vi "Lab Panel V4.2.vi"() -> ()   [LabVIEW 2013]
uses:
  <vilib>/Platform/TimedLoop/XDataNode/timing_clust.ctl
  <vilib>/Platform/TimedLoop/XDataNode/nitl_modes.ctl
  <vilib>/Platform/TimedLoop/XDataNode/wakeup.ctl
  Global 1.vi
  <vilib>/platform/TimedLoop/XDataNode/XDataNode.xnode
  <vilib>/Platform/TimedLoop/XDataNode/XDNodeRunTimeDep.lvlib
panel:
  out "TEMP update":bool
  out "AI update":bool
  in  "stop":bool
  in  "Tab Control 2":T1(tab)
  out "SIG LAB05-2":T2 {"PF" format="%.2f"; "AMPS" format="%.1f"}
  out "SIG LAB05-1":T2 {"PF" format="%.2f"; "AMPS" format="%.1f"}
  out "SIG LAB04-2":T2 {"PF" format="%.2f"; "AMPS" format="%.1f"}
  out "SIG LAB04-1":T2 {"PF" format="%.2f"; "AMPS" format="%.1f"}
  out "SIG LAB03-2":T2 {"PF" format="%.2f"; "AMPS" format="%.1f"}
  out "SIG LAB03-1":T2 {"PF" format="%.2f"; "AMPS" format="%.1f"}
  out "SIG LAB02-2":T2 {"PF" format="%.2f"; "AMPS" format="%.1f"}
  in  "RUN LAB01-1":bool
  in  "O/I  LAB05-1":bool
  in  "O/I  LAB05-2":bool
  in  "O/I  LAB04-1":bool
  in  "O/I  LAB04-2":bool
  in  "O/I  LAB02-1":bool
  in  "O/I  LAB02-2":bool
  in  "O/I  LAB01-2":bool
  in  "O/I  LAB01-1":bool
  in  "O/I  LAB03-1":bool
  in  "RUN LAB05-2":bool
  in  "RUN LAB05-1":bool
  in  "RUN LAB04-2":bool
  in  "RUN LAB04-1":bool
  in  "RUN LAB03-2":bool
  in  "RUN LAB03-1":bool
  in  "RUN LAB02-2":bool
  in  "RUN LAB02-1":bool
  in  "RUN LAB01-2":bool
  in  "SELECT LAB05-2":T3(radio)
  in  "SELECT LAB05-1":T3(radio)
  in  "SELECT LAB04-2":T3(radio)
  in  "SELECT LAB04-1":T3(radio)
  in  "SELECT LAB03-2":T3(radio)
  in  "SELECT LAB03-1":T3(radio)
  in  "SELECT LAB02-2":T3(radio)
  in  "SELECT LAB02-1":T3(radio)
  in  "SELECT LAB01-2":T3(radio)
  in  "SELECT LAB01-1":T3(radio)
  in  "O/I  LAB03-2":bool
  out "SIG LAB01-1":T2 {"PF" format="%.2f"; "AMPS" format="%.1f"}
  out "SIG LAB01-2":T2 {"PF" format="%.2f"; "AMPS" format="%.1f"}
  out "SIG LAB02-1":T2 {"PF" format="%.2f"; "AMPS" format="%.1f"}
  out "DISP LAB05-2":T4 {"MINS" format="%.2g"}
  out "DISP LAB05-1":T4 {"MINS" format="%.2g"}
  out "DISP LAB04-2":T4 {"MINS" format="%.2g"}
  out "DISP LAB04-1":T4 {"MINS" format="%.2g"}
  out "DISP LAB03-2":T4 {"MINS" format="%.2g"}
  out "DISP LAB03-1":T4 {"MINS" format="%.2g"}
  in  "SET LAB05-2":T5={"NAME"="", "DESCRIPTION"="", "CYCLES"=5.0, "T-RISE mins"=0.0, "T-RISE deg C"=0.0} {"CYCLES" min=5.0 step=1.0}
  in  "SET LAB05-1":T5={"NAME"="", "DESCRIPTION"="", "CYCLES"=5.0, "T-RISE mins"=0.0, "T-RISE deg C"=0.0} {"CYCLES" min=5.0 step=1.0}
  in  "SET LAB04-2":T5={"NAME"="", "DESCRIPTION"="", "CYCLES"=5.0, "T-RISE mins"=0.0, "T-RISE deg C"=0.0} {"CYCLES" min=5.0 step=1.0}
  in  "SET LAB04-1":T5={"NAME"="", "DESCRIPTION"="", "CYCLES"=5.0, "T-RISE mins"=0.0, "T-RISE deg C"=0.0} {"CYCLES" min=5.0 step=1.0}
  in  "SET LAB03-2":T5={"NAME"="", "DESCRIPTION"="", "CYCLES"=5.0, "T-RISE mins"=0.0, "T-RISE deg C"=0.0} {"CYCLES" min=5.0 step=1.0}
  in  "SET LAB03-1":T5={"NAME"="", "DESCRIPTION"="", "CYCLES"=5.0, "T-RISE mins"=0.0, "T-RISE deg C"=0.0} {"CYCLES" min=5.0 step=1.0}
  out "DISP LAB02-2":T4 {"MINS" format="%.2g"}
  out "DISP LAB02-1":T4 {"MINS" format="%.2g"}
  in  "SET LAB02-2":T5={"NAME"="", "DESCRIPTION"="", "CYCLES"=5.0, "T-RISE mins"=0.0, "T-RISE deg C"=0.0} {"CYCLES" min=5.0 step=1.0}
  in  "SET LAB02-1":T5={"NAME"="", "DESCRIPTION"="", "CYCLES"=5.0, "T-RISE mins"=0.0, "T-RISE deg C"=0.0} {"CYCLES" min=5.0 step=1.0}
  out "RESULT LAB05-2":bool
  out "RESULT LAB05-1":bool
  out "RESULT LAB04-2":bool
  out "RESULT LAB04-1":bool
  out "RESULT LAB03-2":bool
  out "RESULT LAB03-1":bool
  out "RESULT LAB02-2":bool
  out "RESULT LAB02-1":bool
  out "RESULT LAB01-2":bool
  out "RESULT LAB01-1":bool
  in  "SET LAB01-1":T5={"NAME"="", "DESCRIPTION"="", "CYCLES"=5.0, "T-RISE mins"=0.0, "T-RISE deg C"=0.0} {"CYCLES" min=5.0 step=1.0}
  in  "SET LAB01-2":T5={"NAME"="", "DESCRIPTION"="", "CYCLES"=5.0, "T-RISE mins"=0.0, "T-RISE deg C"=0.0} {"CYCLES" min=5.0 step=1.0}
  out "DISP LAB01-1":T4 {"MINS" format="%.2g"}
  out "DISP LAB01-2":T4 {"MINS" format="%.2f"}
  out "TEMP RISE LAB05-2":cluster{"TL":dbl, "TN":dbl}
  out "TEMP RISE LAB05-1":cluster{"TL":dbl, "TN":dbl}
  out "TEMP RISE LAB04-2":cluster{"TL":dbl, "TN":dbl}
  out "TEMP RISE LAB04-1":cluster{"TL":dbl, "TN":dbl}
  out "TEMP RISE LAB03-2":cluster{"TL":dbl, "TN":dbl}
  out "TEMP RISE LAB03-1":cluster{"TL":dbl, "TN":dbl}
  out "TEMP RISE LAB02-2":cluster{"TL":dbl, "TN":dbl}
  out "TEMP RISE LAB02-1":cluster{"TL":dbl, "TN":dbl}
  out "TEMP RISE LAB01-2":cluster{"TL":dbl, "TN":dbl}
  out "TEMP RISE LAB01-1":cluster{"TL":dbl, "TN":dbl}
  in  "JIG OFF TIME (S)":dbl=2.0 min=2.0 max=10.0 step=0.5 format="%.1g"
  in  "JIG ON TIME (S)":dbl=1.0 min=1.0 max=10.0 step=0.5 format="%.1g"
  out "JIG LAB05-2":bool
  out "JIG LAB05-1":bool
  out "JIG LAB04-2":bool
  out "JIG LAB04-1":bool
  out "JIG LAB03-2":bool
  out "JIG LAB03-1":bool
  out "JIG LAB02-2":bool
  out "JIG LAB02-1":bool
  out "JIG LAB01-2":bool
  out "JIG LAB01-1":bool
  out "TEMP START LAB01-1":cluster{"TL":dbl, "TN":dbl}
  out "TEMP START LAB02-1":cluster{"TL":dbl, "TN":dbl}
  out "TEMP START LAB03-1":cluster{"TL":dbl, "TN":dbl}
  out "TEMP START LAB04-1":cluster{"TL":dbl, "TN":dbl}
  out "TEMP START LAB01-2":cluster{"TL":dbl, "TN":dbl}
  out "TEMP START LAB02-2":cluster{"TL":dbl, "TN":dbl}
  out "TEMP START LAB03-2":cluster{"TL":dbl, "TN":dbl}
  out "TEMP START LAB04-2":cluster{"TL":dbl, "TN":dbl}
  out "TEMP START LAB05-2":cluster{"TL":dbl, "TN":dbl}
  out "TEMP START LAB05-1":cluster{"TL":dbl, "TN":dbl}
  in  "MAIL SETTINGS":T6
  out "MAIL REPORT":string
  in  "TO (string):":string
  in  "Send Mail Now":bool
  in  "Auto Mail Send":bool
  in  "Network Directory":path
  out "CAL LAB01":T7 {"2 (TN) cal" min=0.0 step=0.01 format="%.2f"; "2 (TL) cal" min=0.0 step=0.01 format="%.2f"; "2 (PF) cal" min=0.0 step=0.01 format="%.2f"; "2 (V) cal" min=0.0 step=0.01 format="%.2f"; "2 (A) cal" min=0.0 step=0.01 format="%.2f"; "1 (TN) cal" min=0.0 step=0.01 format="%.2f"; "1 (TL) cal" min=0.0 step=0.01 format="%.2f"; "1 (PF) cal" min=0.0 step=0.01 format="%.2f"; "1 (V) cal" min=0.0 step=0.01 format="%.2f"; "1  (A) cal" min=0.0 step=0.01 format="%.2f"}
  out "CAL LAB03":T7 {"2 (TN) cal" min=0.0 step=0.01 format="%.2f"; "2 (TL) cal" min=0.0 step=0.01 format="%.2f"; "2 (PF) cal" min=0.0 step=0.01 format="%.2f"; "2 (V) cal" min=0.0 step=0.01 format="%.2f"; "2 (A) cal" min=0.0 step=0.01 format="%.2f"; "1 (TN) cal" min=0.0 step=0.01 format="%.2f"; "1 (TL) cal" min=0.0 step=0.01 format="%.2f"; "1 (PF) cal" min=0.0 step=0.01 format="%.2f"; "1 (V) cal" min=0.0 step=0.01 format="%.2f"; "1  (A) cal" min=0.0 step=0.01 format="%.2f"}
  out "CAL LAB02":T8 {"2 (TN) cal" min=0.0 step=0.01 format="%.2f"; "2 (TL) cal" min=0.0 step=0.01 format="%.2f"; "2 (PF) cal" min=0.0 step=0.01 format="%.2f"; "2 (V) cal" min=0.0 step=0.01 format="%.2f"; "2 (A) cal" min=0.0 step=0.01 format="%.2f"; "1 (TN) cal" min=0.0 step=0.01 format="%.2f"; "1 (TL) cal" min=0.0 step=0.01 format="%.2f"; "1 (PF) cal" min=0.0 step=0.01 format="%.2f"; "1 (V) cal" min=0.0 step=0.01 format="%.2f"; "1 (A) cal" min=0.0 step=0.01 format="%.2f"}
  out "CAL LAB05":T7 {"2 (TN) cal" min=0.0 step=0.01 format="%.2f"; "2 (TL) cal" min=0.0 step=0.01 format="%.2f"; "2 (PF) cal" min=0.0 step=0.01 format="%.2f"; "2 (V) cal" min=0.0 step=0.01 format="%.2f"; "2 (A) cal" min=0.0 step=0.01 format="%.2f"; "1 (TN) cal" min=0.0 step=0.01 format="%.2f"; "1 (TL) cal" min=0.0 step=0.01 format="%.2f"; "1 (PF) cal" min=0.0 step=0.01 format="%.2f"; "1 (V) cal" min=0.0 step=0.01 format="%.2f"; "1  (A) cal" min=0.0 step=0.01 format="%.2f"}
  out "CAL LAB04":T7 {"2 (TN) cal" min=0.0 step=0.01 format="%.2f"; "2 (TL) cal" min=0.0 step=0.01 format="%.2f"; "2 (PF) cal" min=0.0 step=0.01 format="%.2f"; "2 (V) cal" min=0.0 step=0.01 format="%.2f"; "2 (A) cal" min=0.0 step=0.01 format="%.2f"; "1 (TN) cal" min=0.0 step=0.01 format="%.2f"; "1 (TL) cal" min=0.0 step=0.01 format="%.2f"; "1 (PF) cal" min=0.0 step=0.01 format="%.2f"; "1 (V) cal" min=0.0 step=0.01 format="%.2f"; "1  (A) cal" min=0.0 step=0.01 format="%.2f"}
  out "calibration file error out":errorcluster
  in  "CALIBRATE":bool
  in  "SHOW ADMIN PAGE":bool
  out "ON L05-2":cluster{"amps":dbl, "volts":dbl, "pf":dbl}
  out "ON L05-1":cluster{"amps":dbl, "volts":dbl, "pf":dbl}
  out "FAIL LAB05-2":cluster{"LO":dbl, "HI":dbl}
  out "FAIL LAB05-1":cluster{"LO":dbl, "HI":dbl}
  out "FAIL LAB04-2":cluster{"LO":dbl, "HI":dbl}
  out "FAIL LAB04-1":cluster{"LO":dbl, "HI":dbl}
  out "FAIL LAB03-2":cluster{"LO":dbl, "HI":dbl}
  out "FAIL LAB03-1":cluster{"LO":dbl, "HI":dbl}
  out "FAIL LAB02-2":cluster{"LO":dbl, "HI":dbl}
  out "FAIL LAB02-1":cluster{"LO":dbl, "HI":dbl}
  out "FAIL LAB01-2":cluster{"LO":dbl, "HI":dbl}
  out "FAIL LAB01-1":cluster{"LO":dbl, "HI":dbl}
  out "ON L01-1":cluster{"amps":dbl, "volts":dbl, "pf":dbl}
  out "ON L01-2":cluster{"amps":dbl, "volts":dbl, "pf":dbl}
  out "ON L02-1":cluster{"amps":dbl, "volts":dbl, "pf":dbl}
  out "ON L02-2":cluster{"amps":dbl, "volts":dbl, "pf":dbl}
  out "ON L03-1":cluster{"amps":dbl, "volts":dbl, "pf":dbl}
  out "ON L03-2":cluster{"amps":dbl, "volts":dbl, "pf":dbl}
  out "ON L04-1":cluster{"amps":dbl, "volts":dbl, "pf":dbl}
  out "ON L04-2":cluster{"amps":dbl, "volts":dbl, "pf":dbl}
  in  "C drive data root dir":path
  out "run lab05-2":bool
  out "run lab05-1":bool
  out "run lab04-2":bool
  out "run lab04-1":bool
  out "run lab03-2":bool
  out "run lab03-1":bool
  out "run lab02-2":bool
  out "run lab02-1":bool
  out "run lab01-2":bool
  out "run lab01-1":bool
  out "stop2":bool
  in  "Tab Control":T9(tab)
  out "LAB01-2 (GRAPH)":dynamicdata(graph)
  out "LAB01-1 (GRAPH)":dynamicdata(graph)
  out "LAB02-2 (GRAPH)":dynamicdata(graph)
  out "LAB02-1 (GRAPH)":dynamicdata(graph)
  out "LAB03-2 (GRAPH)":dynamicdata(graph)
  out "LAB03-1 (GRAPH)":dynamicdata(graph)
  out "LAB04-2 (GRAPH)":dynamicdata(graph)
  out "LAB04-1 (GRAPH)":dynamicdata(graph)
  out "LAB05-2 (GRAPH)":dynamicdata(graph)
  out "LAB05-1 (GRAPH)":dynamicdata(graph)
  out "LAB05 TEMP":T10
  out "LAB04 TEMP":T10
  out "LAB02 TEMP":T10
  out "LAB01 TEMP":T10
  out "LAB03 TEMP":T10
  out "Analog Error Array":errorcluster[](array[cluster])
  out "AI loop time":dbl format="%.6g"
  out "loops":dbl
  in  "loop  delay(mS)":dbl
  out "on loops":dbl
  out "off loops":dbl
  out "jig cycle":dbl
  out "TDMS LAB01-1":refnum<k34>
  out "data file error":errorcluster
  out "TDMS LAB02-1":refnum<k34>
  out "TDMS LAB01-2":refnum<k34>
  out "TDMS LAB02-2":refnum<k34>
  out "TDMS LAB03-1":refnum<k34>
  out "TDMS LAB03-2":refnum<k34>
  out "TDMS LAB04-1":refnum<k34>
  out "TDMS LAB04-2":refnum<k34>
  out "TDMS LAB05-1":refnum<k34>
  out "TDMS LAB05-2":refnum<k34>
  out "mail control":string
  # "LAB01"
  # "LAB02"
  # "LAB05"
  # "LAB03"
  # "LAB04"
  # "LAB01"
  # "LAB02"
  # "LAB03"
  # "LAB04"
  # "LAB05"
  # "JIG SET"
  # "(Enter recipients address seperated by comma)"
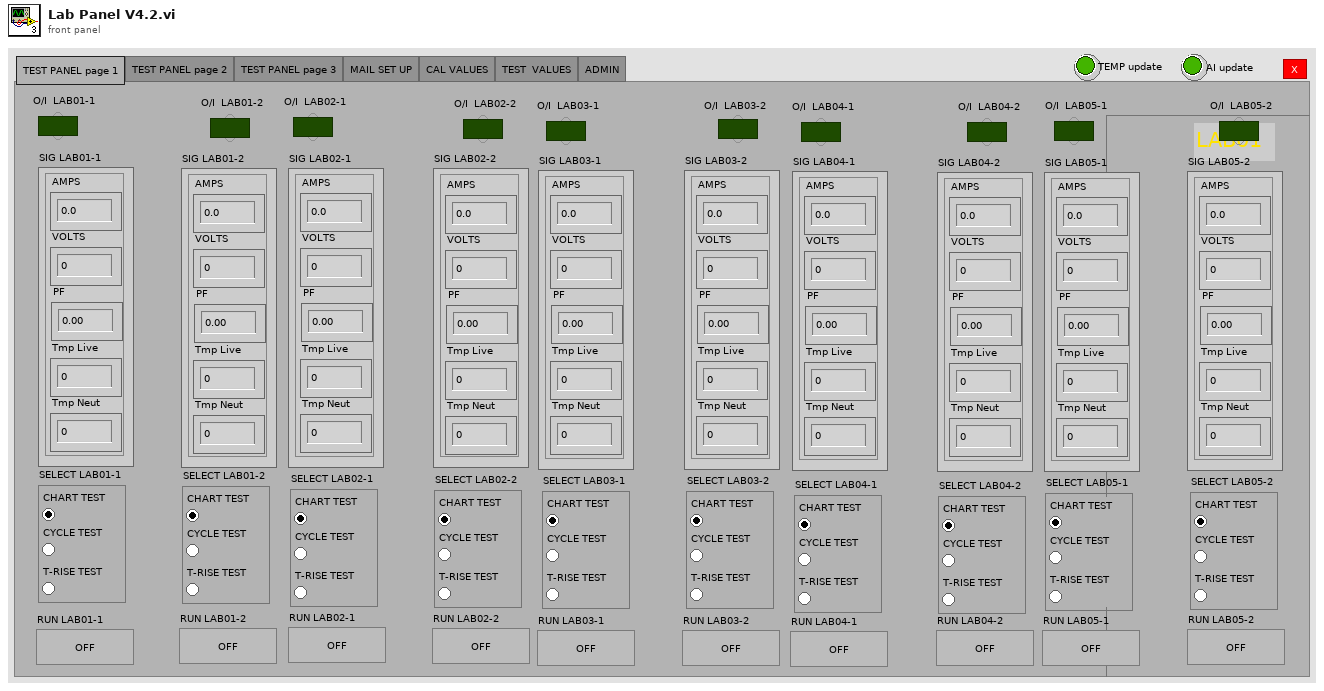
[diagram p1: front panel]
types:
  T1 = enum32{"TEST PANEL page 1", "TEST PANEL page 2", "TEST PANEL page 3", "MAIL SET UP", "CAL VALUES", "TEST  VALUES", "ADMIN"}
  T2 = cluster{"AMPS":dbl, "VOLTS":dbl, "PF":dbl, "Tmp Live":dbl, "Tmp Neut":dbl}
  T3 = enum32{"CHART TEST", "CYCLE TEST", "T-RISE TEST"}
  T4 = cluster{"CYCLE":dbl, "MINS":dbl, "STATUS":string}
  T5 = cluster{"NAME":string, "DESCRIPTION":string, "CYCLES":dbl, "T-RISE mins":dbl, "T-RISE deg C":dbl}
  T6 = cluster{"OUT SERVER ADDRESS":string, "FROM ACCOUNT":string, "USER NAME":string, "PASSWORD":string, "TEST MAIL":bool, "TEST MAIL STATUS":string, "mail error":errorcluster}
  T7 = cluster{"1  (A) cal":dbl, "1 (V) cal":dbl, "1 (PF) cal":dbl, "1 (TL) cal":dbl, "1 (TN) cal":dbl, "2 (A) cal":dbl, "2 (V) cal":dbl, "2 (PF) cal":dbl, "2 (TL) cal":dbl, "2 (TN) cal":dbl}
  T8 = cluster{"1 (A) cal":dbl, "1 (V) cal":dbl, "1 (PF) cal":dbl, "1 (TL) cal":dbl, "1 (TN) cal":dbl, "2 (A) cal":dbl, "2 (V) cal":dbl, "2 (PF) cal":dbl, "2 (TL) cal":dbl, "2 (TN) cal":dbl}
  T9 = enum32{"LAB01", "LAB02", "LAB03", "LAB04", "LAB05", "TEMPERATURE", "ERROR"}
  T10 = cluster{"T1 Live":dbl, "T1 Neut":dbl, "T2 Live":dbl, "T2 Neut":dbl, "ID":dbl, "ER":dbl}
  T11 = enum8{"Enabled", "Disabled", "Disabled and Grayed Out"}
  T12 = typedef "XDNodeRunTimeDep.lvlib/timing_clust.ctl" = cluster{"Expected End [f-1]":u64, "Actual End [f-1]":u64, "Finished Late? [f-1]":bool, "Expected End [i-1]":u64, "Actual End [i-1]":u64, "Finished Late? [i-1]":bool, "Expected Start [i]":u64, "Actual Start [i]":u64, "Expected Start [f]":u64, "Actual Start [f]":u64, "Source Name":string, "Structure Name":string, "Period":i64, "Deadline":i64, "Offset":i64, "Start":i64, "Priority":i32, "Timeout":i32, "Mode":T13, "Wakeup Reason":T14, "Error":errorcluster, "Source Type":string, "Secondary Source Type":string, "Global End Time":u64, "Global Start Time":u64, "Frame Duration":u64, "Iteration Duration":u64, "Assigned CPU":i32, "I/O Scan Engine Mode":u32}
  T13 = typedef "XDNodeRunTimeDep.lvlib/nitl_modes.ctl" = enum32{"No Change", "Process missed periods, maintain original phase", "Discard missed periods, maintain original phase", "Process missed periods, ignore original phase", "Discard missed periods, ignore original phase"}
  T14 = typedef "XDNodeRunTimeDep.lvlib/wakeup.ctl" = enum32{"Normal", "Aborted", "Asynchronous wakeup", "Timing source error", "Timed loop error", "Timeout"}
  T15 = enum16{"open", "open or create", "create or replace", "create", "open (read-only)"}
  T16 = enum16{"open", "replace", "create", "open or create", "replace or create", "replace or create with confirmation"}
  T17 = cluster{"SET LAB01-1":cluster{"NAME":string, "DESCRIPTION":string, "CYCLES":dbl, "T-RISE mins":dbl, "T-RISE deg C":dbl}, "SET LAB01-2":cluster{"NAME":string, "DESCRIPTION":string, "CYCLES":dbl, "T-RISE mins":dbl, "T-RISE deg C":dbl}, "SET LAB02-1":cluster{"NAME":string, "DESCRIPTION":string, "CYCLES":dbl, "T-RISE mins":dbl, "T-RISE deg C":dbl}, "SET LAB02-2":cluster{"NAME":string, "DESCRIPTION":string, "CYCLES":dbl, "T-RISE mins":dbl, "T-RISE deg C":dbl}, "SET LAB03-1":cluster{"NAME":string, "DESCRIPTION":string, "CYCLES":dbl, "T-RISE mins":dbl, "T-RISE deg C":dbl}, "SET LAB03-2":cluster{"NAME":string, "DESCRIPTION":string, "CYCLES":dbl, "T-RISE mins":dbl, "T-RISE deg C":dbl}, "SET LAB04-1":cluster{"NAME":string, "DESCRIPTION":string, "CYCLES":dbl, "T-RISE mins":dbl, "T-RISE deg C":dbl}, "SET LAB04-2":cluster{"NAME":string, "DESCRIPTION":string, "CYCLES":dbl, "T-RISE mins":dbl, "T-RISE deg C":dbl}, "SET LAB05-1":cluster{"NAME":string, "DESCRIPTION":string, "CYCLES":dbl, "T-RISE mins":dbl, "T-RISE deg C":dbl}, "SET LAB05-2":cluster{"NAME":string, "DESCRIPTION":string, "CYCLES":dbl, "T-RISE mins":dbl, "T-RISE deg C":dbl}, "Network Directory":path, "C drive data root dir":path}
  T18 = cluster{"MAIL SETTINGS":cluster{"OUT SERVER ADDRESS":string, "FROM ACCOUNT":string, "USER NAME":string, "PASSWORD":string, "TEST MAIL":bool, "TEST MAIL STATUS":string, "mail error":errorcluster}, "Auto Mail Send":bool, string}
  T19 = cluster{"T1":dbl, "T2":dbl, "T3":dbl, "T4":dbl, "ID":dbl, "ER":dbl}
  T20 = cluster{"LAB01-1 (A)":dbl, "LAB01-1 (V)":dbl, "LAB01-1 (PF)":dbl, "LAB01-2 (A)":dbl, "LAB01-2 (V)":dbl, "LAB01-2 (PF)":dbl}
  T21 = cluster{"LAB02-1 (A)":dbl, "LAB02-1 (V)":dbl, "LAB02-1 (PF)":dbl, "LAB02-2 (A)":dbl, "LAB02-2 (V)":dbl, "LAB02-2 (PF)":dbl}
  T22 = cluster{"LAB03-1 (A)":dbl, "LAB03-1 (V)":dbl, "LAB03-1 (PF)":dbl, "LAB03-2 (A)":dbl, "LAB03-2 (V)":dbl, "LAB03-2 (PF)":dbl}
  T23 = cluster{"LAB04-1 (A)":dbl, "LAB04-1 (V)":dbl, "LAB04-1 (PF)":dbl, "LAB04-2 (A)":dbl, "LAB04-2 (V)":dbl, "LAB04-2 (PF)":dbl}
  T24 = cluster{"LAB05-1 (A)":dbl, "LAB05-1 (V)":dbl, "LAB05-1 (PF)":dbl, "LAB05-2 (A)":dbl, "LAB05-2 (V)":dbl, "LAB05-2 (PF)":dbl}
  T25 = cluster{"FAIL LAB01-1":cluster{"LO":dbl, "HI":dbl}, "SIG LAB01-1":cluster{"AMPS":dbl, "VOLTS":dbl, "PF":dbl, "Tmp Live":dbl, "Tmp Neut":dbl}, "TEMP START LAB01-1":cluster{"TL":dbl, "TN":dbl}, "DISP LAB01-1":cluster{"CYCLE":dbl, "MINS":dbl, "STATUS":string}, "SET LAB01-1":cluster{"NAME":string, "DESCRIPTION":string, "CYCLES":dbl, "T-RISE mins":dbl, "T-RISE deg C":dbl}, "TDMS LAB01-1":refnum<k34>}
  T26 = cluster{"FAIL LAB01-2":cluster{"LO":dbl, "HI":dbl}, "SIG LAB01-2":cluster{"AMPS":dbl, "VOLTS":dbl, "PF":dbl, "Tmp Live":dbl, "Tmp Neut":dbl}, "TEMP START LAB01-2":cluster{"TL":dbl, "TN":dbl}, "DISP LAB01-2":cluster{"CYCLE":dbl, "MINS":dbl, "STATUS":string}, "SET LAB01-2":cluster{"NAME":string, "DESCRIPTION":string, "CYCLES":dbl, "T-RISE mins":dbl, "T-RISE deg C":dbl}, "TDMS LAB01-2":refnum<k34>}
  T27 = cluster{"FAIL LAB02-1":cluster{"LO":dbl, "HI":dbl}, "SIG LAB02-1":cluster{"AMPS":dbl, "VOLTS":dbl, "PF":dbl, "Tmp Live":dbl, "Tmp Neut":dbl}, "TEMP START LAB02-1":cluster{"TL":dbl, "TN":dbl}, "DISP LAB02-1":cluster{"CYCLE":dbl, "MINS":dbl, "STATUS":string}, "SET LAB02-1":cluster{"NAME":string, "DESCRIPTION":string, "CYCLES":dbl, "T-RISE mins":dbl, "T-RISE deg C":dbl}, "TDMS LAB02-1":refnum<k34>}
  T28 = cluster{"FAIL LAB02-2":cluster{"LO":dbl, "HI":dbl}, "SIG LAB02-2":cluster{"AMPS":dbl, "VOLTS":dbl, "PF":dbl, "Tmp Live":dbl, "Tmp Neut":dbl}, "TEMP START LAB02-2":cluster{"TL":dbl, "TN":dbl}, "DISP LAB02-2":cluster{"CYCLE":dbl, "MINS":dbl, "STATUS":string}, "SET LAB02-2":cluster{"NAME":string, "DESCRIPTION":string, "CYCLES":dbl, "T-RISE mins":dbl, "T-RISE deg C":dbl}, "TDMS LAB02-2":refnum<k34>}
  T29 = cluster{"FAIL LAB03-1":cluster{"LO":dbl, "HI":dbl}, "SIG LAB03-1":cluster{"AMPS":dbl, "VOLTS":dbl, "PF":dbl, "Tmp Live":dbl, "Tmp Neut":dbl}, "TEMP START LAB03-1":cluster{"TL":dbl, "TN":dbl}, "DISP LAB03-1":cluster{"CYCLE":dbl, "MINS":dbl, "STATUS":string}, "SET LAB03-1":cluster{"NAME":string, "DESCRIPTION":string, "CYCLES":dbl, "T-RISE mins":dbl, "T-RISE deg C":dbl}, "TDMS LAB03-1":refnum<k34>}
  T30 = cluster{"FAIL LAB03-2":cluster{"LO":dbl, "HI":dbl}, "SIG LAB03-2":cluster{"AMPS":dbl, "VOLTS":dbl, "PF":dbl, "Tmp Live":dbl, "Tmp Neut":dbl}, "TEMP START LAB03-2":cluster{"TL":dbl, "TN":dbl}, "DISP LAB03-2":cluster{"CYCLE":dbl, "MINS":dbl, "STATUS":string}, "SET LAB03-2":cluster{"NAME":string, "DESCRIPTION":string, "CYCLES":dbl, "T-RISE mins":dbl, "T-RISE deg C":dbl}, "TDMS LAB03-2":refnum<k34>}
  T31 = cluster{"FAIL LAB04-1":cluster{"LO":dbl, "HI":dbl}, "SIG LAB04-1":cluster{"AMPS":dbl, "VOLTS":dbl, "PF":dbl, "Tmp Live":dbl, "Tmp Neut":dbl}, "TEMP START LAB04-1":cluster{"TL":dbl, "TN":dbl}, "DISP LAB04-1":cluster{"CYCLE":dbl, "MINS":dbl, "STATUS":string}, "SET LAB04-1":cluster{"NAME":string, "DESCRIPTION":string, "CYCLES":dbl, "T-RISE mins":dbl, "T-RISE deg C":dbl}, "TDMS LAB04-1":refnum<k34>}
  T32 = cluster{"FAIL LAB04-2":cluster{"LO":dbl, "HI":dbl}, "SIG LAB04-2":cluster{"AMPS":dbl, "VOLTS":dbl, "PF":dbl, "Tmp Live":dbl, "Tmp Neut":dbl}, "TEMP START LAB04-2":cluster{"TL":dbl, "TN":dbl}, "DISP LAB04-2":cluster{"CYCLE":dbl, "MINS":dbl, "STATUS":string}, "SET LAB04-2":cluster{"NAME":string, "DESCRIPTION":string, "CYCLES":dbl, "T-RISE mins":dbl, "T-RISE deg C":dbl}, "TDMS LAB04-2":refnum<k34>}
  T33 = cluster{"FAIL LAB05-1":cluster{"LO":dbl, "HI":dbl}, "SIG LAB05-1":cluster{"AMPS":dbl, "VOLTS":dbl, "PF":dbl, "Tmp Live":dbl, "Tmp Neut":dbl}, "TEMP START LAB05-1":cluster{"TL":dbl, "TN":dbl}, "DISP LAB05-1":cluster{"CYCLE":dbl, "MINS":dbl, "STATUS":string}, "SET LAB05-1":cluster{"NAME":string, "DESCRIPTION":string, "CYCLES":dbl, "T-RISE mins":dbl, "T-RISE deg C":dbl}, "TDMS LAB05-1":refnum<k34>}
  T34 = cluster{"FAIL LAB05-2":cluster{"LO":dbl, "HI":dbl}, "SIG LAB05-2":cluster{"AMPS":dbl, "VOLTS":dbl, "PF":dbl, "Tmp Live":dbl, "Tmp Neut":dbl}, "TEMP START LAB05-2":cluster{"TL":dbl, "TN":dbl}, "DISP LAB05-2":cluster{"CYCLE":dbl, "MINS":dbl, "STATUS":string}, "SET LAB05-2":cluster{"NAME":string, "DESCRIPTION":string, "CYCLES":dbl, "T-RISE mins":dbl, "T-RISE deg C":dbl}, "TDMS LAB05-2":refnum<k34>}
  T35 = cluster{"MAIL SETTINGS":cluster{"OUT SERVER ADDRESS":string, "FROM ACCOUNT":string, "USER NAME":string, "PASSWORD":string, "TEST MAIL":bool, "TEST MAIL STATUS":string, "mail error":errorcluster}, "Auto Mail Send":bool, "TO (string):":string}
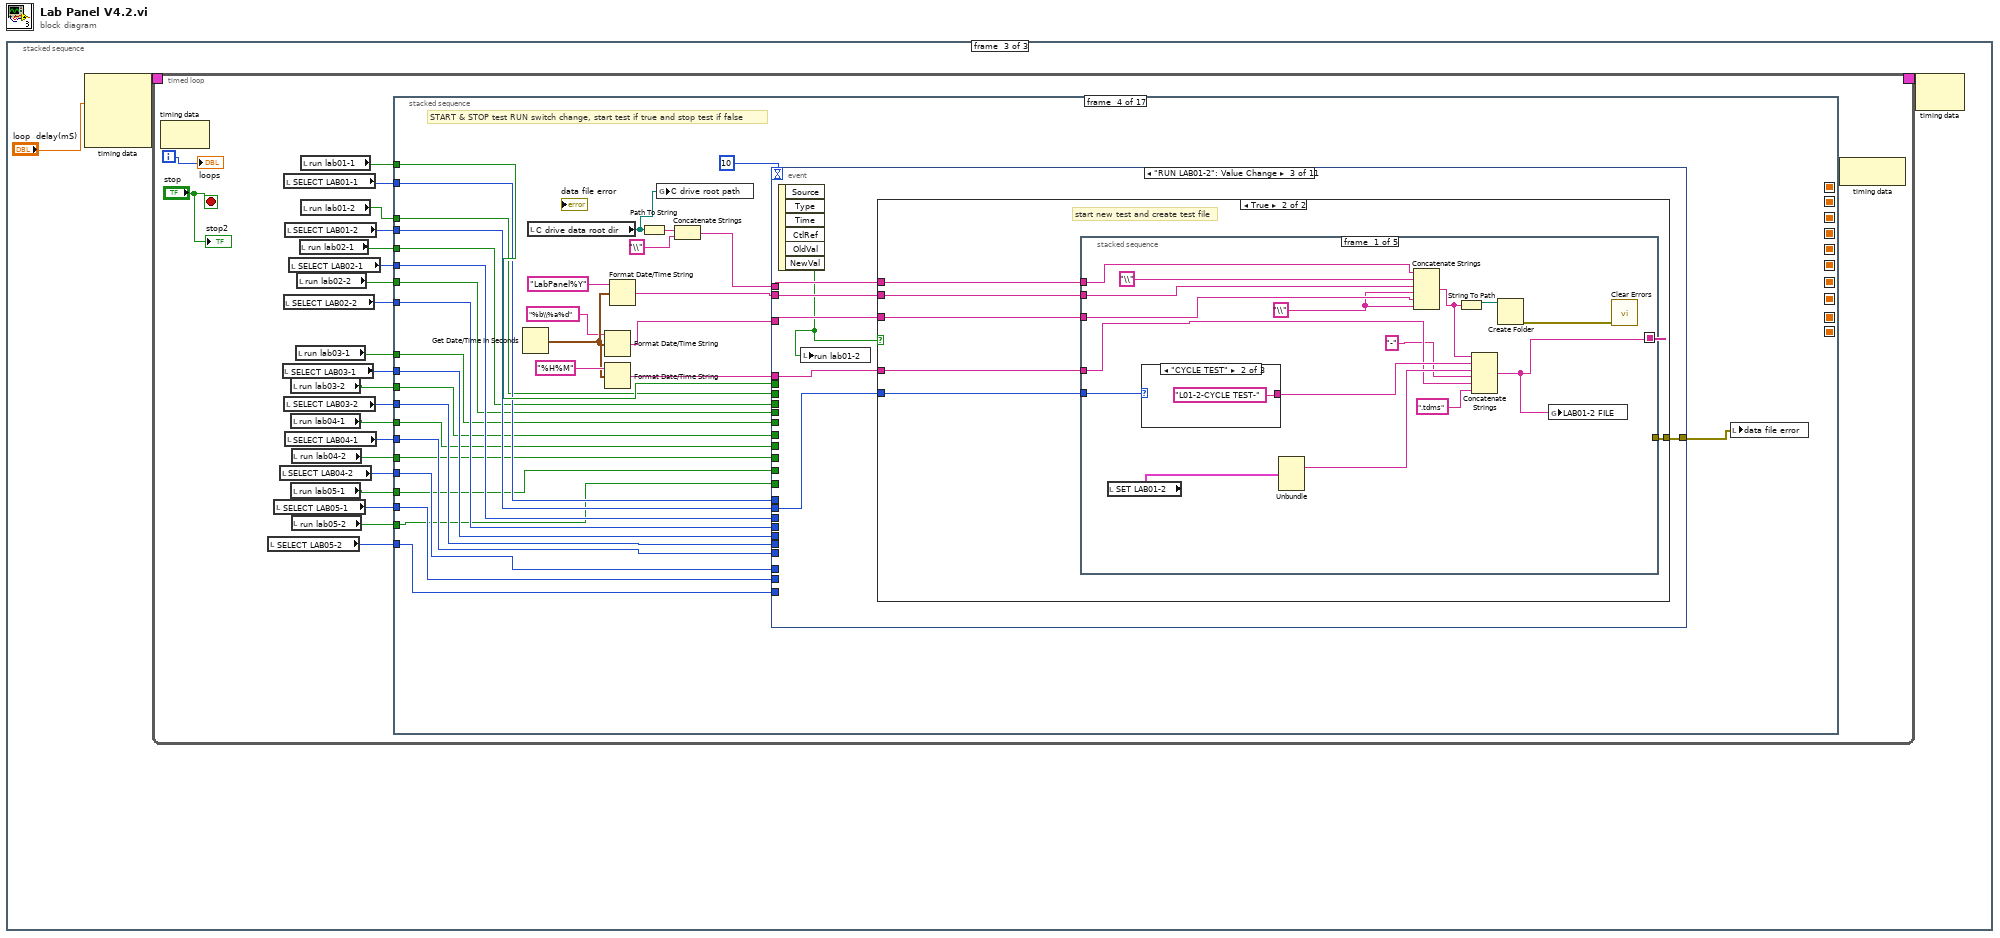
[diagram p0: block diagram]
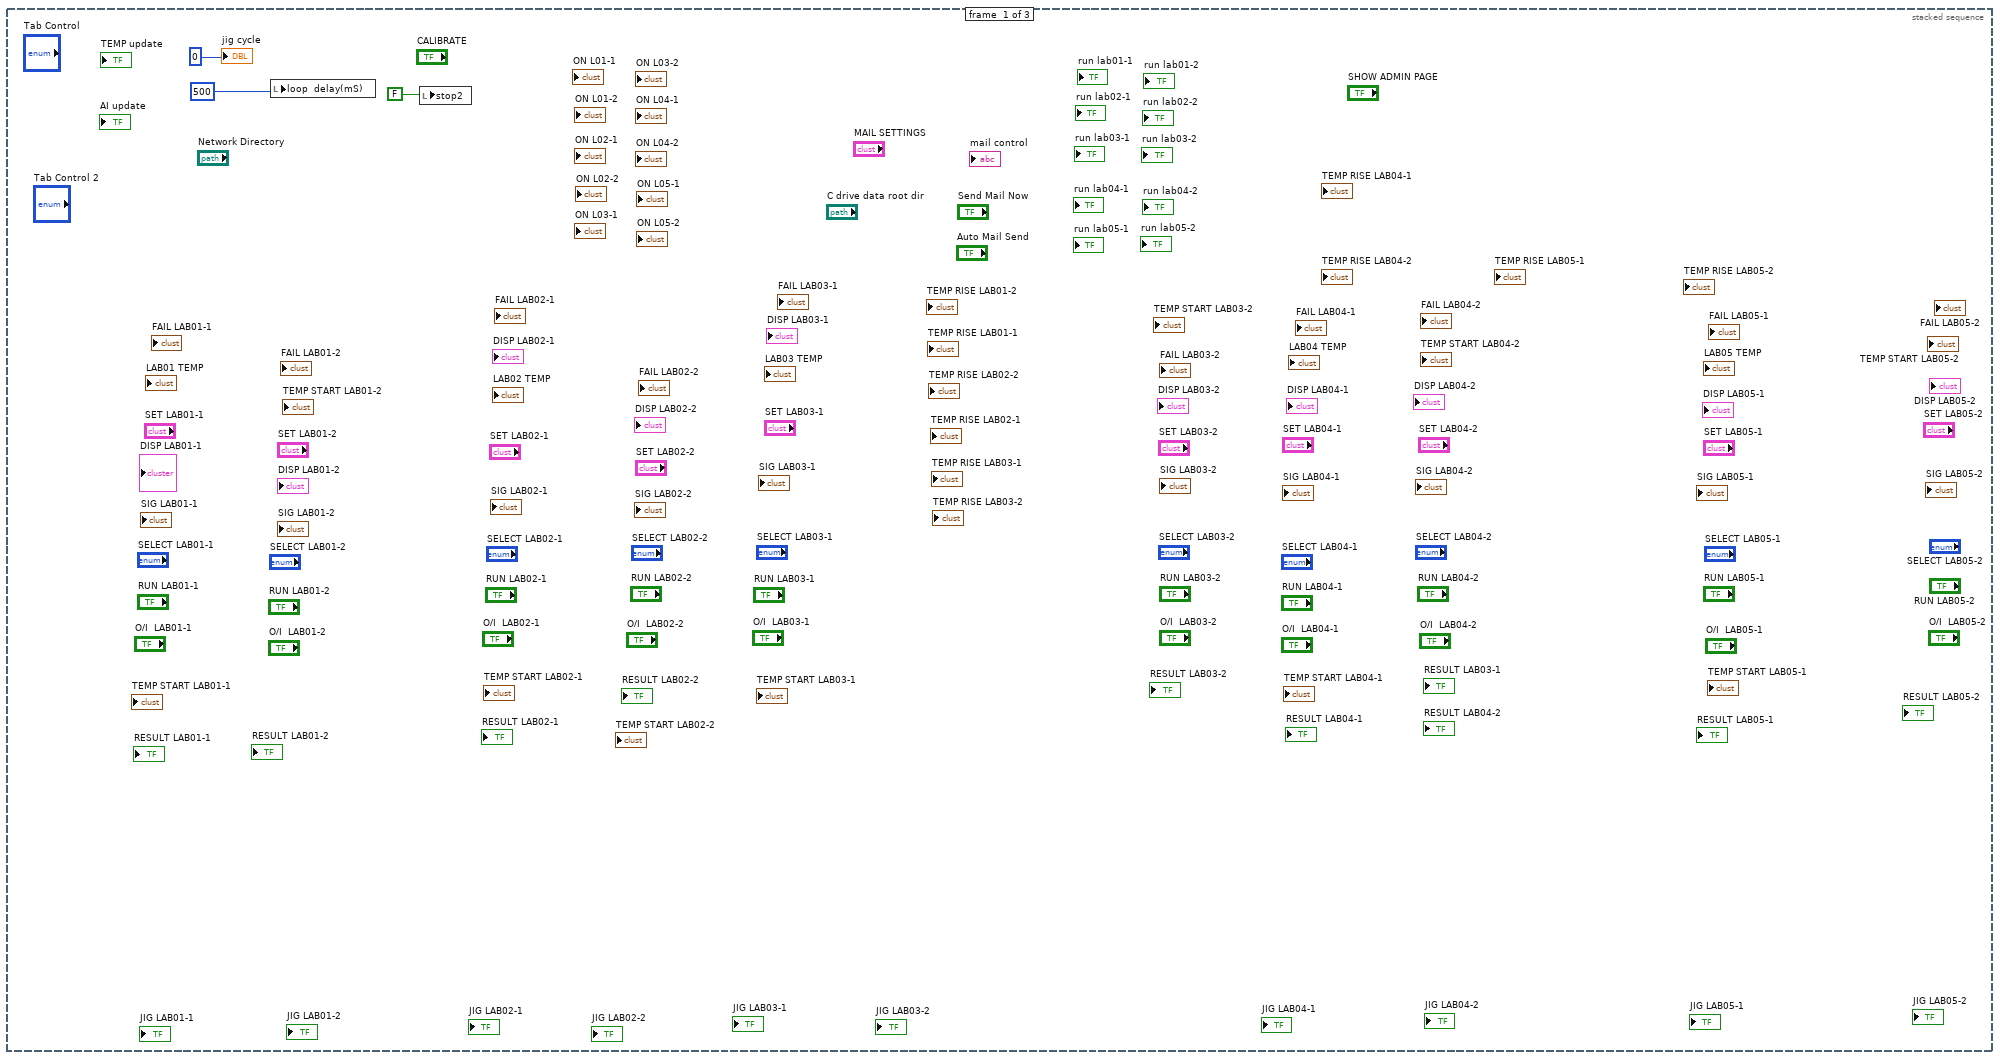
[diagram p2: hidden frame]
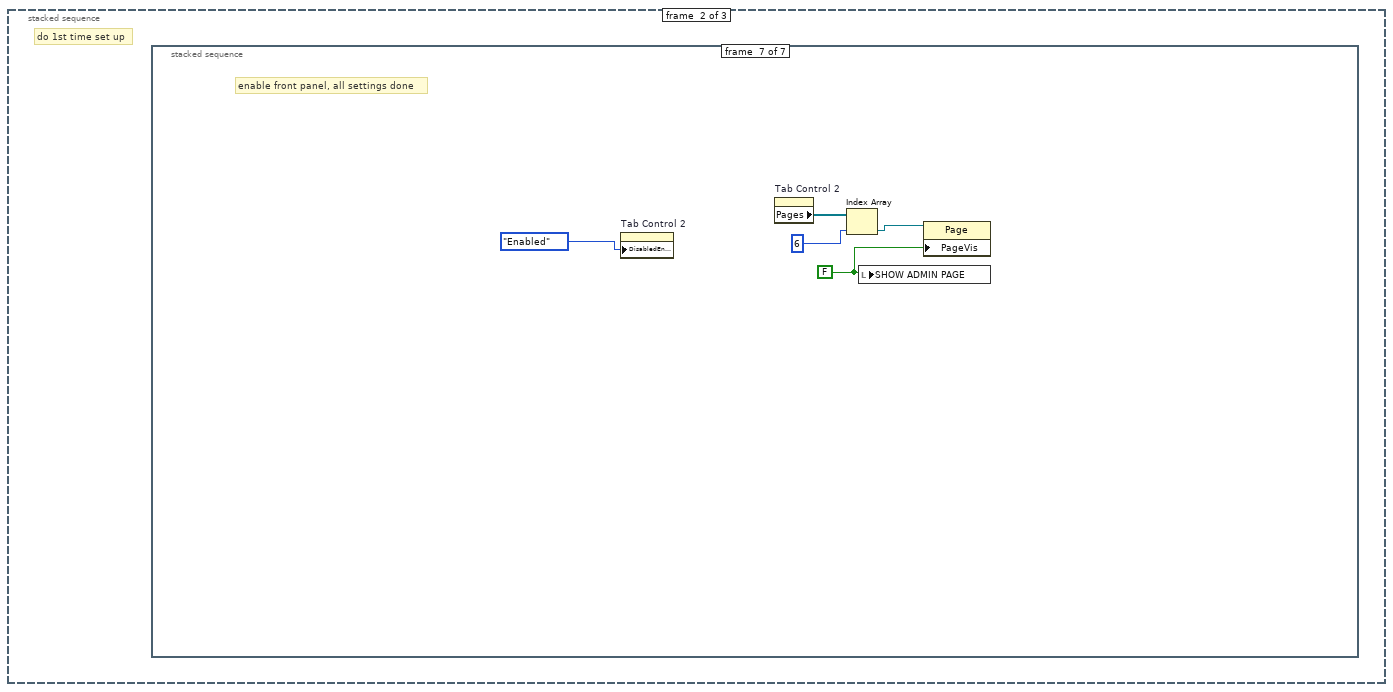
[diagram p3: hidden frame]
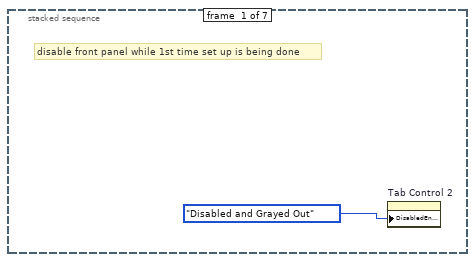
[diagram p4: hidden frame]
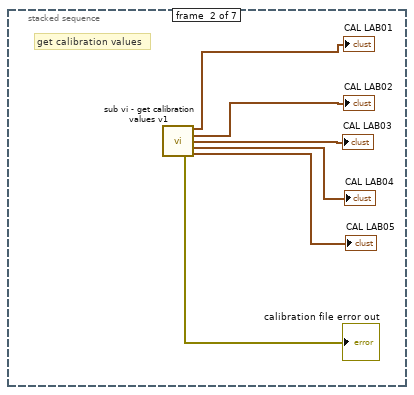
[diagram p5: hidden frame]
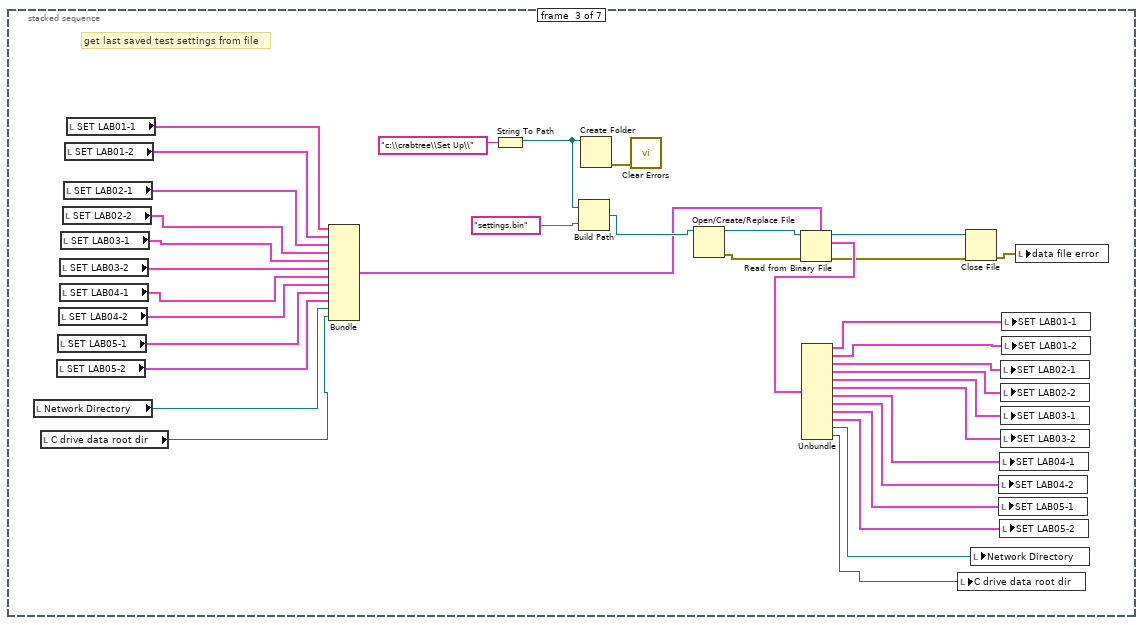
[diagram p6: hidden frame]
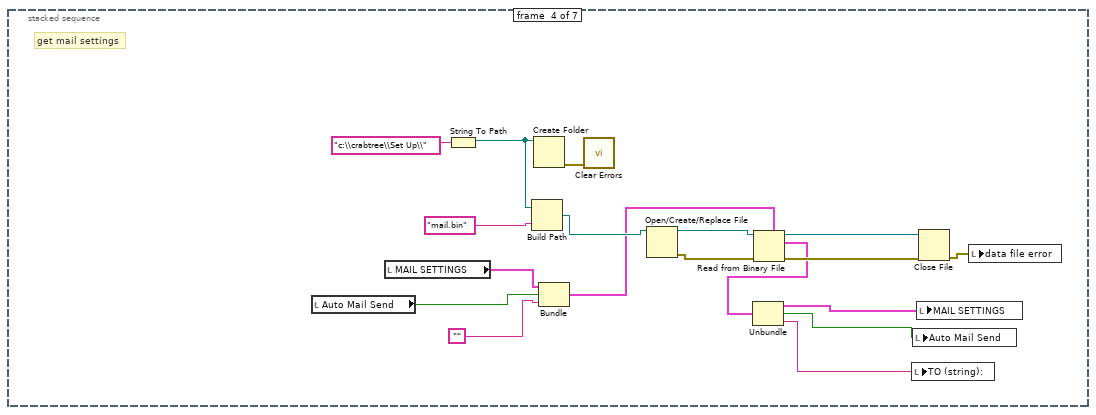
[diagram p7: hidden frame]
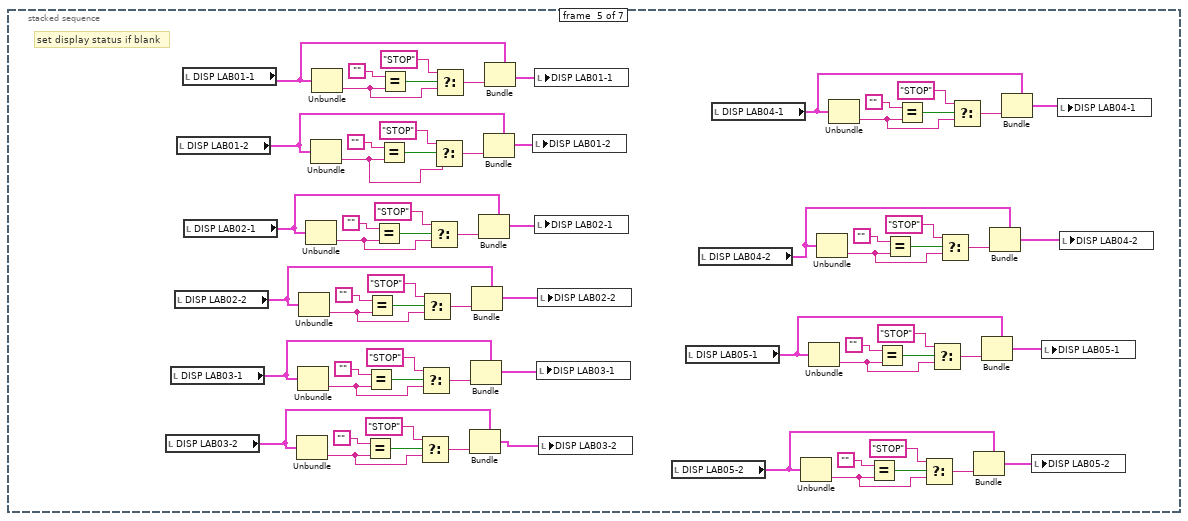
[diagram p8: hidden frame]
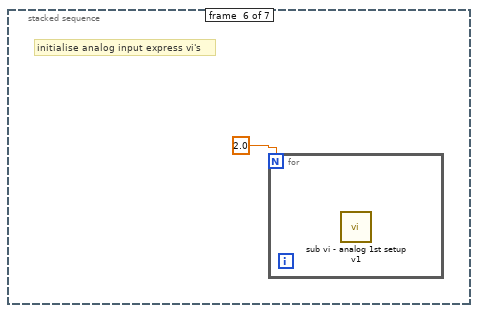
[diagram p9: hidden frame]
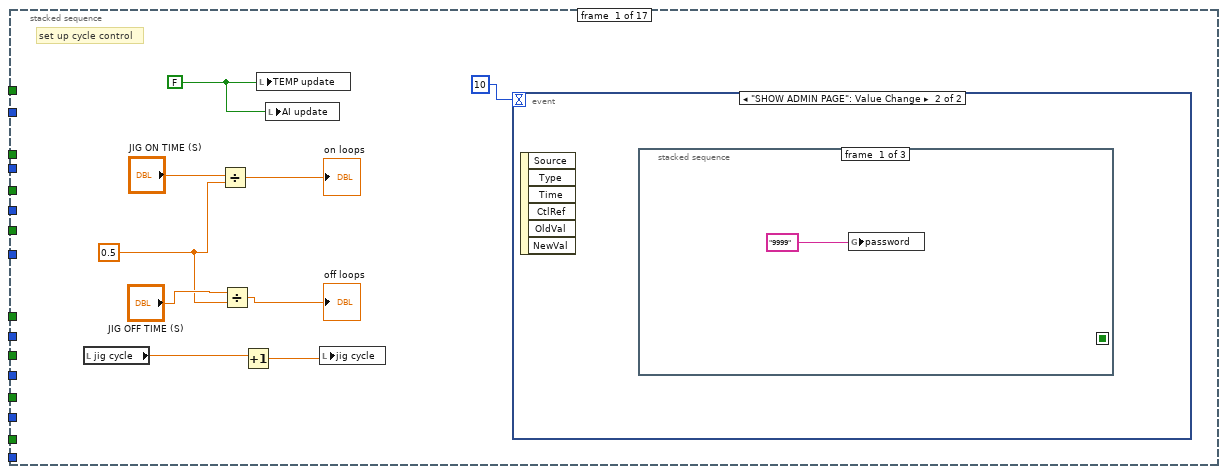
[diagram p10: hidden frame]
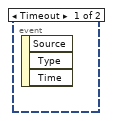
[diagram p11: hidden frame]
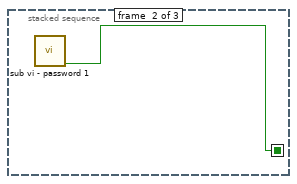
[diagram p12: hidden frame]
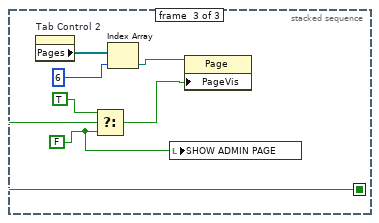
[diagram p13: hidden frame]
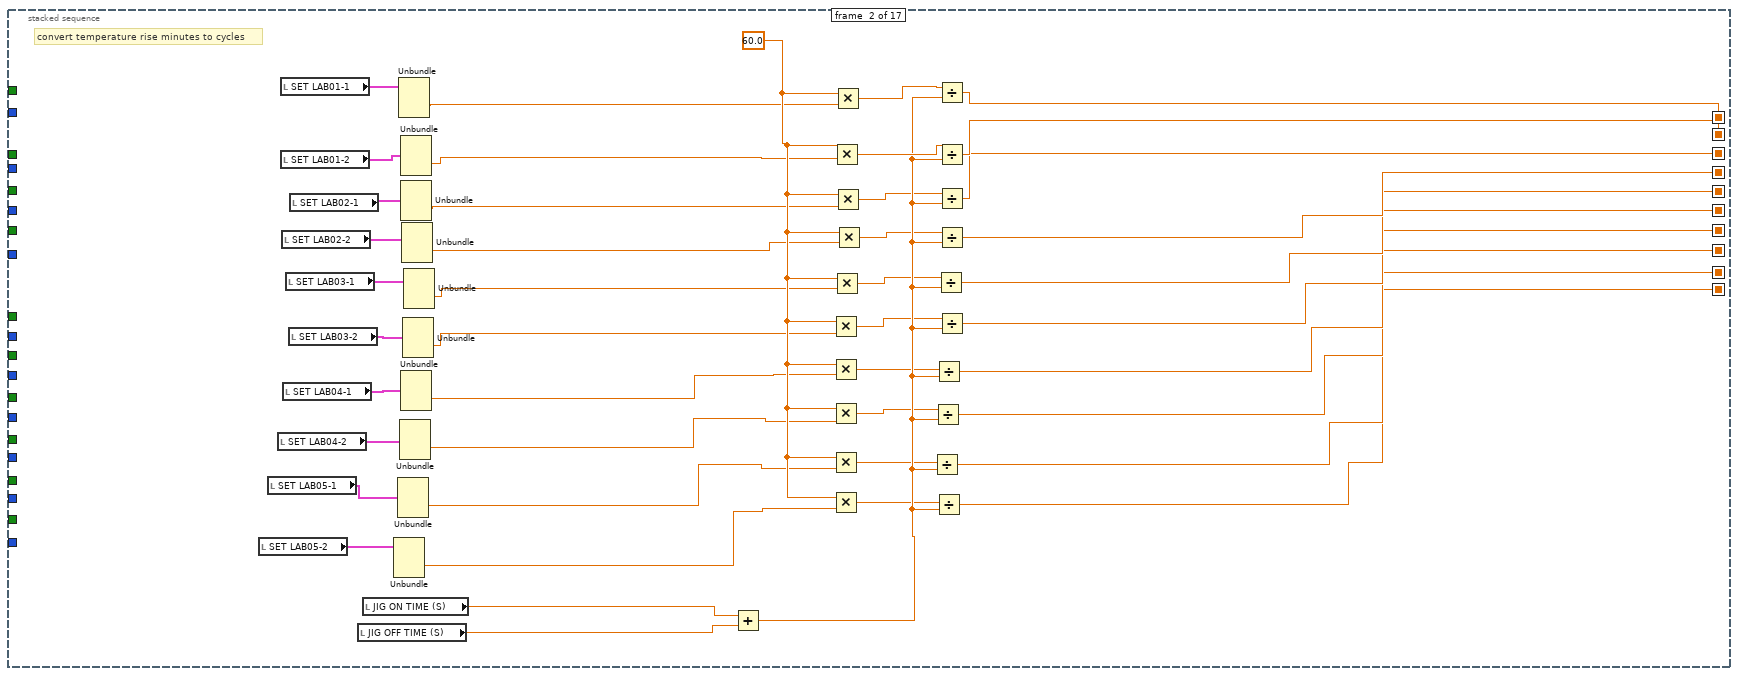
[diagram p14: hidden frame]
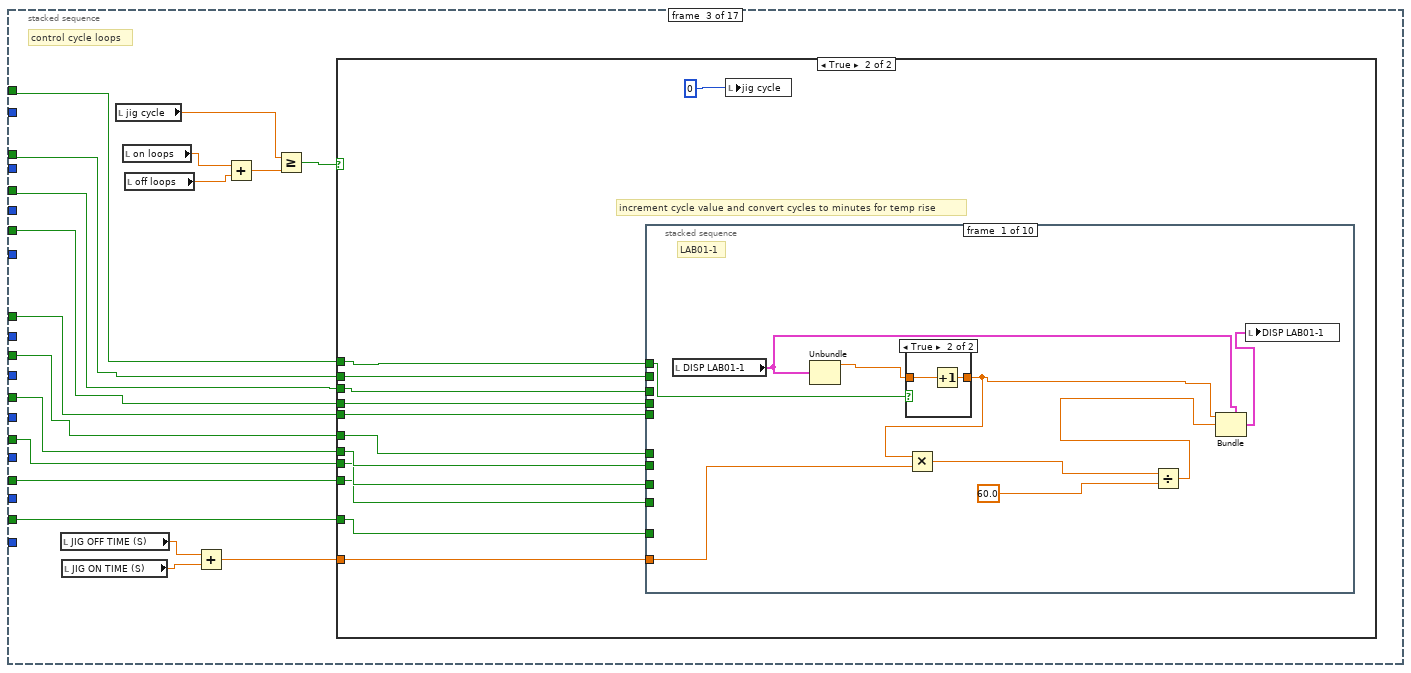
[diagram p15: hidden frame]
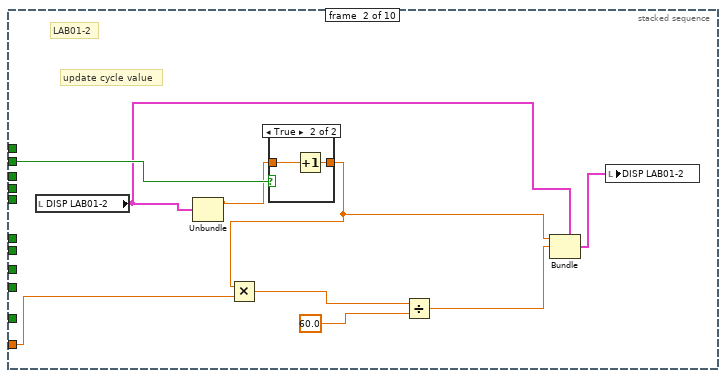
[diagram p18: hidden frame]
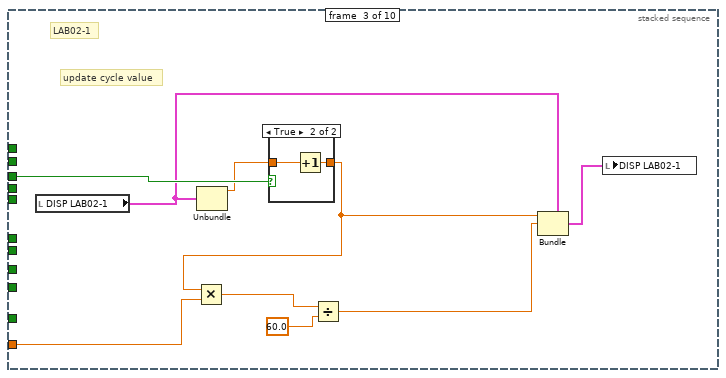
[diagram p20: hidden frame]
diagram:
  n1 = stacked-sequence {
    frame #0 {
      n2 = local write "loop  delay(mS)"(500) -> ()
      n3 = local write "stop2"(FALSE) -> ()
      "jig cycle" <- 0
    }
    frame #1 {
      # "do 1st time set up"
      n4 = stacked-sequence {
        frame #0 {
          # "disable front panel while 1st time set up is being done"
          n5 = property on="Tab Control 2" class="TabCtl (strict)"("DisabledEnum"=T11."Disabled and Grayed Out" ("Disabled")) -> ()  [unwired: 2 in, 2 out]
        }
        frame #1 {
          # "get calibration values"
          n6 = call "sub vi - get calibration values v1.vi"() -> ("LAB01 (CAL)"=→"CAL LAB01":T7, "LAB02 (CAL)"=→"CAL LAB02":T8, "LAB03 (CAL)"=→"CAL LAB03":T7, "LAB04 (CAL)"=→"CAL LAB04":T7, "calibration file error out"=→"calibration file error out":errorcluster, "LAB05 (CAL)"=→"CAL LAB05":T7)  [unwired: 10 in]
        }
        frame #2 {
          # "get last saved test settings from file"
          n7 = local read "Network Directory"() -> (w13:path)
          n8 = local read "C drive data root dir"() -> (w11:path)
          n9 = local read "SET LAB05-2"() -> (w43:T5)
          n10 = local read "SET LAB05-1"() -> (w44:T5)
          n11 = local read "SET LAB04-2"() -> (w45:T5)
          n12 = local read "SET LAB03-2"() -> (w42:T5)
          n13 = local read "SET LAB04-1"() -> (w46:T5)
          n14 = local read "SET LAB03-1"() -> (w41:T5)
          n15 = local read "SET LAB02-2"() -> (w40:T5)
          n16 = local read "SET LAB02-1"() -> (w39:T5)
          n17 = local read "SET LAB01-2"() -> (w38:T5)
          n18 = local read "SET LAB01-1"() -> (w37:T5)
          n19 = Bundle("SET LAB01-1"=w37, "SET LAB01-2"=w38, "SET LAB02-1"=w39, "SET LAB02-2"=w40, "SET LAB03-1"=w41, "SET LAB03-2"=w42, "SET LAB04-1"=w46, "SET LAB04-2"=w45, "SET LAB05-1"=w44, "SET LAB05-2"=w43, "Network Directory"=w13, "C drive data root dir"=w11) -> (w30:T17)  [unwired: 1 in]
          n20 = String To Path(string="c:\\crabtree\\Set Up\\") -> (path=w34:path)
          n21 = Build Path(base path=w34, name or relative path="settings.bin") -> (appended path=w32:path)
          n22 = Create Folder(path (use dialog)=w34) -> (error out=w36:errorcluster)  [unwired: 2 in, 2 out]
          n23 = call <vilib>:"Clear Errors.vi"("error in (no error)"=w36) -> ()  [unwired: 6 in, 1 out]
          n24 = Open/Create/Replace File(file path (use dialog)=w32) -> (refnum out=w29:refnum<file>, error out=w31:errorcluster)  [unwired: 5 in, 1 out]
          n25 = Read from Binary File(5:w30, 8:w31, 11:w29) -> (0:w26:errorcluster, 2:w28:T17, 3:w27:refnum<file>)  [unwired: 3 in, 1 out]
          n26 = Unbundle(w28) -> ("SET LAB01-1"=w24:T5, "SET LAB01-2"=w23:T5, "SET LAB02-1"=w22:T5, "SET LAB02-2"=w21:T5, "SET LAB03-1"=w20:T5, "SET LAB03-2"=w19:T5, "SET LAB04-1"=w18:T5, "SET LAB04-2"=w17:T5, "SET LAB05-1"=w16:T5, "SET LAB05-2"=w15:T5, "Network Directory"=w14:path, "C drive data root dir"=w12:path)
          n27 = local write "C drive data root dir"(w12) -> ()
          n28 = Close File(refnum=w27, error in=w26) -> (error out=w25:errorcluster)  [unwired: 1 out]
          n29 = local write "Network Directory"(w14) -> ()
          n30 = local write "SET LAB04-2"(w17) -> ()
          n31 = local write "SET LAB05-1"(w16) -> ()
          n32 = local write "SET LAB04-1"(w18) -> ()
          n33 = local write "SET LAB05-2"(w15) -> ()
          n34 = local write "SET LAB02-1"(w22) -> ()
          n35 = local write "SET LAB02-2"(w21) -> ()
          n36 = local write "SET LAB03-1"(w20) -> ()
          n37 = local write "SET LAB03-2"(w19) -> ()
          n38 = local write "SET LAB01-1"(w24) -> ()
          n39 = local write "SET LAB01-2"(w23) -> ()
          n40 = local write "data file error"(w25) -> ()
        }
        frame #3 {
          # "get mail settings"
          n41 = local read "Auto Mail Send"() -> (w50:bool)
          n42 = local read "MAIL SETTINGS"() -> (w54:T6)
          n43 = String To Path(string="c:\\crabtree\\Set Up\\") -> (path=w62:path)
          n44 = Build Path(base path=w62, name or relative path="mail.bin") -> (appended path=w60:path)
          n45 = Create Folder(path (use dialog)=w62) -> (error out=w64:errorcluster)  [unwired: 2 in, 2 out]
          n46 = Bundle("MAIL SETTINGS"=w54, "Auto Mail Send"=w50, "") -> (w53:T18)  [unwired: 1 in]
          n47 = call <vilib>:"Clear Errors.vi"("error in (no error)"=w64) -> ()  [unwired: 6 in, 1 out]
          n48 = Open/Create/Replace File(file path (use dialog)=w60) -> (refnum out=w58:refnum<file>, error out=w59:errorcluster)  [unwired: 5 in, 1 out]
          n49 = Read from Binary File(5:w53, 8:w59, 11:w58) -> (0:w56:errorcluster, 2:w52:T18, 3:w57:refnum<file>)  [unwired: 3 in, 1 out]
          n50 = Unbundle(w52) -> ("MAIL SETTINGS"=w51:T6, "Auto Mail Send"=w49:bool, w48:string)
          n51 = local write "TO (string):"(w48) -> ()
          n52 = local write "Auto Mail Send"(w49) -> ()
          n53 = local write "MAIL SETTINGS"(w51) -> ()
          n54 = Close File(refnum=w57, error in=w56) -> (error out=w55:errorcluster)  [unwired: 1 out]
          n55 = local write "data file error"(w55) -> ()
        }
        frame #4 {
          # "set display status if blank"
          n56 = local read "DISP LAB03-2"() -> (w94:T4)
          n57 = local read "DISP LAB03-1"() -> (w101:T4)
          n58 = local read "DISP LAB02-2"() -> (w108:T4)
          n59 = local read "DISP LAB01-2"() -> (w121:T4)
          n60 = local read "DISP LAB01-1"() -> (w130:T4)
          n61 = local read "DISP LAB02-1"() -> (w115:T4)
          n62 = Unbundle(w94) -> ("STATUS"=w96:string)  [unwired: 2 out]
          n63 = Unbundle(w101) -> ("STATUS"=w103:string)  [unwired: 2 out]
          n64 = Unbundle(w108) -> ("STATUS"=w110:string)  [unwired: 2 out]
          n65 = Unbundle(w115) -> ("STATUS"=w117:string)  [unwired: 2 out]
          n66 = Unbundle(w121) -> ("STATUS"=w124:string)  [unwired: 2 out]
          n67 = Unbundle(w130) -> ("STATUS"=w131:string)  [unwired: 2 out]
          n68 = Equal?(x="", y=w96) -> (x = y?=w98:bool)
          n69 = Equal?(x="", y=w103) -> (x = y?=w105:bool)
          n70 = Equal?(x="", y=w110) -> (x = y?=w112:bool)
          n71 = Equal?(x="", y=w117) -> (x = y?=w119:bool)
          n72 = Equal?(x="", y=w124) -> (x = y?=w126:bool)
          n73 = Equal?(x="", y=w131) -> (x = y?=w133:bool)
          n74 = Select(t="STOP", s=w98, f=w96) -> (s? t:f=w95:string)
          n75 = Select(t="STOP", s=w105, f=w103) -> (s? t:f=w102:string)
          n76 = Select(t="STOP", s=w112, f=w110) -> (s? t:f=w109:string)
          n77 = Select(t="STOP", s=w119, f=w117) -> (s? t:f=w116:string)
          n78 = Select(t="STOP", s=w126, f=w124) -> (s? t:f=w123:string)
          n79 = Select(t="STOP", s=w133, f=w131) -> (s? t:f=w129:string)
          n80 = Bundle(cluster=w94, "STATUS"=w95) -> (w93:T4)  [unwired: 2 in]
          n81 = Bundle(cluster=w101, "STATUS"=w102) -> (w100:T4)  [unwired: 2 in]
          n82 = Bundle(cluster=w108, "STATUS"=w109) -> (w107:T4)  [unwired: 2 in]
          n83 = Bundle(cluster=w115, "STATUS"=w116) -> (w114:T4)  [unwired: 2 in]
          n84 = Bundle(cluster=w121, "STATUS"=w123) -> (w122:T4)  [unwired: 2 in]
          n85 = Bundle(cluster=w130, "STATUS"=w129) -> (w128:T4)  [unwired: 2 in]
          n86 = local write "DISP LAB01-2"(w122) -> ()
          n87 = local write "DISP LAB01-1"(w128) -> ()
          n88 = local write "DISP LAB02-1"(w114) -> ()
          n89 = local write "DISP LAB03-1"(w100) -> ()
          n90 = local write "DISP LAB02-2"(w107) -> ()
          n91 = local write "DISP LAB03-2"(w93) -> ()
          n92 = local read "DISP LAB05-2"() -> (w66:T4)
          n93 = local read "DISP LAB05-1"() -> (w73:T4)
          n94 = local read "DISP LAB04-2"() -> (w75:T4)
          n95 = local read "DISP LAB04-1"() -> (w77:T4)
          n96 = Unbundle(w66) -> ("STATUS"=w68:string)  [unwired: 2 out]
          n97 = Unbundle(w73) -> ("STATUS"=w79:string)  [unwired: 2 out]
          n98 = Unbundle(w75) -> ("STATUS"=w84:string)  [unwired: 2 out]
          n99 = Unbundle(w77) -> ("STATUS"=w89:string)  [unwired: 2 out]
          n100 = Equal?(x="", y=w68) -> (x = y?=w70:bool)
          n101 = Equal?(x="", y=w79) -> (x = y?=w81:bool)
          n102 = Equal?(x="", y=w84) -> (x = y?=w86:bool)
          n103 = Equal?(x="", y=w89) -> (x = y?=w91:bool)
          n104 = Select(t="STOP", s=w70, f=w68) -> (s? t:f=w67:string)
          n105 = Select(t="STOP", s=w81, f=w79) -> (s? t:f=w78:string)
          n106 = Select(t="STOP", s=w86, f=w84) -> (s? t:f=w83:string)
          n107 = Select(t="STOP", s=w91, f=w89) -> (s? t:f=w88:string)
          n108 = Bundle(cluster=w66, "STATUS"=w67) -> (w65:T4)  [unwired: 2 in]
          n109 = Bundle(cluster=w73, "STATUS"=w78) -> (w72:T4)  [unwired: 2 in]
          n110 = Bundle(cluster=w75, "STATUS"=w83) -> (w74:T4)  [unwired: 2 in]
          n111 = Bundle(cluster=w77, "STATUS"=w88) -> (w76:T4)  [unwired: 2 in]
          n112 = local write "DISP LAB05-2"(w65) -> ()
          n113 = local write "DISP LAB05-1"(w72) -> ()
          n114 = local write "DISP LAB04-1"(w76) -> ()
          n115 = local write "DISP LAB04-2"(w74) -> ()
        }
        frame #5 {
          # "initialise analog input express vi's"
          n116 = for {
            N: 2.0 -> [_]
            n117 = call "sub vi - analog 1st setup v1.vi"() -> ()  [unwired: 11 in, 5 out]
          }
        }
        frame #6 {
          w136 = FALSE
          # "enable front panel, all settings done"
          n118 = property on="Tab Control 2" class="TabCtl (strict)"("DisabledEnum"=T11."Enabled" ("Disabled")) -> ()  [unwired: 2 in, 2 out]
          n119 = property on="Tab Control 2" class="TabCtl (strict)"() -> ("Pages"=w137:refnum<vi>[])  [unwired: 2 in, 2 out]
          n120 = Index Array(array=w137, index=6) -> (element=w139:refnum<vi>)
          n121 = local write "SHOW ADMIN PAGE"(w136) -> ()
          n122 = property class="Page"(reference=w139, "PageVis"=w136) -> ()  [unwired: 1 in, 2 out]
        }
      }
    }
    frame #2 {
      n123 = node-c288("loop  delay(mS)") -> (w143:T12)  [unwired: 3 in]
      n124 = timed-loop {
        timing: w143 -> [_]
        timing-out: [_] -> w142
        i -> [w165]
        stop <- "stop" stop-if-true
        n125 = node-c288() -> ()  [unwired: 1 in, 1 out]
        n126 = local read "SELECT LAB05-2"() -> (w145:T3)
        n127 = local read "SELECT LAB05-1"() -> (w146:T3)
        n128 = local read "SELECT LAB04-2"() -> (w147:T3)
        n129 = local read "SELECT LAB03-1"() -> (w150:T3)
        n130 = local read "SELECT LAB02-2"() -> (w151:T3)
        n131 = local read "SELECT LAB01-1"() -> (w154:T3)
        n132 = local read "SELECT LAB03-2"() -> (w149:T3)
        n133 = local read "SELECT LAB01-2"() -> (w153:T3)
        n134 = local read "SELECT LAB04-1"() -> (w148:T3)
        n135 = local read "SELECT LAB02-1"() -> (w152:T3)
        n136 = local read "run lab03-2"() -> (w159:bool)
        n137 = local read "run lab04-1"() -> (w158:bool)
        n138 = local read "run lab05-1"() -> (w156:bool)
        n139 = local read "run lab04-2"() -> (w157:bool)
        n140 = local read "run lab05-2"() -> (w155:bool)
        n141 = local read "run lab03-1"() -> (w160:bool)
        n142 = local read "run lab02-2"() -> (w161:bool)
        n143 = local read "run lab02-1"() -> (w162:bool)
        n144 = local read "run lab01-1"() -> (w164:bool)
        n145 = local read "run lab01-2"() -> (w163:bool)
        n146 = stacked-sequence {
          seq-local: [_ w227 _ _ _ _ _ _ _ _ _ _ _ _ _ _ _] -> [_ _ _ _ _ w1762 _ _ _ _ _ _ _ _ _ _ _]
          seq-local: [_ w226 _ _ _ _ _ _ _ _ _ _ _ _ _ _ _] -> [_ _ _ _ _ w1761 _ _ _ _ _ _ _ _ _ _ _]
          seq-local: [_ w213 _ _ _ _ _ _ _ _ _ _ _ _ _ _ _] -> [_ _ _ _ _ w1760 _ _ _ _ _ _ _ _ _ _ _]
          seq-local: [_ w212 _ _ _ _ _ _ _ _ _ _ _ _ _ _ _] -> [_ _ _ _ _ w1759 _ _ _ _ _ _ _ _ _ _ _]
          seq-local: [_ w211 _ _ _ _ _ _ _ _ _ _ _ _ _ _ _] -> [_ _ _ _ _ w1758 _ _ _ _ _ _ _ _ _ _ _]
          seq-local: [_ w210 _ _ _ _ _ _ _ _ _ _ _ _ _ _ _] -> [_ _ _ _ _ w1757 _ _ _ _ _ _ _ _ _ _ _]
          seq-local: [_ w209 _ _ _ _ _ _ _ _ _ _ _ _ _ _ _] -> [_ _ _ _ _ w1756 _ _ _ _ _ _ _ _ _ _ _]
          seq-local: [_ w208 _ _ _ _ _ _ _ _ _ _ _ _ _ _ _] -> [_ _ _ _ _ w1755 _ _ _ _ _ _ _ _ _ _ _]
          seq-local: [_ w207 _ _ _ _ _ _ _ _ _ _ _ _ _ _ _] -> [_ _ _ _ _ w1754 _ _ _ _ _ _ _ _ _ _ _]
          seq-local: [_ w206 _ _ _ _ _ _ _ _ _ _ _ _ _ _ _] -> [_ _ _ _ _ w1753 _ _ _ _ _ _ _ _ _ _ _]
          tunnel: w164 -> [_ _ w243 w408 w1352 w1782 w2092 w2337 _ _ _ _ w2788 w3733 _ _ w4008]
          tunnel: w163 -> [_ _ w242 w406 w1351 w1781 w2093 w2336 _ _ _ _ w2787 w3731 _ _ w4007]
          tunnel: w162 -> [_ _ w241 w404 w1350 w1780 w2091 w2335 _ _ _ _ w2786 w3729 _ _ w4006]
          tunnel: w161 -> [_ _ w240 w402 w1349 w1779 w2090 w2334 _ _ _ _ w2785 w3727 _ _ w4005]
          tunnel: w160 -> [_ _ w239 w400 w1348 w1778 w2089 w2333 _ _ _ _ w2784 w3725 _ _ w4004]
          tunnel: w159 -> [_ _ w238 w398 w1347 w1777 w2088 w2332 _ _ _ _ w2783 w3723 _ _ w4003]
          tunnel: w158 -> [_ _ w237 w396 w1346 w1776 w2087 w2331 _ _ _ _ w2782 w3721 _ _ w4002]
          tunnel: w157 -> [_ _ w236 w394 w1345 w1775 w2086 w2330 _ _ _ _ w2781 w3719 _ _ w4001]
          tunnel: w156 -> [_ _ w235 w392 w1344 w1774 w2085 w2329 _ _ _ _ w2780 w3717 _ _ w4000]
          tunnel: w155 -> [_ _ w234 w390 w1343 w1773 w2084 w2328 _ _ _ _ w2779 w3715 _ _ w3999]
          tunnel: w154 -> [_ _ _ w407 w1342 w1772 _ _ _ _ _ _ _ w3735 _ _ _]
          tunnel: w153 -> [_ _ _ w405 w1341 w1771 _ _ _ _ _ _ _ w3730 _ _ _]
          tunnel: w152 -> [_ _ _ w403 w1340 w1770 _ _ _ _ _ _ _ w3728 _ _ _]
          tunnel: w151 -> [_ _ _ w401 w1339 w1769 _ _ _ _ _ _ _ w3726 _ _ _]
          tunnel: w150 -> [_ _ _ w399 w1338 w1768 _ _ _ _ _ _ _ w3724 _ _ _]
          tunnel: w149 -> [_ _ _ w397 w1337 w1767 _ _ _ _ _ _ _ w3722 _ _ _]
          tunnel: w148 -> [_ _ _ w395 w1336 w1766 _ _ _ _ _ _ _ w3720 _ _ _]
          tunnel: w147 -> [_ _ _ w393 w1335 w1765 _ _ _ _ _ _ _ w3718 _ _ _]
          tunnel: w146 -> [_ _ _ w391 w1334 w1764 _ _ _ _ _ _ _ w3716 _ _ _]
          tunnel: w145 -> [_ _ _ w389 w1333 w1763 _ _ _ _ _ _ _ w3714 _ _ _]
          frame #0 {
            w169 = FALSE
            w174 = 0.5
            # "set up cycle control"
            n147 = local read "jig cycle"() -> (w173:dbl)
            n148 = Divide(x="JIG ON TIME (S)", y=w174) -> (x/y=→"on loops":dbl)
            n149 = Divide(x="JIG OFF TIME (S)", y=w174) -> (x/y=→"off loops":dbl)
            n150 = Increment(x=w173) -> (x+1=w172:dbl)
            n151 = local write "TEMP update"(w169) -> ()
            n152 = local write "AI update"(w169) -> ()
            n153 = local write "jig cycle"(w172) -> ()
            n154 = event shown="[1] \"SHOW ADMIN PAGE\": Value Change" {
              selector: _ -> [_ _]
              dyn-events: _ -> [_ _]
              timeout: 10 -> [_ _]
              event Timeout {
                n155 = event-data() -> ()  [unwired: 1 in, 3 out]
              }
              event "SHOW ADMIN PAGE": Value Change {
                n156 = event-data() -> ()  [unwired: 1 in, 6 out]
                n157 = stacked-sequence {
                  seq-local: [_ w178 _] -> [_ _ w179]
                  frame #0 {
                    n158 = global write "Global 1.vi" "password"("9999") -> ()
                  }
                  frame #1 {
                    n159 = call "sub vi - password 1.vi"() -> ("RESULT"=w178:bool)  [unwired: 11 in]
                  }
                  frame #2 {
                    w181 = FALSE
                    n160 = property on="Tab Control 2" class="TabCtl (strict)"() -> ("Pages"=w185:refnum<vi>[])  [unwired: 2 in, 2 out]
                    n161 = Select(t=TRUE, s=w179, f=w181) -> (s? t:f=w180:bool)
                    n162 = Index Array(array=w185, index=6) -> (element=w183:refnum<vi>)
                    n163 = local write "SHOW ADMIN PAGE"(w181) -> ()
                    n164 = property class="Page"(reference=w183, "PageVis"=w180) -> ()  [unwired: 1 in, 2 out]
                  }
                }
              }
            }
          }
          frame #1 {
            w223 = 60.0
            # "convert temperature rise minutes to cycles"
            n165 = local read "SET LAB05-2"() -> (w187:T5)
            n166 = local read "SET LAB05-1"() -> (w189:T5)
            n167 = local read "SET LAB04-2"() -> (w191:T5)
            n168 = local read "SET LAB01-1"() -> (w205:T5)
            n169 = local read "SET LAB01-2"() -> (w203:T5)
            n170 = local read "SET LAB02-2"() -> (w199:T5)
            n171 = local read "SET LAB04-1"() -> (w193:T5)
            n172 = local read "SET LAB03-1"() -> (w197:T5)
            n173 = local read "SET LAB03-2"() -> (w195:T5)
            n174 = local read "SET LAB02-1"() -> (w201:T5)
            n175 = local read "JIG OFF TIME (S)"() -> (w228:dbl)
            n176 = local read "JIG ON TIME (S)"() -> (w229:dbl)
            n177 = Unbundle(w187) -> ("T-RISE mins"=w186:dbl)  [unwired: 4 out]
            n178 = Unbundle(w189) -> ("T-RISE mins"=w188:dbl)  [unwired: 4 out]
            n179 = Unbundle(w205) -> ("T-RISE mins"=w204:dbl)  [unwired: 4 out]
            n180 = Unbundle(w191) -> ("T-RISE mins"=w190:dbl)  [unwired: 4 out]
            n181 = Unbundle(w203) -> ("T-RISE mins"=w202:dbl)  [unwired: 4 out]
            n182 = Unbundle(w201) -> ("T-RISE mins"=w200:dbl)  [unwired: 4 out]
            n183 = Unbundle(w193) -> ("T-RISE mins"=w192:dbl)  [unwired: 4 out]
            n184 = Unbundle(w199) -> ("T-RISE mins"=w198:dbl)  [unwired: 4 out]
            n185 = Unbundle(w195) -> ("T-RISE mins"=w194:dbl)  [unwired: 4 out]
            n186 = Unbundle(w197) -> ("T-RISE mins"=w196:dbl)  [unwired: 4 out]
            n187 = Add(x=w229, y=w228) -> (x+y=w222:dbl)
            n188 = Multiply(x=w223, y=w194) -> (x*y=w218:dbl)
            n189 = Multiply(x=w223, y=w192) -> (x*y=w217:dbl)
            n190 = Multiply(x=w223, y=w190) -> (x*y=w216:dbl)
            n191 = Multiply(x=w223, y=w188) -> (x*y=w215:dbl)
            n192 = Multiply(x=w223, y=w186) -> (x*y=w214:dbl)
            n193 = Multiply(x=w223, y=w202) -> (x*y=w224:dbl)
            n194 = Multiply(x=w223, y=w196) -> (x*y=w219:dbl)
            n195 = Multiply(x=w223, y=w204) -> (x*y=w225:dbl)
            n196 = Multiply(x=w223, y=w200) -> (x*y=w221:dbl)
            n197 = Multiply(x=w223, y=w198) -> (x*y=w220:dbl)
            n198 = Divide(x=w215, y=w222) -> (x/y=w207:dbl)
            n199 = Divide(x=w216, y=w222) -> (x/y=w208:dbl)
            n200 = Divide(x=w217, y=w222) -> (x/y=w209:dbl)
            n201 = Divide(x=w214, y=w222) -> (x/y=w206:dbl)
            n202 = Divide(x=w219, y=w222) -> (x/y=w211:dbl)
            n203 = Divide(x=w225, y=w222) -> (x/y=w227:dbl)
            n204 = Divide(x=w224, y=w222) -> (x/y=w226:dbl)
            n205 = Divide(x=w221, y=w222) -> (x/y=w213:dbl)
            n206 = Divide(x=w220, y=w222) -> (x/y=w212:dbl)
            n207 = Divide(x=w218, y=w222) -> (x/y=w210:dbl)
          }
          frame #2 {
            # "control cycle loops"
            n208 = local read "JIG OFF TIME (S)"() -> (w232:dbl)
            n209 = local read "JIG ON TIME (S)"() -> (w231:dbl)
            n210 = local read "jig cycle"() -> (w245:dbl)
            n211 = local read "on loops"() -> (w247:dbl)
            n212 = local read "off loops"() -> (w246:dbl)
            n213 = Add(x=w232, y=w231) -> (x+y=w230:dbl)
            n214 = Add(x=w247, y=w246) -> (x+y=w233:dbl)
            n215 = Greater Or Equal?(x=w245, y=w233) -> (x >= y?=w244:bool)
            n216 = case shown="True" w244 {
              tunnel: w243 -> [_ w258]
              tunnel: w242 -> [_ w257]
              tunnel: w241 -> [_ w256]
              tunnel: w240 -> [_ w255]
              tunnel: w239 -> [_ w254]
              tunnel: w238 -> [_ w253]
              tunnel: w237 -> [_ w252]
              tunnel: w236 -> [_ w251]
              tunnel: w235 -> [_ w250]
              tunnel: w234 -> [_ w249]
              tunnel: w230 -> [_ w248]
              frame False {
              }
              frame True {
                # "increment cycle value and convert cycles to minutes for temp rise"
                n217 = stacked-sequence {
                  tunnel: w258 -> [w268 _ _ _ _ _ _ _ _ _]
                  tunnel: w257 -> [_ w280 _ _ _ _ _ _ _ _]
                  tunnel: w256 -> [_ _ w292 _ _ _ _ _ _ _]
                  tunnel: w255 -> [_ _ _ w304 _ _ _ _ _ _]
                  tunnel: w254 -> [_ _ _ _ w316 _ _ _ _ _]
                  tunnel: w253 -> [_ _ _ _ _ w328 _ _ _ _]
                  tunnel: w252 -> [_ _ _ _ _ _ w340 _ _ _]
                  tunnel: w251 -> [_ _ _ _ _ _ _ w352 _ _]
                  tunnel: w250 -> [_ _ _ _ _ _ _ _ w364 _]
                  tunnel: w249 -> [_ _ _ _ _ _ _ _ _ w376]
                  tunnel: w248 -> [w265 w277 w289 w301 w313 w325 w337 w349 w361 w373]
                  frame #0 {
                    # "LAB01-1"
                    n218 = local read "DISP LAB01-1"() -> (w263:T4)
                    n219 = Unbundle(w263) -> ("CYCLE"=w264:dbl)  [unwired: 2 out]
                    n220 = case shown="True" w268 {
                      tunnel: w264 -> [w269 w271]
                      tunnel: [w269 w270] -> w262
                      frame False {
                      }
                      frame True {
                        n221 = Increment(x=w271) -> (x+1=w270:dbl)
                      }
                    }
                    n222 = Multiply(x=w262, y=w265) -> (x*y=w266:dbl)
                    n223 = Divide(x=w266, y=60.0) -> (x/y=w261:dbl)
                    n224 = Bundle(cluster=w263, "CYCLE"=w262, "MINS"=w261) -> (w260:T4)  [unwired: 1 in]
                    n225 = local write "DISP LAB01-1"(w260) -> ()
                  }
                  frame #1 {
                    # "update cycle value"
                    # "LAB01-2"
                    n226 = local read "DISP LAB01-2"() -> (w275:T4)
                    n227 = Unbundle(w275) -> ("CYCLE"=w276:dbl)  [unwired: 2 out]
                    n228 = case shown="True" w280 {
                      tunnel: w276 -> [w281 w283]
                      tunnel: [w281 w282] -> w273
                      frame False {
                      }
                      frame True {
                        n229 = Increment(x=w283) -> (x+1=w282:dbl)
                      }
                    }
                    n230 = Multiply(x=w273, y=w277) -> (x*y=w278:dbl)
                    n231 = Divide(x=w278, y=60.0) -> (x/y=w272:dbl)
                    n232 = Bundle(cluster=w275, "CYCLE"=w273, "MINS"=w272) -> (w274:T4)  [unwired: 1 in]
                    n233 = local write "DISP LAB01-2"(w274) -> ()
                  }
                  frame #2 {
                    # "update cycle value"
                    # "LAB02-1"
                    n234 = local read "DISP LAB02-1"() -> (w287:T4)
                    n235 = Unbundle(w287) -> ("CYCLE"=w288:dbl)  [unwired: 2 out]
                    n236 = case shown="True" w292 {
                      tunnel: [w293 w295] -> w285
                      tunnel: w288 -> [w293 w294]
                      frame False {
                      }
                      frame True {
                        n237 = Increment(x=w294) -> (x+1=w295:dbl)
                      }
                    }
                    n238 = Multiply(x=w285, y=w289) -> (x*y=w290:dbl)
                    n239 = Divide(x=w290, y=60.0) -> (x/y=w284:dbl)
                    n240 = Bundle(cluster=w287, "CYCLE"=w285, "MINS"=w284) -> (w286:T4)  [unwired: 1 in]
                    n241 = local write "DISP LAB02-1"(w286) -> ()
                  }
                  frame #3 {
                    # "update cycle value"
                    # "LAB02-2"
                    n242 = local read "DISP LAB02-2"() -> (w299:T4)
                    n243 = Unbundle(w299) -> ("CYCLE"=w300:dbl)  [unwired: 2 out]
                    n244 = case shown="True" w304 {
                      tunnel: [w305 w307] -> w298
                      tunnel: w300 -> [w305 w306]
                      frame False {
                      }
                      frame True {
                        n245 = Increment(x=w306) -> (x+1=w307:dbl)
                      }
                    }
                    n246 = Multiply(x=w298, y=w301) -> (x*y=w302:dbl)
                    n247 = Divide(x=w302, y=60.0) -> (x/y=w297:dbl)
                    n248 = Bundle(cluster=w299, "CYCLE"=w298, "MINS"=w297) -> (w296:T4)  [unwired: 1 in]
                    n249 = local write "DISP LAB02-2"(w296) -> ()
                  }
                  frame #4 {
                    # "update cycle value"
                    # "LAB03-1"
                    n250 = local read "DISP LAB03-1"() -> (w311:T4)
                    n251 = Unbundle(w311) -> ("CYCLE"=w312:dbl)  [unwired: 2 out]
                    n252 = case shown="True" w316 {
                      tunnel: [w317 w319] -> w308
                      tunnel: w312 -> [w317 w318]
                      frame False {
                      }
                      frame True {
                        n253 = Increment(x=w318) -> (x+1=w319:dbl)
                      }
                    }
                    n254 = Multiply(x=w308, y=w313) -> (x*y=w314:dbl)
                    n255 = Divide(x=w314, y=60.0) -> (x/y=w309:dbl)
                    n256 = Bundle(cluster=w311, "CYCLE"=w308, "MINS"=w309) -> (w310:T4)  [unwired: 1 in]
                    n257 = local write "DISP LAB03-1"(w310) -> ()
                  }
                  frame #5 {
                    # "update cycle value"
                    # "LAB03-2"
                    n258 = local read "DISP LAB03-2"() -> (w323:T4)
                    n259 = Unbundle(w323) -> ("CYCLE"=w324:dbl)  [unwired: 2 out]
                    n260 = case shown="False" w328 {
                      tunnel: [w329 w331] -> w322
                      tunnel: w324 -> [w329 w330]
                      frame False {
                      }
                      frame True {
                        n261 = Increment(x=w330) -> (x+1=w331:dbl)
                      }
                    }
                    n262 = Multiply(x=w322, y=w325) -> (x*y=w326:dbl)
                    n263 = Divide(x=w326, y=60.0) -> (x/y=w321:dbl)
                    n264 = Bundle(cluster=w323, "CYCLE"=w322, "MINS"=w321) -> (w320:T4)  [unwired: 1 in]
                    n265 = local write "DISP LAB03-2"(w320) -> ()
                  }
                  frame #6 {
                    # "update cycle value"
                    # "LAB04-1"
                    n266 = local read "DISP LAB04-1"() -> (w335:T4)
                    n267 = Unbundle(w335) -> ("CYCLE"=w336:dbl)  [unwired: 2 out]
                    n268 = case shown="True" w340 {
                      tunnel: [w341 w343] -> w333
                      tunnel: w336 -> [w341 w342]
                      frame False {
                      }
                      frame True {
                        n269 = Increment(x=w342) -> (x+1=w343:dbl)
                      }
                    }
                    n270 = Multiply(x=w333, y=w337) -> (x*y=w338:dbl)
                    n271 = Divide(x=w338, y=60.0) -> (x/y=w332:dbl)
                    n272 = Bundle(cluster=w335, "CYCLE"=w333, "MINS"=w332) -> (w334:T4)  [unwired: 1 in]
                    n273 = local write "DISP LAB04-1"(w334) -> ()
                  }
                  frame #7 {
                    # "update cycle value"
                    # "LAB04-2"
                    n274 = local read "DISP LAB04-2"() -> (w347:T4)
                    n275 = Unbundle(w347) -> ("CYCLE"=w348:dbl)  [unwired: 2 out]
                    n276 = case shown="True" w352 {
                      tunnel: [w353 w355] -> w345
                      tunnel: w348 -> [w353 w354]
                      frame False {
                      }
                      frame True {
                        n277 = Increment(x=w354) -> (x+1=w355:dbl)
                      }
                    }
                    n278 = Multiply(x=w345, y=w349) -> (x*y=w351:dbl)
                    n279 = Divide(x=w351, y=60.0) -> (x/y=w344:dbl)
                    n280 = Bundle(cluster=w347, "CYCLE"=w345, "MINS"=w344) -> (w346:T4)  [unwired: 1 in]
                    n281 = local write "DISP LAB04-2"(w346) -> ()
                  }
                  frame #8 {
                    # "update cycle value"
                    # "LAB05-1"
                    n282 = local read "DISP LAB05-1"() -> (w359:T4)
                    n283 = Unbundle(w359) -> ("CYCLE"=w360:dbl)  [unwired: 2 out]
                    n284 = case shown="True" w364 {
                      tunnel: [w365 w367] -> w357
                      tunnel: w360 -> [w365 w366]
                      frame False {
                      }
                      frame True {
                        n285 = Increment(x=w366) -> (x+1=w367:dbl)
                      }
                    }
                    n286 = Multiply(x=w357, y=w361) -> (x*y=w362:dbl)
                    n287 = Divide(x=w362, y=60.0) -> (x/y=w356:dbl)
                    n288 = Bundle(cluster=w359, "CYCLE"=w357, "MINS"=w356) -> (w358:T4)  [unwired: 1 in]
                    n289 = local write "DISP LAB05-1"(w358) -> ()
                  }
                  frame #9 {
                    # "update cycle value"
                    # "LAB05-2"
                    n290 = local read "DISP LAB05-2"() -> (w372:T4)
                    n291 = Unbundle(w372) -> ("CYCLE"=w371:dbl)  [unwired: 2 out]
                    n292 = case shown="True" w376 {
                      tunnel: [w377 w379] -> w370
                      tunnel: w371 -> [w377 w378]
                      frame False {
                      }
                      frame True {
                        n293 = Increment(x=w378) -> (x+1=w379:dbl)
                      }
                    }
                    n294 = Multiply(x=w370, y=w373) -> (x*y=w374:dbl)
                    n295 = Divide(x=w374, y=60.0) -> (x/y=w369:dbl)
                    n296 = Bundle(cluster=w372, "CYCLE"=w370, "MINS"=w369) -> (w368:T4)  [unwired: 1 in]
                    n297 = local write "DISP LAB05-2"(w368) -> ()
                  }
                }
                n298 = local write "jig cycle"(0) -> ()
              }
            }
          }
          frame #3 {
            # "START & STOP test RUN switch change, start test if true and stop test if false"
            n299 = Get Date/Time In Seconds() -> (seconds since 1Jan1904=w387:timestamp)
            n300 = local read "C drive data root dir"() -> (w380:path)
            n301 = Format Date/Time String(time format string (%c)="%b\\%a%d", seconds (now)=w387) -> (date/time string=w411:string)  [unwired: 1 in]
            n302 = Format Date/Time String(time format string (%c)="%H%M", seconds (now)=w387) -> (date/time string=w409:string)  [unwired: 1 in]
            n303 = Format Date/Time String(time format string (%c)="LabPanel%Y", seconds (now)=w387) -> (date/time string=w386:string)  [unwired: 1 in]
            n304 = Path To String(path=w380) -> (string=w383:string)
            n305 = global write "Global 1.vi" "C drive root path"(w380) -> ()
            n306 = Concatenate Strings(w383, "\\") -> (w381:string)
            n307 = event shown="[2] \"RUN LAB01-2\": Value Change" {
              selector: _ -> [_ _ _ _ _ _ _ _ _ _ _]
              dyn-events: _ -> [_ _ _ _ _ _ _ _ _ _ _]
              timeout: 10 -> [_ _ _ _ _ _ _ _ _ _ _]
              tunnel: w381 -> [_ w419 w511 w603 w695 w787 w879 w971 w1063 w1155 w1247]
              tunnel: w411 -> [_ w418 w510 w602 w694 w786 w878 w970 w1062 w1154 w1246]
              tunnel: w409 -> [_ w416 w509 w601 w693 w785 w877 w969 w1061 w1153 w1245]
              tunnel: w407 -> [_ w417 _ _ _ _ _ _ _ _ _]
              tunnel: w408 -> [_ _ _ _ _ _ _ _ _ _ _]
              tunnel: w406 -> [_ _ _ _ _ _ _ _ _ _ _]
              tunnel: w405 -> [_ _ w508 _ _ _ _ _ _ _ _]
              tunnel: w404 -> [_ _ _ _ _ _ _ _ _ _ _]
              tunnel: w403 -> [_ _ _ w600 _ _ _ _ _ _ _]
              tunnel: w402 -> [_ _ _ _ _ _ _ _ _ _ _]
              tunnel: w401 -> [_ _ _ _ w692 _ _ _ _ _ _]
              tunnel: w400 -> [_ _ _ _ _ _ _ _ _ _ _]
              tunnel: w399 -> [_ _ _ _ _ w784 _ _ _ _ _]
              tunnel: w398 -> [_ _ _ _ _ _ _ _ _ _ _]
              tunnel: w397 -> [_ _ _ _ _ _ w876 _ _ _ _]
              tunnel: w396 -> [_ _ _ _ _ _ _ _ _ _ _]
              tunnel: w395 -> [_ _ _ _ _ _ _ w968 _ _ _]
              tunnel: w394 -> [_ _ _ _ _ _ _ _ _ _ _]
              tunnel: w393 -> [_ _ _ _ _ _ _ _ w1060 _ _]
              tunnel: w392 -> [_ _ _ _ _ _ _ _ _ _ _]
              tunnel: w391 -> [_ _ _ _ _ _ _ _ _ w1152 _]
              tunnel: w390 -> [_ _ _ _ _ _ _ _ _ _ _]
              tunnel: w389 -> [_ _ _ _ _ _ _ _ _ _ w1244]
              tunnel: w386 -> [_ w415 w507 w599 w691 w783 w875 w967 w1059 w1151 w1243]
              tunnel: [_ w414 w506 w598 w690 w782 w874 w966 w1058 w1150 w1242] -> w384
              event Timeout {
                n308 = event-data() -> ()  [unwired: 1 in, 3 out]
              }
              event "RUN LAB01-1": Value Change {
                n309 = event-data() -> ("NewVal"=w413:bool)  [unwired: 1 in, 5 out]
                n310 = local write "run lab01-1"(w413) -> ()
                n311 = case shown="True" w413 {
                  tunnel: w419 -> [_ w452]
                  tunnel: w418 -> [_ w451]
                  tunnel: w417 -> [w421 w450]
                  tunnel: w416 -> [_ w449]
                  tunnel: w415 -> [_ w448]
                  tunnel: [w420 w447] -> w414
                  frame False {
                    # "stop test"
                    n312 = stacked-sequence {
                      tunnel: w421 -> [_ w433 _ _]
                      tunnel: [_ w425 _ _] -> w420
                      frame #0 {
                        n313 = local read "DISP LAB01-1"() -> (w424:T4)
                        n314 = Bundle(cluster=w424, "STATUS"="STOP") -> (w422:T4)  [unwired: 2 in]
                        n315 = local write "DISP LAB01-1"(w422) -> ()
                      }
                      frame #1 {
                        n316 = local read "DISP LAB01-1"() -> (w432:T4)
                        n317 = Unbundle(w432) -> ("CYCLE"=w430:dbl, "MINS"=w431:dbl)  [unwired: 1 out]
                        n318 = case shown="\"CYCLE TEST\"" w433 {
                          tunnel: w431 -> [_ _ w440]
                          tunnel: w430 -> [w438 w439 _]
                          tunnel: [w438 w439 w440] -> w429
                          frame "CHART TEST", Default {
                          }
                          frame "CYCLE TEST" {
                          }
                          frame "T-RISE TEST" {
                          }
                        }
                        n319 = local read "TDMS LAB01-1"() -> (w437:refnum<k34>)
                        n320 = Build Array("STOPPED") -> (w434:string[])
                        n321 = Build Array(w429) -> (w428:dbl[])
                        n322 = TDMS Write(0:w437, 5:"TEST RESULT", 7:w434, 9:w428) -> (4:w426:refnum<k34>, 15:w427:errorcluster)  [unwired: 2 in, 2 out]
                        n323 = TDMS Close(8:w427, 11:w426) -> (0:w425:errorcluster)  [unwired: 1 out]
                      }
                      frame #2 {
                        n324 = stacked-sequence {
                          tunnel: "LAB01-1" -> [w443 w445]
                          frame #0 {
                            n325 = call "sub vi - defrag tdms v1.vi"("panel id"=w443) -> ("error out"=w442:errorcluster)  [unwired: 10 in]
                            n326 = local write "data file error"(w442) -> ()
                          }
                          frame #1 {
                            n327 = call "Save data file to network drive v1.vi"("panel id"=w445) -> ("network file save error"=w444:errorcluster)  [unwired: 9 in, 1 out]
                            n328 = local write "RESULT LAB01-1"(FALSE) -> ()
                            n329 = local write "data file error"(w444) -> ()
                          }
                        }
                      }
                      frame #3 {
                      }
                    }
                  }
                  frame True {
                    # "start new test and create test file"
                    n330 = stacked-sequence {
                      seq-local: [w453 _ _ _ _] -> [_ w474 _ _ _]
                      tunnel: w452 -> [w458 _ _ _ _]
                      tunnel: w451 -> [w454 _ _ _ _]
                      tunnel: w450 -> [w468 _ _ _ _]
                      tunnel: w449 -> [w461 _ _ _ _]
                      tunnel: w448 -> [w456 _ _ _ _]
                      tunnel: [_ w475 _ _ _] -> w447
                      frame #0 {
                        w455 = "\\"
                        n331 = case shown="\"CHART TEST\", Default" w468 {
                          tunnel: ["L01-1-CHART TEST-" "L01-1-CYCLE TEST-" "L01-1-T-RISE TEST-"] -> w464
                          frame "CHART TEST", Default {
                          }
                          frame "CYCLE TEST" {
                          }
                          frame "T-RISE TEST" {
                          }
                        }
                        n332 = local read "SET LAB01-1"() -> (w463:T5)
                        n333 = Unbundle(w463) -> ("DESCRIPTION"=w462:string)  [unwired: 4 out]
                        n334 = Concatenate Strings(w458, "\\", w456, w455, w454, w455) -> (w465:string)
                        n335 = String To Path(string=w465) -> (path=w467:path)
                        n336 = Concatenate Strings(w465, w464, w462, "-", w461, ".tdms") -> (w453:string)
                        n337 = Create Folder(path (use dialog)=w467) -> (error out=w466:errorcluster)  [unwired: 2 in, 2 out]
                        n338 = call <vilib>:"Clear Errors.vi"("error in (no error)"=w466) -> ()  [unwired: 6 in, 1 out]
                        n339 = global write "Global 1.vi" "LAB01-1 FILE"(w453) -> ()
                      }
                      frame #1 {
                        n340 = String To Path(string=w474) -> (path=w472:path)
                        n341 = TDMS Open(5:FALSE, 6:FALSE, 10:T15."create or replace" ("operation (0:open)"), 11:w472) -> (0:w475:errorcluster, 3:→"TDMS LAB01-1":refnum<k34>)  [unwired: 3 in]
                      }
                      frame #2 {
                        n342 = local read "TDMS LAB01-1"() -> (w495:refnum<k34>)
                        n343 = local read "SET LAB01-1"() -> (w484:T5)
                        n344 = Build Array("Testers Name", "Description", "Set Test Cycles", "T-Rise minutes", "T-Rise Deg C") -> (w485:string[])
                        n345 = Unbundle(w484) -> ("NAME"=w483:string, "DESCRIPTION"=w482:string, "CYCLES"=w481:dbl, "T-RISE mins"=w480:dbl, "T-RISE deg C"=w479:dbl)
                        n346 = Number To Decimal String(number=w481) -> (decimal integer string=w494:string)  [unwired: 1 in]
                        n347 = Number To Decimal String(number=w480) -> (decimal integer string=w493:string)  [unwired: 1 in]
                        n348 = Number To Decimal String(number=w479) -> (decimal integer string=w492:string)  [unwired: 1 in]
                        n349 = Build Array(w483, w482, w494, w493, w492) -> (w491:string[])
                        n350 = TDMS Set Properties(5:w491, 7:w485, 11:w495) -> ()  [unwired: 3 in, 4 out]
                      }
                      frame #3 {
                        w496 = 0.0
                        n351 = local read "DISP LAB01-1"() -> (w499:T4)
                        n352 = Bundle(cluster=w499, "CYCLE"=w496, "MINS"=w496, "STATUS"="RUN") -> (w498:T4)
                        n353 = local write "DISP LAB01-1"(w498) -> ()
                      }
                      frame #4 {
                        n354 = local read "SIG LAB01-1"() -> (w502:T2)
                        n355 = local read "TEMP START LAB01-1"() -> (w504:cluster{"TL":dbl, "TN":dbl})
                        n356 = Unbundle(w502) -> ("Tmp Live"=w501:dbl, "Tmp Neut"=w500:dbl)  [unwired: 3 out]
                        n357 = Bundle(cluster=w504, "TL"=w501, "TN"=w500) -> (w503:cluster{"TL":dbl, "TN":dbl})
                        n358 = local write "TEMP START LAB01-1"(w503) -> ()
                      }
                    }
                  }
                }
              }
              event "RUN LAB01-2": Value Change {
                n359 = event-data() -> ("NewVal"=w505:bool)  [unwired: 1 in, 5 out]
                n360 = local write "run lab01-2"(w505) -> ()
                n361 = case shown="True" w505 {
                  tunnel: w511 -> [_ w544]
                  tunnel: w510 -> [_ w543]
                  tunnel: w508 -> [w513 w542]
                  tunnel: w509 -> [_ w541]
                  tunnel: w507 -> [_ w540]
                  tunnel: [w512 w539] -> w506
                  frame False {
                    # "stop test"
                    n362 = stacked-sequence {
                      tunnel: w513 -> [w522 _]
                      tunnel: [w514 _] -> w512
                      frame #0 {
                        n363 = local read "DISP LAB01-2"() -> (w521:T4)
                        n364 = Unbundle(w521) -> ("CYCLE"=w519:dbl, "MINS"=w520:dbl)  [unwired: 1 out]
                        n365 = case shown="\"CHART TEST\", Default" w522 {
                          tunnel: w520 -> [_ _ w529]
                          tunnel: w519 -> [w527 w528 _]
                          tunnel: [w527 w528 w529] -> w518
                          frame "CHART TEST", Default {
                          }
                          frame "CYCLE TEST" {
                          }
                          frame "T-RISE TEST" {
                          }
                        }
                        n366 = local read "TDMS LAB01-2"() -> (w526:refnum<k34>)
                        n367 = Build Array("STOPPED") -> (w523:string[])
                        n368 = Build Array(w518) -> (w517:dbl[])
                        n369 = TDMS Write(0:w526, 5:"TEST RESULT", 7:w523, 9:w517) -> (4:w515:refnum<k34>, 15:w516:errorcluster)  [unwired: 2 in, 2 out]
                        n370 = TDMS Close(8:w516, 11:w515) -> (0:w514:errorcluster)  [unwired: 1 out]
                      }
                      frame #1 {
                        n371 = local read "DISP LAB01-2"() -> (w533:T4)
                        n372 = stacked-sequence {
                          tunnel: "LAB01-2" -> [w535 w537]
                          frame #0 {
                            n373 = call "sub vi - defrag tdms v1.vi"("panel id"=w535) -> ("error out"=w534:errorcluster)  [unwired: 10 in]
                            n374 = local write "data file error"(w534) -> ()
                          }
                          frame #1 {
                            n375 = call "Save data file to network drive v1.vi"("panel id"=w537) -> ("network file save error"=w536:errorcluster)  [unwired: 9 in, 1 out]
                            n376 = local write "RESULT LAB01-2"(FALSE) -> ()
                            n377 = local write "data file error"(w536) -> ()
                          }
                        }
                        n378 = Bundle(cluster=w533, "STATUS"="STOP") -> (w531:T4)  [unwired: 2 in]
                        n379 = local write "DISP LAB01-2"(w531) -> ()
                      }
                    }
                  }
                  frame True {
                    # "start new test and create test file"
                    n380 = stacked-sequence {
                      seq-local: [w545 _ _ _ _] -> [_ w570 _ _ _]
                      tunnel: w544 -> [w550 _ _ _ _]
                      tunnel: w543 -> [w547 _ _ _ _]
                      tunnel: w542 -> [w560 _ _ _ _]
                      tunnel: w541 -> [w553 _ _ _ _]
                      tunnel: w540 -> [w548 _ _ _ _]
                      tunnel: [_ w564 _ _ _] -> w539
                      frame #0 {
                        w546 = "\\"
                        n381 = local read "SET LAB01-2"() -> (w555:T5)
                        n382 = case shown="\"CYCLE TEST\"" w560 {
                          tunnel: ["L01-2-CHART TEST-" "L01-2-CYCLE TEST-" "L01-2-T-RISE TEST-"] -> w556
                          frame "CHART TEST", Default {
                          }
                          frame "CYCLE TEST" {
                          }
                          frame "T-RISE TEST" {
                          }
                        }
                        n383 = Unbundle(w555) -> ("DESCRIPTION"=w554:string)  [unwired: 4 out]
                        n384 = Concatenate Strings(w550, "\\", w548, w546, w547, w546) -> (w557:string)
                        n385 = String To Path(string=w557) -> (path=w559:path)
                        n386 = Concatenate Strings(w557, w556, w554, "-", w553, ".tdms") -> (w545:string)
                        n387 = Create Folder(path (use dialog)=w559) -> (error out=w558:errorcluster)  [unwired: 2 in, 2 out]
                        n388 = global write "Global 1.vi" "LAB01-2 FILE"(w545) -> ()
                        n389 = call <vilib>:"Clear Errors.vi"("error in (no error)"=w558) -> ()  [unwired: 6 in, 1 out]
                      }
                      frame #1 {
                        n390 = String To Path(string=w570) -> (path=w565:path)
                        n391 = TDMS Open(5:FALSE, 6:FALSE, 10:T15."create or replace" ("operation (0:open)"), 11:w565) -> (0:w564:errorcluster, 3:→"TDMS LAB01-2":refnum<k34>)  [unwired: 3 in]
                      }
                      frame #2 {
                        n392 = local read "SET LAB01-2"() -> (w576:T5)
                        n393 = local read "TDMS LAB01-2"() -> (w587:refnum<k34>)
                        n394 = Build Array("Testers Name", "Description", "Set Test Cycles", "T-Rise minutes", "T-Rise Deg C") -> (w577:string[])
                        n395 = Unbundle(w576) -> ("NAME"=w575:string, "DESCRIPTION"=w574:string, "CYCLES"=w573:dbl, "T-RISE mins"=w572:dbl, "T-RISE deg C"=w571:dbl)
                        n396 = Number To Decimal String(number=w573) -> (decimal integer string=w586:string)  [unwired: 1 in]
                        n397 = Number To Decimal String(number=w572) -> (decimal integer string=w585:string)  [unwired: 1 in]
                        n398 = Number To Decimal String(number=w571) -> (decimal integer string=w584:string)  [unwired: 1 in]
                        n399 = Build Array(w575, w574, w586, w585, w584) -> (w583:string[])
                        n400 = TDMS Set Properties(5:w583, 7:w577, 11:w587) -> ()  [unwired: 3 in, 4 out]
                      }
                      frame #3 {
                        w589 = 0.0
                        n401 = local read "DISP LAB01-2"() -> (w591:T4)
                        n402 = Bundle(cluster=w591, "CYCLE"=w589, "MINS"=w589, "STATUS"="RUN") -> (w590:T4)
                        n403 = local write "DISP LAB01-2"(w590) -> ()
                      }
                      frame #4 {
                        n404 = local read "SIG LAB01-2"() -> (w594:T2)
                        n405 = local read "TEMP START LAB01-2"() -> (w596:cluster{"TL":dbl, "TN":dbl})
                        n406 = Unbundle(w594) -> ("Tmp Live"=w593:dbl, "Tmp Neut"=w592:dbl)  [unwired: 3 out]
                        n407 = Bundle(cluster=w596, "TL"=w593, "TN"=w592) -> (w595:cluster{"TL":dbl, "TN":dbl})
                        n408 = local write "TEMP START LAB01-2"(w595) -> ()
                      }
                    }
                  }
                }
              }
              event "RUN LAB02-1": Value Change {
                n409 = event-data() -> ("NewVal"=w597:bool)  [unwired: 1 in, 5 out]
                n410 = local write "run lab02-1"(w597) -> ()
                n411 = case shown="True" w597 {
                  tunnel: w603 -> [_ w636]
                  tunnel: w602 -> [_ w635]
                  tunnel: w600 -> [w605 w634]
                  tunnel: w601 -> [_ w633]
                  tunnel: w599 -> [_ w632]
                  tunnel: [w604 w631] -> w598
                  frame False {
                    # "stop test"
                    n412 = stacked-sequence {
                      tunnel: w605 -> [w614 _]
                      tunnel: [w606 _] -> w604
                      frame #0 {
                        n413 = local read "DISP LAB02-1"() -> (w613:T4)
                        n414 = Unbundle(w613) -> ("CYCLE"=w611:dbl, "MINS"=w612:dbl)  [unwired: 1 out]
                        n415 = case shown="\"CYCLE TEST\"" w614 {
                          tunnel: w612 -> [_ _ w621]
                          tunnel: w611 -> [w619 w620 _]
                          tunnel: [w619 w620 w621] -> w610
                          frame "CHART TEST", Default {
                          }
                          frame "CYCLE TEST" {
                          }
                          frame "T-RISE TEST" {
                          }
                        }
                        n416 = local read "TDMS LAB02-1"() -> (w618:refnum<k34>)
                        n417 = Build Array("STOPPED") -> (w615:string[])
                        n418 = Build Array(w610) -> (w609:dbl[])
                        n419 = TDMS Write(0:w618, 5:"TEST RESULT", 7:w615, 9:w609) -> (4:w607:refnum<k34>, 15:w608:errorcluster)  [unwired: 2 in, 2 out]
                        n420 = TDMS Close(8:w608, 11:w607) -> (0:w606:errorcluster)  [unwired: 1 out]
                      }
                      frame #1 {
                        n421 = local read "DISP LAB02-1"() -> (w625:T4)
                        n422 = stacked-sequence {
                          tunnel: "LAB02-1" -> [w627 w629]
                          frame #0 {
                            n423 = call "sub vi - defrag tdms v1.vi"("panel id"=w627) -> ("error out"=w626:errorcluster)  [unwired: 10 in]
                            n424 = local write "data file error"(w626) -> ()
                          }
                          frame #1 {
                            n425 = local write "RESULT LAB02-1"(FALSE) -> ()
                            n426 = call "Save data file to network drive v1.vi"("panel id"=w629) -> ("network file save error"=w628:errorcluster)  [unwired: 9 in, 1 out]
                            n427 = local write "data file error"(w628) -> ()
                          }
                        }
                        n428 = Bundle(cluster=w625, "STATUS"="STOP") -> (w623:T4)  [unwired: 2 in]
                        n429 = local write "DISP LAB02-1"(w623) -> ()
                      }
                    }
                  }
                  frame True {
                    # "start new test and create test file"
                    n430 = stacked-sequence {
                      seq-local: [w637 _ _ _ _] -> [_ w662 _ _ _]
                      tunnel: w636 -> [w642 _ _ _ _]
                      tunnel: w635 -> [w639 _ _ _ _]
                      tunnel: w634 -> [w652 _ _ _ _]
                      tunnel: w633 -> [w645 _ _ _ _]
                      tunnel: w632 -> [w640 _ _ _ _]
                      tunnel: [_ w656 _ _ _] -> w631
                      frame #0 {
                        w638 = "\\"
                        n431 = local read "SET LAB02-1"() -> (w647:T5)
                        n432 = case shown="\"CYCLE TEST\"" w652 {
                          tunnel: ["L02-1-CHART TEST-" "L02-1-CYCLE TEST-" "L02-1-T-RISE TEST-"] -> w648
                          frame "CHART TEST", Default {
                          }
                          frame "CYCLE TEST" {
                          }
                          frame "T-RISE TEST" {
                          }
                        }
                        n433 = Unbundle(w647) -> ("DESCRIPTION"=w646:string)  [unwired: 4 out]
                        n434 = Concatenate Strings(w642, "\\", w640, w638, w639, w638) -> (w649:string)
                        n435 = String To Path(string=w649) -> (path=w651:path)
                        n436 = Concatenate Strings(w649, w648, w646, "-", w645, ".tdms") -> (w637:string)
                        n437 = Create Folder(path (use dialog)=w651) -> (error out=w650:errorcluster)  [unwired: 2 in, 2 out]
                        n438 = global write "Global 1.vi" "LAB02-1 FILE"(w637) -> ()
                        n439 = call <vilib>:"Clear Errors.vi"("error in (no error)"=w650) -> ()  [unwired: 6 in, 1 out]
                      }
                      frame #1 {
                        n440 = String To Path(string=w662) -> (path=w657:path)
                        n441 = TDMS Open(5:FALSE, 6:FALSE, 10:T15."create or replace" ("operation (0:open)"), 11:w657) -> (0:w656:errorcluster, 3:→"TDMS LAB02-1":refnum<k34>)  [unwired: 3 in]
                      }
                      frame #2 {
                        n442 = local read "SET LAB02-1"() -> (w668:T5)
                        n443 = local read "TDMS LAB02-1"() -> (w679:refnum<k34>)
                        n444 = Build Array("Testers Name", "Description", "Set Test Cycles", "T-Rise minutes", "T-Rise Deg C") -> (w669:string[])
                        n445 = Unbundle(w668) -> ("NAME"=w667:string, "DESCRIPTION"=w666:string, "CYCLES"=w665:dbl, "T-RISE mins"=w664:dbl, "T-RISE deg C"=w663:dbl)
                        n446 = Number To Decimal String(number=w665) -> (decimal integer string=w678:string)  [unwired: 1 in]
                        n447 = Number To Decimal String(number=w664) -> (decimal integer string=w677:string)  [unwired: 1 in]
                        n448 = Number To Decimal String(number=w663) -> (decimal integer string=w676:string)  [unwired: 1 in]
                        n449 = Build Array(w667, w666, w678, w677, w676) -> (w675:string[])
                        n450 = TDMS Set Properties(5:w675, 7:w669, 11:w679) -> ()  [unwired: 3 in, 4 out]
                      }
                      frame #3 {
                        w681 = 0.0
                        n451 = local read "DISP LAB02-1"() -> (w683:T4)
                        n452 = Bundle(cluster=w683, "CYCLE"=w681, "MINS"=w681, "STATUS"="RUN") -> (w682:T4)
                        n453 = local write "DISP LAB02-1"(w682) -> ()
                      }
                      frame #4 {
                        n454 = local read "SIG LAB02-1"() -> (w686:T2)
                        n455 = local read "TEMP START LAB02-1"() -> (w688:cluster{"TL":dbl, "TN":dbl})
                        n456 = Unbundle(w686) -> ("Tmp Live"=w685:dbl, "Tmp Neut"=w684:dbl)  [unwired: 3 out]
                        n457 = Bundle(cluster=w688, "TL"=w685, "TN"=w684) -> (w687:cluster{"TL":dbl, "TN":dbl})
                        n458 = local write "TEMP START LAB02-1"(w687) -> ()
                      }
                    }
                  }
                }
              }
              event "RUN LAB02-2": Value Change {
                n459 = event-data() -> ("NewVal"=w689:bool)  [unwired: 1 in, 5 out]
                n460 = local write "run lab02-2"(w689) -> ()
                n461 = case shown="True" w689 {
                  tunnel: w695 -> [_ w728]
                  tunnel: w694 -> [_ w727]
                  tunnel: w692 -> [w697 w726]
                  tunnel: w693 -> [_ w725]
                  tunnel: w691 -> [_ w724]
                  tunnel: [w696 w723] -> w690
                  frame False {
                    # "stop test"
                    n462 = stacked-sequence {
                      tunnel: w697 -> [w706 _]
                      tunnel: [w698 _] -> w696
                      frame #0 {
                        n463 = local read "DISP LAB02-2"() -> (w705:T4)
                        n464 = Unbundle(w705) -> ("CYCLE"=w703:dbl, "MINS"=w704:dbl)  [unwired: 1 out]
                        n465 = case shown="\"CYCLE TEST\"" w706 {
                          tunnel: w704 -> [_ _ w713]
                          tunnel: w703 -> [w711 w712 _]
                          tunnel: [w711 w712 w713] -> w702
                          frame "CHART TEST", Default {
                          }
                          frame "CYCLE TEST" {
                          }
                          frame "T-RISE TEST" {
                          }
                        }
                        n466 = local read "TDMS LAB02-2"() -> (w710:refnum<k34>)
                        n467 = Build Array("STOPPED") -> (w707:string[])
                        n468 = Build Array(w702) -> (w701:dbl[])
                        n469 = TDMS Write(0:w710, 5:"TEST RESULT", 7:w707, 9:w701) -> (4:w699:refnum<k34>, 15:w700:errorcluster)  [unwired: 2 in, 2 out]
                        n470 = TDMS Close(8:w700, 11:w699) -> (0:w698:errorcluster)  [unwired: 1 out]
                      }
                      frame #1 {
                        n471 = local read "DISP LAB02-2"() -> (w717:T4)
                        n472 = stacked-sequence {
                          tunnel: "LAB02-2" -> [w719 w721]
                          frame #0 {
                            n473 = call "sub vi - defrag tdms v1.vi"("panel id"=w719) -> ("error out"=w718:errorcluster)  [unwired: 10 in]
                            n474 = local write "data file error"(w718) -> ()
                          }
                          frame #1 {
                            n475 = call "Save data file to network drive v1.vi"("panel id"=w721) -> ("network file save error"=w720:errorcluster)  [unwired: 9 in, 1 out]
                            n476 = local write "RESULT LAB02-2"(FALSE) -> ()
                            n477 = local write "data file error"(w720) -> ()
                          }
                        }
                        n478 = Bundle(cluster=w717, "STATUS"="STOP") -> (w715:T4)  [unwired: 2 in]
                        n479 = local write "DISP LAB02-2"(w715) -> ()
                      }
                    }
                  }
                  frame True {
                    # "start new test and create test file"
                    n480 = stacked-sequence {
                      seq-local: [w729 _ _ _ _] -> [_ w754 _ _ _]
                      tunnel: w728 -> [w734 _ _ _ _]
                      tunnel: w727 -> [w731 _ _ _ _]
                      tunnel: w726 -> [w744 _ _ _ _]
                      tunnel: w725 -> [w737 _ _ _ _]
                      tunnel: w724 -> [w732 _ _ _ _]
                      tunnel: [_ w748 _ _ _] -> w723
                      frame #0 {
                        w730 = "\\"
                        n481 = local read "SET LAB02-2"() -> (w739:T5)
                        n482 = case shown="\"CYCLE TEST\"" w744 {
                          tunnel: ["L02-2-CHART TEST-" "L02-2-CYCLE TEST-" "L02-2-T-RISE TEST-"] -> w740
                          frame "CHART TEST", Default {
                          }
                          frame "CYCLE TEST" {
                          }
                          frame "T-RISE TEST" {
                          }
                        }
                        n483 = Unbundle(w739) -> ("DESCRIPTION"=w738:string)  [unwired: 4 out]
                        n484 = Concatenate Strings(w734, "\\", w732, w730, w731, w730) -> (w741:string)
                        n485 = String To Path(string=w741) -> (path=w743:path)
                        n486 = Concatenate Strings(w741, w740, w738, "-", w737, ".tdms") -> (w729:string)
                        n487 = Create Folder(path (use dialog)=w743) -> (error out=w742:errorcluster)  [unwired: 2 in, 2 out]
                        n488 = global write "Global 1.vi" "LAB02-2 FILE"(w729) -> ()
                        n489 = call <vilib>:"Clear Errors.vi"("error in (no error)"=w742) -> ()  [unwired: 6 in, 1 out]
                      }
                      frame #1 {
                        n490 = String To Path(string=w754) -> (path=w749:path)
                        n491 = TDMS Open(5:FALSE, 6:FALSE, 10:T15."create or replace" ("operation (0:open)"), 11:w749) -> (0:w748:errorcluster, 3:→"TDMS LAB02-2":refnum<k34>)  [unwired: 3 in]
                      }
                      frame #2 {
                        n492 = local read "SET LAB02-2"() -> (w760:T5)
                        n493 = local read "TDMS LAB02-2"() -> (w771:refnum<k34>)
                        n494 = Build Array("Testers Name", "Description", "Set Test Cycles", "T-Rise minutes", "T-Rise Deg C") -> (w761:string[])
                        n495 = Unbundle(w760) -> ("NAME"=w759:string, "DESCRIPTION"=w758:string, "CYCLES"=w757:dbl, "T-RISE mins"=w756:dbl, "T-RISE deg C"=w755:dbl)
                        n496 = Number To Decimal String(number=w757) -> (decimal integer string=w770:string)  [unwired: 1 in]
                        n497 = Number To Decimal String(number=w756) -> (decimal integer string=w769:string)  [unwired: 1 in]
                        n498 = Number To Decimal String(number=w755) -> (decimal integer string=w768:string)  [unwired: 1 in]
                        n499 = Build Array(w759, w758, w770, w769, w768) -> (w767:string[])
                        n500 = TDMS Set Properties(5:w767, 7:w761, 11:w771) -> ()  [unwired: 3 in, 4 out]
                      }
                      frame #3 {
                        w773 = 0.0
                        n501 = local read "DISP LAB02-2"() -> (w775:T4)
                        n502 = Bundle(cluster=w775, "CYCLE"=w773, "MINS"=w773, "STATUS"="RUN") -> (w774:T4)
                        n503 = local write "DISP LAB02-2"(w774) -> ()
                      }
                      frame #4 {
                        n504 = local read "SIG LAB02-2"() -> (w778:T2)
                        n505 = local read "TEMP START LAB02-2"() -> (w780:cluster{"TL":dbl, "TN":dbl})
                        n506 = Unbundle(w778) -> ("Tmp Live"=w777:dbl, "Tmp Neut"=w776:dbl)  [unwired: 3 out]
                        n507 = Bundle(cluster=w780, "TL"=w777, "TN"=w776) -> (w779:cluster{"TL":dbl, "TN":dbl})
                        n508 = local write "TEMP START LAB02-2"(w779) -> ()
                      }
                    }
                  }
                }
              }
              event "RUN LAB03-1": Value Change {
                n509 = event-data() -> ("NewVal"=w781:bool)  [unwired: 1 in, 5 out]
                n510 = local write "run lab03-1"(w781) -> ()
                n511 = case shown="True" w781 {
                  tunnel: w787 -> [_ w820]
                  tunnel: w786 -> [_ w819]
                  tunnel: w784 -> [w789 w818]
                  tunnel: w785 -> [_ w817]
                  tunnel: w783 -> [_ w816]
                  tunnel: [w788 w815] -> w782
                  frame False {
                    # "stop test"
                    n512 = stacked-sequence {
                      tunnel: w789 -> [w798 _]
                      tunnel: [w790 _] -> w788
                      frame #0 {
                        n513 = local read "DISP LAB03-1"() -> (w797:T4)
                        n514 = Unbundle(w797) -> ("CYCLE"=w795:dbl, "MINS"=w796:dbl)  [unwired: 1 out]
                        n515 = case shown="\"CYCLE TEST\"" w798 {
                          tunnel: w796 -> [_ _ w805]
                          tunnel: w795 -> [w803 w804 _]
                          tunnel: [w803 w804 w805] -> w794
                          frame "CHART TEST", Default {
                          }
                          frame "CYCLE TEST" {
                          }
                          frame "T-RISE TEST" {
                          }
                        }
                        n516 = local read "TDMS LAB03-1"() -> (w802:refnum<k34>)
                        n517 = Build Array("STOPPED") -> (w799:string[])
                        n518 = Build Array(w794) -> (w793:dbl[])
                        n519 = TDMS Write(0:w802, 5:"TEST RESULT", 7:w799, 9:w793) -> (4:w791:refnum<k34>, 15:w792:errorcluster)  [unwired: 2 in, 2 out]
                        n520 = TDMS Close(8:w792, 11:w791) -> (0:w790:errorcluster)  [unwired: 1 out]
                      }
                      frame #1 {
                        n521 = local read "DISP LAB03-1"() -> (w809:T4)
                        n522 = stacked-sequence {
                          tunnel: "LAB03-1" -> [w811 w813]
                          frame #0 {
                            n523 = call "sub vi - defrag tdms v1.vi"("panel id"=w811) -> ("error out"=w810:errorcluster)  [unwired: 10 in]
                            n524 = local write "data file error"(w810) -> ()
                          }
                          frame #1 {
                            n525 = call "Save data file to network drive v1.vi"("panel id"=w813) -> ("network file save error"=w812:errorcluster)  [unwired: 9 in, 1 out]
                            n526 = local write "RESULT LAB03-1"(FALSE) -> ()
                            n527 = local write "data file error"(w812) -> ()
                          }
                        }
                        n528 = Bundle(cluster=w809, "STATUS"="STOP") -> (w807:T4)  [unwired: 2 in]
                        n529 = local write "DISP LAB03-1"(w807) -> ()
                      }
                    }
                  }
                  frame True {
                    # "start new test and create test file"
                    n530 = stacked-sequence {
                      seq-local: [w821 _ _ _ _] -> [_ w846 _ _ _]
                      tunnel: w820 -> [w826 _ _ _ _]
                      tunnel: w819 -> [w823 _ _ _ _]
                      tunnel: w818 -> [w836 _ _ _ _]
                      tunnel: w817 -> [w829 _ _ _ _]
                      tunnel: w816 -> [w824 _ _ _ _]
                      tunnel: [_ w840 _ _ _] -> w815
                      frame #0 {
                        w822 = "\\"
                        n531 = local read "SET LAB03-1"() -> (w831:T5)
                        n532 = case shown="\"T-RISE TEST\"" w836 {
                          tunnel: ["L03-1-CHART TEST-" "L03-1-CYCLE TEST-" "L03-1-T-RISE TEST-"] -> w832
                          frame "CHART TEST", Default {
                          }
                          frame "CYCLE TEST" {
                          }
                          frame "T-RISE TEST" {
                          }
                        }
                        n533 = Unbundle(w831) -> ("DESCRIPTION"=w830:string)  [unwired: 4 out]
                        n534 = Concatenate Strings(w826, "\\", w824, w822, w823, w822) -> (w833:string)
                        n535 = String To Path(string=w833) -> (path=w835:path)
                        n536 = Concatenate Strings(w833, w832, w830, "-", w829, ".tdms") -> (w821:string)
                        n537 = Create Folder(path (use dialog)=w835) -> (error out=w834:errorcluster)  [unwired: 2 in, 2 out]
                        n538 = global write "Global 1.vi" "LAB03-1 FILE"(w821) -> ()
                        n539 = call <vilib>:"Clear Errors.vi"("error in (no error)"=w834) -> ()  [unwired: 6 in, 1 out]
                      }
                      frame #1 {
                        n540 = String To Path(string=w846) -> (path=w841:path)
                        n541 = TDMS Open(5:FALSE, 6:FALSE, 10:T15."create or replace" ("operation (0:open)"), 11:w841) -> (0:w840:errorcluster, 3:→"TDMS LAB03-1":refnum<k34>)  [unwired: 3 in]
                      }
                      frame #2 {
                        n542 = local read "SET LAB03-1"() -> (w852:T5)
                        n543 = local read "TDMS LAB03-1"() -> (w863:refnum<k34>)
                        n544 = Build Array("Testers Name", "Description", "Set Test Cycles", "T-Rise minutes", "T-Rise Deg C") -> (w853:string[])
                        n545 = Unbundle(w852) -> ("NAME"=w851:string, "DESCRIPTION"=w850:string, "CYCLES"=w849:dbl, "T-RISE mins"=w848:dbl, "T-RISE deg C"=w847:dbl)
                        n546 = Number To Decimal String(number=w849) -> (decimal integer string=w862:string)  [unwired: 1 in]
                        n547 = Number To Decimal String(number=w848) -> (decimal integer string=w861:string)  [unwired: 1 in]
                        n548 = Number To Decimal String(number=w847) -> (decimal integer string=w860:string)  [unwired: 1 in]
                        n549 = Build Array(w851, w850, w862, w861, w860) -> (w859:string[])
                        n550 = TDMS Set Properties(5:w859, 7:w853, 11:w863) -> ()  [unwired: 3 in, 4 out]
                      }
                      frame #3 {
                        w865 = 0.0
                        n551 = local read "DISP LAB03-1"() -> (w867:T4)
                        n552 = Bundle(cluster=w867, "CYCLE"=w865, "MINS"=w865, "STATUS"="RUN") -> (w866:T4)
                        n553 = local write "DISP LAB03-1"(w866) -> ()
                      }
                      frame #4 {
                        n554 = local read "SIG LAB03-1"() -> (w870:T2)
                        n555 = local read "TEMP START LAB03-1"() -> (w872:cluster{"TL":dbl, "TN":dbl})
                        n556 = Unbundle(w870) -> ("Tmp Live"=w869:dbl, "Tmp Neut"=w868:dbl)  [unwired: 3 out]
                        n557 = Bundle(cluster=w872, "TL"=w869, "TN"=w868) -> (w871:cluster{"TL":dbl, "TN":dbl})
                        n558 = local write "TEMP START LAB03-1"(w871) -> ()
                      }
                    }
                  }
                }
              }
              event "RUN LAB03-2": Value Change {
                n559 = event-data() -> ("NewVal"=w873:bool)  [unwired: 1 in, 5 out]
                n560 = local write "run lab03-2"(w873) -> ()
                n561 = case shown="True" w873 {
                  tunnel: w879 -> [_ w912]
                  tunnel: w878 -> [_ w911]
                  tunnel: w876 -> [w881 w910]
                  tunnel: w877 -> [_ w909]
                  tunnel: w875 -> [_ w908]
                  tunnel: [w880 w907] -> w874
                  frame False {
                    # "stop test"
                    n562 = stacked-sequence {
                      tunnel: w881 -> [w890 _]
                      tunnel: [w882 _] -> w880
                      frame #0 {
                        n563 = local read "DISP LAB03-2"() -> (w889:T4)
                        n564 = Unbundle(w889) -> ("CYCLE"=w887:dbl, "MINS"=w888:dbl)  [unwired: 1 out]
                        n565 = case shown="\"CYCLE TEST\"" w890 {
                          tunnel: w888 -> [_ _ w897]
                          tunnel: w887 -> [w895 w896 _]
                          tunnel: [w895 w896 w897] -> w886
                          frame "CHART TEST", Default {
                          }
                          frame "CYCLE TEST" {
                          }
                          frame "T-RISE TEST" {
                          }
                        }
                        n566 = local read "TDMS LAB03-2"() -> (w894:refnum<k34>)
                        n567 = Build Array("STOPPED") -> (w891:string[])
                        n568 = Build Array(w886) -> (w885:dbl[])
                        n569 = TDMS Write(0:w894, 5:"TEST RESULT", 7:w891, 9:w885) -> (4:w883:refnum<k34>, 15:w884:errorcluster)  [unwired: 2 in, 2 out]
                        n570 = TDMS Close(8:w884, 11:w883) -> (0:w882:errorcluster)  [unwired: 1 out]
                      }
                      frame #1 {
                        n571 = local read "DISP LAB03-2"() -> (w901:T4)
                        n572 = stacked-sequence {
                          tunnel: "LAB03-2" -> [w903 w905]
                          frame #0 {
                            n573 = call "sub vi - defrag tdms v1.vi"("panel id"=w903) -> ("error out"=w902:errorcluster)  [unwired: 10 in]
                            n574 = local write "data file error"(w902) -> ()
                          }
                          frame #1 {
                            n575 = call "Save data file to network drive v1.vi"("panel id"=w905) -> ("network file save error"=w904:errorcluster)  [unwired: 9 in, 1 out]
                            n576 = local write "RESULT LAB03-2"(FALSE) -> ()
                            n577 = local write "data file error"(w904) -> ()
                          }
                        }
                        n578 = Bundle(cluster=w901, "STATUS"="STOP") -> (w899:T4)  [unwired: 2 in]
                        n579 = local write "DISP LAB03-2"(w899) -> ()
                      }
                    }
                  }
                  frame True {
                    # "start new test and create test file"
                    n580 = stacked-sequence {
                      seq-local: [w913 _ _ _ _] -> [_ w938 _ _ _]
                      tunnel: w912 -> [w918 _ _ _ _]
                      tunnel: w911 -> [w915 _ _ _ _]
                      tunnel: w910 -> [w928 _ _ _ _]
                      tunnel: w909 -> [w921 _ _ _ _]
                      tunnel: w908 -> [w916 _ _ _ _]
                      tunnel: [_ w932 _ _ _] -> w907
                      frame #0 {
                        w914 = "\\"
                        n581 = local read "SET LAB03-2"() -> (w923:T5)
                        n582 = case shown="\"T-RISE TEST\"" w928 {
                          tunnel: ["L03-2-CHART TEST-" "L03-2-CYCLE TEST-" "L03-2-T-RISE TEST-"] -> w924
                          frame "CHART TEST", Default {
                          }
                          frame "CYCLE TEST" {
                          }
                          frame "T-RISE TEST" {
                          }
                        }
                        n583 = Unbundle(w923) -> ("DESCRIPTION"=w922:string)  [unwired: 4 out]
                        n584 = Concatenate Strings(w918, "\\", w916, w914, w915, w914) -> (w925:string)
                        n585 = String To Path(string=w925) -> (path=w927:path)
                        n586 = Concatenate Strings(w925, w924, w922, "-", w921, ".tdms") -> (w913:string)
                        n587 = Create Folder(path (use dialog)=w927) -> (error out=w926:errorcluster)  [unwired: 2 in, 2 out]
                        n588 = global write "Global 1.vi" "LAB03-2 FILE"(w913) -> ()
                        n589 = call <vilib>:"Clear Errors.vi"("error in (no error)"=w926) -> ()  [unwired: 6 in, 1 out]
                      }
                      frame #1 {
                        n590 = String To Path(string=w938) -> (path=w933:path)
                        n591 = TDMS Open(5:FALSE, 6:FALSE, 10:T15."create or replace" ("operation (0:open)"), 11:w933) -> (0:w932:errorcluster, 3:→"TDMS LAB03-2":refnum<k34>)  [unwired: 3 in]
                      }
                      frame #2 {
                        n592 = local read "SET LAB03-2"() -> (w944:T5)
                        n593 = local read "TDMS LAB03-2"() -> (w955:refnum<k34>)
                        n594 = Build Array("Testers Name", "Description", "Set Test Cycles", "T-Rise minutes", "T-Rise Deg C") -> (w945:string[])
                        n595 = Unbundle(w944) -> ("NAME"=w943:string, "DESCRIPTION"=w942:string, "CYCLES"=w941:dbl, "T-RISE mins"=w940:dbl, "T-RISE deg C"=w939:dbl)
                        n596 = Number To Decimal String(number=w941) -> (decimal integer string=w954:string)  [unwired: 1 in]
                        n597 = Number To Decimal String(number=w940) -> (decimal integer string=w953:string)  [unwired: 1 in]
                        n598 = Number To Decimal String(number=w939) -> (decimal integer string=w952:string)  [unwired: 1 in]
                        n599 = Build Array(w943, w942, w954, w953, w952) -> (w951:string[])
                        n600 = TDMS Set Properties(5:w951, 7:w945, 11:w955) -> ()  [unwired: 3 in, 4 out]
                      }
                      frame #3 {
                        w957 = 0.0
                        n601 = local read "DISP LAB03-2"() -> (w959:T4)
                        n602 = Bundle(cluster=w959, "CYCLE"=w957, "MINS"=w957, "STATUS"="RUN") -> (w958:T4)
                        n603 = local write "DISP LAB03-2"(w958) -> ()
                      }
                      frame #4 {
                        n604 = local read "SIG LAB03-2"() -> (w962:T2)
                        n605 = local read "TEMP START LAB03-2"() -> (w964:cluster{"TL":dbl, "TN":dbl})
                        n606 = Unbundle(w962) -> ("Tmp Live"=w961:dbl, "Tmp Neut"=w960:dbl)  [unwired: 3 out]
                        n607 = Bundle(cluster=w964, "TL"=w961, "TN"=w960) -> (w963:cluster{"TL":dbl, "TN":dbl})
                        n608 = local write "TEMP START LAB03-2"(w963) -> ()
                      }
                    }
                  }
                }
              }
              event "RUN LAB04-1": Value Change {
                n609 = event-data() -> ("NewVal"=w965:bool)  [unwired: 1 in, 5 out]
                n610 = local write "run lab04-1"(w965) -> ()
                n611 = case shown="True" w965 {
                  tunnel: w971 -> [_ w1004]
                  tunnel: w970 -> [_ w1003]
                  tunnel: w968 -> [w973 w1002]
                  tunnel: w969 -> [_ w1001]
                  tunnel: w967 -> [_ w1000]
                  tunnel: [w972 w999] -> w966
                  frame False {
                    # "stop test"
                    n612 = stacked-sequence {
                      tunnel: w973 -> [w982 _]
                      tunnel: [w974 _] -> w972
                      frame #0 {
                        n613 = local read "DISP LAB04-1"() -> (w981:T4)
                        n614 = Unbundle(w981) -> ("CYCLE"=w979:dbl, "MINS"=w980:dbl)  [unwired: 1 out]
                        n615 = case shown="\"CYCLE TEST\"" w982 {
                          tunnel: w980 -> [_ _ w989]
                          tunnel: w979 -> [w987 w988 _]
                          tunnel: [w987 w988 w989] -> w978
                          frame "CHART TEST", Default {
                          }
                          frame "CYCLE TEST" {
                          }
                          frame "T-RISE TEST" {
                          }
                        }
                        n616 = local read "TDMS LAB04-1"() -> (w986:refnum<k34>)
                        n617 = Build Array("STOPPED") -> (w983:string[])
                        n618 = Build Array(w978) -> (w977:dbl[])
                        n619 = TDMS Write(0:w986, 5:"TEST RESULT", 7:w983, 9:w977) -> (4:w975:refnum<k34>, 15:w976:errorcluster)  [unwired: 2 in, 2 out]
                        n620 = TDMS Close(8:w976, 11:w975) -> (0:w974:errorcluster)  [unwired: 1 out]
                      }
                      frame #1 {
                        n621 = local read "DISP LAB04-1"() -> (w993:T4)
                        n622 = stacked-sequence {
                          tunnel: "LAB04-1" -> [w995 w997]
                          frame #0 {
                            n623 = call "sub vi - defrag tdms v1.vi"("panel id"=w995) -> ("error out"=w994:errorcluster)  [unwired: 10 in]
                            n624 = local write "data file error"(w994) -> ()
                          }
                          frame #1 {
                            n625 = call "Save data file to network drive v1.vi"("panel id"=w997) -> ("network file save error"=w996:errorcluster)  [unwired: 9 in, 1 out]
                            n626 = local write "RESULT LAB04-1"(FALSE) -> ()
                            n627 = local write "data file error"(w996) -> ()
                          }
                        }
                        n628 = Bundle(cluster=w993, "STATUS"="STOP") -> (w991:T4)  [unwired: 2 in]
                        n629 = local write "DISP LAB04-1"(w991) -> ()
                      }
                    }
                  }
                  frame True {
                    # "start new test and create test file"
                    n630 = stacked-sequence {
                      seq-local: [w1005 _ _ _ _] -> [_ w1030 _ _ _]
                      tunnel: w1004 -> [w1010 _ _ _ _]
                      tunnel: w1003 -> [w1006 _ _ _ _]
                      tunnel: w1002 -> [w1020 _ _ _ _]
                      tunnel: w1001 -> [w1013 _ _ _ _]
                      tunnel: w1000 -> [w1008 _ _ _ _]
                      tunnel: [_ w1024 _ _ _] -> w999
                      frame #0 {
                        w1007 = "\\"
                        n631 = local read "SET LAB04-1"() -> (w1015:T5)
                        n632 = case shown="\"CYCLE TEST\"" w1020 {
                          tunnel: ["L04-1-CHART TEST-" "L04-1-CYCLE TEST-" "L04-1-T-RISE TEST-"] -> w1016
                          frame "CHART TEST", Default {
                          }
                          frame "CYCLE TEST" {
                          }
                          frame "T-RISE TEST" {
                          }
                        }
                        n633 = Unbundle(w1015) -> ("DESCRIPTION"=w1014:string)  [unwired: 4 out]
                        n634 = Concatenate Strings(w1010, "\\", w1008, w1007, w1006, w1007) -> (w1017:string)
                        n635 = String To Path(string=w1017) -> (path=w1019:path)
                        n636 = Concatenate Strings(w1017, w1016, w1014, "-", w1013, ".tdms") -> (w1005:string)
                        n637 = Create Folder(path (use dialog)=w1019) -> (error out=w1018:errorcluster)  [unwired: 2 in, 2 out]
                        n638 = global write "Global 1.vi" "LAB04-1 FILE"(w1005) -> ()
                        n639 = call <vilib>:"Clear Errors.vi"("error in (no error)"=w1018) -> ()  [unwired: 6 in, 1 out]
                      }
                      frame #1 {
                        n640 = String To Path(string=w1030) -> (path=w1025:path)
                        n641 = TDMS Open(5:FALSE, 6:FALSE, 10:T15."create or replace" ("operation (0:open)"), 11:w1025) -> (0:w1024:errorcluster, 3:→"TDMS LAB04-1":refnum<k34>)  [unwired: 3 in]
                      }
                      frame #2 {
                        n642 = local read "SET LAB04-1"() -> (w1036:T5)
                        n643 = local read "TDMS LAB04-1"() -> (w1047:refnum<k34>)
                        n644 = Build Array("Testers Name", "Description", "Set Test Cycles", "T-Rise minutes", "T-Rise Deg C") -> (w1037:string[])
                        n645 = Unbundle(w1036) -> ("NAME"=w1035:string, "DESCRIPTION"=w1034:string, "CYCLES"=w1033:dbl, "T-RISE mins"=w1032:dbl, "T-RISE deg C"=w1031:dbl)
                        n646 = Number To Decimal String(number=w1033) -> (decimal integer string=w1046:string)  [unwired: 1 in]
                        n647 = Number To Decimal String(number=w1032) -> (decimal integer string=w1045:string)  [unwired: 1 in]
                        n648 = Number To Decimal String(number=w1031) -> (decimal integer string=w1044:string)  [unwired: 1 in]
                        n649 = Build Array(w1035, w1034, w1046, w1045, w1044) -> (w1043:string[])
                        n650 = TDMS Set Properties(5:w1043, 7:w1037, 11:w1047) -> ()  [unwired: 3 in, 4 out]
                      }
                      frame #3 {
                        w1049 = 0.0
                        n651 = local read "DISP LAB04-1"() -> (w1051:T4)
                        n652 = Bundle(cluster=w1051, "CYCLE"=w1049, "MINS"=w1049, "STATUS"="RUN") -> (w1050:T4)
                        n653 = local write "DISP LAB04-1"(w1050) -> ()
                      }
                      frame #4 {
                        n654 = local read "SIG LAB04-1"() -> (w1054:T2)
                        n655 = local read "TEMP START LAB04-1"() -> (w1056:cluster{"TL":dbl, "TN":dbl})
                        n656 = Unbundle(w1054) -> ("Tmp Live"=w1053:dbl, "Tmp Neut"=w1052:dbl)  [unwired: 3 out]
                        n657 = Bundle(cluster=w1056, "TL"=w1053, "TN"=w1052) -> (w1055:cluster{"TL":dbl, "TN":dbl})
                        n658 = local write "TEMP START LAB04-1"(w1055) -> ()
                      }
                    }
                  }
                }
              }
              event "RUN LAB04-2": Value Change {
                n659 = event-data() -> ("NewVal"=w1057:bool)  [unwired: 1 in, 5 out]
                n660 = local write "run lab04-2"(w1057) -> ()
                n661 = case shown="True" w1057 {
                  tunnel: w1063 -> [_ w1096]
                  tunnel: w1062 -> [_ w1095]
                  tunnel: w1060 -> [w1065 w1094]
                  tunnel: w1061 -> [_ w1093]
                  tunnel: w1059 -> [_ w1092]
                  tunnel: [w1064 w1091] -> w1058
                  frame False {
                    # "stop test"
                    n662 = stacked-sequence {
                      tunnel: w1065 -> [w1074 _]
                      tunnel: [w1066 _] -> w1064
                      frame #0 {
                        n663 = local read "DISP LAB04-2"() -> (w1073:T4)
                        n664 = Unbundle(w1073) -> ("CYCLE"=w1071:dbl, "MINS"=w1072:dbl)  [unwired: 1 out]
                        n665 = case shown="\"CYCLE TEST\"" w1074 {
                          tunnel: w1072 -> [_ _ w1081]
                          tunnel: w1071 -> [w1079 w1080 _]
                          tunnel: [w1079 w1080 w1081] -> w1070
                          frame "CHART TEST", Default {
                          }
                          frame "CYCLE TEST" {
                          }
                          frame "T-RISE TEST" {
                          }
                        }
                        n666 = local read "TDMS LAB04-2"() -> (w1078:refnum<k34>)
                        n667 = Build Array("STOPPED") -> (w1075:string[])
                        n668 = Build Array(w1070) -> (w1069:dbl[])
                        n669 = TDMS Write(0:w1078, 5:"TEST RESULT", 7:w1075, 9:w1069) -> (4:w1067:refnum<k34>, 15:w1068:errorcluster)  [unwired: 2 in, 2 out]
                        n670 = TDMS Close(8:w1068, 11:w1067) -> (0:w1066:errorcluster)  [unwired: 1 out]
                      }
                      frame #1 {
                        n671 = local read "DISP LAB04-2"() -> (w1085:T4)
                        n672 = stacked-sequence {
                          tunnel: "LAB04-2" -> [w1087 w1089]
                          frame #0 {
                            n673 = call "sub vi - defrag tdms v1.vi"("panel id"=w1087) -> ("error out"=w1086:errorcluster)  [unwired: 10 in]
                            n674 = local write "data file error"(w1086) -> ()
                          }
                          frame #1 {
                            n675 = call "Save data file to network drive v1.vi"("panel id"=w1089) -> ("network file save error"=w1088:errorcluster)  [unwired: 9 in, 1 out]
                            n676 = local write "RESULT LAB04-2"(FALSE) -> ()
                            n677 = local write "data file error"(w1088) -> ()
                          }
                        }
                        n678 = Bundle(cluster=w1085, "STATUS"="STOP") -> (w1083:T4)  [unwired: 2 in]
                        n679 = local write "DISP LAB04-2"(w1083) -> ()
                      }
                    }
                  }
                  frame True {
                    # "start new test and create test file"
                    n680 = stacked-sequence {
                      seq-local: [w1097 _ _ _ _] -> [_ w1122 _ _ _]
                      tunnel: w1096 -> [w1102 _ _ _ _]
                      tunnel: w1095 -> [w1098 _ _ _ _]
                      tunnel: w1094 -> [w1112 _ _ _ _]
                      tunnel: w1093 -> [w1105 _ _ _ _]
                      tunnel: w1092 -> [w1100 _ _ _ _]
                      tunnel: [_ w1116 _ _ _] -> w1091
                      frame #0 {
                        w1099 = "\\"
                        n681 = local read "SET LAB04-2"() -> (w1107:T5)
                        n682 = case shown="\"CHART TEST\", Default" w1112 {
                          tunnel: ["L04-2-CHART TEST-" "L04-2-CYCLE TEST-" "L04-2-T-RISE TEST-"] -> w1108
                          frame "CHART TEST", Default {
                          }
                          frame "CYCLE TEST" {
                          }
                          frame "T-RISE TEST" {
                          }
                        }
                        n683 = Unbundle(w1107) -> ("DESCRIPTION"=w1106:string)  [unwired: 4 out]
                        n684 = Concatenate Strings(w1102, "\\", w1100, w1099, w1098, w1099) -> (w1109:string)
                        n685 = String To Path(string=w1109) -> (path=w1111:path)
                        n686 = Concatenate Strings(w1109, w1108, w1106, "-", w1105, ".tdms") -> (w1097:string)
                        n687 = Create Folder(path (use dialog)=w1111) -> (error out=w1110:errorcluster)  [unwired: 2 in, 2 out]
                        n688 = global write "Global 1.vi" "LAB04-2 FILE"(w1097) -> ()
                        n689 = call <vilib>:"Clear Errors.vi"("error in (no error)"=w1110) -> ()  [unwired: 6 in, 1 out]
                      }
                      frame #1 {
                        n690 = String To Path(string=w1122) -> (path=w1117:path)
                        n691 = TDMS Open(5:FALSE, 6:FALSE, 10:T15."create or replace" ("operation (0:open)"), 11:w1117) -> (0:w1116:errorcluster, 3:→"TDMS LAB04-2":refnum<k34>)  [unwired: 3 in]
                      }
                      frame #2 {
                        n692 = local read "SET LAB04-2"() -> (w1128:T5)
                        n693 = local read "TDMS LAB04-2"() -> (w1139:refnum<k34>)
                        n694 = Build Array("Testers Name", "Description", "Set Test Cycles", "T-Rise minutes", "T-Rise Deg C") -> (w1129:string[])
                        n695 = Unbundle(w1128) -> ("NAME"=w1127:string, "DESCRIPTION"=w1126:string, "CYCLES"=w1125:dbl, "T-RISE mins"=w1124:dbl, "T-RISE deg C"=w1123:dbl)
                        n696 = Number To Decimal String(number=w1125) -> (decimal integer string=w1138:string)  [unwired: 1 in]
                        n697 = Number To Decimal String(number=w1124) -> (decimal integer string=w1137:string)  [unwired: 1 in]
                        n698 = Number To Decimal String(number=w1123) -> (decimal integer string=w1136:string)  [unwired: 1 in]
                        n699 = Build Array(w1127, w1126, w1138, w1137, w1136) -> (w1135:string[])
                        n700 = TDMS Set Properties(5:w1135, 7:w1129, 11:w1139) -> ()  [unwired: 3 in, 4 out]
                      }
                      frame #3 {
                        w1141 = 0.0
                        n701 = local read "DISP LAB04-2"() -> (w1143:T4)
                        n702 = Bundle(cluster=w1143, "CYCLE"=w1141, "MINS"=w1141, "STATUS"="RUN") -> (w1142:T4)
                        n703 = local write "DISP LAB04-2"(w1142) -> ()
                      }
                      frame #4 {
                        n704 = local read "SIG LAB04-2"() -> (w1146:T2)
                        n705 = local read "TEMP START LAB04-2"() -> (w1148:cluster{"TL":dbl, "TN":dbl})
                        n706 = Unbundle(w1146) -> ("Tmp Live"=w1145:dbl, "Tmp Neut"=w1144:dbl)  [unwired: 3 out]
                        n707 = Bundle(cluster=w1148, "TL"=w1145, "TN"=w1144) -> (w1147:cluster{"TL":dbl, "TN":dbl})
                        n708 = local write "TEMP START LAB04-2"(w1147) -> ()
                      }
                    }
                  }
                }
              }
              event "RUN LAB05-1": Value Change {
                n709 = event-data() -> ("NewVal"=w1149:bool)  [unwired: 1 in, 5 out]
                n710 = local write "run lab05-1"(w1149) -> ()
                n711 = case shown="True" w1149 {
                  tunnel: w1155 -> [_ w1188]
                  tunnel: w1154 -> [_ w1187]
                  tunnel: w1152 -> [w1157 w1186]
                  tunnel: w1153 -> [_ w1185]
                  tunnel: w1151 -> [_ w1184]
                  tunnel: [w1156 w1183] -> w1150
                  frame False {
                    # "stop test"
                    n712 = stacked-sequence {
                      tunnel: w1157 -> [w1166 _]
                      tunnel: [w1158 _] -> w1156
                      frame #0 {
                        n713 = local read "DISP LAB05-1"() -> (w1165:T4)
                        n714 = Unbundle(w1165) -> ("CYCLE"=w1163:dbl, "MINS"=w1164:dbl)  [unwired: 1 out]
                        n715 = case shown="\"CYCLE TEST\"" w1166 {
                          tunnel: w1164 -> [_ _ w1173]
                          tunnel: w1163 -> [w1171 w1172 _]
                          tunnel: [w1171 w1172 w1173] -> w1162
                          frame "CHART TEST", Default {
                          }
                          frame "CYCLE TEST" {
                          }
                          frame "T-RISE TEST" {
                          }
                        }
                        n716 = local read "TDMS LAB05-1"() -> (w1170:refnum<k34>)
                        n717 = Build Array("STOPPED") -> (w1167:string[])
                        n718 = Build Array(w1162) -> (w1161:dbl[])
                        n719 = TDMS Write(0:w1170, 5:"TEST RESULT", 7:w1167, 9:w1161) -> (4:w1159:refnum<k34>, 15:w1160:errorcluster)  [unwired: 2 in, 2 out]
                        n720 = TDMS Close(8:w1160, 11:w1159) -> (0:w1158:errorcluster)  [unwired: 1 out]
                      }
                      frame #1 {
                        n721 = local read "DISP LAB05-1"() -> (w1177:T4)
                        n722 = stacked-sequence {
                          tunnel: "LAB05-1" -> [w1179 w1181]
                          frame #0 {
                            n723 = call "sub vi - defrag tdms v1.vi"("panel id"=w1179) -> ("error out"=w1178:errorcluster)  [unwired: 10 in]
                            n724 = local write "data file error"(w1178) -> ()
                          }
                          frame #1 {
                            n725 = call "Save data file to network drive v1.vi"("panel id"=w1181) -> ("network file save error"=w1180:errorcluster)  [unwired: 9 in, 1 out]
                            n726 = local write "RESULT LAB05-1"(FALSE) -> ()
                            n727 = local write "data file error"(w1180) -> ()
                          }
                        }
                        n728 = Bundle(cluster=w1177, "STATUS"="STOP") -> (w1175:T4)  [unwired: 2 in]
                        n729 = local write "DISP LAB05-1"(w1175) -> ()
                      }
                    }
                  }
                  frame True {
                    # "start new test and create test file"
                    n730 = stacked-sequence {
                      seq-local: [w1189 _ _ _ _] -> [_ w1214 _ _ _]
                      tunnel: w1188 -> [w1194 _ _ _ _]
                      tunnel: w1187 -> [w1190 _ _ _ _]
                      tunnel: w1186 -> [w1204 _ _ _ _]
                      tunnel: w1185 -> [w1197 _ _ _ _]
                      tunnel: w1184 -> [w1192 _ _ _ _]
                      tunnel: [_ w1208 _ _ _] -> w1183
                      frame #0 {
                        w1191 = "\\"
                        n731 = local read "SET LAB05-1"() -> (w1199:T5)
                        n732 = case shown="\"CYCLE TEST\"" w1204 {
                          tunnel: ["L05-1-CHART TEST-" "L05-1-CYCLE TEST-" "L05-1-T-RISE TEST-"] -> w1200
                          frame "CHART TEST", Default {
                          }
                          frame "CYCLE TEST" {
                          }
                          frame "T-RISE TEST" {
                          }
                        }
                        n733 = Unbundle(w1199) -> ("DESCRIPTION"=w1198:string)  [unwired: 4 out]
                        n734 = Concatenate Strings(w1194, "\\", w1192, w1191, w1190, w1191) -> (w1201:string)
                        n735 = String To Path(string=w1201) -> (path=w1203:path)
                        n736 = Concatenate Strings(w1201, w1200, w1198, "-", w1197, ".tdms") -> (w1189:string)
                        n737 = Create Folder(path (use dialog)=w1203) -> (error out=w1202:errorcluster)  [unwired: 2 in, 2 out]
                        n738 = global write "Global 1.vi" "LAB05-1 FILE"(w1189) -> ()
                        n739 = call <vilib>:"Clear Errors.vi"("error in (no error)"=w1202) -> ()  [unwired: 6 in, 1 out]
                      }
                      frame #1 {
                        n740 = String To Path(string=w1214) -> (path=w1209:path)
                        n741 = TDMS Open(5:FALSE, 6:FALSE, 10:T15."create or replace" ("operation (0:open)"), 11:w1209) -> (0:w1208:errorcluster, 3:→"TDMS LAB05-1":refnum<k34>)  [unwired: 3 in]
                      }
                      frame #2 {
                        n742 = local read "SET LAB05-1"() -> (w1220:T5)
                        n743 = local read "TDMS LAB05-1"() -> (w1231:refnum<k34>)
                        n744 = Build Array("Testers Name", "Description", "Set Test Cycles", "T-Rise minutes", "T-Rise Deg C") -> (w1221:string[])
                        n745 = Unbundle(w1220) -> ("NAME"=w1219:string, "DESCRIPTION"=w1218:string, "CYCLES"=w1217:dbl, "T-RISE mins"=w1216:dbl, "T-RISE deg C"=w1215:dbl)
                        n746 = Number To Decimal String(number=w1217) -> (decimal integer string=w1230:string)  [unwired: 1 in]
                        n747 = Number To Decimal String(number=w1216) -> (decimal integer string=w1229:string)  [unwired: 1 in]
                        n748 = Number To Decimal String(number=w1215) -> (decimal integer string=w1228:string)  [unwired: 1 in]
                        n749 = Build Array(w1219, w1218, w1230, w1229, w1228) -> (w1227:string[])
                        n750 = TDMS Set Properties(5:w1227, 7:w1221, 11:w1231) -> ()  [unwired: 3 in, 4 out]
                      }
                      frame #3 {
                        w1233 = 0.0
                        n751 = local read "DISP LAB05-1"() -> (w1235:T4)
                        n752 = Bundle(cluster=w1235, "CYCLE"=w1233, "MINS"=w1233, "STATUS"="RUN") -> (w1234:T4)
                        n753 = local write "DISP LAB05-1"(w1234) -> ()
                      }
                      frame #4 {
                        n754 = local read "SIG LAB05-1"() -> (w1238:T2)
                        n755 = local read "TEMP START LAB05-1"() -> (w1240:cluster{"TL":dbl, "TN":dbl})
                        n756 = Unbundle(w1238) -> ("Tmp Live"=w1237:dbl, "Tmp Neut"=w1236:dbl)  [unwired: 3 out]
                        n757 = Bundle(cluster=w1240, "TL"=w1237, "TN"=w1236) -> (w1239:cluster{"TL":dbl, "TN":dbl})
                        n758 = local write "TEMP START LAB05-1"(w1239) -> ()
                      }
                    }
                  }
                }
              }
              event "RUN LAB05-2": Value Change {
                n759 = event-data() -> ("NewVal"=w1241:bool)  [unwired: 1 in, 5 out]
                n760 = local write "run lab05-2"(w1241) -> ()
                n761 = case shown="True" w1241 {
                  tunnel: w1247 -> [_ w1280]
                  tunnel: w1246 -> [_ w1279]
                  tunnel: w1244 -> [w1249 w1278]
                  tunnel: w1245 -> [_ w1277]
                  tunnel: w1243 -> [_ w1276]
                  tunnel: [w1248 w1275] -> w1242
                  frame False {
                    # "stop test"
                    n762 = stacked-sequence {
                      tunnel: w1249 -> [w1258 _]
                      tunnel: [w1250 _] -> w1248
                      frame #0 {
                        n763 = local read "DISP LAB05-2"() -> (w1257:T4)
                        n764 = Unbundle(w1257) -> ("CYCLE"=w1255:dbl, "MINS"=w1256:dbl)  [unwired: 1 out]
                        n765 = case shown="\"CYCLE TEST\"" w1258 {
                          tunnel: w1256 -> [_ _ w1265]
                          tunnel: w1255 -> [w1263 w1264 _]
                          tunnel: [w1263 w1264 w1265] -> w1254
                          frame "CHART TEST", Default {
                          }
                          frame "CYCLE TEST" {
                          }
                          frame "T-RISE TEST" {
                          }
                        }
                        n766 = local read "TDMS LAB05-2"() -> (w1262:refnum<k34>)
                        n767 = Build Array("STOPPED") -> (w1259:string[])
                        n768 = Build Array(w1254) -> (w1253:dbl[])
                        n769 = TDMS Write(0:w1262, 5:"TEST RESULT", 7:w1259, 9:w1253) -> (4:w1251:refnum<k34>, 15:w1252:errorcluster)  [unwired: 2 in, 2 out]
                        n770 = TDMS Close(8:w1252, 11:w1251) -> (0:w1250:errorcluster)  [unwired: 1 out]
                      }
                      frame #1 {
                        n771 = local read "DISP LAB05-2"() -> (w1269:T4)
                        n772 = stacked-sequence {
                          tunnel: "LAB05-2" -> [w1271 w1273]
                          frame #0 {
                            n773 = call "sub vi - defrag tdms v1.vi"("panel id"=w1271) -> ("error out"=w1270:errorcluster)  [unwired: 10 in]
                            n774 = local write "data file error"(w1270) -> ()
                          }
                          frame #1 {
                            n775 = local write "RESULT LAB05-2"(FALSE) -> ()
                            n776 = call "Save data file to network drive v1.vi"("panel id"=w1273) -> ("network file save error"=w1272:errorcluster)  [unwired: 9 in, 1 out]
                            n777 = local write "data file error"(w1272) -> ()
                          }
                        }
                        n778 = Bundle(cluster=w1269, "STATUS"="STOP") -> (w1267:T4)  [unwired: 2 in]
                        n779 = local write "DISP LAB05-2"(w1267) -> ()
                      }
                    }
                  }
                  frame True {
                    # "start new test and create test file"
                    n780 = stacked-sequence {
                      seq-local: [w1281 _ _ _ _] -> [_ w1306 _ _ _]
                      tunnel: w1280 -> [w1286 _ _ _ _]
                      tunnel: w1279 -> [w1282 _ _ _ _]
                      tunnel: w1278 -> [w1296 _ _ _ _]
                      tunnel: w1277 -> [w1289 _ _ _ _]
                      tunnel: w1276 -> [w1284 _ _ _ _]
                      tunnel: [_ w1300 _ _ _] -> w1275
                      frame #0 {
                        w1283 = "\\"
                        n781 = local read "SET LAB05-2"() -> (w1291:T5)
                        n782 = case shown="\"CYCLE TEST\"" w1296 {
                          tunnel: ["L05-2-CHART TEST-" "L05-2-CYCLE TEST-" "L05-2-T-RISE TEST-"] -> w1292
                          frame "CHART TEST", Default {
                          }
                          frame "CYCLE TEST" {
                          }
                          frame "T-RISE TEST" {
                          }
                        }
                        n783 = Unbundle(w1291) -> ("DESCRIPTION"=w1290:string)  [unwired: 4 out]
                        n784 = Concatenate Strings(w1286, "\\", w1284, w1283, w1282, w1283) -> (w1293:string)
                        n785 = String To Path(string=w1293) -> (path=w1295:path)
                        n786 = Concatenate Strings(w1293, w1292, w1290, "-", w1289, ".tdms") -> (w1281:string)
                        n787 = Create Folder(path (use dialog)=w1295) -> (error out=w1294:errorcluster)  [unwired: 2 in, 2 out]
                        n788 = global write "Global 1.vi" "LAB05-2 FILE"(w1281) -> ()
                        n789 = call <vilib>:"Clear Errors.vi"("error in (no error)"=w1294) -> ()  [unwired: 6 in, 1 out]
                      }
                      frame #1 {
                        n790 = String To Path(string=w1306) -> (path=w1301:path)
                        n791 = TDMS Open(5:FALSE, 6:FALSE, 10:T15."create or replace" ("operation (0:open)"), 11:w1301) -> (0:w1300:errorcluster, 3:→"TDMS LAB05-2":refnum<k34>)  [unwired: 3 in]
                      }
                      frame #2 {
                        n792 = local read "SET LAB05-2"() -> (w1312:T5)
                        n793 = local read "TDMS LAB05-2"() -> (w1323:refnum<k34>)
                        n794 = Build Array("Testers Name", "Description", "Set Test Cycles", "T-Rise minutes", "T-Rise Deg C") -> (w1313:string[])
                        n795 = Unbundle(w1312) -> ("NAME"=w1311:string, "DESCRIPTION"=w1310:string, "CYCLES"=w1309:dbl, "T-RISE mins"=w1308:dbl, "T-RISE deg C"=w1307:dbl)
                        n796 = Number To Decimal String(number=w1309) -> (decimal integer string=w1322:string)  [unwired: 1 in]
                        n797 = Number To Decimal String(number=w1308) -> (decimal integer string=w1321:string)  [unwired: 1 in]
                        n798 = Number To Decimal String(number=w1307) -> (decimal integer string=w1320:string)  [unwired: 1 in]
                        n799 = Build Array(w1311, w1310, w1322, w1321, w1320) -> (w1319:string[])
                        n800 = TDMS Set Properties(5:w1319, 7:w1313, 11:w1323) -> ()  [unwired: 3 in, 4 out]
                      }
                      frame #3 {
                        w1325 = 0.0
                        n801 = local read "DISP LAB05-2"() -> (w1327:T4)
                        n802 = Bundle(cluster=w1327, "CYCLE"=w1325, "MINS"=w1325, "STATUS"="RUN") -> (w1326:T4)
                        n803 = local write "DISP LAB05-2"(w1326) -> ()
                      }
                      frame #4 {
                        n804 = local read "SIG LAB05-2"() -> (w1330:T2)
                        n805 = local read "TEMP START LAB05-2"() -> (w1332:cluster{"TL":dbl, "TN":dbl})
                        n806 = Unbundle(w1330) -> ("Tmp Live"=w1329:dbl, "Tmp Neut"=w1328:dbl)  [unwired: 3 out]
                        n807 = Bundle(cluster=w1332, "TL"=w1329, "TN"=w1328) -> (w1331:cluster{"TL":dbl, "TN":dbl})
                        n808 = local write "TEMP START LAB05-2"(w1331) -> ()
                      }
                    }
                  }
                }
              }
            }
            n809 = local write "data file error"(w384) -> ()
          }
          frame #4 {
            # "check if test cycles reached for cycle tests, if so then test pass"
            n810 = stacked-sequence {
              tunnel: w1352 -> [_ _ _ _ _ _ _ _ _ _]
              tunnel: w1351 -> [_ _ _ _ _ _ _ _ _ _]
              tunnel: w1350 -> [_ _ _ _ _ _ _ _ _ _]
              tunnel: w1349 -> [_ _ _ _ _ _ _ _ _ _]
              tunnel: w1348 -> [_ _ _ _ _ _ _ _ _ _]
              tunnel: w1347 -> [_ _ _ _ _ _ _ _ _ _]
              tunnel: w1346 -> [_ _ _ _ _ _ _ _ _ _]
              tunnel: w1345 -> [_ _ _ _ _ _ _ _ _ _]
              tunnel: w1344 -> [_ _ _ _ _ _ _ _ _ _]
              tunnel: w1343 -> [_ _ _ _ _ _ _ _ _ _]
              tunnel: w1342 -> [w1358 _ _ _ _ _ _ _ _ _]
              tunnel: w1341 -> [_ w1393 _ _ _ _ _ _ _ _]
              tunnel: w1340 -> [_ _ w1433 _ _ _ _ _ _ _]
              tunnel: w1339 -> [_ _ _ w1473 _ _ _ _ _ _]
              tunnel: w1338 -> [_ _ _ _ w1513 _ _ _ _ _]
              tunnel: w1337 -> [_ _ _ _ _ w1553 _ _ _ _]
              tunnel: w1336 -> [_ _ _ _ _ _ w1593 _ _ _]
              tunnel: w1335 -> [_ _ _ _ _ _ _ w1633 _ _]
              tunnel: w1334 -> [_ _ _ _ _ _ _ _ w1673 _]
              tunnel: w1333 -> [_ _ _ _ _ _ _ _ _ w1713]
              frame #0 {
                # "LAB01-1"
                n811 = Less?(x=w1358, y=2) -> (x < y?=w1356:bool)
                n812 = local read "DISP LAB01-1"() -> (w1359:T4)
                n813 = Unbundle(w1359) -> ("STATUS"=w1353:string)  [unwired: 2 out]
                n814 = Equal?(x=w1353, y="RUN") -> (x = y?=w1355:bool)
                n815 = And(x=w1355, y=w1356) -> (x .and. y?=w1354:bool)
                n816 = case shown="True" w1354 {
                  tunnel: w1359 -> [_ w1364]
                  tunnel: w1358 -> [_ w1368]
                  frame False {
                  }
                  frame True {
                    n817 = local read "SET LAB01-1"() -> (w1370:T5)
                    n818 = local read "TDMS LAB01-1"() -> (w1363:refnum<k34>)
                    n819 = Unbundle(w1370) -> ("CYCLES"=w1361:dbl, "T-RISE mins"=w1367:dbl)  [unwired: 3 out]
                    n820 = case shown="\"CYCLE TEST\"" w1368 {
                      tunnel: w1367 -> [_ _ w1377]
                      tunnel: [w1372 w1374 w1377] -> w1366
                      tunnel: w1361 -> [w1372 w1374 _]
                      tunnel: ["CHART PASS" "CYCLE PASS" "T-RISE PASS"] -> w1365
                      frame "CHART TEST", Default {
                      }
                      frame "CYCLE TEST" {
                      }
                      frame "T-RISE TEST" {
                      }
                    }
                    n821 = Unbundle(w1364) -> ("CYCLE"=w1369:dbl)  [unwired: 2 out]
                    n822 = Increment(x=w1361) -> (x+1=w1362:dbl)
                    n823 = Greater Or Equal?(x=w1369, y=w1362) -> (x >= y?=w1371:bool)
                    n824 = case shown="True" w1371 {
                      tunnel: w1366 -> [w1381 _]
                      tunnel: w1365 -> [w1380 _]
                      tunnel: w1364 -> [w1379 _]
                      tunnel: w1363 -> [w1378 _]
                      frame True {
                        n825 = stacked-sequence {
                          tunnel: w1381 -> [w1385 _]
                          tunnel: w1380 -> [w1383 w1389]
                          tunnel: w1379 -> [_ w1392]
                          tunnel: w1378 -> [w1382 _]
                          frame #0 {
                            n826 = Build Array(w1383) -> (w1386:string[])
                            n827 = Build Array(w1385) -> (w1384:dbl[])
                            n828 = TDMS Write(0:w1382, 5:"TEST PASS", 7:w1386, 9:w1384) -> (15:w1388:errorcluster)  [unwired: 2 in, 3 out]
                            n829 = local write "data file error"(w1388) -> ()
                          }
                          frame #1 {
                            n830 = Bundle(cluster=w1392, "STATUS"=w1389) -> (w1390:T4)  [unwired: 2 in]
                            n831 = local write "RESULT LAB01-1"(TRUE) -> ()
                            n832 = local write "DISP LAB01-1"(w1390) -> ()
                          }
                        }
                      }
                      frame False {
                      }
                    }
                  }
                }
              }
              frame #1 {
                # "LAB01-2"
                n833 = Less?(x=w1393, y=2) -> (x < y?=w1396:bool)
                n834 = local read "DISP LAB01-2"() -> (w1398:T4)
                n835 = Unbundle(w1398) -> ("STATUS"=w1399:string)  [unwired: 2 out]
                n836 = Equal?(x=w1399, y="RUN") -> (x = y?=w1395:bool)
                n837 = And(x=w1395, y=w1396) -> (x .and. y?=w1394:bool)
                n838 = case shown="True" w1394 {
                  tunnel: w1398 -> [_ w1404]
                  tunnel: w1393 -> [_ w1408]
                  frame False {
                  }
                  frame True {
                    n839 = local read "SET LAB01-2"() -> (w1410:T5)
                    n840 = local read "TDMS LAB01-2"() -> (w1403:refnum<k34>)
                    n841 = Unbundle(w1410) -> ("CYCLES"=w1401:dbl, "T-RISE mins"=w1407:dbl)  [unwired: 3 out]
                    n842 = case shown="\"T-RISE TEST\"" w1408 {
                      tunnel: w1407 -> [_ _ w1417]
                      tunnel: [w1412 w1414 w1417] -> w1406
                      tunnel: w1401 -> [w1412 w1414 _]
                      tunnel: ["CHART PASS" "CYCLE PASS" "T-RISE PASS"] -> w1405
                      frame "CHART TEST", Default {
                      }
                      frame "CYCLE TEST" {
                      }
                      frame "T-RISE TEST" {
                      }
                    }
                    n843 = Unbundle(w1404) -> ("CYCLE"=w1409:dbl)  [unwired: 2 out]
                    n844 = Increment(x=w1401) -> (x+1=w1402:dbl)
                    n845 = Greater Or Equal?(x=w1409, y=w1402) -> (x >= y?=w1411:bool)
                    n846 = case shown="True" w1411 {
                      tunnel: w1406 -> [w1421 _]
                      tunnel: w1405 -> [w1420 _]
                      tunnel: w1404 -> [w1419 _]
                      tunnel: w1403 -> [w1418 _]
                      frame True {
                        n847 = stacked-sequence {
                          tunnel: w1421 -> [w1425 _]
                          tunnel: w1420 -> [w1423 w1429]
                          tunnel: w1419 -> [_ w1432]
                          tunnel: w1418 -> [w1422 _]
                          frame #0 {
                            n848 = Build Array(w1423) -> (w1426:string[])
                            n849 = Build Array(w1425) -> (w1424:dbl[])
                            n850 = TDMS Write(0:w1422, 5:"TEST PASS", 7:w1426, 9:w1424) -> (15:w1428:errorcluster)  [unwired: 2 in, 3 out]
                            n851 = local write "data file error"(w1428) -> ()
                          }
                          frame #1 {
                            n852 = Bundle(cluster=w1432, "STATUS"=w1429) -> (w1430:T4)  [unwired: 2 in]
                            n853 = local write "RESULT LAB01-2"(TRUE) -> ()
                            n854 = local write "DISP LAB01-2"(w1430) -> ()
                          }
                        }
                      }
                      frame False {
                      }
                    }
                  }
                }
              }
              frame #2 {
                # "LAB02-1"
                n855 = Less?(x=w1433, y=2) -> (x < y?=w1436:bool)
                n856 = local read "DISP LAB02-1"() -> (w1438:T4)
                n857 = Unbundle(w1438) -> ("STATUS"=w1439:string)  [unwired: 2 out]
                n858 = Equal?(x=w1439, y="RUN") -> (x = y?=w1435:bool)
                n859 = And(x=w1435, y=w1436) -> (x .and. y?=w1434:bool)
                n860 = case shown="True" w1434 {
                  tunnel: w1438 -> [_ w1444]
                  tunnel: w1433 -> [_ w1448]
                  frame False {
                  }
                  frame True {
                    n861 = local read "SET LAB02-1"() -> (w1450:T5)
                    n862 = local read "TDMS LAB02-1"() -> (w1443:refnum<k34>)
                    n863 = Unbundle(w1444) -> ("CYCLE"=w1449:dbl)  [unwired: 2 out]
                    n864 = Unbundle(w1450) -> ("CYCLES"=w1441:dbl, "T-RISE mins"=w1447:dbl)  [unwired: 3 out]
                    n865 = case shown="\"T-RISE TEST\"" w1448 {
                      tunnel: w1447 -> [_ _ w1457]
                      tunnel: [w1452 w1454 w1457] -> w1446
                      tunnel: w1441 -> [w1452 w1454 _]
                      tunnel: ["CHART PASS" "CYCLE PASS" "T-RISE PASS"] -> w1445
                      frame "CHART TEST", Default {
                      }
                      frame "CYCLE TEST" {
                      }
                      frame "T-RISE TEST" {
                      }
                    }
                    n866 = Increment(x=w1441) -> (x+1=w1442:dbl)
                    n867 = Greater Or Equal?(x=w1449, y=w1442) -> (x >= y?=w1451:bool)
                    n868 = case shown="True" w1451 {
                      tunnel: w1446 -> [w1461 _]
                      tunnel: w1445 -> [w1460 _]
                      tunnel: w1444 -> [w1459 _]
                      tunnel: w1443 -> [w1458 _]
                      frame True {
                        n869 = stacked-sequence {
                          tunnel: w1461 -> [w1465 _]
                          tunnel: w1460 -> [w1463 w1469]
                          tunnel: w1459 -> [_ w1472]
                          tunnel: w1458 -> [w1462 _]
                          frame #0 {
                            n870 = Build Array(w1463) -> (w1466:string[])
                            n871 = Build Array(w1465) -> (w1464:dbl[])
                            n872 = TDMS Write(0:w1462, 5:"TEST PASS", 7:w1466, 9:w1464) -> (15:w1468:errorcluster)  [unwired: 2 in, 3 out]
                            n873 = local write "data file error"(w1468) -> ()
                          }
                          frame #1 {
                            n874 = Bundle(cluster=w1472, "STATUS"=w1469) -> (w1470:T4)  [unwired: 2 in]
                            n875 = local write "RESULT LAB02-1"(TRUE) -> ()
                            n876 = local write "DISP LAB02-1"(w1470) -> ()
                          }
                        }
                      }
                      frame False {
                      }
                    }
                  }
                }
              }
              frame #3 {
                # "LAB02-2"
                n877 = Less?(x=w1473, y=2) -> (x < y?=w1476:bool)
                n878 = local read "DISP LAB02-2"() -> (w1478:T4)
                n879 = Unbundle(w1478) -> ("STATUS"=w1479:string)  [unwired: 2 out]
                n880 = Equal?(x=w1479, y="RUN") -> (x = y?=w1475:bool)
                n881 = And(x=w1475, y=w1476) -> (x .and. y?=w1474:bool)
                n882 = case shown="True" w1474 {
                  tunnel: w1478 -> [_ w1484]
                  tunnel: w1473 -> [_ w1488]
                  frame False {
                  }
                  frame True {
                    n883 = local read "SET LAB02-2"() -> (w1490:T5)
                    n884 = local read "TDMS LAB02-2"() -> (w1483:refnum<k34>)
                    n885 = Unbundle(w1484) -> ("CYCLE"=w1489:dbl)  [unwired: 2 out]
                    n886 = Unbundle(w1490) -> ("CYCLES"=w1481:dbl, "T-RISE mins"=w1487:dbl)  [unwired: 3 out]
                    n887 = case shown="\"T-RISE TEST\"" w1488 {
                      tunnel: w1487 -> [_ _ w1497]
                      tunnel: [w1492 w1494 w1497] -> w1486
                      tunnel: w1481 -> [w1492 w1494 _]
                      tunnel: ["CHART PASS" "CYCLE PASS" "T-RISE PASS"] -> w1485
                      frame "CHART TEST", Default {
                      }
                      frame "CYCLE TEST" {
                      }
                      frame "T-RISE TEST" {
                      }
                    }
                    n888 = Increment(x=w1481) -> (x+1=w1482:dbl)
                    n889 = Greater Or Equal?(x=w1489, y=w1482) -> (x >= y?=w1491:bool)
                    n890 = case shown="True" w1491 {
                      tunnel: w1486 -> [w1501 _]
                      tunnel: w1485 -> [w1500 _]
                      tunnel: w1484 -> [w1499 _]
                      tunnel: w1483 -> [w1498 _]
                      frame True {
                        n891 = stacked-sequence {
                          tunnel: w1501 -> [w1505 _]
                          tunnel: w1500 -> [w1503 w1509]
                          tunnel: w1499 -> [_ w1512]
                          tunnel: w1498 -> [w1502 _]
                          frame #0 {
                            n892 = Build Array(w1503) -> (w1506:string[])
                            n893 = Build Array(w1505) -> (w1504:dbl[])
                            n894 = TDMS Write(0:w1502, 5:"TEST PASS", 7:w1506, 9:w1504) -> (15:w1508:errorcluster)  [unwired: 2 in, 3 out]
                            n895 = local write "data file error"(w1508) -> ()
                          }
                          frame #1 {
                            n896 = Bundle(cluster=w1512, "STATUS"=w1509) -> (w1510:T4)  [unwired: 2 in]
                            n897 = local write "RESULT LAB02-2"(TRUE) -> ()
                            n898 = local write "DISP LAB02-2"(w1510) -> ()
                          }
                        }
                      }
                      frame False {
                      }
                    }
                  }
                }
              }
              frame #4 {
                # "LAB03-1"
                n899 = Less?(x=w1513, y=2) -> (x < y?=w1516:bool)
                n900 = local read "DISP LAB03-1"() -> (w1518:T4)
                n901 = Unbundle(w1518) -> ("STATUS"=w1519:string)  [unwired: 2 out]
                n902 = Equal?(x=w1519, y="RUN") -> (x = y?=w1515:bool)
                n903 = And(x=w1515, y=w1516) -> (x .and. y?=w1514:bool)
                n904 = case shown="True" w1514 {
                  tunnel: w1518 -> [_ w1524]
                  tunnel: w1513 -> [_ w1528]
                  frame False {
                  }
                  frame True {
                    n905 = local read "SET LAB03-1"() -> (w1530:T5)
                    n906 = local read "TDMS LAB03-1"() -> (w1523:refnum<k34>)
                    n907 = Unbundle(w1524) -> ("CYCLE"=w1529:dbl)  [unwired: 2 out]
                    n908 = Unbundle(w1530) -> ("CYCLES"=w1521:dbl, "T-RISE mins"=w1527:dbl)  [unwired: 3 out]
                    n909 = case shown="\"T-RISE TEST\"" w1528 {
                      tunnel: w1527 -> [_ _ w1537]
                      tunnel: [w1532 w1534 w1537] -> w1526
                      tunnel: w1521 -> [w1532 w1534 _]
                      tunnel: ["CHART PASS" "CYCLE PASS" "T-RISE PASS"] -> w1525
                      frame "CHART TEST", Default {
                      }
                      frame "CYCLE TEST" {
                      }
                      frame "T-RISE TEST" {
                      }
                    }
                    n910 = Increment(x=w1521) -> (x+1=w1522:dbl)
                    n911 = Greater Or Equal?(x=w1529, y=w1522) -> (x >= y?=w1531:bool)
                    n912 = case shown="True" w1531 {
                      tunnel: w1526 -> [w1541 _]
                      tunnel: w1525 -> [w1540 _]
                      tunnel: w1524 -> [w1539 _]
                      tunnel: w1523 -> [w1538 _]
                      frame True {
                        n913 = stacked-sequence {
                          tunnel: w1541 -> [w1545 _]
                          tunnel: w1540 -> [w1543 w1549]
                          tunnel: w1539 -> [_ w1552]
                          tunnel: w1538 -> [w1542 _]
                          frame #0 {
                            n914 = Build Array(w1543) -> (w1546:string[])
                            n915 = Build Array(w1545) -> (w1544:dbl[])
                            n916 = TDMS Write(0:w1542, 5:"TEST PASS", 7:w1546, 9:w1544) -> (15:w1548:errorcluster)  [unwired: 2 in, 3 out]
                            n917 = local write "data file error"(w1548) -> ()
                          }
                          frame #1 {
                            n918 = Bundle(cluster=w1552, "STATUS"=w1549) -> (w1550:T4)  [unwired: 2 in]
                            n919 = local write "RESULT LAB03-1"(TRUE) -> ()
                            n920 = local write "DISP LAB03-1"(w1550) -> ()
                          }
                        }
                      }
                      frame False {
                      }
                    }
                  }
                }
              }
              frame #5 {
                # "LAB03-2"
                n921 = Less?(x=w1553, y=2) -> (x < y?=w1556:bool)
                n922 = local read "DISP LAB03-2"() -> (w1558:T4)
                n923 = Unbundle(w1558) -> ("STATUS"=w1559:string)  [unwired: 2 out]
                n924 = Equal?(x=w1559, y="RUN") -> (x = y?=w1555:bool)
                n925 = And(x=w1555, y=w1556) -> (x .and. y?=w1554:bool)
                n926 = case shown="True" w1554 {
                  tunnel: w1558 -> [_ w1564]
                  tunnel: w1553 -> [_ w1568]
                  frame False {
                  }
                  frame True {
                    n927 = local read "SET LAB03-2"() -> (w1570:T5)
                    n928 = local read "TDMS LAB03-2"() -> (w1563:refnum<k34>)
                    n929 = Unbundle(w1564) -> ("CYCLE"=w1569:dbl)  [unwired: 2 out]
                    n930 = Unbundle(w1570) -> ("CYCLES"=w1561:dbl, "T-RISE mins"=w1567:dbl)  [unwired: 3 out]
                    n931 = case shown="\"T-RISE TEST\"" w1568 {
                      tunnel: w1567 -> [_ _ w1577]
                      tunnel: [w1572 w1574 w1577] -> w1566
                      tunnel: w1561 -> [w1572 w1574 _]
                      tunnel: ["CHART PASS" "CYCLE PASS" "T-RISE PASS"] -> w1565
                      frame "CHART TEST", Default {
                      }
                      frame "CYCLE TEST" {
                      }
                      frame "T-RISE TEST" {
                      }
                    }
                    n932 = Increment(x=w1561) -> (x+1=w1562:dbl)
                    n933 = Greater Or Equal?(x=w1569, y=w1562) -> (x >= y?=w1571:bool)
                    n934 = case shown="True" w1571 {
                      tunnel: w1566 -> [w1581 _]
                      tunnel: w1565 -> [w1580 _]
                      tunnel: w1564 -> [w1579 _]
                      tunnel: w1563 -> [w1578 _]
                      frame True {
                        n935 = stacked-sequence {
                          tunnel: w1581 -> [w1585 _]
                          tunnel: w1580 -> [w1583 w1589]
                          tunnel: w1579 -> [_ w1592]
                          tunnel: w1578 -> [w1582 _]
                          frame #0 {
                            n936 = Build Array(w1583) -> (w1586:string[])
                            n937 = Build Array(w1585) -> (w1584:dbl[])
                            n938 = TDMS Write(0:w1582, 5:"TEST PASS", 7:w1586, 9:w1584) -> (15:w1588:errorcluster)  [unwired: 2 in, 3 out]
                            n939 = local write "data file error"(w1588) -> ()
                          }
                          frame #1 {
                            n940 = Bundle(cluster=w1592, "STATUS"=w1589) -> (w1590:T4)  [unwired: 2 in]
                            n941 = local write "RESULT LAB03-2"(TRUE) -> ()
                            n942 = local write "DISP LAB03-2"(w1590) -> ()
                          }
                        }
                      }
                      frame False {
                      }
                    }
                  }
                }
              }
              frame #6 {
                # "LAB04-1"
                n943 = Less?(x=w1593, y=2) -> (x < y?=w1596:bool)
                n944 = local read "DISP LAB04-1"() -> (w1598:T4)
                n945 = Unbundle(w1598) -> ("STATUS"=w1599:string)  [unwired: 2 out]
                n946 = Equal?(x=w1599, y="RUN") -> (x = y?=w1595:bool)
                n947 = And(x=w1595, y=w1596) -> (x .and. y?=w1594:bool)
                n948 = case shown="True" w1594 {
                  tunnel: w1598 -> [_ w1604]
                  tunnel: w1593 -> [_ w1608]
                  frame False {
                  }
                  frame True {
                    n949 = local read "SET LAB04-1"() -> (w1610:T5)
                    n950 = local read "TDMS LAB04-1"() -> (w1603:refnum<k34>)
                    n951 = Unbundle(w1604) -> ("CYCLE"=w1609:dbl)  [unwired: 2 out]
                    n952 = Unbundle(w1610) -> ("CYCLES"=w1601:dbl, "T-RISE mins"=w1607:dbl)  [unwired: 3 out]
                    n953 = case shown="\"T-RISE TEST\"" w1608 {
                      tunnel: w1607 -> [_ _ w1617]
                      tunnel: [w1612 w1614 w1617] -> w1606
                      tunnel: w1601 -> [w1612 w1614 _]
                      tunnel: ["CHART PASS" "CYCLE PASS" "T-RISE PASS"] -> w1605
                      frame "CHART TEST", Default {
                      }
                      frame "CYCLE TEST" {
                      }
                      frame "T-RISE TEST" {
                      }
                    }
                    n954 = Increment(x=w1601) -> (x+1=w1602:dbl)
                    n955 = Greater Or Equal?(x=w1609, y=w1602) -> (x >= y?=w1611:bool)
                    n956 = case shown="True" w1611 {
                      tunnel: w1606 -> [w1621 _]
                      tunnel: w1605 -> [w1620 _]
                      tunnel: w1604 -> [w1619 _]
                      tunnel: w1603 -> [w1618 _]
                      frame True {
                        n957 = stacked-sequence {
                          tunnel: w1621 -> [w1625 _]
                          tunnel: w1620 -> [w1623 w1629]
                          tunnel: w1619 -> [_ w1632]
                          tunnel: w1618 -> [w1622 _]
                          frame #0 {
                            n958 = Build Array(w1623) -> (w1626:string[])
                            n959 = Build Array(w1625) -> (w1624:dbl[])
                            n960 = TDMS Write(0:w1622, 5:"TEST PASS", 7:w1626, 9:w1624) -> (15:w1628:errorcluster)  [unwired: 2 in, 3 out]
                            n961 = local write "data file error"(w1628) -> ()
                          }
                          frame #1 {
                            n962 = Bundle(cluster=w1632, "STATUS"=w1629) -> (w1630:T4)  [unwired: 2 in]
                            n963 = local write "RESULT LAB04-1"(TRUE) -> ()
                            n964 = local write "DISP LAB04-1"(w1630) -> ()
                          }
                        }
                      }
                      frame False {
                      }
                    }
                  }
                }
              }
              frame #7 {
                # "LAB04-2"
                n965 = Less?(x=w1633, y=2) -> (x < y?=w1636:bool)
                n966 = local read "DISP LAB04-2"() -> (w1638:T4)
                n967 = Unbundle(w1638) -> ("STATUS"=w1639:string)  [unwired: 2 out]
                n968 = Equal?(x=w1639, y="RUN") -> (x = y?=w1635:bool)
                n969 = And(x=w1635, y=w1636) -> (x .and. y?=w1634:bool)
                n970 = case shown="True" w1634 {
                  tunnel: w1638 -> [_ w1644]
                  tunnel: w1633 -> [_ w1648]
                  frame False {
                  }
                  frame True {
                    n971 = local read "SET LAB04-2"() -> (w1650:T5)
                    n972 = local read "TDMS LAB04-2"() -> (w1643:refnum<k34>)
                    n973 = Unbundle(w1644) -> ("CYCLE"=w1649:dbl)  [unwired: 2 out]
                    n974 = Unbundle(w1650) -> ("CYCLES"=w1641:dbl, "T-RISE mins"=w1647:dbl)  [unwired: 3 out]
                    n975 = case shown="\"T-RISE TEST\"" w1648 {
                      tunnel: w1647 -> [_ _ w1657]
                      tunnel: [w1652 w1654 w1657] -> w1646
                      tunnel: w1641 -> [w1652 w1654 _]
                      tunnel: ["CHART PASS" "CYCLE PASS" "T-RISE PASS"] -> w1645
                      frame "CHART TEST", Default {
                      }
                      frame "CYCLE TEST" {
                      }
                      frame "T-RISE TEST" {
                      }
                    }
                    n976 = Increment(x=w1641) -> (x+1=w1642:dbl)
                    n977 = Greater Or Equal?(x=w1649, y=w1642) -> (x >= y?=w1651:bool)
                    n978 = case shown="True" w1651 {
                      tunnel: w1646 -> [w1661 _]
                      tunnel: w1645 -> [w1660 _]
                      tunnel: w1644 -> [w1659 _]
                      tunnel: w1643 -> [w1658 _]
                      frame True {
                        n979 = stacked-sequence {
                          tunnel: w1661 -> [w1665 _]
                          tunnel: w1660 -> [w1663 w1669]
                          tunnel: w1659 -> [_ w1672]
                          tunnel: w1658 -> [w1662 _]
                          frame #0 {
                            n980 = Build Array(w1663) -> (w1666:string[])
                            n981 = Build Array(w1665) -> (w1664:dbl[])
                            n982 = TDMS Write(0:w1662, 5:"TEST PASS", 7:w1666, 9:w1664) -> (15:w1668:errorcluster)  [unwired: 2 in, 3 out]
                            n983 = local write "data file error"(w1668) -> ()
                          }
                          frame #1 {
                            n984 = Bundle(cluster=w1672, "STATUS"=w1669) -> (w1670:T4)  [unwired: 2 in]
                            n985 = local write "RESULT LAB04-2"(TRUE) -> ()
                            n986 = local write "DISP LAB04-2"(w1670) -> ()
                          }
                        }
                      }
                      frame False {
                      }
                    }
                  }
                }
              }
              frame #8 {
                # "LAB05-1"
                n987 = Less?(x=w1673, y=2) -> (x < y?=w1676:bool)
                n988 = local read "DISP LAB05-1"() -> (w1678:T4)
                n989 = Unbundle(w1678) -> ("STATUS"=w1679:string)  [unwired: 2 out]
                n990 = Equal?(x=w1679, y="RUN") -> (x = y?=w1675:bool)
                n991 = And(x=w1675, y=w1676) -> (x .and. y?=w1674:bool)
                n992 = case shown="True" w1674 {
                  tunnel: w1678 -> [_ w1684]
                  tunnel: w1673 -> [_ w1688]
                  frame False {
                  }
                  frame True {
                    n993 = local read "SET LAB05-1"() -> (w1690:T5)
                    n994 = local read "TDMS LAB05-1"() -> (w1683:refnum<k34>)
                    n995 = Unbundle(w1684) -> ("CYCLE"=w1689:dbl)  [unwired: 2 out]
                    n996 = Unbundle(w1690) -> ("CYCLES"=w1681:dbl, "T-RISE mins"=w1687:dbl)  [unwired: 3 out]
                    n997 = case shown="\"T-RISE TEST\"" w1688 {
                      tunnel: w1687 -> [_ _ w1697]
                      tunnel: [w1692 w1694 w1697] -> w1686
                      tunnel: w1681 -> [w1692 w1694 _]
                      tunnel: ["CHART PASS" "CYCLE PASS" "T-RISE PASS"] -> w1685
                      frame "CHART TEST", Default {
                      }
                      frame "CYCLE TEST" {
                      }
                      frame "T-RISE TEST" {
                      }
                    }
                    n998 = Increment(x=w1681) -> (x+1=w1682:dbl)
                    n999 = Greater Or Equal?(x=w1689, y=w1682) -> (x >= y?=w1691:bool)
                    n1000 = case shown="True" w1691 {
                      tunnel: w1686 -> [w1701 _]
                      tunnel: w1685 -> [w1700 _]
                      tunnel: w1684 -> [w1699 _]
                      tunnel: w1683 -> [w1698 _]
                      frame True {
                        n1001 = stacked-sequence {
                          tunnel: w1701 -> [w1705 _]
                          tunnel: w1700 -> [w1703 w1709]
                          tunnel: w1699 -> [_ w1712]
                          tunnel: w1698 -> [w1702 _]
                          frame #0 {
                            n1002 = Build Array(w1703) -> (w1706:string[])
                            n1003 = Build Array(w1705) -> (w1704:dbl[])
                            n1004 = TDMS Write(0:w1702, 5:"TEST PASS", 7:w1706, 9:w1704) -> (15:w1708:errorcluster)  [unwired: 2 in, 3 out]
                            n1005 = local write "data file error"(w1708) -> ()
                          }
                          frame #1 {
                            n1006 = Bundle(cluster=w1712, "STATUS"=w1709) -> (w1710:T4)  [unwired: 2 in]
                            n1007 = local write "RESULT LAB05-1"(TRUE) -> ()
                            n1008 = local write "DISP LAB05-1"(w1710) -> ()
                          }
                        }
                      }
                      frame False {
                      }
                    }
                  }
                }
              }
              frame #9 {
                # "LAB05-2"
                n1009 = Less?(x=w1713, y=2) -> (x < y?=w1716:bool)
                n1010 = local read "DISP LAB05-2"() -> (w1718:T4)
                n1011 = Unbundle(w1718) -> ("STATUS"=w1719:string)  [unwired: 2 out]
                n1012 = Equal?(x=w1719, y="RUN") -> (x = y?=w1715:bool)
                n1013 = And(x=w1715, y=w1716) -> (x .and. y?=w1714:bool)
                n1014 = case shown="True" w1714 {
                  tunnel: w1718 -> [_ w1724]
                  tunnel: w1713 -> [_ w1728]
                  frame False {
                  }
                  frame True {
                    n1015 = local read "SET LAB05-2"() -> (w1730:T5)
                    n1016 = local read "TDMS LAB05-2"() -> (w1723:refnum<k34>)
                    n1017 = Unbundle(w1724) -> ("CYCLE"=w1729:dbl)  [unwired: 2 out]
                    n1018 = Unbundle(w1730) -> ("CYCLES"=w1721:dbl, "T-RISE mins"=w1727:dbl)  [unwired: 3 out]
                    n1019 = case shown="\"T-RISE TEST\"" w1728 {
                      tunnel: w1727 -> [_ _ w1737]
                      tunnel: [w1732 w1734 w1737] -> w1726
                      tunnel: w1721 -> [w1732 w1734 _]
                      tunnel: ["CHART PASS" "CYCLE PASS" "T-RISE PASS"] -> w1725
                      frame "CHART TEST", Default {
                      }
                      frame "CYCLE TEST" {
                      }
                      frame "T-RISE TEST" {
                      }
                    }
                    n1020 = Increment(x=w1721) -> (x+1=w1722:dbl)
                    n1021 = Greater Or Equal?(x=w1729, y=w1722) -> (x >= y?=w1731:bool)
                    n1022 = case shown="True" w1731 {
                      tunnel: w1726 -> [w1741 _]
                      tunnel: w1725 -> [w1740 _]
                      tunnel: w1724 -> [w1739 _]
                      tunnel: w1723 -> [w1738 _]
                      frame True {
                        n1023 = stacked-sequence {
                          tunnel: w1741 -> [w1745 _]
                          tunnel: w1740 -> [w1743 w1749]
                          tunnel: w1739 -> [_ w1752]
                          tunnel: w1738 -> [w1742 _]
                          frame #0 {
                            n1024 = Build Array(w1743) -> (w1746:string[])
                            n1025 = Build Array(w1745) -> (w1744:dbl[])
                            n1026 = TDMS Write(0:w1742, 5:"TEST PASS", 7:w1746, 9:w1744) -> (15:w1748:errorcluster)  [unwired: 2 in, 3 out]
                            n1027 = local write "data file error"(w1748) -> ()
                          }
                          frame #1 {
                            n1028 = Bundle(cluster=w1752, "STATUS"=w1749) -> (w1750:T4)  [unwired: 2 in]
                            n1029 = local write "RESULT LAB05-2"(TRUE) -> ()
                            n1030 = local write "DISP LAB05-2"(w1750) -> ()
                          }
                        }
                      }
                      frame False {
                      }
                    }
                  }
                }
              }
            }
          }
          frame #5 {
            # "check if test cycles reached for temperature rise test"
            n1031 = stacked-sequence {
              tunnel: w1782 -> [_ _ _ _ _ _ _ _ _ _]
              tunnel: w1781 -> [_ _ _ _ _ _ _ _ _ _]
              tunnel: w1780 -> [_ _ _ _ _ _ _ _ _ _]
              tunnel: w1779 -> [_ _ _ _ _ _ _ _ _ _]
              tunnel: w1778 -> [_ _ _ _ _ _ _ _ _ _]
              tunnel: w1777 -> [_ _ _ _ _ _ _ _ _ _]
              tunnel: w1776 -> [_ _ _ _ _ _ _ _ _ _]
              tunnel: w1775 -> [_ _ _ _ _ _ _ _ _ _]
              tunnel: w1774 -> [_ _ _ _ _ _ _ _ _ _]
              tunnel: w1773 -> [_ _ _ _ _ _ _ _ _ _]
              tunnel: w1772 -> [w1788 _ _ _ _ _ _ _ _ _]
              tunnel: w1762 -> [w1783 _ _ _ _ _ _ _ _ _]
              tunnel: w1771 -> [_ w1814 _ _ _ _ _ _ _ _]
              tunnel: w1770 -> [_ _ w1844 _ _ _ _ _ _ _]
              tunnel: w1769 -> [_ _ _ w1874 _ _ _ _ _ _]
              tunnel: w1768 -> [_ _ _ _ w1904 _ _ _ _ _]
              tunnel: w1767 -> [_ _ _ _ _ w1934 _ _ _ _]
              tunnel: w1766 -> [_ _ _ _ _ _ w1964 _ _ _]
              tunnel: w1765 -> [_ _ _ _ _ _ _ w1994 _ _]
              tunnel: w1764 -> [_ _ _ _ _ _ _ _ w2024 _]
              tunnel: w1763 -> [_ _ _ _ _ _ _ _ _ w2054]
              tunnel: w1761 -> [_ w1813 _ _ _ _ _ _ _ _]
              tunnel: w1760 -> [_ _ w1843 _ _ _ _ _ _ _]
              tunnel: w1759 -> [_ _ _ w1873 _ _ _ _ _ _]
              tunnel: w1758 -> [_ _ _ _ w1903 _ _ _ _ _]
              tunnel: w1757 -> [_ _ _ _ _ w1933 _ _ _ _]
              tunnel: w1756 -> [_ _ _ _ _ _ w1963 _ _ _]
              tunnel: w1755 -> [_ _ _ _ _ _ _ w1993 _ _]
              tunnel: w1754 -> [_ _ _ _ _ _ _ _ w2023 _]
              tunnel: w1753 -> [_ _ _ _ _ _ _ _ _ w2053]
              frame #0 {
                # "LAB01-1"
                n1032 = Equal?(x=w1788, y=2) -> (x = y?=w1786:bool)
                n1033 = local read "DISP LAB01-1"() -> (w1789:T4)
                n1034 = Unbundle(w1789) -> ("STATUS"=w1790:string)  [unwired: 2 out]
                n1035 = Equal?(x=w1790, y="RUN") -> (x = y?=w1785:bool)
                n1036 = And(x=w1785, y=w1786) -> (x .and. y?=w1784:bool)
                n1037 = case shown="True" w1784 {
                  tunnel: w1789 -> [_ w1793]
                  tunnel: w1783 -> [_ w1796]
                  frame False {
                  }
                  frame True {
                    n1038 = local read "SET LAB01-1"() -> (w1795:T5)
                    n1039 = local read "TDMS LAB01-1"() -> (w1792:refnum<k34>)
                    n1040 = Unbundle(w1793) -> ("CYCLE"=w1797:dbl)  [unwired: 2 out]
                    n1041 = Unbundle(w1795) -> ("T-RISE mins"=w1794:dbl)  [unwired: 4 out]
                    n1042 = Greater Or Equal?(x=w1797, y=w1796) -> (x >= y?=w1798:bool)
                    n1043 = case shown="True" w1798 {
                      tunnel: w1794 -> [w1801 _]
                      tunnel: w1793 -> [w1800 _]
                      tunnel: w1792 -> [w1799 _]
                      frame True {
                        n1044 = stacked-sequence {
                          tunnel: w1801 -> [w1804 _]
                          tunnel: w1800 -> [_ w1809]
                          tunnel: w1799 -> [w1802 _]
                          frame #0 {
                            n1045 = Build Array("T-RISE") -> (w1806:string[])
                            n1046 = Build Array(w1804) -> (w1805:dbl[])
                            n1047 = TDMS Write(0:w1802, 5:"TEST PASS", 7:w1806, 9:w1805) -> (15:w1808:errorcluster)  [unwired: 2 in, 3 out]
                            n1048 = local write "data file error"(w1808) -> ()
                          }
                          frame #1 {
                            n1049 = Bundle(cluster=w1809, "STATUS"="T-RISE PASS") -> (w1811:T4)  [unwired: 2 in]
                            n1050 = local write "RESULT LAB01-1"(TRUE) -> ()
                            n1051 = local write "DISP LAB01-1"(w1811) -> ()
                          }
                        }
                      }
                      frame False {
                      }
                    }
                  }
                }
              }
              frame #1 {
                # "LAB01-2"
                n1052 = Equal?(x=w1814, y=2) -> (x = y?=w1817:bool)
                n1053 = local read "DISP LAB01-2"() -> (w1819:T4)
                n1054 = Unbundle(w1819) -> ("STATUS"=w1820:string)  [unwired: 2 out]
                n1055 = Equal?(x=w1820, y="RUN") -> (x = y?=w1816:bool)
                n1056 = And(x=w1816, y=w1817) -> (x .and. y?=w1815:bool)
                n1057 = case shown="True" w1815 {
                  tunnel: w1819 -> [_ w1823]
                  tunnel: w1813 -> [_ w1826]
                  frame False {
                  }
                  frame True {
                    n1058 = local read "SET LAB01-2"() -> (w1825:T5)
                    n1059 = local read "TDMS LAB01-2"() -> (w1822:refnum<k34>)
                    n1060 = Unbundle(w1823) -> ("CYCLE"=w1827:dbl)  [unwired: 2 out]
                    n1061 = Unbundle(w1825) -> ("T-RISE mins"=w1824:dbl)  [unwired: 4 out]
                    n1062 = Greater Or Equal?(x=w1827, y=w1826) -> (x >= y?=w1828:bool)
                    n1063 = case shown="True" w1828 {
                      tunnel: w1824 -> [w1831 _]
                      tunnel: w1823 -> [w1830 _]
                      tunnel: w1822 -> [w1829 _]
                      frame True {
                        n1064 = stacked-sequence {
                          tunnel: w1831 -> [w1834 _]
                          tunnel: w1830 -> [_ w1839]
                          tunnel: w1829 -> [w1832 _]
                          frame #0 {
                            n1065 = Build Array("T-RISE") -> (w1836:string[])
                            n1066 = Build Array(w1834) -> (w1835:dbl[])
                            n1067 = TDMS Write(0:w1832, 5:"TEST PASS", 7:w1836, 9:w1835) -> (15:w1838:errorcluster)  [unwired: 2 in, 3 out]
                            n1068 = local write "data file error"(w1838) -> ()
                          }
                          frame #1 {
                            n1069 = Bundle(cluster=w1839, "STATUS"="T-RISE PASS") -> (w1841:T4)  [unwired: 2 in]
                            n1070 = local write "RESULT LAB01-2"(TRUE) -> ()
                            n1071 = local write "DISP LAB01-2"(w1841) -> ()
                          }
                        }
                      }
                      frame False {
                      }
                    }
                  }
                }
              }
              frame #2 {
                # "LAB02-1"
                n1072 = Equal?(x=w1844, y=2) -> (x = y?=w1847:bool)
                n1073 = local read "DISP LAB02-1"() -> (w1849:T4)
                n1074 = Unbundle(w1849) -> ("STATUS"=w1850:string)  [unwired: 2 out]
                n1075 = Equal?(x=w1850, y="RUN") -> (x = y?=w1846:bool)
                n1076 = And(x=w1846, y=w1847) -> (x .and. y?=w1845:bool)
                n1077 = case shown="True" w1845 {
                  tunnel: w1849 -> [_ w1853]
                  tunnel: w1843 -> [_ w1856]
                  frame False {
                  }
                  frame True {
                    n1078 = local read "SET LAB02-1"() -> (w1855:T5)
                    n1079 = local read "TDMS LAB02-1"() -> (w1852:refnum<k34>)
                    n1080 = Unbundle(w1853) -> ("CYCLE"=w1857:dbl)  [unwired: 2 out]
                    n1081 = Unbundle(w1855) -> ("T-RISE mins"=w1854:dbl)  [unwired: 4 out]
                    n1082 = Greater Or Equal?(x=w1857, y=w1856) -> (x >= y?=w1858:bool)
                    n1083 = case shown="True" w1858 {
                      tunnel: w1854 -> [w1861 _]
                      tunnel: w1853 -> [w1860 _]
                      tunnel: w1852 -> [w1859 _]
                      frame True {
                        n1084 = stacked-sequence {
                          tunnel: w1861 -> [w1864 _]
                          tunnel: w1860 -> [_ w1869]
                          tunnel: w1859 -> [w1862 _]
                          frame #0 {
                            n1085 = Build Array("T-RISE") -> (w1866:string[])
                            n1086 = Build Array(w1864) -> (w1865:dbl[])
                            n1087 = TDMS Write(0:w1862, 5:"TEST PASS", 7:w1866, 9:w1865) -> (15:w1868:errorcluster)  [unwired: 2 in, 3 out]
                            n1088 = local write "data file error"(w1868) -> ()
                          }
                          frame #1 {
                            n1089 = Bundle(cluster=w1869, "STATUS"="T-RISE PASS") -> (w1871:T4)  [unwired: 2 in]
                            n1090 = local write "RESULT LAB02-1"(TRUE) -> ()
                            n1091 = local write "DISP LAB02-1"(w1871) -> ()
                          }
                        }
                      }
                      frame False {
                      }
                    }
                  }
                }
              }
              frame #3 {
                # "LAB02-2"
                n1092 = Equal?(x=w1874, y=2) -> (x = y?=w1877:bool)
                n1093 = local read "DISP LAB02-2"() -> (w1879:T4)
                n1094 = Unbundle(w1879) -> ("STATUS"=w1880:string)  [unwired: 2 out]
                n1095 = Equal?(x=w1880, y="RUN") -> (x = y?=w1876:bool)
                n1096 = And(x=w1876, y=w1877) -> (x .and. y?=w1875:bool)
                n1097 = case shown="True" w1875 {
                  tunnel: w1879 -> [_ w1883]
                  tunnel: w1873 -> [_ w1886]
                  frame False {
                  }
                  frame True {
                    n1098 = local read "SET LAB02-2"() -> (w1885:T5)
                    n1099 = local read "TDMS LAB02-2"() -> (w1882:refnum<k34>)
                    n1100 = Unbundle(w1883) -> ("CYCLE"=w1887:dbl)  [unwired: 2 out]
                    n1101 = Unbundle(w1885) -> ("T-RISE mins"=w1884:dbl)  [unwired: 4 out]
                    n1102 = Greater Or Equal?(x=w1887, y=w1886) -> (x >= y?=w1888:bool)
                    n1103 = case shown="True" w1888 {
                      tunnel: w1884 -> [w1891 _]
                      tunnel: w1883 -> [w1890 _]
                      tunnel: w1882 -> [w1889 _]
                      frame True {
                        n1104 = stacked-sequence {
                          tunnel: w1891 -> [w1894 _]
                          tunnel: w1890 -> [_ w1899]
                          tunnel: w1889 -> [w1892 _]
                          frame #0 {
                            n1105 = Build Array("T-RISE") -> (w1896:string[])
                            n1106 = Build Array(w1894) -> (w1895:dbl[])
                            n1107 = TDMS Write(0:w1892, 5:"TEST PASS", 7:w1896, 9:w1895) -> (15:w1898:errorcluster)  [unwired: 2 in, 3 out]
                            n1108 = local write "data file error"(w1898) -> ()
                          }
                          frame #1 {
                            n1109 = Bundle(cluster=w1899, "STATUS"="T-RISE PASS") -> (w1901:T4)  [unwired: 2 in]
                            n1110 = local write "RESULT LAB02-2"(TRUE) -> ()
                            n1111 = local write "DISP LAB02-2"(w1901) -> ()
                          }
                        }
                      }
                      frame False {
                      }
                    }
                  }
                }
              }
              frame #4 {
                # "LAB03-1"
                n1112 = Equal?(x=w1904, y=2) -> (x = y?=w1907:bool)
                n1113 = local read "DISP LAB03-1"() -> (w1909:T4)
                n1114 = Unbundle(w1909) -> ("STATUS"=w1910:string)  [unwired: 2 out]
                n1115 = Equal?(x=w1910, y="RUN") -> (x = y?=w1906:bool)
                n1116 = And(x=w1906, y=w1907) -> (x .and. y?=w1905:bool)
                n1117 = case shown="True" w1905 {
                  tunnel: w1909 -> [_ w1913]
                  tunnel: w1903 -> [_ w1916]
                  frame False {
                  }
                  frame True {
                    n1118 = local read "SET LAB03-1"() -> (w1915:T5)
                    n1119 = local read "TDMS LAB03-1"() -> (w1912:refnum<k34>)
                    n1120 = Unbundle(w1913) -> ("CYCLE"=w1917:dbl)  [unwired: 2 out]
                    n1121 = Unbundle(w1915) -> ("T-RISE mins"=w1914:dbl)  [unwired: 4 out]
                    n1122 = Greater Or Equal?(x=w1917, y=w1916) -> (x >= y?=w1918:bool)
                    n1123 = case shown="True" w1918 {
                      tunnel: w1914 -> [w1921 _]
                      tunnel: w1913 -> [w1920 _]
                      tunnel: w1912 -> [w1919 _]
                      frame True {
                        n1124 = stacked-sequence {
                          tunnel: w1921 -> [w1924 _]
                          tunnel: w1920 -> [_ w1929]
                          tunnel: w1919 -> [w1922 _]
                          frame #0 {
                            n1125 = Build Array("T-RISE") -> (w1926:string[])
                            n1126 = Build Array(w1924) -> (w1925:dbl[])
                            n1127 = TDMS Write(0:w1922, 5:"TEST PASS", 7:w1926, 9:w1925) -> (15:w1928:errorcluster)  [unwired: 2 in, 3 out]
                            n1128 = local write "data file error"(w1928) -> ()
                          }
                          frame #1 {
                            n1129 = Bundle(cluster=w1929, "STATUS"="T-RISE PASS") -> (w1931:T4)  [unwired: 2 in]
                            n1130 = local write "RESULT LAB03-1"(TRUE) -> ()
                            n1131 = local write "DISP LAB03-1"(w1931) -> ()
                          }
                        }
                      }
                      frame False {
                      }
                    }
                  }
                }
              }
              frame #5 {
                # "LAB03-2"
                n1132 = Equal?(x=w1934, y=2) -> (x = y?=w1937:bool)
                n1133 = local read "DISP LAB03-2"() -> (w1939:T4)
                n1134 = Unbundle(w1939) -> ("STATUS"=w1940:string)  [unwired: 2 out]
                n1135 = Equal?(x=w1940, y="RUN") -> (x = y?=w1936:bool)
                n1136 = And(x=w1936, y=w1937) -> (x .and. y?=w1935:bool)
                n1137 = case shown="True" w1935 {
                  tunnel: w1939 -> [_ w1943]
                  tunnel: w1933 -> [_ w1946]
                  frame False {
                  }
                  frame True {
                    n1138 = local read "SET LAB03-2"() -> (w1945:T5)
                    n1139 = local read "TDMS LAB03-2"() -> (w1942:refnum<k34>)
                    n1140 = Unbundle(w1943) -> ("CYCLE"=w1947:dbl)  [unwired: 2 out]
                    n1141 = Unbundle(w1945) -> ("T-RISE mins"=w1944:dbl)  [unwired: 4 out]
                    n1142 = Greater Or Equal?(x=w1947, y=w1946) -> (x >= y?=w1948:bool)
                    n1143 = case shown="True" w1948 {
                      tunnel: w1944 -> [w1951 _]
                      tunnel: w1943 -> [w1950 _]
                      tunnel: w1942 -> [w1949 _]
                      frame True {
                        n1144 = stacked-sequence {
                          tunnel: w1951 -> [w1954 _]
                          tunnel: w1950 -> [_ w1959]
                          tunnel: w1949 -> [w1952 _]
                          frame #0 {
                            n1145 = Build Array("T-RISE") -> (w1956:string[])
                            n1146 = Build Array(w1954) -> (w1955:dbl[])
                            n1147 = TDMS Write(0:w1952, 5:"TEST PASS", 7:w1956, 9:w1955) -> (15:w1958:errorcluster)  [unwired: 2 in, 3 out]
                            n1148 = local write "data file error"(w1958) -> ()
                          }
                          frame #1 {
                            n1149 = Bundle(cluster=w1959, "STATUS"="T-RISE PASS") -> (w1961:T4)  [unwired: 2 in]
                            n1150 = local write "RESULT LAB03-2"(TRUE) -> ()
                            n1151 = local write "DISP LAB03-2"(w1961) -> ()
                          }
                        }
                      }
                      frame False {
                      }
                    }
                  }
                }
              }
              frame #6 {
                # "LAB04-1"
                n1152 = Equal?(x=w1964, y=2) -> (x = y?=w1967:bool)
                n1153 = local read "DISP LAB04-1"() -> (w1969:T4)
                n1154 = Unbundle(w1969) -> ("STATUS"=w1970:string)  [unwired: 2 out]
                n1155 = Equal?(x=w1970, y="RUN") -> (x = y?=w1966:bool)
                n1156 = And(x=w1966, y=w1967) -> (x .and. y?=w1965:bool)
                n1157 = case shown="True" w1965 {
                  tunnel: w1969 -> [_ w1973]
                  tunnel: w1963 -> [_ w1976]
                  frame False {
                  }
                  frame True {
                    n1158 = local read "SET LAB04-1"() -> (w1975:T5)
                    n1159 = local read "TDMS LAB04-1"() -> (w1972:refnum<k34>)
                    n1160 = Unbundle(w1973) -> ("CYCLE"=w1977:dbl)  [unwired: 2 out]
                    n1161 = Unbundle(w1975) -> ("T-RISE mins"=w1974:dbl)  [unwired: 4 out]
                    n1162 = Greater Or Equal?(x=w1977, y=w1976) -> (x >= y?=w1978:bool)
                    n1163 = case shown="True" w1978 {
                      tunnel: w1974 -> [w1981 _]
                      tunnel: w1973 -> [w1980 _]
                      tunnel: w1972 -> [w1979 _]
                      frame True {
                        n1164 = stacked-sequence {
                          tunnel: w1981 -> [w1984 _]
                          tunnel: w1980 -> [_ w1989]
                          tunnel: w1979 -> [w1982 _]
                          frame #0 {
                            n1165 = Build Array("T-RISE") -> (w1986:string[])
                            n1166 = Build Array(w1984) -> (w1985:dbl[])
                            n1167 = TDMS Write(0:w1982, 5:"TEST PASS", 7:w1986, 9:w1985) -> (15:w1988:errorcluster)  [unwired: 2 in, 3 out]
                            n1168 = local write "data file error"(w1988) -> ()
                          }
                          frame #1 {
                            n1169 = Bundle(cluster=w1989, "STATUS"="T-RISE PASS") -> (w1991:T4)  [unwired: 2 in]
                            n1170 = local write "RESULT LAB04-1"(TRUE) -> ()
                            n1171 = local write "DISP LAB04-1"(w1991) -> ()
                          }
                        }
                      }
                      frame False {
                      }
                    }
                  }
                }
              }
              frame #7 {
                # "LAB04-2"
                n1172 = Equal?(x=w1994, y=2) -> (x = y?=w1997:bool)
                n1173 = local read "DISP LAB04-2"() -> (w1999:T4)
                n1174 = Unbundle(w1999) -> ("STATUS"=w2000:string)  [unwired: 2 out]
                n1175 = Equal?(x=w2000, y="RUN") -> (x = y?=w1996:bool)
                n1176 = And(x=w1996, y=w1997) -> (x .and. y?=w1995:bool)
                n1177 = case shown="True" w1995 {
                  tunnel: w1999 -> [_ w2003]
                  tunnel: w1993 -> [_ w2006]
                  frame False {
                  }
                  frame True {
                    n1178 = local read "SET LAB04-2"() -> (w2005:T5)
                    n1179 = local read "TDMS LAB04-2"() -> (w2002:refnum<k34>)
                    n1180 = Unbundle(w2003) -> ("CYCLE"=w2007:dbl)  [unwired: 2 out]
                    n1181 = Unbundle(w2005) -> ("T-RISE mins"=w2004:dbl)  [unwired: 4 out]
                    n1182 = Greater Or Equal?(x=w2007, y=w2006) -> (x >= y?=w2008:bool)
                    n1183 = case shown="True" w2008 {
                      tunnel: w2004 -> [w2011 _]
                      tunnel: w2003 -> [w2010 _]
                      tunnel: w2002 -> [w2009 _]
                      frame True {
                        n1184 = stacked-sequence {
                          tunnel: w2011 -> [w2014 _]
                          tunnel: w2010 -> [_ w2019]
                          tunnel: w2009 -> [w2012 _]
                          frame #0 {
                            n1185 = Build Array("T-RISE") -> (w2016:string[])
                            n1186 = Build Array(w2014) -> (w2015:dbl[])
                            n1187 = TDMS Write(0:w2012, 5:"TEST PASS", 7:w2016, 9:w2015) -> (15:w2018:errorcluster)  [unwired: 2 in, 3 out]
                            n1188 = local write "data file error"(w2018) -> ()
                          }
                          frame #1 {
                            n1189 = Bundle(cluster=w2019, "STATUS"="T-RISE PASS") -> (w2021:T4)  [unwired: 2 in]
                            n1190 = local write "RESULT LAB04-2"(TRUE) -> ()
                            n1191 = local write "DISP LAB04-2"(w2021) -> ()
                          }
                        }
                      }
                      frame False {
                      }
                    }
                  }
                }
              }
              frame #8 {
                # "LAB05-1"
                n1192 = Equal?(x=w2024, y=2) -> (x = y?=w2027:bool)
                n1193 = local read "DISP LAB05-1"() -> (w2029:T4)
                n1194 = Unbundle(w2029) -> ("STATUS"=w2030:string)  [unwired: 2 out]
                n1195 = Equal?(x=w2030, y="RUN") -> (x = y?=w2026:bool)
                n1196 = And(x=w2026, y=w2027) -> (x .and. y?=w2025:bool)
                n1197 = case shown="True" w2025 {
                  tunnel: w2029 -> [_ w2033]
                  tunnel: w2023 -> [_ w2036]
                  frame False {
                  }
                  frame True {
                    n1198 = local read "SET LAB05-1"() -> (w2035:T5)
                    n1199 = local read "TDMS LAB05-1"() -> (w2032:refnum<k34>)
                    n1200 = Unbundle(w2033) -> ("CYCLE"=w2037:dbl)  [unwired: 2 out]
                    n1201 = Unbundle(w2035) -> ("T-RISE mins"=w2034:dbl)  [unwired: 4 out]
                    n1202 = Greater Or Equal?(x=w2037, y=w2036) -> (x >= y?=w2038:bool)
                    n1203 = case shown="True" w2038 {
                      tunnel: w2034 -> [w2041 _]
                      tunnel: w2033 -> [w2040 _]
                      tunnel: w2032 -> [w2039 _]
                      frame True {
                        n1204 = stacked-sequence {
                          tunnel: w2041 -> [w2044 _]
                          tunnel: w2040 -> [_ w2049]
                          tunnel: w2039 -> [w2042 _]
                          frame #0 {
                            n1205 = Build Array("T-RISE") -> (w2046:string[])
                            n1206 = Build Array(w2044) -> (w2045:dbl[])
                            n1207 = TDMS Write(0:w2042, 5:"TEST PASS", 7:w2046, 9:w2045) -> (15:w2048:errorcluster)  [unwired: 2 in, 3 out]
                            n1208 = local write "data file error"(w2048) -> ()
                          }
                          frame #1 {
                            n1209 = Bundle(cluster=w2049, "STATUS"="T-RISE PASS") -> (w2051:T4)  [unwired: 2 in]
                            n1210 = local write "RESULT LAB05-1"(TRUE) -> ()
                            n1211 = local write "DISP LAB05-1"(w2051) -> ()
                          }
                        }
                      }
                      frame False {
                      }
                    }
                  }
                }
              }
              frame #9 {
                # "LAB05-2"
                n1212 = Equal?(x=w2054, y=2) -> (x = y?=w2057:bool)
                n1213 = local read "DISP LAB05-2"() -> (w2059:T4)
                n1214 = Unbundle(w2059) -> ("STATUS"=w2060:string)  [unwired: 2 out]
                n1215 = Equal?(x=w2060, y="RUN") -> (x = y?=w2056:bool)
                n1216 = And(x=w2056, y=w2057) -> (x .and. y?=w2055:bool)
                n1217 = case shown="True" w2055 {
                  tunnel: w2059 -> [_ w2063]
                  tunnel: w2053 -> [_ w2066]
                  frame False {
                  }
                  frame True {
                    n1218 = local read "SET LAB05-2"() -> (w2065:T5)
                    n1219 = local read "TDMS LAB05-2"() -> (w2062:refnum<k34>)
                    n1220 = Unbundle(w2063) -> ("CYCLE"=w2067:dbl)  [unwired: 2 out]
                    n1221 = Unbundle(w2065) -> ("T-RISE mins"=w2064:dbl)  [unwired: 4 out]
                    n1222 = Greater Or Equal?(x=w2067, y=w2066) -> (x >= y?=w2068:bool)
                    n1223 = case shown="True" w2068 {
                      tunnel: w2064 -> [w2071 _]
                      tunnel: w2063 -> [w2070 _]
                      tunnel: w2062 -> [w2069 _]
                      frame True {
                        n1224 = stacked-sequence {
                          tunnel: w2071 -> [w2074 _]
                          tunnel: w2070 -> [_ w2079]
                          tunnel: w2069 -> [w2072 _]
                          frame #0 {
                            n1225 = Build Array("T-RISE") -> (w2076:string[])
                            n1226 = Build Array(w2074) -> (w2075:dbl[])
                            n1227 = TDMS Write(0:w2072, 5:"TEST PASS", 7:w2076, 9:w2075) -> (15:w2078:errorcluster)  [unwired: 2 in, 3 out]
                            n1228 = local write "data file error"(w2078) -> ()
                          }
                          frame #1 {
                            n1229 = Bundle(cluster=w2079, "STATUS"="T-RISE PASS") -> (w2081:T4)  [unwired: 2 in]
                            n1230 = local write "RESULT LAB05-2"(TRUE) -> ()
                            n1231 = local write "DISP LAB05-2"(w2081) -> ()
                          }
                        }
                      }
                      frame False {
                      }
                    }
                  }
                }
              }
            }
          }
          frame #6 {
            # "end test & close test files"
            n1232 = stacked-sequence {
              tunnel: w2092 -> [_ _ _ _ _ _ _ _ _ _]
              tunnel: w2093 -> [_ _ _ _ _ _ _ _ _ _]
              tunnel: w2091 -> [_ _ _ _ _ _ _ _ _ _]
              tunnel: w2090 -> [_ _ _ _ _ _ _ _ _ _]
              tunnel: w2089 -> [_ _ _ _ _ _ _ _ _ _]
              tunnel: w2088 -> [_ _ _ _ _ _ _ _ _ _]
              tunnel: w2087 -> [_ _ _ _ _ _ _ _ _ _]
              tunnel: w2086 -> [_ _ _ _ _ _ _ _ _ _]
              tunnel: w2085 -> [_ _ _ _ _ _ _ _ _ _]
              tunnel: w2084 -> [_ _ _ _ _ _ _ _ _ _]
              frame #0 {
                # "LAB01-1"
                n1233 = local read "DISP LAB01-1"() -> (w2097:T4)
                n1234 = local read "run lab01-1"() -> (w2094:bool)
                n1235 = local read "TDMS LAB01-1"() -> (w2095:refnum<k34>)
                n1236 = Unbundle(w2097) -> ("CYCLE"=w2098:dbl, "STATUS"=w2096:string)  [unwired: 1 out]
                n1237 = case shown="True" w2094 {
                  tunnel: w2098 -> [_ w2102]
                  tunnel: w2097 -> [_ w2101]
                  tunnel: w2096 -> [_ w2100]
                  tunnel: w2095 -> [_ w2099]
                  frame False {
                  }
                  frame True {
                    n1238 = Not Equal?(x=w2100, y="RUN") -> (x != y?=w2103:bool)
                    n1239 = Greater?(x=w2102, y=2.0) -> (0:w2105:bool)
                    n1240 = And(x=w2105, y=w2103) -> (x .and. y?=w2104:bool)
                    n1241 = case shown="True" w2104 {
                      tunnel: w2101 -> [_ w2109]
                      tunnel: w2099 -> [_ w2108]
                      frame False {
                      }
                      frame True {
                        n1242 = stacked-sequence {
                          tunnel: w2109 -> [w2113 _ _]
                          tunnel: w2108 -> [_ w2115 _]
                          frame #0 {
                            w2110 = FALSE
                            n1243 = local write "mail control"("END") -> ()
                            n1244 = Bundle(cluster=w2113) -> (w2112:T4)  [unwired: 3 in]
                            n1245 = local write "DISP LAB01-1"(w2112) -> ()
                            n1246 = local write "O/I  LAB01-1"(w2110) -> ()
                            n1247 = local write "run lab01-1"(w2110) -> ()
                            n1248 = local write "RUN LAB01-1"(w2110) -> ()
                          }
                          frame #1 {
                            n1249 = TDMS Close(11:w2115) -> (0:w2114:errorcluster)  [unwired: 1 in, 1 out]
                            n1250 = local write "data file error"(w2114) -> ()
                          }
                          frame #2 {
                            n1251 = stacked-sequence {
                              tunnel: "LAB01-1" -> [w2118 w2120]
                              frame #0 {
                                n1252 = call "sub vi - defrag tdms v1.vi"("panel id"=w2118) -> ("error out"=w2117:errorcluster)  [unwired: 10 in]
                                n1253 = local write "data file error"(w2117) -> ()
                              }
                              frame #1 {
                                n1254 = call "Save data file to network drive v1.vi"("panel id"=w2120) -> ("network file save error"=w2119:errorcluster)  [unwired: 9 in, 1 out]
                                n1255 = local write "data file error"(w2119) -> ()
                              }
                            }
                          }
                        }
                      }
                    }
                  }
                }
              }
              frame #1 {
                # "LAB01-2"
                n1256 = local read "run lab01-2"() -> (w2121:bool)
                n1257 = case shown="True" w2121 {
                  frame False {
                  }
                  frame True {
                    n1258 = local read "DISP LAB01-2"() -> (w2128:T4)
                    n1259 = local read "TDMS LAB01-2"() -> (w2127:refnum<k34>)
                    n1260 = Unbundle(w2128) -> ("CYCLE"=w2124:dbl, "STATUS"=w2129:string)  [unwired: 1 out]
                    n1261 = Not Equal?(x=w2129, y="RUN") -> (x != y?=w2123:bool)
                    n1262 = Greater?(x=w2124, y=2.0) -> (0:w2125:bool)
                    n1263 = And(x=w2125, y=w2123) -> (x .and. y?=w2122:bool)
                    n1264 = case shown="True" w2122 {
                      tunnel: w2128 -> [_ w2132]
                      tunnel: w2127 -> [_ w2131]
                      frame False {
                      }
                      frame True {
                        n1265 = stacked-sequence {
                          tunnel: w2132 -> [w2135 _ _]
                          tunnel: w2131 -> [_ w2137 _]
                          frame #0 {
                            w2133 = FALSE
                            n1266 = local write "mail control"("END") -> ()
                            n1267 = Bundle(cluster=w2135) -> (w2136:T4)  [unwired: 3 in]
                            n1268 = local write "RUN LAB01-2"(w2133) -> ()
                            n1269 = local write "run lab01-2"(w2133) -> ()
                            n1270 = local write "O/I  LAB01-2"(w2133) -> ()
                            n1271 = local write "DISP LAB01-2"(w2136) -> ()
                          }
                          frame #1 {
                            n1272 = TDMS Close(11:w2137) -> (0:w2138:errorcluster)  [unwired: 1 in, 1 out]
                            n1273 = local write "data file error"(w2138) -> ()
                          }
                          frame #2 {
                            n1274 = stacked-sequence {
                              tunnel: "LAB01-2" -> [w2141 w2143]
                              frame #0 {
                                n1275 = call "sub vi - defrag tdms v1.vi"("panel id"=w2141) -> ("error out"=w2140:errorcluster)  [unwired: 10 in]
                                n1276 = local write "data file error"(w2140) -> ()
                              }
                              frame #1 {
                                n1277 = call "Save data file to network drive v1.vi"("panel id"=w2143) -> ("network file save error"=w2142:errorcluster)  [unwired: 9 in, 1 out]
                                n1278 = local write "data file error"(w2142) -> ()
                              }
                            }
                          }
                        }
                      }
                    }
                  }
                }
              }
              frame #2 {
                # "LAB02-1"
                n1279 = local read "run lab02-1"() -> (w2144:bool)
                n1280 = case shown="True" w2144 {
                  frame False {
                  }
                  frame True {
                    n1281 = local read "DISP LAB02-1"() -> (w2151:T4)
                    n1282 = Unbundle(w2151) -> ("CYCLE"=w2147:dbl, "STATUS"=w2152:string)  [unwired: 1 out]
                    n1283 = local read "TDMS LAB02-1"() -> (w2150:refnum<k34>)
                    n1284 = Not Equal?(x=w2152, y="RUN") -> (x != y?=w2146:bool)
                    n1285 = Greater?(x=w2147, y=2.0) -> (0:w2148:bool)
                    n1286 = And(x=w2148, y=w2146) -> (x .and. y?=w2145:bool)
                    n1287 = case shown="True" w2145 {
                      tunnel: w2151 -> [_ w2155]
                      tunnel: w2150 -> [_ w2154]
                      frame False {
                      }
                      frame True {
                        n1288 = stacked-sequence {
                          tunnel: w2155 -> [w2158 _ _]
                          tunnel: w2154 -> [_ w2160 _]
                          frame #0 {
                            w2156 = FALSE
                            n1289 = local write "mail control"("END") -> ()
                            n1290 = Bundle(cluster=w2158) -> (w2159:T4)  [unwired: 3 in]
                            n1291 = local write "O/I  LAB02-1"(w2156) -> ()
                            n1292 = local write "RUN LAB02-1"(w2156) -> ()
                            n1293 = local write "run lab02-1"(w2156) -> ()
                            n1294 = local write "DISP LAB02-1"(w2159) -> ()
                          }
                          frame #1 {
                            n1295 = TDMS Close(11:w2160) -> (0:w2161:errorcluster)  [unwired: 1 in, 1 out]
                            n1296 = local write "data file error"(w2161) -> ()
                          }
                          frame #2 {
                            n1297 = stacked-sequence {
                              tunnel: "LAB02-1" -> [w2164 w2166]
                              frame #0 {
                                n1298 = call "sub vi - defrag tdms v1.vi"("panel id"=w2164) -> ("error out"=w2163:errorcluster)  [unwired: 10 in]
                                n1299 = local write "data file error"(w2163) -> ()
                              }
                              frame #1 {
                                n1300 = call "Save data file to network drive v1.vi"("panel id"=w2166) -> ("network file save error"=w2165:errorcluster)  [unwired: 9 in, 1 out]
                                n1301 = local write "data file error"(w2165) -> ()
                              }
                            }
                          }
                        }
                      }
                    }
                  }
                }
              }
              frame #3 {
                # "LAB02-2"
                n1302 = local read "run lab02-2"() -> (w2167:bool)
                n1303 = case shown="True" w2167 {
                  frame False {
                  }
                  frame True {
                    n1304 = local read "DISP LAB02-2"() -> (w2174:T4)
                    n1305 = local read "TDMS LAB02-2"() -> (w2173:refnum<k34>)
                    n1306 = Unbundle(w2174) -> ("CYCLE"=w2170:dbl, "STATUS"=w2175:string)  [unwired: 1 out]
                    n1307 = Not Equal?(x=w2175, y="RUN") -> (x != y?=w2169:bool)
                    n1308 = Greater?(x=w2170, y=2.0) -> (0:w2171:bool)
                    n1309 = And(x=w2171, y=w2169) -> (x .and. y?=w2168:bool)
                    n1310 = case shown="True" w2168 {
                      tunnel: w2174 -> [_ w2178]
                      tunnel: w2173 -> [_ w2177]
                      frame False {
                      }
                      frame True {
                        n1311 = stacked-sequence {
                          tunnel: w2178 -> [w2181 _ _]
                          tunnel: w2177 -> [_ w2183 _]
                          frame #0 {
                            w2179 = FALSE
                            n1312 = local write "mail control"("END") -> ()
                            n1313 = Bundle(cluster=w2181) -> (w2182:T4)  [unwired: 3 in]
                            n1314 = local write "O/I  LAB02-2"(w2179) -> ()
                            n1315 = local write "run lab02-2"(w2179) -> ()
                            n1316 = local write "RUN LAB02-2"(w2179) -> ()
                            n1317 = local write "DISP LAB02-2"(w2182) -> ()
                          }
                          frame #1 {
                            n1318 = TDMS Close(11:w2183) -> (0:w2184:errorcluster)  [unwired: 1 in, 1 out]
                            n1319 = local write "data file error"(w2184) -> ()
                          }
                          frame #2 {
                            n1320 = stacked-sequence {
                              tunnel: "LAB02-2" -> [w2187 w2189]
                              frame #0 {
                                n1321 = call "sub vi - defrag tdms v1.vi"("panel id"=w2187) -> ("error out"=w2186:errorcluster)  [unwired: 10 in]
                                n1322 = local write "data file error"(w2186) -> ()
                              }
                              frame #1 {
                                n1323 = call "Save data file to network drive v1.vi"("panel id"=w2189) -> ("network file save error"=w2188:errorcluster)  [unwired: 9 in, 1 out]
                                n1324 = local write "data file error"(w2188) -> ()
                              }
                            }
                          }
                        }
                      }
                    }
                  }
                }
              }
              frame #4 {
                # "LAB03-1"
                n1325 = local read "run lab03-1"() -> (w2190:bool)
                n1326 = case shown="True" w2190 {
                  frame False {
                  }
                  frame True {
                    n1327 = local read "DISP LAB03-1"() -> (w2197:T4)
                    n1328 = local read "TDMS LAB03-1"() -> (w2196:refnum<k34>)
                    n1329 = Unbundle(w2197) -> ("CYCLE"=w2193:dbl, "STATUS"=w2198:string)  [unwired: 1 out]
                    n1330 = Not Equal?(x=w2198, y="RUN") -> (x != y?=w2192:bool)
                    n1331 = Greater?(x=w2193, y=2.0) -> (0:w2194:bool)
                    n1332 = And(x=w2194, y=w2192) -> (x .and. y?=w2191:bool)
                    n1333 = case shown="True" w2191 {
                      tunnel: w2197 -> [_ w2201]
                      tunnel: w2196 -> [_ w2200]
                      frame False {
                      }
                      frame True {
                        n1334 = stacked-sequence {
                          tunnel: w2201 -> [w2204 _ _]
                          tunnel: w2200 -> [_ w2206 _]
                          frame #0 {
                            w2202 = FALSE
                            n1335 = local write "mail control"("END") -> ()
                            n1336 = Bundle(cluster=w2204) -> (w2205:T4)  [unwired: 3 in]
                            n1337 = local write "O/I  LAB03-1"(w2202) -> ()
                            n1338 = local write "run lab03-1"(w2202) -> ()
                            n1339 = local write "RUN LAB03-1"(w2202) -> ()
                            n1340 = local write "DISP LAB03-1"(w2205) -> ()
                          }
                          frame #1 {
                            n1341 = TDMS Close(11:w2206) -> (0:w2207:errorcluster)  [unwired: 1 in, 1 out]
                            n1342 = local write "data file error"(w2207) -> ()
                          }
                          frame #2 {
                            n1343 = stacked-sequence {
                              tunnel: "LAB03-1" -> [w2210 w2212]
                              frame #0 {
                                n1344 = call "sub vi - defrag tdms v1.vi"("panel id"=w2210) -> ("error out"=w2209:errorcluster)  [unwired: 10 in]
                                n1345 = local write "data file error"(w2209) -> ()
                              }
                              frame #1 {
                                n1346 = call "Save data file to network drive v1.vi"("panel id"=w2212) -> ("network file save error"=w2211:errorcluster)  [unwired: 9 in, 1 out]
                                n1347 = local write "data file error"(w2211) -> ()
                              }
                            }
                          }
                        }
                      }
                    }
                  }
                }
              }
              frame #5 {
                # "LAB03-2"
                n1348 = local read "run lab03-2"() -> (w2213:bool)
                n1349 = case shown="True" w2213 {
                  frame False {
                  }
                  frame True {
                    n1350 = local read "DISP LAB03-2"() -> (w2220:T4)
                    n1351 = Unbundle(w2220) -> ("CYCLE"=w2216:dbl, "STATUS"=w2221:string)  [unwired: 1 out]
                    n1352 = local read "TDMS LAB03-2"() -> (w2219:refnum<k34>)
                    n1353 = Not Equal?(x=w2221, y="RUN") -> (x != y?=w2215:bool)
                    n1354 = Greater?(x=w2216, y=2.0) -> (0:w2217:bool)
                    n1355 = And(x=w2217, y=w2215) -> (x .and. y?=w2214:bool)
                    n1356 = case shown="True" w2214 {
                      tunnel: w2220 -> [_ w2224]
                      tunnel: w2219 -> [_ w2223]
                      frame False {
                      }
                      frame True {
                        n1357 = stacked-sequence {
                          tunnel: w2224 -> [w2227 _ _]
                          tunnel: w2223 -> [_ w2229 _]
                          frame #0 {
                            w2225 = FALSE
                            n1358 = local write "mail control"("END") -> ()
                            n1359 = Bundle(cluster=w2227) -> (w2228:T4)  [unwired: 3 in]
                            n1360 = local write "RUN LAB03-2"(w2225) -> ()
                            n1361 = local write "O/I  LAB03-2"(w2225) -> ()
                            n1362 = local write "DISP LAB03-2"(w2228) -> ()
                            n1363 = local write "run lab03-2"(w2225) -> ()
                          }
                          frame #1 {
                            n1364 = TDMS Close(11:w2229) -> (0:w2230:errorcluster)  [unwired: 1 in, 1 out]
                            n1365 = local write "data file error"(w2230) -> ()
                          }
                          frame #2 {
                            n1366 = stacked-sequence {
                              tunnel: "LAB03-2" -> [w2233 w2235]
                              frame #0 {
                                n1367 = call "sub vi - defrag tdms v1.vi"("panel id"=w2233) -> ("error out"=w2232:errorcluster)  [unwired: 10 in]
                                n1368 = local write "data file error"(w2232) -> ()
                              }
                              frame #1 {
                                n1369 = call "Save data file to network drive v1.vi"("panel id"=w2235) -> ("network file save error"=w2234:errorcluster)  [unwired: 9 in, 1 out]
                                n1370 = local write "data file error"(w2234) -> ()
                              }
                            }
                          }
                        }
                      }
                    }
                  }
                }
              }
              frame #6 {
                # "LAB04-1"
                n1371 = local read "run lab04-1"() -> (w2236:bool)
                n1372 = case shown="True" w2236 {
                  frame False {
                  }
                  frame True {
                    n1373 = local read "DISP LAB04-1"() -> (w2243:T4)
                    n1374 = Unbundle(w2243) -> ("CYCLE"=w2239:dbl, "STATUS"=w2244:string)  [unwired: 1 out]
                    n1375 = local read "TDMS LAB04-1"() -> (w2242:refnum<k34>)
                    n1376 = Not Equal?(x=w2244, y="RUN") -> (x != y?=w2238:bool)
                    n1377 = Greater?(x=w2239, y=2.0) -> (0:w2240:bool)
                    n1378 = And(x=w2240, y=w2238) -> (x .and. y?=w2237:bool)
                    n1379 = case shown="True" w2237 {
                      tunnel: w2243 -> [_ w2247]
                      tunnel: w2242 -> [_ w2246]
                      frame False {
                      }
                      frame True {
                        n1380 = stacked-sequence {
                          tunnel: w2247 -> [w2250 _ _]
                          tunnel: w2246 -> [_ w2252 _]
                          frame #0 {
                            w2248 = FALSE
                            n1381 = local write "mail control"("END") -> ()
                            n1382 = Bundle(cluster=w2250) -> (w2251:T4)  [unwired: 3 in]
                            n1383 = local write "RUN LAB04-1"(w2248) -> ()
                            n1384 = local write "O/I  LAB04-1"(w2248) -> ()
                            n1385 = local write "run lab04-1"(w2248) -> ()
                            n1386 = local write "DISP LAB04-1"(w2251) -> ()
                          }
                          frame #1 {
                            n1387 = TDMS Close(11:w2252) -> (0:w2253:errorcluster)  [unwired: 1 in, 1 out]
                            n1388 = local write "data file error"(w2253) -> ()
                          }
                          frame #2 {
                            n1389 = stacked-sequence {
                              tunnel: "LAB04-1" -> [w2256 w2258]
                              frame #0 {
                                n1390 = call "sub vi - defrag tdms v1.vi"("panel id"=w2256) -> ("error out"=w2255:errorcluster)  [unwired: 10 in]
                                n1391 = local write "data file error"(w2255) -> ()
                              }
                              frame #1 {
                                n1392 = call "Save data file to network drive v1.vi"("panel id"=w2258) -> ("network file save error"=w2257:errorcluster)  [unwired: 9 in, 1 out]
                                n1393 = local write "data file error"(w2257) -> ()
                              }
                            }
                          }
                        }
                      }
                    }
                  }
                }
              }
              frame #7 {
                # "LAB04-2"
                n1394 = local read "run lab04-2"() -> (w2259:bool)
                n1395 = case shown="True" w2259 {
                  frame False {
                  }
                  frame True {
                    n1396 = local read "DISP LAB04-2"() -> (w2266:T4)
                    n1397 = Unbundle(w2266) -> ("CYCLE"=w2262:dbl, "STATUS"=w2267:string)  [unwired: 1 out]
                    n1398 = Not Equal?(x=w2267, y="RUN") -> (x != y?=w2261:bool)
                    n1399 = local read "TDMS LAB04-2"() -> (w2265:refnum<k34>)
                    n1400 = Greater?(x=w2262, y=2.0) -> (0:w2263:bool)
                    n1401 = And(x=w2263, y=w2261) -> (x .and. y?=w2260:bool)
                    n1402 = case shown="True" w2260 {
                      tunnel: w2266 -> [_ w2270]
                      tunnel: w2265 -> [_ w2269]
                      frame False {
                      }
                      frame True {
                        n1403 = stacked-sequence {
                          tunnel: w2270 -> [w2273 _ _]
                          tunnel: w2269 -> [_ w2275 _]
                          frame #0 {
                            w2271 = FALSE
                            n1404 = local write "mail control"("END") -> ()
                            n1405 = Bundle(cluster=w2273) -> (w2274:T4)  [unwired: 3 in]
                            n1406 = local write "O/I  LAB04-2"(w2271) -> ()
                            n1407 = local write "RUN LAB04-2"(w2271) -> ()
                            n1408 = local write "run lab04-2"(w2271) -> ()
                            n1409 = local write "DISP LAB04-2"(w2274) -> ()
                          }
                          frame #1 {
                            n1410 = TDMS Close(11:w2275) -> (0:w2276:errorcluster)  [unwired: 1 in, 1 out]
                            n1411 = local write "data file error"(w2276) -> ()
                          }
                          frame #2 {
                            n1412 = stacked-sequence {
                              tunnel: "LAB04-2" -> [w2279 w2281]
                              frame #0 {
                                n1413 = call "sub vi - defrag tdms v1.vi"("panel id"=w2279) -> ("error out"=w2278:errorcluster)  [unwired: 10 in]
                                n1414 = local write "data file error"(w2278) -> ()
                              }
                              frame #1 {
                                n1415 = call "Save data file to network drive v1.vi"("panel id"=w2281) -> ("network file save error"=w2280:errorcluster)  [unwired: 9 in, 1 out]
                                n1416 = local write "data file error"(w2280) -> ()
                              }
                            }
                          }
                        }
                      }
                    }
                  }
                }
              }
              frame #8 {
                # "LAB05-1"
                n1417 = local read "run lab05-1"() -> (w2282:bool)
                n1418 = case shown="True" w2282 {
                  frame False {
                  }
                  frame True {
                    n1419 = local read "DISP LAB05-1"() -> (w2289:T4)
                    n1420 = Unbundle(w2289) -> ("CYCLE"=w2285:dbl, "STATUS"=w2290:string)  [unwired: 1 out]
                    n1421 = Not Equal?(x=w2290, y="RUN") -> (x != y?=w2284:bool)
                    n1422 = local read "TDMS LAB05-1"() -> (w2288:refnum<k34>)
                    n1423 = Greater?(x=w2285, y=2.0) -> (0:w2286:bool)
                    n1424 = And(x=w2286, y=w2284) -> (x .and. y?=w2283:bool)
                    n1425 = case shown="True" w2283 {
                      tunnel: w2289 -> [_ w2293]
                      tunnel: w2288 -> [_ w2292]
                      frame False {
                      }
                      frame True {
                        n1426 = stacked-sequence {
                          tunnel: w2293 -> [w2296 _ _]
                          tunnel: w2292 -> [_ w2298 _]
                          frame #0 {
                            w2294 = FALSE
                            n1427 = local write "mail control"("END") -> ()
                            n1428 = Bundle(cluster=w2296) -> (w2297:T4)  [unwired: 3 in]
                            n1429 = local write "O/I  LAB05-1"(w2294) -> ()
                            n1430 = local write "RUN LAB05-1"(w2294) -> ()
                            n1431 = local write "run lab05-1"(w2294) -> ()
                            n1432 = local write "DISP LAB05-1"(w2297) -> ()
                          }
                          frame #1 {
                            n1433 = TDMS Close(11:w2298) -> (0:w2299:errorcluster)  [unwired: 1 in, 1 out]
                            n1434 = local write "data file error"(w2299) -> ()
                          }
                          frame #2 {
                            n1435 = stacked-sequence {
                              tunnel: "LAB05-1" -> [w2302 w2304]
                              frame #0 {
                                n1436 = call "sub vi - defrag tdms v1.vi"("panel id"=w2302) -> ("error out"=w2301:errorcluster)  [unwired: 10 in]
                                n1437 = local write "data file error"(w2301) -> ()
                              }
                              frame #1 {
                                n1438 = call "Save data file to network drive v1.vi"("panel id"=w2304) -> ("network file save error"=w2303:errorcluster)  [unwired: 9 in, 1 out]
                                n1439 = local write "data file error"(w2303) -> ()
                              }
                            }
                          }
                        }
                      }
                    }
                  }
                }
              }
              frame #9 {
                # "LAB05-2"
                n1440 = local read "run lab05-2"() -> (w2305:bool)
                n1441 = case shown="True" w2305 {
                  frame False {
                  }
                  frame True {
                    n1442 = local read "DISP LAB05-2"() -> (w2312:T4)
                    n1443 = Unbundle(w2312) -> ("CYCLE"=w2308:dbl, "STATUS"=w2313:string)  [unwired: 1 out]
                    n1444 = Not Equal?(x=w2313, y="RUN") -> (x != y?=w2307:bool)
                    n1445 = local read "TDMS LAB05-2"() -> (w2311:refnum<k34>)
                    n1446 = Greater?(x=w2308, y=2.0) -> (0:w2309:bool)
                    n1447 = And(x=w2309, y=w2307) -> (x .and. y?=w2306:bool)
                    n1448 = case shown="True" w2306 {
                      tunnel: w2312 -> [_ w2316]
                      tunnel: w2311 -> [_ w2315]
                      frame False {
                      }
                      frame True {
                        n1449 = stacked-sequence {
                          tunnel: w2316 -> [w2319 _ _]
                          tunnel: w2315 -> [_ w2321 _]
                          frame #0 {
                            w2317 = FALSE
                            n1450 = local write "mail control"("END") -> ()
                            n1451 = Bundle(cluster=w2319) -> (w2320:T4)  [unwired: 3 in]
                            n1452 = local write "RUN LAB05-2"(w2317) -> ()
                            n1453 = local write "O/I  LAB05-2"(w2317) -> ()
                            n1454 = local write "run lab05-2"(w2317) -> ()
                            n1455 = local write "DISP LAB05-2"(w2320) -> ()
                          }
                          frame #1 {
                            n1456 = TDMS Close(11:w2321) -> (0:w2322:errorcluster)  [unwired: 1 in, 1 out]
                            n1457 = local write "data file error"(w2322) -> ()
                          }
                          frame #2 {
                            n1458 = stacked-sequence {
                              tunnel: "LAB05-2" -> [w2325 w2327]
                              frame #0 {
                                n1459 = call "sub vi - defrag tdms v1.vi"("panel id"=w2325) -> ("error out"=w2324:errorcluster)  [unwired: 10 in]
                                n1460 = local write "data file error"(w2324) -> ()
                              }
                              frame #1 {
                                n1461 = call "Save data file to network drive v1.vi"("panel id"=w2327) -> ("network file save error"=w2326:errorcluster)  [unwired: 9 in, 1 out]
                                n1462 = local write "data file error"(w2326) -> ()
                              }
                            }
                          }
                        }
                      }
                    }
                  }
                }
              }
            }
            n1463 = local read "Network Directory"() -> (w2083:path)
            n1464 = global write "Global 1.vi" "Network Drive"(w2083) -> ()
          }
          frame #7 {
            # "disable functions"
            n1465 = stacked-sequence {
              tunnel: w2337 -> [w2351 _ w2407]
              tunnel: w2336 -> [w2346 _ w2406]
              tunnel: w2335 -> [w2345 _ w2405]
              tunnel: w2334 -> [w2343 _ w2404]
              tunnel: w2333 -> [w2344 _ w2403]
              tunnel: w2332 -> [_ w2368 w2402]
              tunnel: w2331 -> [_ w2369 w2401]
              tunnel: w2330 -> [_ w2370 w2400]
              tunnel: w2329 -> [_ w2371 w2399]
              tunnel: w2328 -> [_ w2372 w2398]
              frame #0 {
                n1466 = Select(t=2, s=w2343, f=0) -> (s? t:f=w2339:i32)
                n1467 = Select(t=2, s=w2345, f=0) -> (s? t:f=w2340:i32)
                n1468 = Select(t=2, s=w2344, f=0) -> (s? t:f=w2338:i32)
                n1469 = Select(t=2, s=w2351, f=0) -> (s? t:f=w2342:i32)
                n1470 = Select(t=2, s=w2346, f=0) -> (s? t:f=w2341:i32)
                n1471 = property on="SELECT LAB02-2" class="RadioBtnsControl (strict)"("DisabledEnum"=w2339) -> ()  [unwired: 2 in, 2 out]
                n1472 = property on="SELECT LAB02-1" class="RadioBtnsControl (strict)"("DisabledEnum"=w2340) -> ()  [unwired: 2 in, 2 out]
                n1473 = property on="SELECT LAB03-1" class="RadioBtnsControl (strict)"("DisabledEnum"=w2338) -> ()  [unwired: 2 in, 2 out]
                n1474 = property on="SELECT LAB01-1" class="RadioBtnsControl (strict)"("DisabledEnum"=w2342) -> ()  [unwired: 2 in, 2 out]
                n1475 = property on="SELECT LAB01-2" class="RadioBtnsControl (strict)"("DisabledEnum"=w2341) -> ()  [unwired: 2 in, 2 out]
                n1476 = Not(x=w2351) -> (.not. x?=w2352:bool)
                n1477 = property on="RESULT LAB01-1" class="Bool (strict)"("Visible"=w2352) -> ()  [unwired: 2 in, 2 out]
                n1478 = Not(x=w2346) -> (.not. x?=w2350:bool)
                n1479 = Not(x=w2345) -> (.not. x?=w2349:bool)
                n1480 = Not(x=w2343) -> (.not. x?=w2348:bool)
                n1481 = property on="RESULT LAB01-2" class="Bool (strict)"("Visible"=w2350) -> ()  [unwired: 2 in, 2 out]
                n1482 = Not(x=w2344) -> (.not. x?=w2347:bool)
                n1483 = property on="RESULT LAB02-1" class="Bool (strict)"("Visible"=w2349) -> ()  [unwired: 2 in, 2 out]
                n1484 = property on="RESULT LAB02-2" class="Bool (strict)"("Visible"=w2348) -> ()  [unwired: 2 in, 2 out]
                n1485 = property on="RESULT LAB03-1" class="Bool (strict)"("Visible"=w2347) -> ()  [unwired: 2 in, 2 out]
                n1486 = property on="SET LAB01-1" class="Clust (strict)"("DisabledEnum"=w2342) -> ()  [unwired: 2 in, 2 out]
                n1487 = property on="SET LAB01-2" class="Clust (strict)"("DisabledEnum"=w2341) -> ()  [unwired: 2 in, 2 out]
                n1488 = property on="SET LAB02-1" class="Clust (strict)"("DisabledEnum"=w2340) -> ()  [unwired: 2 in, 2 out]
                n1489 = property on="SET LAB02-2" class="Clust (strict)"("DisabledEnum"=w2339) -> ()  [unwired: 2 in, 2 out]
                n1490 = property on="SET LAB03-1" class="Clust (strict)"("DisabledEnum"=w2338) -> ()  [unwired: 2 in, 2 out]
                n1491 = property on="O/I  LAB01-1" class="Bool (strict)"("DisabledEnum"=w2342) -> ()  [unwired: 2 in, 2 out]
                n1492 = property on="O/I  LAB01-2" class="Bool (strict)"("DisabledEnum"=w2341) -> ()  [unwired: 2 in, 2 out]
                n1493 = property on="O/I  LAB02-1" class="Bool (strict)"("DisabledEnum"=w2340) -> ()  [unwired: 2 in, 2 out]
                n1494 = property on="O/I  LAB02-2" class="Bool (strict)"("DisabledEnum"=w2339) -> ()  [unwired: 2 in, 2 out]
                n1495 = property on="O/I  LAB03-1" class="Bool (strict)"("DisabledEnum"=w2338) -> ()  [unwired: 2 in, 2 out]
              }
              frame #1 {
                n1496 = Select(t=2, s=w2372, f=0) -> (s? t:f=w2363:i32)
                n1497 = Select(t=2, s=w2371, f=0) -> (s? t:f=w2364:i32)
                n1498 = Select(t=2, s=w2368, f=0) -> (s? t:f=w2367:i32)
                n1499 = Select(t=2, s=w2369, f=0) -> (s? t:f=w2366:i32)
                n1500 = Select(t=2, s=w2370, f=0) -> (s? t:f=w2365:i32)
                n1501 = property on="SELECT LAB05-2" class="RadioBtnsControl (strict)"("DisabledEnum"=w2363) -> ()  [unwired: 2 in, 2 out]
                n1502 = property on="SELECT LAB05-1" class="RadioBtnsControl (strict)"("DisabledEnum"=w2364) -> ()  [unwired: 2 in, 2 out]
                n1503 = property on="SELECT LAB03-2" class="RadioBtnsControl (strict)"("DisabledEnum"=w2367) -> ()  [unwired: 2 in, 2 out]
                n1504 = property on="SELECT LAB04-1" class="RadioBtnsControl (strict)"("DisabledEnum"=w2366) -> ()  [unwired: 2 in, 2 out]
                n1505 = property on="SELECT LAB04-2" class="RadioBtnsControl (strict)"("DisabledEnum"=w2365) -> ()  [unwired: 2 in, 2 out]
                n1506 = property on="SET LAB05-2" class="Clust (strict)"("DisabledEnum"=w2363) -> ()  [unwired: 2 in, 2 out]
                n1507 = property on="SET LAB05-1" class="Clust (strict)"("DisabledEnum"=w2364) -> ()  [unwired: 2 in, 2 out]
                n1508 = property on="SET LAB03-2" class="Clust (strict)"("DisabledEnum"=w2367) -> ()  [unwired: 2 in, 2 out]
                n1509 = property on="SET LAB04-1" class="Clust (strict)"("DisabledEnum"=w2366) -> ()  [unwired: 2 in, 2 out]
                n1510 = property on="SET LAB04-2" class="Clust (strict)"("DisabledEnum"=w2365) -> ()  [unwired: 2 in, 2 out]
                n1511 = property on="O/I  LAB05-2" class="Bool (strict)"("DisabledEnum"=w2363) -> ()  [unwired: 2 in, 2 out]
                n1512 = property on="O/I  LAB05-1" class="Bool (strict)"("DisabledEnum"=w2364) -> ()  [unwired: 2 in, 2 out]
                n1513 = property on="O/I  LAB04-1" class="Bool (strict)"("DisabledEnum"=w2366) -> ()  [unwired: 2 in, 2 out]
                n1514 = property on="O/I  LAB04-2" class="Bool (strict)"("DisabledEnum"=w2365) -> ()  [unwired: 2 in, 2 out]
                n1515 = property on="O/I  LAB03-2" class="Bool (strict)"("DisabledEnum"=w2367) -> ()  [unwired: 2 in, 2 out]
                n1516 = Not(x=w2372) -> (.not. x?=w2373:bool)
                n1517 = Not(x=w2371) -> (.not. x?=w2374:bool)
                n1518 = Not(x=w2370) -> (.not. x?=w2375:bool)
                n1519 = property on="RESULT LAB05-2" class="Bool (strict)"("Visible"=w2373) -> ()  [unwired: 2 in, 2 out]
                n1520 = property on="RESULT LAB05-1" class="Bool (strict)"("Visible"=w2374) -> ()  [unwired: 2 in, 2 out]
                n1521 = Not(x=w2369) -> (.not. x?=w2376:bool)
                n1522 = property on="RESULT LAB04-2" class="Bool (strict)"("Visible"=w2375) -> ()  [unwired: 2 in, 2 out]
                n1523 = Not(x=w2368) -> (.not. x?=w2377:bool)
                n1524 = property on="RESULT LAB04-1" class="Bool (strict)"("Visible"=w2376) -> ()  [unwired: 2 in, 2 out]
                n1525 = property on="RESULT LAB03-2" class="Bool (strict)"("Visible"=w2377) -> ()  [unwired: 2 in, 2 out]
              }
              frame #2 {
                # "disable calibrate if any test running"
                n1526 = Or(x=w2399, y=w2398) -> (x .or. y?=w2392:bool)
                n1527 = Or(x=w2401, y=w2400) -> (x .or. y?=w2394:bool)
                n1528 = Or(x=w2405, y=w2404) -> (x .or. y?=w2396:bool)
                n1529 = Or(x=w2403, y=w2402) -> (x .or. y?=w2395:bool)
                n1530 = Or(x=w2407, y=w2406) -> (x .or. y?=w2397:bool)
                n1531 = Or(x=w2395, y=w2394) -> (x .or. y?=w2393:bool)
                n1532 = Or(x=w2397, y=w2396) -> (x .or. y?=w2391:bool)
                n1533 = Or(x=w2393, y=w2392) -> (x .or. y?=w2390:bool)
                n1534 = Or(x=w2391, y=w2390) -> (x .or. y?=w2389:bool)
                n1535 = case shown="False" w2389 {
                  tunnel: [0 2] -> w2388
                  frame False {
                  }
                  frame True {
                  }
                }
                n1536 = property on="Network Directory" class="Path"("DisabledEnum"=w2388) -> ()  [unwired: 2 in, 2 out]
                n1537 = property on="MAIL SETTINGS" class="Clust (strict)"("DisabledEnum"=w2388) -> ()  [unwired: 2 in, 2 out]
                n1538 = property on="CALIBRATE" class="Bool (strict)"("DisabledEnum"=w2388) -> ()  [unwired: 2 in, 2 out]
                n1539 = property on="SHOW ADMIN PAGE" class="Bool (strict)"("DisabledEnum"=w2388) -> ()  [unwired: 2 in, 2 out]
              }
            }
          }
          frame #8 {
            # "drive jigs"
            n1540 = stacked-sequence {
              frame #0 {
                # "jig on"
                n1541 = local read "jig cycle"() -> (w2410:dbl)
                n1542 = Equal?(x=w2410, y=0) -> (x = y?=w2412:bool)
                n1543 = case shown="True" w2412 {
                  frame False {
                  }
                  frame True {
                    n1544 = local read "RUN LAB01-1"() -> (w2413:bool)
                    n1545 = local read "RUN LAB01-2"() -> (w2414:bool)
                    n1546 = local read "RUN LAB03-1"() -> (w2420:bool)
                    n1547 = local read "RUN LAB03-2"() -> (w2419:bool)
                    n1548 = local read "RUN LAB02-1"() -> (w2422:bool)
                    n1549 = local read "RUN LAB02-2"() -> (w2421:bool)
                    n1550 = local read "RUN LAB04-1"() -> (w2418:bool)
                    n1551 = local read "RUN LAB04-2"() -> (w2417:bool)
                    n1552 = local read "RUN LAB05-1"() -> (w2416:bool)
                    n1553 = local read "RUN LAB05-2"() -> (w2415:bool)
                    n1554 = local write "JIG LAB05-1"(w2416) -> ()
                    n1555 = local write "JIG LAB05-2"(w2415) -> ()
                    n1556 = local write "JIG LAB04-2"(w2417) -> ()
                    n1557 = local write "JIG LAB02-1"(w2422) -> ()
                    n1558 = local write "JIG LAB03-1"(w2420) -> ()
                    n1559 = local write "JIG LAB04-1"(w2418) -> ()
                    n1560 = local write "JIG LAB03-2"(w2419) -> ()
                    n1561 = local write "JIG LAB02-2"(w2421) -> ()
                    n1562 = local write "JIG LAB01-1"(w2413) -> ()
                    n1563 = local write "JIG LAB01-2"(w2414) -> ()
                  }
                }
              }
              frame #1 {
                # "jig off"
                n1564 = local read "jig cycle"() -> (w2425:dbl)
                n1565 = local read "on loops"() -> (w2424:dbl)
                n1566 = Equal?(x=w2425, y=w2424) -> (x = y?=w2423:bool)
                n1567 = case shown="True" w2423 {
                  frame False {
                  }
                  frame True {
                    w2476 = FALSE
                    w2477 = TRUE
                    w2475 = 2
                    n1568 = local read "SELECT LAB05-2"() -> (w2466:T3)
                    n1569 = local read "SELECT LAB04-2"() -> (w2468:T3)
                    n1570 = local read "SELECT LAB04-1"() -> (w2469:T3)
                    n1571 = local read "SELECT LAB05-1"() -> (w2467:T3)
                    n1572 = local read "SELECT LAB03-2"() -> (w2470:T3)
                    n1573 = local read "SELECT LAB02-1"() -> (w2473:T3)
                    n1574 = local read "SELECT LAB03-1"() -> (w2471:T3)
                    n1575 = local read "SELECT LAB02-2"() -> (w2472:T3)
                    n1576 = local read "SELECT LAB01-2"() -> (w2474:T3)
                    n1577 = local read "RUN LAB05-1"() -> (w2436:bool)
                    n1578 = local read "RUN LAB05-2"() -> (w2435:bool)
                    n1579 = local read "RUN LAB04-2"() -> (w2437:bool)
                    n1580 = local read "RUN LAB04-1"() -> (w2438:bool)
                    n1581 = local read "RUN LAB01-1"() -> (w2454:bool)
                    n1582 = local read "RUN LAB01-2"() -> (w2443:bool)
                    n1583 = local read "RUN LAB03-2"() -> (w2439:bool)
                    n1584 = local read "SELECT LAB01-1"() -> (w2478:T3)
                    n1585 = local read "RUN LAB03-1"() -> (w2440:bool)
                    n1586 = local read "RUN LAB02-1"() -> (w2442:bool)
                    n1587 = local read "RUN LAB02-2"() -> (w2441:bool)
                    n1588 = Equal?(x=w2475, y=w2471) -> (x = y?=w2449:bool)
                    n1589 = Equal?(x=w2475, y=w2470) -> (x = y?=w2448:bool)
                    n1590 = Equal?(x=w2475, y=w2469) -> (x = y?=w2447:bool)
                    n1591 = Equal?(x=w2475, y=w2468) -> (x = y?=w2446:bool)
                    n1592 = Equal?(x=w2475, y=w2467) -> (x = y?=w2445:bool)
                    n1593 = Equal?(x=w2475, y=w2466) -> (x = y?=w2444:bool)
                    n1594 = Equal?(x=w2475, y=w2478) -> (x = y?=w2455:bool)
                    n1595 = Equal?(x=w2475, y=w2473) -> (x = y?=w2451:bool)
                    n1596 = Equal?(x=w2475, y=w2472) -> (x = y?=w2450:bool)
                    n1597 = Equal?(x=w2475, y=w2474) -> (x = y?=w2452:bool)
                    n1598 = And(x=w2446, y=w2437) -> (x .and. y?=w2428:bool)
                    n1599 = And(x=w2449, y=w2440) -> (x .and. y?=w2431:bool)
                    n1600 = And(x=w2447, y=w2438) -> (x .and. y?=w2429:bool)
                    n1601 = And(x=w2444, y=w2435) -> (x .and. y?=w2426:bool)
                    n1602 = And(x=w2450, y=w2441) -> (x .and. y?=w2432:bool)
                    n1603 = And(x=w2448, y=w2439) -> (x .and. y?=w2430:bool)
                    n1604 = And(x=w2445, y=w2436) -> (x .and. y?=w2427:bool)
                    n1605 = And(x=w2452, y=w2443) -> (x .and. y?=w2434:bool)
                    n1606 = And(x=w2455, y=w2454) -> (x .and. y?=w2453:bool)
                    n1607 = And(x=w2451, y=w2442) -> (x .and. y?=w2433:bool)
                    n1608 = Select(t=w2477, s=w2453, f=w2476) -> (s? t:f=w2456:bool)
                    n1609 = Select(t=w2477, s=w2434, f=w2476) -> (s? t:f=w2457:bool)
                    n1610 = Select(t=w2477, s=w2433, f=w2476) -> (s? t:f=w2458:bool)
                    n1611 = Select(t=w2477, s=w2432, f=w2476) -> (s? t:f=w2459:bool)
                    n1612 = Select(t=w2477, s=w2431, f=w2476) -> (s? t:f=w2460:bool)
                    n1613 = Select(t=w2477, s=w2430, f=w2476) -> (s? t:f=w2461:bool)
                    n1614 = Select(t=w2477, s=w2429, f=w2476) -> (s? t:f=w2462:bool)
                    n1615 = Select(t=w2477, s=w2428, f=w2476) -> (s? t:f=w2463:bool)
                    n1616 = Select(t=w2477, s=w2427, f=w2476) -> (s? t:f=w2464:bool)
                    n1617 = Select(t=w2477, s=w2426, f=w2476) -> (s? t:f=w2465:bool)
                    n1618 = local write "JIG LAB03-2"(w2461) -> ()
                    n1619 = local write "JIG LAB02-1"(w2458) -> ()
                    n1620 = local write "JIG LAB02-2"(w2459) -> ()
                    n1621 = local write "JIG LAB01-2"(w2457) -> ()
                    n1622 = local write "JIG LAB03-1"(w2460) -> ()
                    n1623 = local write "JIG LAB01-1"(w2456) -> ()
                    n1624 = local write "JIG LAB05-2"(w2465) -> ()
                    n1625 = local write "JIG LAB04-1"(w2462) -> ()
                    n1626 = local write "JIG LAB05-1"(w2464) -> ()
                    n1627 = local write "JIG LAB04-2"(w2463) -> ()
                  }
                }
              }
            }
          }
          frame #9 {
            # "drive digital output"
            n1628 = local read "O/I  LAB05-2"() -> (w2484:bool)
            n1629 = local read "O/I  LAB05-1"() -> (w2486:bool)
            n1630 = local read "JIG LAB05-2"() -> (w2483:bool)
            n1631 = local read "O/I  LAB04-2"() -> (w2488:bool)
            n1632 = local read "JIG LAB05-1"() -> (w2485:bool)
            n1633 = local read "JIG LAB04-2"() -> (w2487:bool)
            n1634 = local read "O/I  LAB03-1"() -> (w2493:bool)
            n1635 = local read "O/I  LAB04-1"() -> (w2489:bool)
            n1636 = local read "O/I  LAB02-1"() -> (w2497:bool)
            n1637 = local read "O/I  LAB02-2"() -> (w2495:bool)
            n1638 = local read "O/I  LAB03-2"() -> (w2491:bool)
            n1639 = local read "JIG LAB04-1"() -> (w2482:bool)
            n1640 = local read "JIG LAB03-2"() -> (w2490:bool)
            n1641 = local read "O/I  LAB01-2"() -> (w2499:bool)
            n1642 = local read "JIG LAB02-1"() -> (w2496:bool)
            n1643 = local read "JIG LAB02-2"() -> (w2494:bool)
            n1644 = local read "JIG LAB03-1"() -> (w2492:bool)
            n1645 = local read "O/I  LAB01-1"() -> (w2501:bool)
            n1646 = local read "JIG LAB01-2"() -> (w2498:bool)
            n1647 = local read "JIG LAB01-1"() -> (w2500:bool)
            n1648 = Build Array(w2488, w2487, w2486, w2485, w2484, w2483) -> (w2479:bool[])
            n1649 = Build Array(w2494, w2493, w2492, w2491, w2490, w2489, w2482) -> (w2480:bool[])
            n1650 = Build Array(w2501, w2500, w2499, w2498, w2497, w2496, w2495) -> (w2481:bool[])
            n1651 = call "sub vi - Drive Relays All v6.vi"("Array #2"=w2479, "Array #1"=w2480, "Array #0"=w2481) -> ()  [unwired: 8 in, 1 out]
          }
          frame #10 {
            # "get temperature values"
            n1652 = stacked-sequence {
              frame #0 {
                n1653 = local read "jig cycle"() -> (w2502:dbl)
                n1654 = local read "on loops"() -> (w2505:dbl)
                n1655 = local read "jig cycle"() -> (w2507:dbl)
                n1656 = Add(x=w2505, y=2) -> (x+y=w2506:dbl)
                n1657 = Equal?(x=w2507, y=0) -> (x = y?=w2508:bool)
                n1658 = Equal?(x=w2502, y=w2506) -> (x = y?=w2503:bool)
                n1659 = case shown="True" w2508 {
                  frame False {
                  }
                  frame True {
                    w2520 = FALSE
                    w2521 = TRUE
                    n1660 = local write "TEMP update"(TRUE) -> ()
                    n1661 = call "sub vi - GET ALL TEMP v3.vi"("LA01-EN"=w2521, "LA02-EN"=w2521, "LA03-EN"=w2521, "LA04-EN"=w2520, "LA05-EN"=w2520, "Gen Cal Value"=1.0) -> ("LA01 TEMP"=w2519:T19, "LA02 TEMP"=w2517:T19, "LA03 TEMP"=w2516:T19)  [unwired: 4 in, 3 out]
                    n1662 = local write "LAB03 TEMP"(w2516) -> ()
                    n1663 = local write "LAB02 TEMP"(w2517) -> ()
                    n1664 = local write "LAB01 TEMP"(w2519) -> ()
                  }
                }
                n1665 = case shown="True" w2503 {
                  frame False {
                  }
                  frame True {
                    w2513 = TRUE
                    w2514 = FALSE
                    n1666 = local write "TEMP update"(TRUE) -> ()
                    n1667 = call "sub vi - GET ALL TEMP v3.vi"("LA01-EN"=w2514, "LA02-EN"=w2514, "LA03-EN"=w2514, "LA04-EN"=w2513, "LA05-EN"=w2513, "Gen Cal Value"=1.0) -> ("LA04 TEMP"=w2511:T19, "LA05 TEMP"=w2510:T19)  [unwired: 4 in, 4 out]
                    n1668 = local write "LAB04 TEMP"(w2511) -> ()
                    n1669 = local write "LAB05 TEMP"(w2510) -> ()
                  }
                }
              }
              frame #1 {
                n1670 = local read "CAL LAB01"() -> (w2539:T7)
                n1671 = local read "LAB01 TEMP"() -> (w2540:T10)
                n1672 = Unbundle By Name(w2540) -> ("T1 Live"=w2530:dbl, "T1 Neut"=w2529:dbl, "T2 Live"=w2528:dbl, "T2 Neut"=w2527:dbl)  [unwired: 2 out]
                n1673 = Unbundle By Name(w2539) -> ("1 (TL) cal"=w2526:dbl, "1 (TN) cal"=w2525:dbl, "2 (TL) cal"=w2524:dbl, "2 (TN) cal"=w2523:dbl)  [unwired: 6 out]
                n1674 = Multiply(x=w2530, y=w2526) -> (x*y=w2536:dbl)
                n1675 = Multiply(x=w2529, y=w2525) -> (x*y=w2535:dbl)
                n1676 = Multiply(x=w2528, y=w2524) -> (x*y=w2532:dbl)
                n1677 = Multiply(x=w2527, y=w2523) -> (x*y=w2531:dbl)
                n1678 = local read "SIG LAB01-2"() -> (w2534:T2)
                n1679 = local read "SIG LAB01-1"() -> (w2538:T2)
                n1680 = Bundle By Name(cluster=w2538, "Tmp Live"=w2536, "Tmp Neut"=w2535) -> (w2537:T2)
                n1681 = Bundle By Name(cluster=w2534, "Tmp Live"=w2532, "Tmp Neut"=w2531) -> (w2533:T2)
                n1682 = local write "SIG LAB01-1"(w2537) -> ()
                n1683 = local write "SIG LAB01-2"(w2533) -> ()
              }
              frame #2 {
                n1684 = local read "CAL LAB02"() -> (w2557:T8)
                n1685 = local read "LAB02 TEMP"() -> (w2558:T10)
                n1686 = Unbundle By Name(w2558) -> ("T1 Live"=w2548:dbl, "T1 Neut"=w2547:dbl, "T2 Live"=w2546:dbl, "T2 Neut"=w2545:dbl)  [unwired: 2 out]
                n1687 = Unbundle By Name(w2557) -> ("1 (TL) cal"=w2544:dbl, "1 (TN) cal"=w2543:dbl, "2 (TL) cal"=w2542:dbl, "2 (TN) cal"=w2541:dbl)  [unwired: 6 out]
                n1688 = Multiply(x=w2548, y=w2544) -> (x*y=w2554:dbl)
                n1689 = Multiply(x=w2547, y=w2543) -> (x*y=w2553:dbl)
                n1690 = Multiply(x=w2546, y=w2542) -> (x*y=w2550:dbl)
                n1691 = Multiply(x=w2545, y=w2541) -> (x*y=w2549:dbl)
                n1692 = local read "SIG LAB02-2"() -> (w2552:T2)
                n1693 = local read "SIG LAB02-1"() -> (w2556:T2)
                n1694 = Bundle By Name(cluster=w2556, "Tmp Live"=w2554, "Tmp Neut"=w2553) -> (w2555:T2)
                n1695 = Bundle By Name(cluster=w2552, "Tmp Live"=w2550, "Tmp Neut"=w2549) -> (w2551:T2)
                n1696 = local write "SIG LAB02-1"(w2555) -> ()
                n1697 = local write "SIG LAB02-2"(w2551) -> ()
              }
              frame #3 {
                n1698 = local read "CAL LAB03"() -> (w2575:T7)
                n1699 = local read "LAB03 TEMP"() -> (w2576:T10)
                n1700 = Unbundle By Name(w2576) -> ("T1 Live"=w2566:dbl, "T1 Neut"=w2565:dbl, "T2 Live"=w2564:dbl, "T2 Neut"=w2563:dbl)  [unwired: 2 out]
                n1701 = Unbundle By Name(w2575) -> ("1 (TL) cal"=w2562:dbl, "1 (TN) cal"=w2561:dbl, "2 (TL) cal"=w2560:dbl, "2 (TN) cal"=w2559:dbl)  [unwired: 6 out]
                n1702 = Multiply(x=w2566, y=w2562) -> (x*y=w2572:dbl)
                n1703 = Multiply(x=w2565, y=w2561) -> (x*y=w2571:dbl)
                n1704 = Multiply(x=w2564, y=w2560) -> (x*y=w2568:dbl)
                n1705 = Multiply(x=w2563, y=w2559) -> (x*y=w2567:dbl)
                n1706 = local read "SIG LAB03-2"() -> (w2570:T2)
                n1707 = local read "SIG LAB03-1"() -> (w2574:T2)
                n1708 = Bundle By Name(cluster=w2574, "Tmp Live"=w2572, "Tmp Neut"=w2571) -> (w2573:T2)
                n1709 = Bundle By Name(cluster=w2570, "Tmp Live"=w2568, "Tmp Neut"=w2567) -> (w2569:T2)
                n1710 = local write "SIG LAB03-1"(w2573) -> ()
                n1711 = local write "SIG LAB03-2"(w2569) -> ()
              }
              frame #4 {
                n1712 = local read "CAL LAB04"() -> (w2593:T7)
                n1713 = local read "LAB04 TEMP"() -> (w2594:T10)
                n1714 = Unbundle By Name(w2594) -> ("T1 Live"=w2584:dbl, "T1 Neut"=w2583:dbl, "T2 Live"=w2582:dbl, "T2 Neut"=w2581:dbl)  [unwired: 2 out]
                n1715 = Unbundle By Name(w2593) -> ("1 (TL) cal"=w2580:dbl, "1 (TN) cal"=w2579:dbl, "2 (TL) cal"=w2578:dbl, "2 (TN) cal"=w2577:dbl)  [unwired: 6 out]
                n1716 = Multiply(x=w2584, y=w2580) -> (x*y=w2590:dbl)
                n1717 = Multiply(x=w2583, y=w2579) -> (x*y=w2589:dbl)
                n1718 = Multiply(x=w2582, y=w2578) -> (x*y=w2586:dbl)
                n1719 = Multiply(x=w2581, y=w2577) -> (x*y=w2585:dbl)
                n1720 = local read "SIG LAB04-2"() -> (w2588:T2)
                n1721 = local read "SIG LAB04-1"() -> (w2592:T2)
                n1722 = Bundle By Name(cluster=w2592, "Tmp Live"=w2590, "Tmp Neut"=w2589) -> (w2591:T2)
                n1723 = Bundle By Name(cluster=w2588, "Tmp Live"=w2586, "Tmp Neut"=w2585) -> (w2587:T2)
                n1724 = local write "SIG LAB04-1"(w2591) -> ()
                n1725 = local write "SIG LAB04-2"(w2587) -> ()
              }
              frame #5 {
                n1726 = local read "CAL LAB05"() -> (w2611:T7)
                n1727 = local read "LAB05 TEMP"() -> (w2612:T10)
                n1728 = Unbundle By Name(w2612) -> ("T1 Live"=w2602:dbl, "T1 Neut"=w2601:dbl, "T2 Live"=w2600:dbl, "T2 Neut"=w2599:dbl)  [unwired: 2 out]
                n1729 = Unbundle By Name(w2611) -> ("1 (TL) cal"=w2598:dbl, "1 (TN) cal"=w2597:dbl, "2 (TL) cal"=w2596:dbl, "2 (TN) cal"=w2595:dbl)  [unwired: 6 out]
                n1730 = Multiply(x=w2602, y=w2598) -> (x*y=w2608:dbl)
                n1731 = Multiply(x=w2601, y=w2597) -> (x*y=w2607:dbl)
                n1732 = Multiply(x=w2600, y=w2596) -> (x*y=w2604:dbl)
                n1733 = Multiply(x=w2599, y=w2595) -> (x*y=w2603:dbl)
                n1734 = local read "SIG LAB05-2"() -> (w2606:T2)
                n1735 = local read "SIG LAB05-1"() -> (w2610:T2)
                n1736 = Bundle By Name(cluster=w2610, "Tmp Live"=w2608, "Tmp Neut"=w2607) -> (w2609:T2)
                n1737 = Bundle By Name(cluster=w2606, "Tmp Live"=w2604, "Tmp Neut"=w2603) -> (w2605:T2)
                n1738 = local write "SIG LAB05-1"(w2609) -> ()
                n1739 = local write "SIG LAB05-2"(w2605) -> ()
              }
            }
          }
          frame #11 {
            # "get analog values"
            n1740 = local read "on loops"() -> (w2619:dbl)
            n1741 = local read "jig cycle"() -> (w2616:dbl)
            n1742 = Add(x=w2619, y=1) -> (x+y=w2617:dbl)
            n1743 = Equal?(x=w2616, y=1) -> (x = y?=w2614:bool)
            n1744 = Equal?(x=w2616, y=w2617) -> (x = y?=w2615:bool)
            n1745 = Or(x=w2614, y=w2615) -> (x .or. y?=w2613:bool)
            n1746 = case shown="True" w2613 {
              frame False {
              }
              frame True {
                n1747 = call "sub vi - Read Analog All v8.vi"() -> ("Analog loop time"=w2627:dbl, "array GRAPH"=w2626:dynamicdata[], "LAB01"=w2625:T20, "LAB02"=w2624:T21, "LAB03"=w2623:T22, "LAB04"=w2622:T23, "array ERROR"=w2628:errorcluster[], "LAB05"=w2621:T24)  [unwired: 8 in]
                n1748 = stacked-sequence {
                  tunnel: w2628 -> [w2631 _ _ _ _ _]
                  tunnel: w2627 -> [w2630 _ _ _ _ _]
                  tunnel: w2626 -> [w2629 _ _ _ _ _]
                  tunnel: w2625 -> [_ w2676 _ _ _ _]
                  tunnel: w2624 -> [_ _ w2677 _ _ _]
                  tunnel: w2623 -> [_ _ _ w2702 _ _]
                  tunnel: w2622 -> [_ _ _ _ w2725 _]
                  tunnel: w2621 -> [_ _ _ _ _ w2750]
                  frame #0 {
                    n1749 = local write "AI update"(TRUE) -> ()
                    n1750 = Index Array(array=w2629, index=6) -> (element=→"LAB04-1 (GRAPH)":dynamicdata)
                    n1751 = Index Array(array=w2629, index=7) -> (element=→"LAB04-2 (GRAPH)":dynamicdata)
                    n1752 = Index Array(array=w2629, index=9) -> (element=→"LAB05-2 (GRAPH)":dynamicdata)
                    n1753 = Index Array(array=w2629, index=8) -> (element=→"LAB05-1 (GRAPH)":dynamicdata)
                    n1754 = Index Array(array=w2629, index=5) -> (element=→"LAB03-2 (GRAPH)":dynamicdata)
                    n1755 = Index Array(array=w2629, index=0) -> (element=→"LAB01-1 (GRAPH)":dynamicdata)
                    n1756 = Index Array(array=w2629, index=1) -> (element=→"LAB01-2 (GRAPH)":dynamicdata)
                    n1757 = Index Array(array=w2629, index=2) -> (element=→"LAB02-1 (GRAPH)":dynamicdata)
                    n1758 = Index Array(array=w2629, index=3) -> (element=→"LAB02-2 (GRAPH)":dynamicdata)
                    n1759 = Index Array(array=w2629, index=4) -> (element=→"LAB03-1 (GRAPH)":dynamicdata)
                    "AI loop time" <- w2630
                    "Analog Error Array" <- w2631
                  }
                  frame #1 {
                    n1760 = local read "CAL LAB01"() -> (w2675:T7)
                    n1761 = Unbundle By Name(w2676) -> ("LAB01-1 (A)"=w2674:dbl, "LAB01-1 (V)"=w2673:dbl, "LAB01-1 (PF)"=w2672:dbl, "LAB01-2 (A)"=w2671:dbl, "LAB01-2 (V)"=w2670:dbl, "LAB01-2 (PF)"=w2669:dbl)
                    n1762 = Unbundle By Name(w2675) -> ("1  (A) cal"=w2668:dbl, "1 (V) cal"=w2667:dbl, "1 (PF) cal"=w2666:dbl, "2 (A) cal"=w2665:dbl, "2 (V) cal"=w2664:dbl, "2 (PF) cal"=w2663:dbl)  [unwired: 4 out]
                    n1763 = Multiply(x=w2674, y=w2668) -> (x*y=w2661:dbl)
                    n1764 = Multiply(x=w2673, y=w2667) -> (x*y=w2660:dbl)
                    n1765 = Multiply(x=w2672, y=w2666) -> (x*y=w2659:dbl)
                    n1766 = Multiply(x=w2671, y=w2665) -> (x*y=w2655:dbl)
                    n1767 = Multiply(x=w2670, y=w2664) -> (x*y=w2654:dbl)
                    n1768 = Multiply(x=w2669, y=w2663) -> (x*y=w2653:dbl)
                    n1769 = local read "SIG LAB01-1"() -> (w2662:T2)
                    n1770 = local read "SIG LAB01-2"() -> (w2657:T2)
                    n1771 = Bundle By Name(cluster=w2662, "AMPS"=w2661, "VOLTS"=w2660, "PF"=w2659) -> (w2658:T2)
                    n1772 = Bundle By Name(cluster=w2657, "AMPS"=w2655, "VOLTS"=w2654, "PF"=w2653) -> (w2656:T2)
                    n1773 = local write "SIG LAB01-2"(w2656) -> ()
                    n1774 = local write "SIG LAB01-1"(w2658) -> ()
                  }
                  frame #2 {
                    n1775 = local read "CAL LAB02"() -> (w2700:T8)
                    n1776 = Unbundle By Name(w2677) -> ("LAB02-1 (A)"=w2699:dbl, "LAB02-1 (V)"=w2698:dbl, "LAB02-1 (PF)"=w2697:dbl, "LAB02-2 (A)"=w2696:dbl, "LAB02-2 (V)"=w2695:dbl, "LAB02-2 (PF)"=w2694:dbl)
                    n1777 = Unbundle By Name(w2700) -> ("1 (A) cal"=w2693:dbl, "1 (V) cal"=w2692:dbl, "1 (PF) cal"=w2691:dbl, "2 (A) cal"=w2690:dbl, "2 (V) cal"=w2689:dbl, "2 (PF) cal"=w2688:dbl)  [unwired: 4 out]
                    n1778 = Multiply(x=w2699, y=w2693) -> (x*y=w2686:dbl)
                    n1779 = Multiply(x=w2698, y=w2692) -> (x*y=w2685:dbl)
                    n1780 = Multiply(x=w2697, y=w2691) -> (x*y=w2684:dbl)
                    n1781 = Multiply(x=w2696, y=w2690) -> (x*y=w2680:dbl)
                    n1782 = Multiply(x=w2695, y=w2689) -> (x*y=w2679:dbl)
                    n1783 = Multiply(x=w2694, y=w2688) -> (x*y=w2678:dbl)
                    n1784 = local read "SIG LAB02-1"() -> (w2687:T2)
                    n1785 = local read "SIG LAB02-2"() -> (w2682:T2)
                    n1786 = Bundle By Name(cluster=w2687, "AMPS"=w2686, "VOLTS"=w2685, "PF"=w2684) -> (w2683:T2)
                    n1787 = Bundle By Name(cluster=w2682, "AMPS"=w2680, "VOLTS"=w2679, "PF"=w2678) -> (w2681:T2)
                    n1788 = local write "SIG LAB02-2"(w2681) -> ()
                    n1789 = local write "SIG LAB02-1"(w2683) -> ()
                  }
                  frame #3 {
                    n1790 = local read "CAL LAB03"() -> (w2724:T7)
                    n1791 = Unbundle By Name(w2702) -> ("LAB03-1 (A)"=w2723:dbl, "LAB03-1 (V)"=w2722:dbl, "LAB03-1 (PF)"=w2721:dbl, "LAB03-2 (A)"=w2720:dbl, "LAB03-2 (V)"=w2719:dbl, "LAB03-2 (PF)"=w2718:dbl)
                    n1792 = Unbundle By Name(w2724) -> ("1  (A) cal"=w2717:dbl, "1 (V) cal"=w2716:dbl, "1 (PF) cal"=w2715:dbl, "2 (A) cal"=w2714:dbl, "2 (V) cal"=w2713:dbl, "2 (PF) cal"=w2712:dbl)  [unwired: 4 out]
                    n1793 = Multiply(x=w2723, y=w2717) -> (x*y=w2710:dbl)
                    n1794 = Multiply(x=w2722, y=w2716) -> (x*y=w2701:dbl)
                    n1795 = Multiply(x=w2721, y=w2715) -> (x*y=w2709:dbl)
                    n1796 = Multiply(x=w2720, y=w2714) -> (x*y=w2705:dbl)
                    n1797 = Multiply(x=w2719, y=w2713) -> (x*y=w2704:dbl)
                    n1798 = Multiply(x=w2718, y=w2712) -> (x*y=w2703:dbl)
                    n1799 = local read "SIG LAB03-1"() -> (w2711:T2)
                    n1800 = local read "SIG LAB03-2"() -> (w2707:T2)
                    n1801 = Bundle By Name(cluster=w2711, "AMPS"=w2710, "VOLTS"=w2701, "PF"=w2709) -> (w2708:T2)
                    n1802 = Bundle By Name(cluster=w2707, "AMPS"=w2705, "VOLTS"=w2704, "PF"=w2703) -> (w2706:T2)
                    n1803 = local write "SIG LAB03-2"(w2706) -> ()
                    n1804 = local write "SIG LAB03-1"(w2708) -> ()
                  }
                  frame #4 {
                    n1805 = local read "CAL LAB04"() -> (w2748:T7)
                    n1806 = Unbundle By Name(w2725) -> ("LAB04-1 (A)"=w2747:dbl, "LAB04-1 (V)"=w2746:dbl, "LAB04-1 (PF)"=w2745:dbl, "LAB04-2 (A)"=w2744:dbl, "LAB04-2 (V)"=w2743:dbl, "LAB04-2 (PF)"=w2742:dbl)
                    n1807 = Unbundle By Name(w2748) -> ("1  (A) cal"=w2741:dbl, "1 (V) cal"=w2740:dbl, "1 (PF) cal"=w2739:dbl, "2 (A) cal"=w2738:dbl, "2 (V) cal"=w2737:dbl, "2 (PF) cal"=w2736:dbl)  [unwired: 4 out]
                    n1808 = Multiply(x=w2747, y=w2741) -> (x*y=w2734:dbl)
                    n1809 = Multiply(x=w2746, y=w2740) -> (x*y=w2733:dbl)
                    n1810 = Multiply(x=w2745, y=w2739) -> (x*y=w2732:dbl)
                    n1811 = Multiply(x=w2744, y=w2738) -> (x*y=w2728:dbl)
                    n1812 = Multiply(x=w2743, y=w2737) -> (x*y=w2727:dbl)
                    n1813 = Multiply(x=w2742, y=w2736) -> (x*y=w2726:dbl)
                    n1814 = local read "SIG LAB04-1"() -> (w2735:T2)
                    n1815 = local read "SIG LAB04-2"() -> (w2730:T2)
                    n1816 = Bundle By Name(cluster=w2735, "AMPS"=w2734, "VOLTS"=w2733, "PF"=w2732) -> (w2731:T2)
                    n1817 = Bundle By Name(cluster=w2730, "AMPS"=w2728, "VOLTS"=w2727, "PF"=w2726) -> (w2729:T2)
                    n1818 = local write "SIG LAB04-2"(w2729) -> ()
                    n1819 = local write "SIG LAB04-1"(w2731) -> ()
                  }
                  frame #5 {
                    n1820 = local read "CAL LAB05"() -> (w2772:T7)
                    n1821 = Unbundle By Name(w2750) -> ("LAB05-1 (A)"=w2771:dbl, "LAB05-1 (V)"=w2749:dbl, "LAB05-1 (PF)"=w2770:dbl, "LAB05-2 (A)"=w2769:dbl, "LAB05-2 (V)"=w2768:dbl, "LAB05-2 (PF)"=w2767:dbl)
                    n1822 = Unbundle By Name(w2772) -> ("1  (A) cal"=w2766:dbl, "1 (V) cal"=w2765:dbl, "1 (PF) cal"=w2764:dbl, "2 (A) cal"=w2763:dbl, "2 (V) cal"=w2762:dbl, "2 (PF) cal"=w2761:dbl)  [unwired: 4 out]
                    n1823 = Multiply(x=w2771, y=w2766) -> (x*y=w2759:dbl)
                    n1824 = Multiply(x=w2749, y=w2765) -> (x*y=w2758:dbl)
                    n1825 = Multiply(x=w2770, y=w2764) -> (x*y=w2757:dbl)
                    n1826 = Multiply(x=w2769, y=w2763) -> (x*y=w2753:dbl)
                    n1827 = Multiply(x=w2768, y=w2762) -> (x*y=w2752:dbl)
                    n1828 = Multiply(x=w2767, y=w2761) -> (x*y=w2751:dbl)
                    n1829 = local read "SIG LAB05-1"() -> (w2760:T2)
                    n1830 = local read "SIG LAB05-2"() -> (w2755:T2)
                    n1831 = Bundle By Name(cluster=w2760, "AMPS"=w2759, "VOLTS"=w2758, "PF"=w2757) -> (w2756:T2)
                    n1832 = Bundle By Name(cluster=w2755, "AMPS"=w2753, "VOLTS"=w2752, "PF"=w2751) -> (w2754:T2)
                    n1833 = local write "SIG LAB05-2"(w2754) -> ()
                    n1834 = local write "SIG LAB05-1"(w2756) -> ()
                  }
                }
              }
            }
          }
          frame #12 {
            # "save test data to file"
            n1835 = Get Date/Time In Seconds() -> (seconds since 1Jan1904=w2777:timestamp)
            n1836 = local read "on loops"() -> (w2792:dbl)
            n1837 = local read "jig cycle"() -> (w2789:dbl)
            n1838 = Format Date/Time String(time format string (%c)="%H:%M%:%S", seconds (now)=w2777) -> (date/time string=w2776:string)  [unwired: 1 in]
            n1839 = Add(x=w2792, y=2) -> (x+y=w2790:dbl)
            n1840 = Build Array(w2776) -> (w2775:string[])
            n1841 = Equal?(x=w2789, y=1) -> (x = y?=w2774:bool)
            n1842 = Equal?(x=w2789, y=w2790) -> (x = y?=w2773:bool)
            n1843 = stacked-sequence {
              tunnel: w2788 -> [w2797 _ _ _ _ _ _ _ _ _]
              tunnel: w2787 -> [_ w2886 _ _ _ _ _ _ _ _]
              tunnel: w2786 -> [_ _ w2978 _ _ _ _ _ _ _]
              tunnel: w2785 -> [_ _ _ w3070 _ _ _ _ _ _]
              tunnel: w2784 -> [_ _ _ _ w3162 _ _ _ _ _]
              tunnel: w2783 -> [_ _ _ _ _ w3254 _ _ _ _]
              tunnel: w2782 -> [_ _ _ _ _ _ w3346 _ _ _]
              tunnel: w2781 -> [_ _ _ _ _ _ _ w3438 _ _]
              tunnel: w2780 -> [_ _ _ _ _ _ _ _ w3530 _]
              tunnel: w2779 -> [_ _ _ _ _ _ _ _ _ w3622]
              tunnel: w2775 -> [w2796 w2889 w2981 w3073 w3165 w3257 w3349 w3441 w3533 w3625]
              tunnel: w2774 -> [w2795 w2888 w2980 w3072 w3164 w3256 w3348 w3440 w3532 w3624]
              tunnel: w2773 -> [w2794 w2887 w2979 w3071 w3163 w3255 w3347 w3439 w3531 w3623]
              frame #0 {
                n1844 = case shown="True" w2797 {
                  tunnel: w2796 -> [_ w2801]
                  tunnel: w2795 -> [_ w2800]
                  tunnel: w2794 -> [_ w2798]
                  frame False {
                  }
                  frame True {
                    n1845 = local read "DISP LAB01-1"() -> (w2802:T4)
                    n1846 = local read "SIG LAB01-1"() -> (w2803:T2)
                    n1847 = local read "ON L01-1"() -> (w2799:cluster{"amps":dbl, "volts":dbl, "pf":dbl})
                    n1848 = Unbundle(w2803) -> ("AMPS"=w2809:dbl, "VOLTS"=w2807:dbl, "PF"=w2806:dbl, "Tmp Live"=w2805:dbl, "Tmp Neut"=w2808:dbl)
                    n1849 = Unbundle(w2802) -> ("CYCLE"=w2804:dbl)  [unwired: 2 out]
                    n1850 = stacked-sequence {
                      tunnel: w2809 -> [w2813 w2831]
                      tunnel: w2808 -> [_ w2830]
                      tunnel: w2807 -> [w2812 w2829]
                      tunnel: w2806 -> [w2811 w2828]
                      tunnel: w2805 -> [_ w2827]
                      tunnel: w2804 -> [_ w2826]
                      tunnel: w2801 -> [_ w2825]
                      tunnel: w2800 -> [w2814 _]
                      tunnel: w2799 -> [w2810 w2823]
                      tunnel: w2798 -> [_ w2824]
                      frame #0 {
                        n1851 = case shown="True" w2814 {
                          tunnel: w2813 -> [_ w2819]
                          tunnel: w2812 -> [_ w2818]
                          tunnel: w2811 -> [_ w2817]
                          tunnel: w2810 -> [_ w2815]
                          frame False {
                          }
                          frame True {
                            n1852 = Bundle(cluster=w2815, "amps"=w2819, "volts"=w2818, "pf"=w2817) -> (w2816:cluster{"amps":dbl, "volts":dbl, "pf":dbl})
                            n1853 = local write "ON L01-1"(w2816) -> ()
                          }
                        }
                      }
                      frame #1 {
                        n1854 = Unbundle(w2823) -> ("amps"=w2822:dbl, "volts"=w2821:dbl, "pf"=w2820:dbl)
                        n1855 = case shown="True" w2824 {
                          tunnel: w2831 -> [_ w2836]
                          tunnel: w2830 -> [_ w2885]
                          tunnel: w2829 -> [_ _]
                          tunnel: w2828 -> [_ _]
                          tunnel: w2827 -> [_ w2884]
                          tunnel: w2826 -> [_ w2883]
                          tunnel: w2825 -> [_ w2879]
                          tunnel: w2822 -> [_ w2838]
                          tunnel: w2821 -> [_ w2837]
                          tunnel: w2820 -> [_ w2835]
                          frame False {
                          }
                          frame True {
                            n1856 = local read "TDMS LAB01-1"() -> (w2876:refnum<k34>)
                            n1857 = Build Array(w2837) -> (w2865:dbl[])
                            n1858 = Build Array(w2835) -> (w2860:dbl[])
                            n1859 = Build Array(w2884) -> (w2855:dbl[])
                            n1860 = Build Array(w2885) -> (w2850:dbl[])
                            n1861 = Build Array(w2838) -> (w2872:dbl[])
                            n1862 = Build Array(w2836) -> (w2834:dbl[])
                            n1863 = Build Array(w2883) -> (w2845:dbl[])
                            n1864 = Build Array("TEMP Neut") -> (w2851:string[])
                            n1865 = Build Array("CYCLE") -> (w2846:string[])
                            n1866 = Build Array("TEMP Live") -> (w2856:string[])
                            n1867 = Build Array("PF") -> (w2861:string[])
                            n1868 = Build Array("AMPS OFF") -> (w2839:string[])
                            n1869 = Build Array("AMPS ON") -> (w2873:string[])
                            n1870 = Build Array("VOLTS") -> (w2867:string[])
                            n1871 = TDMS Write(0:w2876, 5:"LAB01-1 TEST VALUES", 7:w2873, 9:w2872) -> (4:w2844:refnum<k34>, 6:w2843:string, 15:w2833:errorcluster)  [unwired: 2 in, 1 out]
                            n1872 = TDMS Write(0:w2844, 5:w2843, 7:w2839, 9:w2834, 11:w2833) -> (4:w2842:refnum<k34>, 6:w2841:string, 15:w2832:errorcluster)  [unwired: 1 in, 1 out]
                            n1873 = TDMS Write(0:w2842, 5:w2841, 7:w2867, 9:w2865, 11:w2832) -> (4:w2864:refnum<k34>, 6:w2863:string, 15:w2862:errorcluster)  [unwired: 1 in, 1 out]
                            n1874 = TDMS Write(0:w2864, 5:w2863, 7:w2861, 9:w2860, 11:w2862) -> (4:w2859:refnum<k34>, 6:w2858:string, 15:w2857:errorcluster)  [unwired: 1 in, 1 out]
                            n1875 = TDMS Write(0:w2859, 5:w2858, 7:w2856, 9:w2855, 11:w2857) -> (4:w2854:refnum<k34>, 6:w2853:string, 15:w2852:errorcluster)  [unwired: 1 in, 1 out]
                            n1876 = TDMS Write(0:w2854, 5:w2853, 7:w2851, 9:w2850, 11:w2852) -> (4:w2849:refnum<k34>, 6:w2848:string, 15:w2847:errorcluster)  [unwired: 1 in, 1 out]
                            n1877 = TDMS Write(0:w2849, 5:w2848, 7:w2846, 9:w2845, 11:w2847) -> (4:w2877:refnum<k34>, 6:w2881:string, 15:w2882:errorcluster)  [unwired: 1 in, 1 out]
                            n1878 = TDMS Write(0:w2877, 5:w2881, 7:"TIME", 9:w2879, 11:w2882) -> (15:w2878:errorcluster)  [unwired: 1 in, 3 out]
                            n1879 = local write "data file error"(w2878) -> ()
                          }
                        }
                      }
                    }
                  }
                }
              }
              frame #1 {
                n1880 = case shown="True" w2886 {
                  tunnel: w2889 -> [_ w2893]
                  tunnel: w2888 -> [_ w2892]
                  tunnel: w2887 -> [_ w2890]
                  frame False {
                  }
                  frame True {
                    n1881 = local read "DISP LAB01-2"() -> (w2894:T4)
                    n1882 = local read "SIG LAB01-2"() -> (w2895:T2)
                    n1883 = local read "ON L01-2"() -> (w2891:cluster{"amps":dbl, "volts":dbl, "pf":dbl})
                    n1884 = Unbundle(w2895) -> ("AMPS"=w2901:dbl, "VOLTS"=w2899:dbl, "PF"=w2898:dbl, "Tmp Live"=w2897:dbl, "Tmp Neut"=w2900:dbl)
                    n1885 = Unbundle(w2894) -> ("CYCLE"=w2896:dbl)  [unwired: 2 out]
                    n1886 = stacked-sequence {
                      tunnel: w2901 -> [w2905 w2923]
                      tunnel: w2900 -> [_ w2922]
                      tunnel: w2899 -> [w2904 w2921]
                      tunnel: w2898 -> [w2903 w2920]
                      tunnel: w2897 -> [_ w2919]
                      tunnel: w2896 -> [_ w2918]
                      tunnel: w2893 -> [_ w2917]
                      tunnel: w2892 -> [w2906 _]
                      tunnel: w2891 -> [w2902 w2915]
                      tunnel: w2890 -> [_ w2916]
                      frame #0 {
                        n1887 = case shown="True" w2906 {
                          tunnel: w2905 -> [_ w2911]
                          tunnel: w2904 -> [_ w2910]
                          tunnel: w2903 -> [_ w2909]
                          tunnel: w2902 -> [_ w2907]
                          frame False {
                          }
                          frame True {
                            n1888 = Bundle(cluster=w2907, "amps"=w2911, "volts"=w2910, "pf"=w2909) -> (w2908:cluster{"amps":dbl, "volts":dbl, "pf":dbl})
                            n1889 = local write "ON L01-2"(w2908) -> ()
                          }
                        }
                      }
                      frame #1 {
                        n1890 = Unbundle(w2915) -> ("amps"=w2914:dbl, "volts"=w2913:dbl, "pf"=w2912:dbl)
                        n1891 = case shown="True" w2916 {
                          tunnel: w2923 -> [_ w2928]
                          tunnel: w2922 -> [_ w2977]
                          tunnel: w2921 -> [_ _]
                          tunnel: w2920 -> [_ _]
                          tunnel: w2919 -> [_ w2976]
                          tunnel: w2918 -> [_ w2975]
                          tunnel: w2917 -> [_ w2971]
                          tunnel: w2914 -> [_ w2930]
                          tunnel: w2913 -> [_ w2929]
                          tunnel: w2912 -> [_ w2927]
                          frame False {
                          }
                          frame True {
                            n1892 = local read "TDMS LAB01-2"() -> (w2968:refnum<k34>)
                            n1893 = Build Array(w2929) -> (w2957:dbl[])
                            n1894 = Build Array(w2927) -> (w2952:dbl[])
                            n1895 = Build Array(w2976) -> (w2947:dbl[])
                            n1896 = Build Array(w2977) -> (w2942:dbl[])
                            n1897 = Build Array(w2930) -> (w2964:dbl[])
                            n1898 = Build Array(w2928) -> (w2926:dbl[])
                            n1899 = Build Array(w2975) -> (w2937:dbl[])
                            n1900 = Build Array("TEMP Neut") -> (w2943:string[])
                            n1901 = Build Array("CYCLE") -> (w2938:string[])
                            n1902 = Build Array("TEMP Live") -> (w2948:string[])
                            n1903 = Build Array("PF") -> (w2953:string[])
                            n1904 = Build Array("AMPS OFF") -> (w2931:string[])
                            n1905 = Build Array("AMPS ON") -> (w2965:string[])
                            n1906 = Build Array("VOLTS") -> (w2959:string[])
                            n1907 = TDMS Write(0:w2968, 5:"LAB01-2 TEST VALUES", 7:w2965, 9:w2964) -> (4:w2936:refnum<k34>, 6:w2935:string, 15:w2925:errorcluster)  [unwired: 2 in, 1 out]
                            n1908 = TDMS Write(0:w2936, 5:w2935, 7:w2931, 9:w2926, 11:w2925) -> (4:w2934:refnum<k34>, 6:w2933:string, 15:w2924:errorcluster)  [unwired: 1 in, 1 out]
                            n1909 = TDMS Write(0:w2934, 5:w2933, 7:w2959, 9:w2957, 11:w2924) -> (4:w2956:refnum<k34>, 6:w2955:string, 15:w2954:errorcluster)  [unwired: 1 in, 1 out]
                            n1910 = TDMS Write(0:w2956, 5:w2955, 7:w2953, 9:w2952, 11:w2954) -> (4:w2951:refnum<k34>, 6:w2950:string, 15:w2949:errorcluster)  [unwired: 1 in, 1 out]
                            n1911 = TDMS Write(0:w2951, 5:w2950, 7:w2948, 9:w2947, 11:w2949) -> (4:w2946:refnum<k34>, 6:w2945:string, 15:w2944:errorcluster)  [unwired: 1 in, 1 out]
                            n1912 = TDMS Write(0:w2946, 5:w2945, 7:w2943, 9:w2942, 11:w2944) -> (4:w2941:refnum<k34>, 6:w2940:string, 15:w2939:errorcluster)  [unwired: 1 in, 1 out]
                            n1913 = TDMS Write(0:w2941, 5:w2940, 7:w2938, 9:w2937, 11:w2939) -> (4:w2969:refnum<k34>, 6:w2973:string, 15:w2974:errorcluster)  [unwired: 1 in, 1 out]
                            n1914 = TDMS Write(0:w2969, 5:w2973, 7:"TIME", 9:w2971, 11:w2974) -> (15:w2970:errorcluster)  [unwired: 1 in, 3 out]
                            n1915 = local write "data file error"(w2970) -> ()
                          }
                        }
                      }
                    }
                  }
                }
              }
              frame #2 {
                n1916 = case shown="True" w2978 {
                  tunnel: w2981 -> [_ w2985]
                  tunnel: w2980 -> [_ w2984]
                  tunnel: w2979 -> [_ w2982]
                  frame False {
                  }
                  frame True {
                    n1917 = local read "DISP LAB02-1"() -> (w2986:T4)
                    n1918 = local read "SIG LAB02-1"() -> (w2987:T2)
                    n1919 = local read "ON L02-1"() -> (w2983:cluster{"amps":dbl, "volts":dbl, "pf":dbl})
                    n1920 = Unbundle(w2987) -> ("AMPS"=w2993:dbl, "VOLTS"=w2991:dbl, "PF"=w2990:dbl, "Tmp Live"=w2989:dbl, "Tmp Neut"=w2992:dbl)
                    n1921 = Unbundle(w2986) -> ("CYCLE"=w2988:dbl)  [unwired: 2 out]
                    n1922 = stacked-sequence {
                      tunnel: w2993 -> [w2997 w3015]
                      tunnel: w2992 -> [_ w3014]
                      tunnel: w2991 -> [w2996 w3013]
                      tunnel: w2990 -> [w2995 w3012]
                      tunnel: w2989 -> [_ w3011]
                      tunnel: w2988 -> [_ w3010]
                      tunnel: w2985 -> [_ w3009]
                      tunnel: w2984 -> [w2998 _]
                      tunnel: w2983 -> [w2994 w3007]
                      tunnel: w2982 -> [_ w3008]
                      frame #0 {
                        n1923 = case shown="True" w2998 {
                          tunnel: w2997 -> [_ w3003]
                          tunnel: w2996 -> [_ w3002]
                          tunnel: w2995 -> [_ w3001]
                          tunnel: w2994 -> [_ w2999]
                          frame False {
                          }
                          frame True {
                            n1924 = Bundle(cluster=w2999, "amps"=w3003, "volts"=w3002, "pf"=w3001) -> (w3000:cluster{"amps":dbl, "volts":dbl, "pf":dbl})
                            n1925 = local write "ON L02-1"(w3000) -> ()
                          }
                        }
                      }
                      frame #1 {
                        n1926 = Unbundle(w3007) -> ("amps"=w3006:dbl, "volts"=w3005:dbl, "pf"=w3004:dbl)
                        n1927 = case shown="True" w3008 {
                          tunnel: w3015 -> [_ w3020]
                          tunnel: w3014 -> [_ w3069]
                          tunnel: w3013 -> [_ _]
                          tunnel: w3012 -> [_ _]
                          tunnel: w3011 -> [_ w3068]
                          tunnel: w3010 -> [_ w3067]
                          tunnel: w3009 -> [_ w3063]
                          tunnel: w3006 -> [_ w3022]
                          tunnel: w3005 -> [_ w3021]
                          tunnel: w3004 -> [_ w3019]
                          frame False {
                          }
                          frame True {
                            n1928 = local read "TDMS LAB02-1"() -> (w3060:refnum<k34>)
                            n1929 = Build Array(w3021) -> (w3049:dbl[])
                            n1930 = Build Array(w3019) -> (w3044:dbl[])
                            n1931 = Build Array(w3068) -> (w3039:dbl[])
                            n1932 = Build Array(w3069) -> (w3034:dbl[])
                            n1933 = Build Array(w3022) -> (w3056:dbl[])
                            n1934 = Build Array(w3020) -> (w3018:dbl[])
                            n1935 = Build Array(w3067) -> (w3029:dbl[])
                            n1936 = Build Array("TEMP Neut") -> (w3035:string[])
                            n1937 = Build Array("CYCLE") -> (w3030:string[])
                            n1938 = Build Array("TEMP Live") -> (w3040:string[])
                            n1939 = Build Array("PF") -> (w3045:string[])
                            n1940 = Build Array("AMPS OFF") -> (w3023:string[])
                            n1941 = Build Array("AMPS ON") -> (w3057:string[])
                            n1942 = Build Array("VOLTS") -> (w3051:string[])
                            n1943 = TDMS Write(0:w3060, 5:"LAB02-1 TEST VALUES", 7:w3057, 9:w3056) -> (4:w3028:refnum<k34>, 6:w3027:string, 15:w3017:errorcluster)  [unwired: 2 in, 1 out]
                            n1944 = TDMS Write(0:w3028, 5:w3027, 7:w3023, 9:w3018, 11:w3017) -> (4:w3026:refnum<k34>, 6:w3025:string, 15:w3016:errorcluster)  [unwired: 1 in, 1 out]
                            n1945 = TDMS Write(0:w3026, 5:w3025, 7:w3051, 9:w3049, 11:w3016) -> (4:w3048:refnum<k34>, 6:w3047:string, 15:w3046:errorcluster)  [unwired: 1 in, 1 out]
                            n1946 = TDMS Write(0:w3048, 5:w3047, 7:w3045, 9:w3044, 11:w3046) -> (4:w3043:refnum<k34>, 6:w3042:string, 15:w3041:errorcluster)  [unwired: 1 in, 1 out]
                            n1947 = TDMS Write(0:w3043, 5:w3042, 7:w3040, 9:w3039, 11:w3041) -> (4:w3038:refnum<k34>, 6:w3037:string, 15:w3036:errorcluster)  [unwired: 1 in, 1 out]
                            n1948 = TDMS Write(0:w3038, 5:w3037, 7:w3035, 9:w3034, 11:w3036) -> (4:w3033:refnum<k34>, 6:w3032:string, 15:w3031:errorcluster)  [unwired: 1 in, 1 out]
                            n1949 = TDMS Write(0:w3033, 5:w3032, 7:w3030, 9:w3029, 11:w3031) -> (4:w3061:refnum<k34>, 6:w3065:string, 15:w3066:errorcluster)  [unwired: 1 in, 1 out]
                            n1950 = TDMS Write(0:w3061, 5:w3065, 7:"TIME", 9:w3063, 11:w3066) -> (15:w3062:errorcluster)  [unwired: 1 in, 3 out]
                            n1951 = local write "data file error"(w3062) -> ()
                          }
                        }
                      }
                    }
                  }
                }
              }
              frame #3 {
                n1952 = case shown="True" w3070 {
                  tunnel: w3073 -> [_ w3077]
                  tunnel: w3072 -> [_ w3076]
                  tunnel: w3071 -> [_ w3074]
                  frame False {
                  }
                  frame True {
                    n1953 = local read "DISP LAB02-2"() -> (w3078:T4)
                    n1954 = local read "SIG LAB02-2"() -> (w3079:T2)
                    n1955 = local read "ON L02-2"() -> (w3075:cluster{"amps":dbl, "volts":dbl, "pf":dbl})
                    n1956 = Unbundle(w3079) -> ("AMPS"=w3085:dbl, "VOLTS"=w3083:dbl, "PF"=w3082:dbl, "Tmp Live"=w3081:dbl, "Tmp Neut"=w3084:dbl)
                    n1957 = Unbundle(w3078) -> ("CYCLE"=w3080:dbl)  [unwired: 2 out]
                    n1958 = stacked-sequence {
                      tunnel: w3085 -> [w3089 w3107]
                      tunnel: w3084 -> [_ w3106]
                      tunnel: w3083 -> [w3088 w3105]
                      tunnel: w3082 -> [w3087 w3104]
                      tunnel: w3081 -> [_ w3103]
                      tunnel: w3080 -> [_ w3102]
                      tunnel: w3077 -> [_ w3101]
                      tunnel: w3076 -> [w3090 _]
                      tunnel: w3075 -> [w3086 w3099]
                      tunnel: w3074 -> [_ w3100]
                      frame #0 {
                        n1959 = case shown="True" w3090 {
                          tunnel: w3089 -> [_ w3095]
                          tunnel: w3088 -> [_ w3094]
                          tunnel: w3087 -> [_ w3093]
                          tunnel: w3086 -> [_ w3091]
                          frame False {
                          }
                          frame True {
                            n1960 = Bundle(cluster=w3091, "amps"=w3095, "volts"=w3094, "pf"=w3093) -> (w3092:cluster{"amps":dbl, "volts":dbl, "pf":dbl})
                            n1961 = local write "ON L02-2"(w3092) -> ()
                          }
                        }
                      }
                      frame #1 {
                        n1962 = Unbundle(w3099) -> ("amps"=w3098:dbl, "volts"=w3097:dbl, "pf"=w3096:dbl)
                        n1963 = case shown="True" w3100 {
                          tunnel: w3107 -> [_ w3112]
                          tunnel: w3106 -> [_ w3161]
                          tunnel: w3105 -> [_ _]
                          tunnel: w3104 -> [_ _]
                          tunnel: w3103 -> [_ w3160]
                          tunnel: w3102 -> [_ w3159]
                          tunnel: w3101 -> [_ w3155]
                          tunnel: w3098 -> [_ w3114]
                          tunnel: w3097 -> [_ w3113]
                          tunnel: w3096 -> [_ w3111]
                          frame False {
                          }
                          frame True {
                            n1964 = local read "TDMS LAB02-2"() -> (w3152:refnum<k34>)
                            n1965 = Build Array(w3113) -> (w3141:dbl[])
                            n1966 = Build Array(w3111) -> (w3136:dbl[])
                            n1967 = Build Array(w3160) -> (w3131:dbl[])
                            n1968 = Build Array(w3161) -> (w3126:dbl[])
                            n1969 = Build Array(w3114) -> (w3148:dbl[])
                            n1970 = Build Array(w3112) -> (w3110:dbl[])
                            n1971 = Build Array(w3159) -> (w3121:dbl[])
                            n1972 = Build Array("TEMP Neut") -> (w3127:string[])
                            n1973 = Build Array("CYCLE") -> (w3122:string[])
                            n1974 = Build Array("TEMP Live") -> (w3132:string[])
                            n1975 = Build Array("PF") -> (w3137:string[])
                            n1976 = Build Array("AMPS OFF") -> (w3115:string[])
                            n1977 = Build Array("AMPS ON") -> (w3149:string[])
                            n1978 = Build Array("VOLTS") -> (w3143:string[])
                            n1979 = TDMS Write(0:w3152, 5:"LAB02-2 TEST VALUES", 7:w3149, 9:w3148) -> (4:w3120:refnum<k34>, 6:w3119:string, 15:w3109:errorcluster)  [unwired: 2 in, 1 out]
                            n1980 = TDMS Write(0:w3120, 5:w3119, 7:w3115, 9:w3110, 11:w3109) -> (4:w3118:refnum<k34>, 6:w3117:string, 15:w3108:errorcluster)  [unwired: 1 in, 1 out]
                            n1981 = TDMS Write(0:w3118, 5:w3117, 7:w3143, 9:w3141, 11:w3108) -> (4:w3140:refnum<k34>, 6:w3139:string, 15:w3138:errorcluster)  [unwired: 1 in, 1 out]
                            n1982 = TDMS Write(0:w3140, 5:w3139, 7:w3137, 9:w3136, 11:w3138) -> (4:w3135:refnum<k34>, 6:w3134:string, 15:w3133:errorcluster)  [unwired: 1 in, 1 out]
                            n1983 = TDMS Write(0:w3135, 5:w3134, 7:w3132, 9:w3131, 11:w3133) -> (4:w3130:refnum<k34>, 6:w3129:string, 15:w3128:errorcluster)  [unwired: 1 in, 1 out]
                            n1984 = TDMS Write(0:w3130, 5:w3129, 7:w3127, 9:w3126, 11:w3128) -> (4:w3125:refnum<k34>, 6:w3124:string, 15:w3123:errorcluster)  [unwired: 1 in, 1 out]
                            n1985 = TDMS Write(0:w3125, 5:w3124, 7:w3122, 9:w3121, 11:w3123) -> (4:w3153:refnum<k34>, 6:w3157:string, 15:w3158:errorcluster)  [unwired: 1 in, 1 out]
                            n1986 = TDMS Write(0:w3153, 5:w3157, 7:"TIME", 9:w3155, 11:w3158) -> (15:w3154:errorcluster)  [unwired: 1 in, 3 out]
                            n1987 = local write "data file error"(w3154) -> ()
                          }
                        }
                      }
                    }
                  }
                }
              }
              frame #4 {
                n1988 = case shown="True" w3162 {
                  tunnel: w3165 -> [_ w3169]
                  tunnel: w3164 -> [_ w3168]
                  tunnel: w3163 -> [_ w3166]
                  frame False {
                  }
                  frame True {
                    n1989 = local read "DISP LAB03-1"() -> (w3170:T4)
                    n1990 = local read "SIG LAB03-1"() -> (w3171:T2)
                    n1991 = local read "ON L03-1"() -> (w3167:cluster{"amps":dbl, "volts":dbl, "pf":dbl})
                    n1992 = Unbundle(w3171) -> ("AMPS"=w3177:dbl, "VOLTS"=w3175:dbl, "PF"=w3174:dbl, "Tmp Live"=w3173:dbl, "Tmp Neut"=w3176:dbl)
                    n1993 = Unbundle(w3170) -> ("CYCLE"=w3172:dbl)  [unwired: 2 out]
                    n1994 = stacked-sequence {
                      tunnel: w3177 -> [w3181 w3199]
                      tunnel: w3176 -> [_ w3198]
                      tunnel: w3175 -> [w3180 w3197]
                      tunnel: w3174 -> [w3179 w3196]
                      tunnel: w3173 -> [_ w3195]
                      tunnel: w3172 -> [_ w3194]
                      tunnel: w3169 -> [_ w3193]
                      tunnel: w3168 -> [w3182 _]
                      tunnel: w3167 -> [w3178 w3191]
                      tunnel: w3166 -> [_ w3192]
                      frame #0 {
                        n1995 = case shown="True" w3182 {
                          tunnel: w3181 -> [_ w3187]
                          tunnel: w3180 -> [_ w3186]
                          tunnel: w3179 -> [_ w3185]
                          tunnel: w3178 -> [_ w3183]
                          frame False {
                          }
                          frame True {
                            n1996 = Bundle(cluster=w3183, "amps"=w3187, "volts"=w3186, "pf"=w3185) -> (w3184:cluster{"amps":dbl, "volts":dbl, "pf":dbl})
                            n1997 = local write "ON L03-1"(w3184) -> ()
                          }
                        }
                      }
                      frame #1 {
                        n1998 = Unbundle(w3191) -> ("amps"=w3190:dbl, "volts"=w3189:dbl, "pf"=w3188:dbl)
                        n1999 = case shown="True" w3192 {
                          tunnel: w3199 -> [_ w3204]
                          tunnel: w3198 -> [_ w3253]
                          tunnel: w3197 -> [_ _]
                          tunnel: w3196 -> [_ _]
                          tunnel: w3195 -> [_ w3252]
                          tunnel: w3194 -> [_ w3251]
                          tunnel: w3193 -> [_ w3247]
                          tunnel: w3190 -> [_ w3206]
                          tunnel: w3189 -> [_ w3205]
                          tunnel: w3188 -> [_ w3203]
                          frame False {
                          }
                          frame True {
                            n2000 = local read "TDMS LAB03-1"() -> (w3244:refnum<k34>)
                            n2001 = Build Array(w3205) -> (w3233:dbl[])
                            n2002 = Build Array(w3203) -> (w3228:dbl[])
                            n2003 = Build Array(w3252) -> (w3223:dbl[])
                            n2004 = Build Array(w3253) -> (w3218:dbl[])
                            n2005 = Build Array(w3206) -> (w3240:dbl[])
                            n2006 = Build Array(w3204) -> (w3202:dbl[])
                            n2007 = Build Array(w3251) -> (w3213:dbl[])
                            n2008 = Build Array("TEMP Neut") -> (w3219:string[])
                            n2009 = Build Array("CYCLE") -> (w3214:string[])
                            n2010 = Build Array("TEMP Live") -> (w3224:string[])
                            n2011 = Build Array("PF") -> (w3229:string[])
                            n2012 = Build Array("AMPS OFF") -> (w3207:string[])
                            n2013 = Build Array("AMPS ON") -> (w3241:string[])
                            n2014 = Build Array("VOLTS") -> (w3235:string[])
                            n2015 = TDMS Write(0:w3244, 5:"LAB03-1 TEST VALUES", 7:w3241, 9:w3240) -> (4:w3212:refnum<k34>, 6:w3211:string, 15:w3201:errorcluster)  [unwired: 2 in, 1 out]
                            n2016 = TDMS Write(0:w3212, 5:w3211, 7:w3207, 9:w3202, 11:w3201) -> (4:w3210:refnum<k34>, 6:w3209:string, 15:w3200:errorcluster)  [unwired: 1 in, 1 out]
                            n2017 = TDMS Write(0:w3210, 5:w3209, 7:w3235, 9:w3233, 11:w3200) -> (4:w3232:refnum<k34>, 6:w3231:string, 15:w3230:errorcluster)  [unwired: 1 in, 1 out]
                            n2018 = TDMS Write(0:w3232, 5:w3231, 7:w3229, 9:w3228, 11:w3230) -> (4:w3227:refnum<k34>, 6:w3226:string, 15:w3225:errorcluster)  [unwired: 1 in, 1 out]
                            n2019 = TDMS Write(0:w3227, 5:w3226, 7:w3224, 9:w3223, 11:w3225) -> (4:w3222:refnum<k34>, 6:w3221:string, 15:w3220:errorcluster)  [unwired: 1 in, 1 out]
                            n2020 = TDMS Write(0:w3222, 5:w3221, 7:w3219, 9:w3218, 11:w3220) -> (4:w3217:refnum<k34>, 6:w3216:string, 15:w3215:errorcluster)  [unwired: 1 in, 1 out]
                            n2021 = TDMS Write(0:w3217, 5:w3216, 7:w3214, 9:w3213, 11:w3215) -> (4:w3245:refnum<k34>, 6:w3249:string, 15:w3250:errorcluster)  [unwired: 1 in, 1 out]
                            n2022 = TDMS Write(0:w3245, 5:w3249, 7:"TIME", 9:w3247, 11:w3250) -> (15:w3246:errorcluster)  [unwired: 1 in, 3 out]
                            n2023 = local write "data file error"(w3246) -> ()
                          }
                        }
                      }
                    }
                  }
                }
              }
              frame #5 {
                n2024 = case shown="True" w3254 {
                  tunnel: w3257 -> [_ w3261]
                  tunnel: w3256 -> [_ w3260]
                  tunnel: w3255 -> [_ w3258]
                  frame False {
                  }
                  frame True {
                    n2025 = local read "DISP LAB03-2"() -> (w3262:T4)
                    n2026 = local read "SIG LAB03-2"() -> (w3263:T2)
                    n2027 = local read "ON L03-2"() -> (w3259:cluster{"amps":dbl, "volts":dbl, "pf":dbl})
                    n2028 = Unbundle(w3263) -> ("AMPS"=w3269:dbl, "VOLTS"=w3267:dbl, "PF"=w3266:dbl, "Tmp Live"=w3265:dbl, "Tmp Neut"=w3268:dbl)
                    n2029 = Unbundle(w3262) -> ("CYCLE"=w3264:dbl)  [unwired: 2 out]
                    n2030 = stacked-sequence {
                      tunnel: w3269 -> [w3273 w3291]
                      tunnel: w3268 -> [_ w3290]
                      tunnel: w3267 -> [w3272 w3289]
                      tunnel: w3266 -> [w3271 w3288]
                      tunnel: w3265 -> [_ w3287]
                      tunnel: w3264 -> [_ w3286]
                      tunnel: w3261 -> [_ w3285]
                      tunnel: w3260 -> [w3274 _]
                      tunnel: w3259 -> [w3270 w3283]
                      tunnel: w3258 -> [_ w3284]
                      frame #0 {
                        n2031 = case shown="True" w3274 {
                          tunnel: w3273 -> [_ w3279]
                          tunnel: w3272 -> [_ w3278]
                          tunnel: w3271 -> [_ w3277]
                          tunnel: w3270 -> [_ w3275]
                          frame False {
                          }
                          frame True {
                            n2032 = Bundle(cluster=w3275, "amps"=w3279, "volts"=w3278, "pf"=w3277) -> (w3276:cluster{"amps":dbl, "volts":dbl, "pf":dbl})
                            n2033 = local write "ON L03-2"(w3276) -> ()
                          }
                        }
                      }
                      frame #1 {
                        n2034 = Unbundle(w3283) -> ("amps"=w3282:dbl, "volts"=w3281:dbl, "pf"=w3280:dbl)
                        n2035 = case shown="True" w3284 {
                          tunnel: w3291 -> [_ w3296]
                          tunnel: w3290 -> [_ w3345]
                          tunnel: w3289 -> [_ _]
                          tunnel: w3288 -> [_ _]
                          tunnel: w3287 -> [_ w3344]
                          tunnel: w3286 -> [_ w3343]
                          tunnel: w3285 -> [_ w3339]
                          tunnel: w3282 -> [_ w3298]
                          tunnel: w3281 -> [_ w3297]
                          tunnel: w3280 -> [_ w3295]
                          frame False {
                          }
                          frame True {
                            n2036 = local read "TDMS LAB03-2"() -> (w3336:refnum<k34>)
                            n2037 = Build Array(w3297) -> (w3325:dbl[])
                            n2038 = Build Array(w3295) -> (w3320:dbl[])
                            n2039 = Build Array(w3344) -> (w3315:dbl[])
                            n2040 = Build Array(w3345) -> (w3310:dbl[])
                            n2041 = Build Array(w3298) -> (w3332:dbl[])
                            n2042 = Build Array(w3296) -> (w3294:dbl[])
                            n2043 = Build Array(w3343) -> (w3305:dbl[])
                            n2044 = Build Array("TEMP Neut") -> (w3311:string[])
                            n2045 = Build Array("CYCLE") -> (w3306:string[])
                            n2046 = Build Array("TEMP Live") -> (w3316:string[])
                            n2047 = Build Array("PF") -> (w3321:string[])
                            n2048 = Build Array("AMPS OFF") -> (w3299:string[])
                            n2049 = Build Array("AMPS ON") -> (w3333:string[])
                            n2050 = Build Array("VOLTS") -> (w3327:string[])
                            n2051 = TDMS Write(0:w3336, 5:"LAB03-2 TEST VALUES", 7:w3333, 9:w3332) -> (4:w3304:refnum<k34>, 6:w3303:string, 15:w3293:errorcluster)  [unwired: 2 in, 1 out]
                            n2052 = TDMS Write(0:w3304, 5:w3303, 7:w3299, 9:w3294, 11:w3293) -> (4:w3302:refnum<k34>, 6:w3301:string, 15:w3292:errorcluster)  [unwired: 1 in, 1 out]
                            n2053 = TDMS Write(0:w3302, 5:w3301, 7:w3327, 9:w3325, 11:w3292) -> (4:w3324:refnum<k34>, 6:w3323:string, 15:w3322:errorcluster)  [unwired: 1 in, 1 out]
                            n2054 = TDMS Write(0:w3324, 5:w3323, 7:w3321, 9:w3320, 11:w3322) -> (4:w3319:refnum<k34>, 6:w3318:string, 15:w3317:errorcluster)  [unwired: 1 in, 1 out]
                            n2055 = TDMS Write(0:w3319, 5:w3318, 7:w3316, 9:w3315, 11:w3317) -> (4:w3314:refnum<k34>, 6:w3313:string, 15:w3312:errorcluster)  [unwired: 1 in, 1 out]
                            n2056 = TDMS Write(0:w3314, 5:w3313, 7:w3311, 9:w3310, 11:w3312) -> (4:w3309:refnum<k34>, 6:w3308:string, 15:w3307:errorcluster)  [unwired: 1 in, 1 out]
                            n2057 = TDMS Write(0:w3309, 5:w3308, 7:w3306, 9:w3305, 11:w3307) -> (4:w3337:refnum<k34>, 6:w3341:string, 15:w3342:errorcluster)  [unwired: 1 in, 1 out]
                            n2058 = TDMS Write(0:w3337, 5:w3341, 7:"TIME", 9:w3339, 11:w3342) -> (15:w3338:errorcluster)  [unwired: 1 in, 3 out]
                            n2059 = local write "data file error"(w3338) -> ()
                          }
                        }
                      }
                    }
                  }
                }
              }
              frame #6 {
                n2060 = case shown="True" w3346 {
                  tunnel: w3349 -> [_ w3353]
                  tunnel: w3348 -> [_ w3352]
                  tunnel: w3347 -> [_ w3350]
                  frame False {
                  }
                  frame True {
                    n2061 = local read "DISP LAB04-1"() -> (w3354:T4)
                    n2062 = local read "SIG LAB04-1"() -> (w3355:T2)
                    n2063 = local read "ON L04-1"() -> (w3351:cluster{"amps":dbl, "volts":dbl, "pf":dbl})
                    n2064 = Unbundle(w3355) -> ("AMPS"=w3361:dbl, "VOLTS"=w3359:dbl, "PF"=w3358:dbl, "Tmp Live"=w3357:dbl, "Tmp Neut"=w3360:dbl)
                    n2065 = Unbundle(w3354) -> ("CYCLE"=w3356:dbl)  [unwired: 2 out]
                    n2066 = stacked-sequence {
                      tunnel: w3361 -> [w3365 w3383]
                      tunnel: w3360 -> [_ w3382]
                      tunnel: w3359 -> [w3364 w3381]
                      tunnel: w3358 -> [w3363 w3380]
                      tunnel: w3357 -> [_ w3379]
                      tunnel: w3356 -> [_ w3378]
                      tunnel: w3353 -> [_ w3377]
                      tunnel: w3352 -> [w3366 _]
                      tunnel: w3351 -> [w3362 w3375]
                      tunnel: w3350 -> [_ w3376]
                      frame #0 {
                        n2067 = case shown="True" w3366 {
                          tunnel: w3365 -> [_ w3371]
                          tunnel: w3364 -> [_ w3370]
                          tunnel: w3363 -> [_ w3369]
                          tunnel: w3362 -> [_ w3367]
                          frame False {
                          }
                          frame True {
                            n2068 = Bundle(cluster=w3367, "amps"=w3371, "volts"=w3370, "pf"=w3369) -> (w3368:cluster{"amps":dbl, "volts":dbl, "pf":dbl})
                            n2069 = local write "ON L04-1"(w3368) -> ()
                          }
                        }
                      }
                      frame #1 {
                        n2070 = Unbundle(w3375) -> ("amps"=w3374:dbl, "volts"=w3373:dbl, "pf"=w3372:dbl)
                        n2071 = case shown="True" w3376 {
                          tunnel: w3383 -> [_ w3388]
                          tunnel: w3382 -> [_ w3437]
                          tunnel: w3381 -> [_ _]
                          tunnel: w3380 -> [_ _]
                          tunnel: w3379 -> [_ w3436]
                          tunnel: w3378 -> [_ w3435]
                          tunnel: w3377 -> [_ w3431]
                          tunnel: w3374 -> [_ w3390]
                          tunnel: w3373 -> [_ w3389]
                          tunnel: w3372 -> [_ w3387]
                          frame False {
                          }
                          frame True {
                            n2072 = local read "TDMS LAB04-1"() -> (w3428:refnum<k34>)
                            n2073 = Build Array(w3389) -> (w3417:dbl[])
                            n2074 = Build Array(w3387) -> (w3412:dbl[])
                            n2075 = Build Array(w3436) -> (w3407:dbl[])
                            n2076 = Build Array(w3437) -> (w3402:dbl[])
                            n2077 = Build Array(w3390) -> (w3424:dbl[])
                            n2078 = Build Array(w3388) -> (w3386:dbl[])
                            n2079 = Build Array(w3435) -> (w3397:dbl[])
                            n2080 = Build Array("TEMP Neut") -> (w3403:string[])
                            n2081 = Build Array("CYCLE") -> (w3398:string[])
                            n2082 = Build Array("TEMP Live") -> (w3408:string[])
                            n2083 = Build Array("PF") -> (w3413:string[])
                            n2084 = Build Array("AMPS OFF") -> (w3391:string[])
                            n2085 = Build Array("AMPS ON") -> (w3425:string[])
                            n2086 = Build Array("VOLTS") -> (w3419:string[])
                            n2087 = TDMS Write(0:w3428, 5:"LAB04-1 TEST VALUES", 7:w3425, 9:w3424) -> (4:w3396:refnum<k34>, 6:w3395:string, 15:w3385:errorcluster)  [unwired: 2 in, 1 out]
                            n2088 = TDMS Write(0:w3396, 5:w3395, 7:w3391, 9:w3386, 11:w3385) -> (4:w3394:refnum<k34>, 6:w3393:string, 15:w3384:errorcluster)  [unwired: 1 in, 1 out]
                            n2089 = TDMS Write(0:w3394, 5:w3393, 7:w3419, 9:w3417, 11:w3384) -> (4:w3416:refnum<k34>, 6:w3415:string, 15:w3414:errorcluster)  [unwired: 1 in, 1 out]
                            n2090 = TDMS Write(0:w3416, 5:w3415, 7:w3413, 9:w3412, 11:w3414) -> (4:w3411:refnum<k34>, 6:w3410:string, 15:w3409:errorcluster)  [unwired: 1 in, 1 out]
                            n2091 = TDMS Write(0:w3411, 5:w3410, 7:w3408, 9:w3407, 11:w3409) -> (4:w3406:refnum<k34>, 6:w3405:string, 15:w3404:errorcluster)  [unwired: 1 in, 1 out]
                            n2092 = TDMS Write(0:w3406, 5:w3405, 7:w3403, 9:w3402, 11:w3404) -> (4:w3401:refnum<k34>, 6:w3400:string, 15:w3399:errorcluster)  [unwired: 1 in, 1 out]
                            n2093 = TDMS Write(0:w3401, 5:w3400, 7:w3398, 9:w3397, 11:w3399) -> (4:w3429:refnum<k34>, 6:w3433:string, 15:w3434:errorcluster)  [unwired: 1 in, 1 out]
                            n2094 = TDMS Write(0:w3429, 5:w3433, 7:"TIME", 9:w3431, 11:w3434) -> (15:w3430:errorcluster)  [unwired: 1 in, 3 out]
                            n2095 = local write "data file error"(w3430) -> ()
                          }
                        }
                      }
                    }
                  }
                }
              }
              frame #7 {
                n2096 = case shown="True" w3438 {
                  tunnel: w3441 -> [_ w3445]
                  tunnel: w3440 -> [_ w3444]
                  tunnel: w3439 -> [_ w3442]
                  frame False {
                  }
                  frame True {
                    n2097 = local read "DISP LAB04-2"() -> (w3446:T4)
                    n2098 = local read "SIG LAB04-2"() -> (w3447:T2)
                    n2099 = local read "ON L04-2"() -> (w3443:cluster{"amps":dbl, "volts":dbl, "pf":dbl})
                    n2100 = Unbundle(w3447) -> ("AMPS"=w3453:dbl, "VOLTS"=w3451:dbl, "PF"=w3450:dbl, "Tmp Live"=w3449:dbl, "Tmp Neut"=w3452:dbl)
                    n2101 = Unbundle(w3446) -> ("CYCLE"=w3448:dbl)  [unwired: 2 out]
                    n2102 = stacked-sequence {
                      tunnel: w3453 -> [w3457 w3475]
                      tunnel: w3452 -> [_ w3474]
                      tunnel: w3451 -> [w3456 w3473]
                      tunnel: w3450 -> [w3455 w3472]
                      tunnel: w3449 -> [_ w3471]
                      tunnel: w3448 -> [_ w3470]
                      tunnel: w3445 -> [_ w3469]
                      tunnel: w3444 -> [w3458 _]
                      tunnel: w3443 -> [w3454 w3467]
                      tunnel: w3442 -> [_ w3468]
                      frame #0 {
                        n2103 = case shown="True" w3458 {
                          tunnel: w3457 -> [_ w3463]
                          tunnel: w3456 -> [_ w3462]
                          tunnel: w3455 -> [_ w3461]
                          tunnel: w3454 -> [_ w3459]
                          frame False {
                          }
                          frame True {
                            n2104 = Bundle(cluster=w3459, "amps"=w3463, "volts"=w3462, "pf"=w3461) -> (w3460:cluster{"amps":dbl, "volts":dbl, "pf":dbl})
                            n2105 = local write "ON L04-2"(w3460) -> ()
                          }
                        }
                      }
                      frame #1 {
                        n2106 = Unbundle(w3467) -> ("amps"=w3466:dbl, "volts"=w3465:dbl, "pf"=w3464:dbl)
                        n2107 = case shown="True" w3468 {
                          tunnel: w3475 -> [_ w3480]
                          tunnel: w3474 -> [_ w3529]
                          tunnel: w3473 -> [_ _]
                          tunnel: w3472 -> [_ _]
                          tunnel: w3471 -> [_ w3528]
                          tunnel: w3470 -> [_ w3527]
                          tunnel: w3469 -> [_ w3523]
                          tunnel: w3466 -> [_ w3482]
                          tunnel: w3465 -> [_ w3481]
                          tunnel: w3464 -> [_ w3479]
                          frame False {
                          }
                          frame True {
                            n2108 = local read "TDMS LAB04-2"() -> (w3520:refnum<k34>)
                            n2109 = Build Array(w3481) -> (w3509:dbl[])
                            n2110 = Build Array(w3479) -> (w3504:dbl[])
                            n2111 = Build Array(w3528) -> (w3499:dbl[])
                            n2112 = Build Array(w3529) -> (w3494:dbl[])
                            n2113 = Build Array(w3482) -> (w3516:dbl[])
                            n2114 = Build Array(w3480) -> (w3478:dbl[])
                            n2115 = Build Array(w3527) -> (w3489:dbl[])
                            n2116 = Build Array("TEMP Neut") -> (w3495:string[])
                            n2117 = Build Array("CYCLE") -> (w3490:string[])
                            n2118 = Build Array("TEMP Live") -> (w3500:string[])
                            n2119 = Build Array("PF") -> (w3505:string[])
                            n2120 = Build Array("AMPS OFF") -> (w3483:string[])
                            n2121 = Build Array("AMPS ON") -> (w3517:string[])
                            n2122 = Build Array("VOLTS") -> (w3511:string[])
                            n2123 = TDMS Write(0:w3520, 5:"LAB04-2 TEST VALUES", 7:w3517, 9:w3516) -> (4:w3488:refnum<k34>, 6:w3487:string, 15:w3477:errorcluster)  [unwired: 2 in, 1 out]
                            n2124 = TDMS Write(0:w3488, 5:w3487, 7:w3483, 9:w3478, 11:w3477) -> (4:w3486:refnum<k34>, 6:w3485:string, 15:w3476:errorcluster)  [unwired: 1 in, 1 out]
                            n2125 = TDMS Write(0:w3486, 5:w3485, 7:w3511, 9:w3509, 11:w3476) -> (4:w3508:refnum<k34>, 6:w3507:string, 15:w3506:errorcluster)  [unwired: 1 in, 1 out]
                            n2126 = TDMS Write(0:w3508, 5:w3507, 7:w3505, 9:w3504, 11:w3506) -> (4:w3503:refnum<k34>, 6:w3502:string, 15:w3501:errorcluster)  [unwired: 1 in, 1 out]
                            n2127 = TDMS Write(0:w3503, 5:w3502, 7:w3500, 9:w3499, 11:w3501) -> (4:w3498:refnum<k34>, 6:w3497:string, 15:w3496:errorcluster)  [unwired: 1 in, 1 out]
                            n2128 = TDMS Write(0:w3498, 5:w3497, 7:w3495, 9:w3494, 11:w3496) -> (4:w3493:refnum<k34>, 6:w3492:string, 15:w3491:errorcluster)  [unwired: 1 in, 1 out]
                            n2129 = TDMS Write(0:w3493, 5:w3492, 7:w3490, 9:w3489, 11:w3491) -> (4:w3521:refnum<k34>, 6:w3525:string, 15:w3526:errorcluster)  [unwired: 1 in, 1 out]
                            n2130 = TDMS Write(0:w3521, 5:w3525, 7:"TIME", 9:w3523, 11:w3526) -> (15:w3522:errorcluster)  [unwired: 1 in, 3 out]
                            n2131 = local write "data file error"(w3522) -> ()
                          }
                        }
                      }
                    }
                  }
                }
              }
              frame #8 {
                n2132 = case shown="True" w3530 {
                  tunnel: w3533 -> [_ w3537]
                  tunnel: w3532 -> [_ w3536]
                  tunnel: w3531 -> [_ w3534]
                  frame False {
                  }
                  frame True {
                    n2133 = local read "DISP LAB05-1"() -> (w3538:T4)
                    n2134 = local read "SIG LAB05-1"() -> (w3539:T2)
                    n2135 = local read "ON L05-1"() -> (w3535:cluster{"amps":dbl, "volts":dbl, "pf":dbl})
                    n2136 = Unbundle(w3539) -> ("AMPS"=w3545:dbl, "VOLTS"=w3543:dbl, "PF"=w3542:dbl, "Tmp Live"=w3541:dbl, "Tmp Neut"=w3544:dbl)
                    n2137 = Unbundle(w3538) -> ("CYCLE"=w3540:dbl)  [unwired: 2 out]
                    n2138 = stacked-sequence {
                      tunnel: w3545 -> [w3549 w3567]
                      tunnel: w3544 -> [_ w3566]
                      tunnel: w3543 -> [w3548 w3565]
                      tunnel: w3542 -> [w3547 w3564]
                      tunnel: w3541 -> [_ w3563]
                      tunnel: w3540 -> [_ w3562]
                      tunnel: w3537 -> [_ w3561]
                      tunnel: w3536 -> [w3550 _]
                      tunnel: w3535 -> [w3546 w3559]
                      tunnel: w3534 -> [_ w3560]
                      frame #0 {
                        n2139 = case shown="True" w3550 {
                          tunnel: w3549 -> [_ w3555]
                          tunnel: w3548 -> [_ w3554]
                          tunnel: w3547 -> [_ w3553]
                          tunnel: w3546 -> [_ w3551]
                          frame False {
                          }
                          frame True {
                            n2140 = Bundle(cluster=w3551, "amps"=w3555, "volts"=w3554, "pf"=w3553) -> (w3552:cluster{"amps":dbl, "volts":dbl, "pf":dbl})
                            n2141 = local write "ON L05-1"(w3552) -> ()
                          }
                        }
                      }
                      frame #1 {
                        n2142 = Unbundle(w3559) -> ("amps"=w3558:dbl, "volts"=w3557:dbl, "pf"=w3556:dbl)
                        n2143 = case shown="True" w3560 {
                          tunnel: w3567 -> [_ w3572]
                          tunnel: w3566 -> [_ w3621]
                          tunnel: w3565 -> [_ _]
                          tunnel: w3564 -> [_ _]
                          tunnel: w3563 -> [_ w3620]
                          tunnel: w3562 -> [_ w3619]
                          tunnel: w3561 -> [_ w3615]
                          tunnel: w3558 -> [_ w3574]
                          tunnel: w3557 -> [_ w3573]
                          tunnel: w3556 -> [_ w3571]
                          frame False {
                          }
                          frame True {
                            n2144 = local read "TDMS LAB05-1"() -> (w3612:refnum<k34>)
                            n2145 = Build Array(w3573) -> (w3601:dbl[])
                            n2146 = Build Array(w3571) -> (w3596:dbl[])
                            n2147 = Build Array(w3620) -> (w3591:dbl[])
                            n2148 = Build Array(w3621) -> (w3586:dbl[])
                            n2149 = Build Array(w3574) -> (w3608:dbl[])
                            n2150 = Build Array(w3572) -> (w3570:dbl[])
                            n2151 = Build Array(w3619) -> (w3581:dbl[])
                            n2152 = Build Array("TEMP Neut") -> (w3587:string[])
                            n2153 = Build Array("CYCLE") -> (w3582:string[])
                            n2154 = Build Array("TEMP Live") -> (w3592:string[])
                            n2155 = Build Array("PF") -> (w3597:string[])
                            n2156 = Build Array("AMPS OFF") -> (w3575:string[])
                            n2157 = Build Array("AMPS ON") -> (w3609:string[])
                            n2158 = Build Array("VOLTS") -> (w3603:string[])
                            n2159 = TDMS Write(0:w3612, 5:"LAB05-1 TEST VALUES", 7:w3609, 9:w3608) -> (4:w3580:refnum<k34>, 6:w3579:string, 15:w3569:errorcluster)  [unwired: 2 in, 1 out]
                            n2160 = TDMS Write(0:w3580, 5:w3579, 7:w3575, 9:w3570, 11:w3569) -> (4:w3578:refnum<k34>, 6:w3577:string, 15:w3568:errorcluster)  [unwired: 1 in, 1 out]
                            n2161 = TDMS Write(0:w3578, 5:w3577, 7:w3603, 9:w3601, 11:w3568) -> (4:w3600:refnum<k34>, 6:w3599:string, 15:w3598:errorcluster)  [unwired: 1 in, 1 out]
                            n2162 = TDMS Write(0:w3600, 5:w3599, 7:w3597, 9:w3596, 11:w3598) -> (4:w3595:refnum<k34>, 6:w3594:string, 15:w3593:errorcluster)  [unwired: 1 in, 1 out]
                            n2163 = TDMS Write(0:w3595, 5:w3594, 7:w3592, 9:w3591, 11:w3593) -> (4:w3590:refnum<k34>, 6:w3589:string, 15:w3588:errorcluster)  [unwired: 1 in, 1 out]
                            n2164 = TDMS Write(0:w3590, 5:w3589, 7:w3587, 9:w3586, 11:w3588) -> (4:w3585:refnum<k34>, 6:w3584:string, 15:w3583:errorcluster)  [unwired: 1 in, 1 out]
                            n2165 = TDMS Write(0:w3585, 5:w3584, 7:w3582, 9:w3581, 11:w3583) -> (4:w3613:refnum<k34>, 6:w3617:string, 15:w3618:errorcluster)  [unwired: 1 in, 1 out]
                            n2166 = TDMS Write(0:w3613, 5:w3617, 7:"TIME", 9:w3615, 11:w3618) -> (15:w3614:errorcluster)  [unwired: 1 in, 3 out]
                            n2167 = local write "data file error"(w3614) -> ()
                          }
                        }
                      }
                    }
                  }
                }
              }
              frame #9 {
                n2168 = case shown="True" w3622 {
                  tunnel: w3625 -> [_ w3629]
                  tunnel: w3624 -> [_ w3628]
                  tunnel: w3623 -> [_ w3626]
                  frame False {
                  }
                  frame True {
                    n2169 = local read "DISP LAB05-2"() -> (w3630:T4)
                    n2170 = local read "SIG LAB05-2"() -> (w3631:T2)
                    n2171 = local read "ON L05-2"() -> (w3627:cluster{"amps":dbl, "volts":dbl, "pf":dbl})
                    n2172 = Unbundle(w3631) -> ("AMPS"=w3637:dbl, "VOLTS"=w3635:dbl, "PF"=w3634:dbl, "Tmp Live"=w3633:dbl, "Tmp Neut"=w3636:dbl)
                    n2173 = Unbundle(w3630) -> ("CYCLE"=w3632:dbl)  [unwired: 2 out]
                    n2174 = stacked-sequence {
                      tunnel: w3637 -> [w3641 w3659]
                      tunnel: w3636 -> [_ w3658]
                      tunnel: w3635 -> [w3640 w3657]
                      tunnel: w3634 -> [w3639 w3656]
                      tunnel: w3633 -> [_ w3655]
                      tunnel: w3632 -> [_ w3654]
                      tunnel: w3629 -> [_ w3653]
                      tunnel: w3628 -> [w3642 _]
                      tunnel: w3627 -> [w3638 w3651]
                      tunnel: w3626 -> [_ w3652]
                      frame #0 {
                        n2175 = case shown="True" w3642 {
                          tunnel: w3641 -> [_ w3647]
                          tunnel: w3640 -> [_ w3646]
                          tunnel: w3639 -> [_ w3645]
                          tunnel: w3638 -> [_ w3643]
                          frame False {
                          }
                          frame True {
                            n2176 = Bundle(cluster=w3643, "amps"=w3647, "volts"=w3646, "pf"=w3645) -> (w3644:cluster{"amps":dbl, "volts":dbl, "pf":dbl})
                            n2177 = local write "ON L05-2"(w3644) -> ()
                          }
                        }
                      }
                      frame #1 {
                        n2178 = Unbundle(w3651) -> ("amps"=w3650:dbl, "volts"=w3649:dbl, "pf"=w3648:dbl)
                        n2179 = case shown="True" w3652 {
                          tunnel: w3659 -> [_ w3664]
                          tunnel: w3658 -> [_ w3713]
                          tunnel: w3657 -> [_ _]
                          tunnel: w3656 -> [_ _]
                          tunnel: w3655 -> [_ w3712]
                          tunnel: w3654 -> [_ w3711]
                          tunnel: w3653 -> [_ w3707]
                          tunnel: w3650 -> [_ w3666]
                          tunnel: w3649 -> [_ w3665]
                          tunnel: w3648 -> [_ w3663]
                          frame False {
                          }
                          frame True {
                            n2180 = local read "TDMS LAB05-2"() -> (w3704:refnum<k34>)
                            n2181 = Build Array(w3665) -> (w3693:dbl[])
                            n2182 = Build Array(w3663) -> (w3688:dbl[])
                            n2183 = Build Array(w3712) -> (w3683:dbl[])
                            n2184 = Build Array(w3713) -> (w3678:dbl[])
                            n2185 = Build Array(w3666) -> (w3700:dbl[])
                            n2186 = Build Array(w3664) -> (w3662:dbl[])
                            n2187 = Build Array(w3711) -> (w3673:dbl[])
                            n2188 = Build Array("TEMP Neut") -> (w3679:string[])
                            n2189 = Build Array("CYCLE") -> (w3674:string[])
                            n2190 = Build Array("TEMP Live") -> (w3684:string[])
                            n2191 = Build Array("PF") -> (w3689:string[])
                            n2192 = Build Array("AMPS OFF") -> (w3667:string[])
                            n2193 = Build Array("AMPS ON") -> (w3701:string[])
                            n2194 = Build Array("VOLTS") -> (w3695:string[])
                            n2195 = TDMS Write(0:w3704, 5:"LAB05-2 TEST VALUES", 7:w3701, 9:w3700) -> (4:w3672:refnum<k34>, 6:w3671:string, 15:w3661:errorcluster)  [unwired: 2 in, 1 out]
                            n2196 = TDMS Write(0:w3672, 5:w3671, 7:w3667, 9:w3662, 11:w3661) -> (4:w3670:refnum<k34>, 6:w3669:string, 15:w3660:errorcluster)  [unwired: 1 in, 1 out]
                            n2197 = TDMS Write(0:w3670, 5:w3669, 7:w3695, 9:w3693, 11:w3660) -> (4:w3692:refnum<k34>, 6:w3691:string, 15:w3690:errorcluster)  [unwired: 1 in, 1 out]
                            n2198 = TDMS Write(0:w3692, 5:w3691, 7:w3689, 9:w3688, 11:w3690) -> (4:w3687:refnum<k34>, 6:w3686:string, 15:w3685:errorcluster)  [unwired: 1 in, 1 out]
                            n2199 = TDMS Write(0:w3687, 5:w3686, 7:w3684, 9:w3683, 11:w3685) -> (4:w3682:refnum<k34>, 6:w3681:string, 15:w3680:errorcluster)  [unwired: 1 in, 1 out]
                            n2200 = TDMS Write(0:w3682, 5:w3681, 7:w3679, 9:w3678, 11:w3680) -> (4:w3677:refnum<k34>, 6:w3676:string, 15:w3675:errorcluster)  [unwired: 1 in, 1 out]
                            n2201 = TDMS Write(0:w3677, 5:w3676, 7:w3674, 9:w3673, 11:w3675) -> (4:w3705:refnum<k34>, 6:w3709:string, 15:w3710:errorcluster)  [unwired: 1 in, 1 out]
                            n2202 = TDMS Write(0:w3705, 5:w3709, 7:"TIME", 9:w3707, 11:w3710) -> (15:w3706:errorcluster)  [unwired: 1 in, 3 out]
                            n2203 = local write "data file error"(w3706) -> ()
                          }
                        }
                      }
                    }
                  }
                }
              }
            }
          }
          frame #13 {
            # "check for amps fail"
            # "check for cycle test & temperature rise fail conditions"
            n2204 = local read "on loops"() -> (w3739:dbl)
            n2205 = local read "jig cycle"() -> (w3736:dbl)
            n2206 = local read "jig cycle"() -> (w3741:dbl)
            n2207 = Add(x=w3739, y=3.0) -> (x+y=w3737:dbl)
            n2208 = Equal?(x=w3736, y=w3737) -> (x = y?=w3732:bool)
            n2209 = Equal?(x=w3741, y=1.0) -> (x = y?=w3734:bool)
            n2210 = stacked-sequence {
              tunnel: w3735 -> [w3744 _ _ _ _ _ _ _ _ _]
              tunnel: w3734 -> [w3745 w3765 w3785 w3805 w3825 w3845 w3865 w3885 w3905 w3925]
              tunnel: w3733 -> [w3742 _ _ _ _ _ _ _ _ _]
              tunnel: w3732 -> [w3743 w3764 w3784 w3804 w3824 w3844 w3864 w3884 w3904 w3924]
              tunnel: w3731 -> [_ w3763 _ _ _ _ _ _ _ _]
              tunnel: w3730 -> [_ w3762 _ _ _ _ _ _ _ _]
              tunnel: w3729 -> [_ _ w3783 _ _ _ _ _ _ _]
              tunnel: w3728 -> [_ _ w3782 _ _ _ _ _ _ _]
              tunnel: w3727 -> [_ _ _ w3803 _ _ _ _ _ _]
              tunnel: w3726 -> [_ _ _ w3802 _ _ _ _ _ _]
              tunnel: w3725 -> [_ _ _ _ w3823 _ _ _ _ _]
              tunnel: w3724 -> [_ _ _ _ w3822 _ _ _ _ _]
              tunnel: w3723 -> [_ _ _ _ _ w3843 _ _ _ _]
              tunnel: w3722 -> [_ _ _ _ _ w3842 _ _ _ _]
              tunnel: w3721 -> [_ _ _ _ _ _ w3863 _ _ _]
              tunnel: w3720 -> [_ _ _ _ _ _ w3862 _ _ _]
              tunnel: w3719 -> [_ _ _ _ _ _ _ w3883 _ _]
              tunnel: w3718 -> [_ _ _ _ _ _ _ w3882 _ _]
              tunnel: w3717 -> [_ _ _ _ _ _ _ _ w3903 _]
              tunnel: w3716 -> [_ _ _ _ _ _ _ _ w3902 _]
              tunnel: w3715 -> [_ _ _ _ _ _ _ _ _ w3923]
              tunnel: w3714 -> [_ _ _ _ _ _ _ _ _ w3922]
              frame #0 {
                # "LAB01-1"
                n2211 = case shown="True" w3742 {
                  tunnel: w3745 -> [_ w3758]
                  tunnel: w3744 -> [_ w3755]
                  tunnel: w3743 -> [_ w3754]
                  frame False {
                  }
                  frame True {
                    n2212 = local read "TEMP START LAB01-1"() -> (w3760:cluster{"TL":dbl, "TN":dbl})
                    n2213 = local read "RESULT LAB01-1"() -> (w3749:bool)
                    n2214 = local read "FAIL LAB01-1"() -> (w3752:cluster{"LO":dbl, "HI":dbl})
                    n2215 = local read "TDMS LAB01-1"() -> (w3759:refnum<k34>)
                    n2216 = local read "SET LAB01-1"() -> (w3756:T5)
                    n2217 = local read "DISP LAB01-1"() -> (w3757:T4)
                    n2218 = local read "SIG LAB01-1"() -> (w3761:T2)
                    n2219 = Bundle("FAIL LAB01-1"=w3752, "SIG LAB01-1"=w3761, "TEMP START LAB01-1"=w3760, "DISP LAB01-1"=w3757, "SET LAB01-1"=w3756, "TDMS LAB01-1"=w3759) -> (w3746:T25)  [unwired: 1 in]
                    n2220 = call "sub vi - cycle&temp fail v6.vi"("Amps Lo?"=w3758, "Input Cluster"=w3746, "SELECT"=w3755, "Amps Hi?"=w3754, "Result In"=w3749) -> ("(FAIL) out"=w3751:cluster{"FAIL LO":dbl, "FAIL HI":dbl}, "(DISP) out"=w3747:T4, "T-RISE"=w3748:cluster{"T-RISE (L)":dbl, "T-RISE (N)":dbl}, "Result Out"=w3750:bool, "file error"=w3753:errorcluster)  [unwired: 10 in]
                    n2221 = local write "TEMP RISE LAB01-1"(w3748) -> ()
                    n2222 = local write "FAIL LAB01-1"(w3751) -> ()
                    n2223 = local write "DISP LAB01-1"(w3747) -> ()
                    n2224 = local write "RESULT LAB01-1"(w3750) -> ()
                    n2225 = local write "data file error"(w3753) -> ()
                  }
                }
              }
              frame #1 {
                # "LAB01-2"
                n2226 = case shown="True" w3763 {
                  tunnel: w3765 -> [_ w3778]
                  tunnel: w3762 -> [_ w3775]
                  tunnel: w3764 -> [_ w3774]
                  frame False {
                  }
                  frame True {
                    n2227 = local read "TEMP START LAB01-2"() -> (w3780:cluster{"TL":dbl, "TN":dbl})
                    n2228 = local read "FAIL LAB01-2"() -> (w3771:cluster{"LO":dbl, "HI":dbl})
                    n2229 = local read "TDMS LAB01-2"() -> (w3779:refnum<k34>)
                    n2230 = local read "SET LAB01-2"() -> (w3776:T5)
                    n2231 = local read "DISP LAB01-2"() -> (w3777:T4)
                    n2232 = local read "RESULT LAB01-2"() -> (w3768:bool)
                    n2233 = local read "SIG LAB01-2"() -> (w3781:T2)
                    n2234 = Bundle("FAIL LAB01-2"=w3771, "SIG LAB01-2"=w3781, "TEMP START LAB01-2"=w3780, "DISP LAB01-2"=w3777, "SET LAB01-2"=w3776, "TDMS LAB01-2"=w3779) -> (w3766:T26)  [unwired: 1 in]
                    n2235 = call "sub vi - cycle&temp fail v6.vi"("Amps Lo?"=w3778, "Input Cluster"=w3766, "SELECT"=w3775, "Amps Hi?"=w3774, "Result In"=w3768) -> ("(FAIL) out"=w3770:cluster{"FAIL LO":dbl, "FAIL HI":dbl}, "(DISP) out"=w3773:T4, "T-RISE"=w3767:cluster{"T-RISE (L)":dbl, "T-RISE (N)":dbl}, "Result Out"=w3769:bool, "file error"=w3772:errorcluster)  [unwired: 10 in]
                    n2236 = local write "TEMP RISE LAB01-2"(w3767) -> ()
                    n2237 = local write "FAIL LAB01-2"(w3770) -> ()
                    n2238 = local write "DISP LAB01-2"(w3773) -> ()
                    n2239 = local write "RESULT LAB01-2"(w3769) -> ()
                    n2240 = local write "data file error"(w3772) -> ()
                  }
                }
              }
              frame #2 {
                # "LAB02-1"
                n2241 = case shown="True" w3783 {
                  tunnel: w3785 -> [_ w3798]
                  tunnel: w3782 -> [_ w3795]
                  tunnel: w3784 -> [_ w3794]
                  frame False {
                  }
                  frame True {
                    n2242 = local read "TEMP START LAB02-1"() -> (w3800:cluster{"TL":dbl, "TN":dbl})
                    n2243 = local read "FAIL LAB02-1"() -> (w3791:cluster{"LO":dbl, "HI":dbl})
                    n2244 = local read "TDMS LAB02-1"() -> (w3799:refnum<k34>)
                    n2245 = local read "SET LAB02-1"() -> (w3796:T5)
                    n2246 = local read "DISP LAB02-1"() -> (w3797:T4)
                    n2247 = local read "SIG LAB02-1"() -> (w3801:T2)
                    n2248 = local read "RESULT LAB02-1"() -> (w3788:bool)
                    n2249 = Bundle("FAIL LAB02-1"=w3791, "SIG LAB02-1"=w3801, "TEMP START LAB02-1"=w3800, "DISP LAB02-1"=w3797, "SET LAB02-1"=w3796, "TDMS LAB02-1"=w3799) -> (w3786:T27)  [unwired: 1 in]
                    n2250 = call "sub vi - cycle&temp fail v6.vi"("Amps Lo?"=w3798, "Input Cluster"=w3786, "SELECT"=w3795, "Amps Hi?"=w3794, "Result In"=w3788) -> ("(FAIL) out"=w3790:cluster{"FAIL LO":dbl, "FAIL HI":dbl}, "(DISP) out"=w3793:T4, "T-RISE"=w3787:cluster{"T-RISE (L)":dbl, "T-RISE (N)":dbl}, "Result Out"=w3789:bool, "file error"=w3792:errorcluster)  [unwired: 10 in]
                    n2251 = local write "TEMP RISE LAB02-1"(w3787) -> ()
                    n2252 = local write "FAIL LAB02-1"(w3790) -> ()
                    n2253 = local write "DISP LAB02-1"(w3793) -> ()
                    n2254 = local write "RESULT LAB02-1"(w3789) -> ()
                    n2255 = local write "data file error"(w3792) -> ()
                  }
                }
              }
              frame #3 {
                # "LAB02-2"
                n2256 = case shown="True" w3803 {
                  tunnel: w3805 -> [_ w3818]
                  tunnel: w3802 -> [_ w3815]
                  tunnel: w3804 -> [_ w3814]
                  frame False {
                  }
                  frame True {
                    n2257 = local read "TEMP START LAB02-2"() -> (w3820:cluster{"TL":dbl, "TN":dbl})
                    n2258 = local read "FAIL LAB02-2"() -> (w3811:cluster{"LO":dbl, "HI":dbl})
                    n2259 = local read "TDMS LAB02-2"() -> (w3819:refnum<k34>)
                    n2260 = local read "SET LAB02-2"() -> (w3816:T5)
                    n2261 = local read "DISP LAB02-2"() -> (w3817:T4)
                    n2262 = local read "SIG LAB02-2"() -> (w3821:T2)
                    n2263 = local read "RESULT LAB02-2"() -> (w3808:bool)
                    n2264 = Bundle("FAIL LAB02-2"=w3811, "SIG LAB02-2"=w3821, "TEMP START LAB02-2"=w3820, "DISP LAB02-2"=w3817, "SET LAB02-2"=w3816, "TDMS LAB02-2"=w3819) -> (w3806:T28)  [unwired: 1 in]
                    n2265 = call "sub vi - cycle&temp fail v6.vi"("Amps Lo?"=w3818, "Input Cluster"=w3806, "SELECT"=w3815, "Amps Hi?"=w3814, "Result In"=w3808) -> ("(FAIL) out"=w3810:cluster{"FAIL LO":dbl, "FAIL HI":dbl}, "(DISP) out"=w3813:T4, "T-RISE"=w3807:cluster{"T-RISE (L)":dbl, "T-RISE (N)":dbl}, "Result Out"=w3809:bool, "file error"=w3812:errorcluster)  [unwired: 10 in]
                    n2266 = local write "TEMP RISE LAB02-2"(w3807) -> ()
                    n2267 = local write "FAIL LAB02-2"(w3810) -> ()
                    n2268 = local write "DISP LAB02-2"(w3813) -> ()
                    n2269 = local write "RESULT LAB02-2"(w3809) -> ()
                    n2270 = local write "data file error"(w3812) -> ()
                  }
                }
              }
              frame #4 {
                # "LAB03-1"
                n2271 = case shown="True" w3823 {
                  tunnel: w3825 -> [_ w3838]
                  tunnel: w3822 -> [_ w3835]
                  tunnel: w3824 -> [_ w3834]
                  frame False {
                  }
                  frame True {
                    n2272 = local read "TEMP START LAB03-1"() -> (w3840:cluster{"TL":dbl, "TN":dbl})
                    n2273 = local read "FAIL LAB03-1"() -> (w3831:cluster{"LO":dbl, "HI":dbl})
                    n2274 = local read "TDMS LAB03-1"() -> (w3839:refnum<k34>)
                    n2275 = local read "SET LAB03-1"() -> (w3836:T5)
                    n2276 = local read "DISP LAB03-1"() -> (w3837:T4)
                    n2277 = local read "SIG LAB03-1"() -> (w3841:T2)
                    n2278 = local read "RESULT LAB03-1"() -> (w3828:bool)
                    n2279 = Bundle("FAIL LAB03-1"=w3831, "SIG LAB03-1"=w3841, "TEMP START LAB03-1"=w3840, "DISP LAB03-1"=w3837, "SET LAB03-1"=w3836, "TDMS LAB03-1"=w3839) -> (w3826:T29)  [unwired: 1 in]
                    n2280 = call "sub vi - cycle&temp fail v6.vi"("Amps Lo?"=w3838, "Input Cluster"=w3826, "SELECT"=w3835, "Amps Hi?"=w3834, "Result In"=w3828) -> ("(FAIL) out"=w3830:cluster{"FAIL LO":dbl, "FAIL HI":dbl}, "(DISP) out"=w3833:T4, "T-RISE"=w3827:cluster{"T-RISE (L)":dbl, "T-RISE (N)":dbl}, "Result Out"=w3829:bool, "file error"=w3832:errorcluster)  [unwired: 10 in]
                    n2281 = local write "TEMP RISE LAB03-1"(w3827) -> ()
                    n2282 = local write "FAIL LAB03-1"(w3830) -> ()
                    n2283 = local write "DISP LAB03-1"(w3833) -> ()
                    n2284 = local write "RESULT LAB03-1"(w3829) -> ()
                    n2285 = local write "data file error"(w3832) -> ()
                  }
                }
              }
              frame #5 {
                # "LAB03-2"
                n2286 = case shown="True" w3843 {
                  tunnel: w3845 -> [_ w3858]
                  tunnel: w3842 -> [_ w3855]
                  tunnel: w3844 -> [_ w3854]
                  frame False {
                  }
                  frame True {
                    n2287 = local read "TEMP START LAB03-2"() -> (w3860:cluster{"TL":dbl, "TN":dbl})
                    n2288 = local read "FAIL LAB03-2"() -> (w3851:cluster{"LO":dbl, "HI":dbl})
                    n2289 = local read "TDMS LAB03-2"() -> (w3859:refnum<k34>)
                    n2290 = local read "SET LAB03-2"() -> (w3856:T5)
                    n2291 = local read "DISP LAB03-2"() -> (w3857:T4)
                    n2292 = local read "RESULT LAB03-2"() -> (w3848:bool)
                    n2293 = local read "SIG LAB03-2"() -> (w3861:T2)
                    n2294 = Bundle("FAIL LAB03-2"=w3851, "SIG LAB03-2"=w3861, "TEMP START LAB03-2"=w3860, "DISP LAB03-2"=w3857, "SET LAB03-2"=w3856, "TDMS LAB03-2"=w3859) -> (w3846:T30)  [unwired: 1 in]
                    n2295 = call "sub vi - cycle&temp fail v6.vi"("Amps Lo?"=w3858, "Input Cluster"=w3846, "SELECT"=w3855, "Amps Hi?"=w3854, "Result In"=w3848) -> ("(FAIL) out"=w3850:cluster{"FAIL LO":dbl, "FAIL HI":dbl}, "(DISP) out"=w3853:T4, "T-RISE"=w3847:cluster{"T-RISE (L)":dbl, "T-RISE (N)":dbl}, "Result Out"=w3849:bool, "file error"=w3852:errorcluster)  [unwired: 10 in]
                    n2296 = local write "FAIL LAB03-2"(w3850) -> ()
                    n2297 = local write "TEMP RISE LAB03-2"(w3847) -> ()
                    n2298 = local write "DISP LAB03-2"(w3853) -> ()
                    n2299 = local write "RESULT LAB03-2"(w3849) -> ()
                    n2300 = local write "data file error"(w3852) -> ()
                  }
                }
              }
              frame #6 {
                # "LAB04-1"
                n2301 = case shown="True" w3863 {
                  tunnel: w3865 -> [_ w3878]
                  tunnel: w3862 -> [_ w3875]
                  tunnel: w3864 -> [_ w3874]
                  frame False {
                  }
                  frame True {
                    n2302 = local read "TEMP START LAB04-1"() -> (w3880:cluster{"TL":dbl, "TN":dbl})
                    n2303 = local read "FAIL LAB04-1"() -> (w3871:cluster{"LO":dbl, "HI":dbl})
                    n2304 = local read "TDMS LAB04-1"() -> (w3879:refnum<k34>)
                    n2305 = local read "SET LAB04-1"() -> (w3876:T5)
                    n2306 = local read "DISP LAB04-1"() -> (w3877:T4)
                    n2307 = local read "SIG LAB04-1"() -> (w3881:T2)
                    n2308 = local read "RESULT LAB04-1"() -> (w3868:bool)
                    n2309 = Bundle("FAIL LAB04-1"=w3871, "SIG LAB04-1"=w3881, "TEMP START LAB04-1"=w3880, "DISP LAB04-1"=w3877, "SET LAB04-1"=w3876, "TDMS LAB04-1"=w3879) -> (w3866:T31)  [unwired: 1 in]
                    n2310 = call "sub vi - cycle&temp fail v6.vi"("Amps Lo?"=w3878, "Input Cluster"=w3866, "SELECT"=w3875, "Amps Hi?"=w3874, "Result In"=w3868) -> ("(FAIL) out"=w3870:cluster{"FAIL LO":dbl, "FAIL HI":dbl}, "(DISP) out"=w3873:T4, "T-RISE"=w3867:cluster{"T-RISE (L)":dbl, "T-RISE (N)":dbl}, "Result Out"=w3869:bool, "file error"=w3872:errorcluster)  [unwired: 10 in]
                    n2311 = local write "TEMP RISE LAB04-1"(w3867) -> ()
                    n2312 = local write "FAIL LAB04-1"(w3870) -> ()
                    n2313 = local write "DISP LAB04-1"(w3873) -> ()
                    n2314 = local write "RESULT LAB04-1"(w3869) -> ()
                    n2315 = local write "data file error"(w3872) -> ()
                  }
                }
              }
              frame #7 {
                # "LAB04-2"
                n2316 = case shown="True" w3883 {
                  tunnel: w3885 -> [_ w3898]
                  tunnel: w3882 -> [_ w3895]
                  tunnel: w3884 -> [_ w3894]
                  frame False {
                  }
                  frame True {
                    n2317 = local read "TEMP START LAB04-2"() -> (w3900:cluster{"TL":dbl, "TN":dbl})
                    n2318 = local read "FAIL LAB04-2"() -> (w3891:cluster{"LO":dbl, "HI":dbl})
                    n2319 = local read "TDMS LAB04-2"() -> (w3899:refnum<k34>)
                    n2320 = local read "SET LAB04-2"() -> (w3896:T5)
                    n2321 = local read "DISP LAB04-2"() -> (w3897:T4)
                    n2322 = local read "SIG LAB04-2"() -> (w3901:T2)
                    n2323 = local read "RESULT LAB04-2"() -> (w3888:bool)
                    n2324 = Bundle("FAIL LAB04-2"=w3891, "SIG LAB04-2"=w3901, "TEMP START LAB04-2"=w3900, "DISP LAB04-2"=w3897, "SET LAB04-2"=w3896, "TDMS LAB04-2"=w3899) -> (w3886:T32)  [unwired: 1 in]
                    n2325 = call "sub vi - cycle&temp fail v6.vi"("Amps Lo?"=w3898, "Input Cluster"=w3886, "SELECT"=w3895, "Amps Hi?"=w3894, "Result In"=w3888) -> ("(FAIL) out"=w3890:cluster{"FAIL LO":dbl, "FAIL HI":dbl}, "(DISP) out"=w3893:T4, "T-RISE"=w3887:cluster{"T-RISE (L)":dbl, "T-RISE (N)":dbl}, "Result Out"=w3889:bool, "file error"=w3892:errorcluster)  [unwired: 10 in]
                    n2326 = local write "TEMP RISE LAB04-2"(w3887) -> ()
                    n2327 = local write "FAIL LAB04-2"(w3890) -> ()
                    n2328 = local write "DISP LAB04-2"(w3893) -> ()
                    n2329 = local write "RESULT LAB04-2"(w3889) -> ()
                    n2330 = local write "data file error"(w3892) -> ()
                  }
                }
              }
              frame #8 {
                # "LAB05-1"
                n2331 = case shown="True" w3903 {
                  tunnel: w3905 -> [_ w3918]
                  tunnel: w3902 -> [_ w3915]
                  tunnel: w3904 -> [_ w3914]
                  frame False {
                  }
                  frame True {
                    n2332 = local read "TEMP START LAB05-1"() -> (w3920:cluster{"TL":dbl, "TN":dbl})
                    n2333 = local read "FAIL LAB05-1"() -> (w3911:cluster{"LO":dbl, "HI":dbl})
                    n2334 = local read "TDMS LAB05-1"() -> (w3919:refnum<k34>)
                    n2335 = local read "SET LAB05-1"() -> (w3916:T5)
                    n2336 = local read "DISP LAB05-1"() -> (w3917:T4)
                    n2337 = local read "SIG LAB05-1"() -> (w3921:T2)
                    n2338 = local read "RESULT LAB05-1"() -> (w3908:bool)
                    n2339 = Bundle("FAIL LAB05-1"=w3911, "SIG LAB05-1"=w3921, "TEMP START LAB05-1"=w3920, "DISP LAB05-1"=w3917, "SET LAB05-1"=w3916, "TDMS LAB05-1"=w3919) -> (w3906:T33)  [unwired: 1 in]
                    n2340 = call "sub vi - cycle&temp fail v6.vi"("Amps Lo?"=w3918, "Input Cluster"=w3906, "SELECT"=w3915, "Amps Hi?"=w3914, "Result In"=w3908) -> ("(FAIL) out"=w3910:cluster{"FAIL LO":dbl, "FAIL HI":dbl}, "(DISP) out"=w3913:T4, "T-RISE"=w3907:cluster{"T-RISE (L)":dbl, "T-RISE (N)":dbl}, "Result Out"=w3909:bool, "file error"=w3912:errorcluster)  [unwired: 10 in]
                    n2341 = local write "TEMP RISE LAB05-1"(w3907) -> ()
                    n2342 = local write "FAIL LAB05-1"(w3910) -> ()
                    n2343 = local write "DISP LAB05-1"(w3913) -> ()
                    n2344 = local write "RESULT LAB05-1"(w3909) -> ()
                    n2345 = local write "data file error"(w3912) -> ()
                  }
                }
              }
              frame #9 {
                # "LAB05-2"
                n2346 = case shown="True" w3923 {
                  tunnel: w3925 -> [_ w3938]
                  tunnel: w3922 -> [_ w3935]
                  tunnel: w3924 -> [_ w3934]
                  frame False {
                  }
                  frame True {
                    n2347 = local read "TEMP START LAB05-2"() -> (w3940:cluster{"TL":dbl, "TN":dbl})
                    n2348 = local read "FAIL LAB05-2"() -> (w3931:cluster{"LO":dbl, "HI":dbl})
                    n2349 = local read "TDMS LAB05-2"() -> (w3939:refnum<k34>)
                    n2350 = local read "SET LAB05-2"() -> (w3936:T5)
                    n2351 = local read "DISP LAB05-2"() -> (w3937:T4)
                    n2352 = local read "SIG LAB05-2"() -> (w3941:T2)
                    n2353 = local read "RESULT LAB05-2"() -> (w3928:bool)
                    n2354 = Bundle("FAIL LAB05-2"=w3931, "SIG LAB05-2"=w3941, "TEMP START LAB05-2"=w3940, "DISP LAB05-2"=w3937, "SET LAB05-2"=w3936, "TDMS LAB05-2"=w3939) -> (w3926:T34)  [unwired: 1 in]
                    n2355 = call "sub vi - cycle&temp fail v6.vi"("Amps Lo?"=w3938, "Input Cluster"=w3926, "SELECT"=w3935, "Amps Hi?"=w3934, "Result In"=w3928) -> ("(FAIL) out"=w3930:cluster{"FAIL LO":dbl, "FAIL HI":dbl}, "(DISP) out"=w3933:T4, "T-RISE"=w3927:cluster{"T-RISE (L)":dbl, "T-RISE (N)":dbl}, "Result Out"=w3929:bool, "file error"=w3932:errorcluster)  [unwired: 10 in]
                    n2356 = local write "TEMP RISE LAB05-2"(w3927) -> ()
                    n2357 = local write "FAIL LAB05-2"(w3930) -> ()
                    n2358 = local write "DISP LAB05-2"(w3933) -> ()
                    n2359 = local write "RESULT LAB05-2"(w3929) -> ()
                    n2360 = local write "data file error"(w3932) -> ()
                  }
                }
              }
            }
          }
          frame #14 {
            # "run calibration routine"
            n2361 = local read "CALIBRATE"() -> (w3942:bool)
            n2362 = case shown="True" w3942 {
              frame False {
              }
              frame True {
                n2363 = stacked-sequence {
                  seq-local: [w3943 _ _] -> [_ w3945 _]
                  frame #0 {
                    n2364 = call "CALIBRATION PASSWORD"() -> ("PASSWORD"=w3943:string)  [unwired: 17 in, 2 out]
                  }
                  frame #1 {
                    n2365 = Equal?(x=w3945, y="7777") -> (x = y?=w3944:bool)
                    n2366 = case shown="True" w3944 {
                      frame False {
                      }
                      frame True {
                        n2367 = stacked-sequence {
                          frame #0 {
                            n2368 = call "sub vi - calibration v1.vi"() -> ()  [unwired: 12 in]
                          }
                          frame #1 {
                            n2369 = call "sub vi - get calibration values v1.vi"() -> ("LAB01 (CAL)"=w3951:T7, "LAB02 (CAL)"=w3950:T8, "LAB03 (CAL)"=w3949:T7, "LAB04 (CAL)"=w3948:T7, "calibration file error out"=w3952:errorcluster, "LAB05 (CAL)"=w3947:T7)  [unwired: 10 in]
                            n2370 = local write "calibration file error out"(w3952) -> ()
                            n2371 = local write "CAL LAB04"(w3948) -> ()
                            n2372 = local write "CAL LAB05"(w3947) -> ()
                            n2373 = local write "CAL LAB01"(w3951) -> ()
                            n2374 = local write "CAL LAB02"(w3950) -> ()
                            n2375 = local write "CAL LAB03"(w3949) -> ()
                          }
                        }
                      }
                    }
                  }
                  frame #2 {
                    n2376 = local write "CALIBRATE"(FALSE) -> ()
                  }
                }
              }
            }
          }
          frame #15 {
            # "save certain settings to file"
            n2377 = String To Path(string="c:\\crabtree\\Set Up\\") -> (path=w3955:path)
            n2378 = Build Path(base path=w3955, name or relative path="settings.bin") -> (appended path=w3957:path)
            n2379 = Build Path(base path=w3955, name or relative path="mail.bin") -> (appended path=w3954:path)
            n2380 = Create Folder(path (use dialog)=w3955) -> (error out=w3960:errorcluster)  [unwired: 2 in, 2 out]
            n2381 = call <vilib>:"Clear Errors.vi"("error in (no error)"=w3960) -> ()  [unwired: 6 in, 1 out]
            n2382 = stacked-sequence {
              seq-local: [w3962 _] -> [_ w3975]
              tunnel: w3957 -> [_ w3976]
              tunnel: w3954 -> [_ w3974]
              frame #0 {
                n2383 = local read "C drive data root dir"() -> (w3961:path)
                n2384 = local read "Network Directory"() -> (w3967:path)
                n2385 = local read "SET LAB05-2"() -> (w3966:T5)
                n2386 = local read "SET LAB05-1"() -> (w3965:T5)
                n2387 = local read "SET LAB04-2"() -> (w3964:T5)
                n2388 = local read "SET LAB03-2"() -> (w3968:T5)
                n2389 = local read "SET LAB04-1"() -> (w3963:T5)
                n2390 = local read "SET LAB03-1"() -> (w3969:T5)
                n2391 = local read "SET LAB02-2"() -> (w3970:T5)
                n2392 = local read "SET LAB02-1"() -> (w3971:T5)
                n2393 = local read "SET LAB01-2"() -> (w3972:T5)
                n2394 = local read "SET LAB01-1"() -> (w3973:T5)
                n2395 = Bundle("SET LAB01-1"=w3973, "SET LAB01-2"=w3972, "SET LAB02-1"=w3971, "SET LAB02-2"=w3970, "SET LAB03-1"=w3969, "SET LAB03-2"=w3968, "SET LAB04-1"=w3963, "SET LAB04-2"=w3964, "SET LAB05-1"=w3965, "SET LAB05-2"=w3966, "Network Directory"=w3967, "C drive data root dir"=w3961) -> (w3962:T17)  [unwired: 1 in]
              }
              frame #1 {
                n2396 = event shown="[1] \"SET LAB01-1\", \"SET LAB01-2\", \"SET LAB02-1\", \"SET LAB02-2\", \"SET LAB03-1\", \"SET LAB03-2\", \"SET LAB04-1\", \"SET LAB04-2\", \"SET LAB05-1\", \"SET LAB05-2\", \"Network Directory\", \"C drive data root dir\": Value Change" {
                  selector: _ -> [_ _ _]
                  dyn-events: _ -> [_ _ _]
                  timeout: 10.0 -> [_ _ _]
                  tunnel: w3976 -> [_ w3978 _]
                  tunnel: w3975 -> [_ w3979 _]
                  tunnel: w3974 -> [_ _ w3990]
                  event Timeout {
                    n2397 = event-data() -> ()  [unwired: 1 in, 3 out]
                  }
                  event "SET LAB01-1", "SET LAB01-2", "SET LAB02-1", "SET LAB02-2", "SET LAB03-1", "SET LAB03-2", "SET LAB04-1", "SET LAB04-2", "SET LAB05-1", "SET LAB05-2", "Network Directory", "C drive data root dir": Value Change {
                    n2398 = event-data() -> ()  [unwired: 1 in, 6 out]
                    n2399 = Open/Create/Replace File(file path (use dialog)=w3978, operation (0:open)=T16."replace or create") -> (refnum out=w3984:refnum<file>, error out=w3983:errorcluster)  [unwired: 4 in, 1 out]
                    n2400 = Write to Binary File(file (use dialog)=w3984, data=w3979, error in=w3983) -> (refnum out=w3982:refnum<file>, error out=w3981:errorcluster)  [unwired: 3 in, 1 out]
                    n2401 = Close File(refnum=w3982, error in=w3981) -> (error out=w3980:errorcluster)  [unwired: 1 out]
                    n2402 = local write "data file error"(w3980) -> ()
                  }
                  event "MAIL SETTINGS.OUT SERVER ADDRESS", "MAIL SETTINGS.FROM ACCOUNT", "MAIL SETTINGS.USER NAME", "MAIL SETTINGS.PASSWORD", "Auto Mail Send", "TO (string):": Value Change {
                    n2403 = event-data() -> ()  [unwired: 1 in, 6 out]
                    n2404 = local read "MAIL SETTINGS"() -> (w3989:T6)
                    n2405 = local read "Auto Mail Send"() -> (w3987:bool)
                    n2406 = local read "TO (string):"() -> (w3986:string)
                    n2407 = Open/Create/Replace File(file path (use dialog)=w3990, operation (0:open)=T16."replace or create") -> (refnum out=w3995:refnum<file>, error out=w3994:errorcluster)  [unwired: 4 in, 1 out]
                    n2408 = Bundle("MAIL SETTINGS"=w3989, "Auto Mail Send"=w3987, "TO (string):"=w3986) -> (w3988:T35)  [unwired: 1 in]
                    n2409 = Write to Binary File(file (use dialog)=w3995, data=w3988, error in=w3994) -> (refnum out=w3993:refnum<file>, error out=w3992:errorcluster)  [unwired: 3 in, 1 out]
                    n2410 = Close File(refnum=w3993, error in=w3992) -> (error out=w3991:errorcluster)  [unwired: 1 out]
                    n2411 = local write "data file error"(w3991) -> ()
                  }
                }
              }
            }
          }
          frame #16 {
            # "mail control"
            n2412 = local read "MAIL SETTINGS"() -> (w4012:T6)
            n2413 = local read "Auto Mail Send"() -> (w3998:bool)
            n2414 = Unbundle(w4012) -> ("OUT SERVER ADDRESS"=w4011:string, "FROM ACCOUNT"=w4010:string, "TEST MAIL"=w4009:bool)  [unwired: 4 out]
            n2415 = stacked-sequence {
              tunnel: "TO (string):" -> [_ w4051]
              tunnel: w4012 -> [w4017 w4050]
              tunnel: w4011 -> [w4016 w4049]
              tunnel: w4010 -> [w4015 w4048]
              tunnel: w4009 -> [w4014 _]
              tunnel: w3998 -> [_ w4047]
              tunnel: w4008 -> [_ w4046]
              tunnel: w4007 -> [_ w4045]
              tunnel: w4006 -> [_ w4044]
              tunnel: w4005 -> [_ w4043]
              tunnel: w4004 -> [_ w4042]
              tunnel: w4003 -> [_ w4041]
              tunnel: w4002 -> [_ w4040]
              tunnel: w4001 -> [_ w4039]
              tunnel: w4000 -> [_ w4038]
              tunnel: w3999 -> [_ w4037]
              tunnel: "TO (string):" -> [w4013 _]
              frame #0 {
                # "mail test"
                n2416 = case shown="True" w4014 {
                  tunnel: w4017 -> [_ w4021]
                  tunnel: w4013 -> [_ w4020]
                  tunnel: w4016 -> [_ w4019]
                  tunnel: w4015 -> [_ w4018]
                  frame False {
                  }
                  frame True {
                    n2417 = stacked-sequence {
                      seq-local: [_ _ w4031 _] -> [_ _ _ w4032]
                      tunnel: w4021 -> [w4024 _ _ w4036]
                      tunnel: w4020 -> [_ _ w4029 _]
                      tunnel: w4019 -> [_ _ w4027 _]
                      tunnel: w4018 -> [_ _ w4028 _]
                      frame #0 {
                        n2418 = Bundle(cluster=w4024, "TEST MAIL STATUS"="TEST START") -> (w4022:T6)  [unwired: 6 in]
                        n2419 = local write "MAIL SETTINGS"(w4022) -> ()
                      }
                      frame #1 {
                        n2420 = Wait (ms)(milliseconds to wait=500) -> ()  [unwired: 1 out]
                      }
                      frame #2 {
                        n2421 = call "sub vi - send mail with attach v5.vi"("TO:"=w4029, "subject"="MAIL TEST FROM LAB PANEL", "from"=w4028, "out going server"=w4027, "message"="TEST MESSAGE") -> ("error out"=w4031:errorcluster)  [unwired: 10 in]
                      }
                      frame #3 {
                        n2422 = Bundle(cluster=w4036, "TEST MAIL"=FALSE, "TEST MAIL STATUS"="TEST END", "mail error"=w4032) -> (w4034:T6)  [unwired: 4 in]
                        n2423 = local write "MAIL SETTINGS"(w4034) -> ()
                      }
                    }
                  }
                }
              }
              frame #1 {
                # "mail report"
                n2424 = stacked-sequence {
                  seq-local: [_ w4116 _ _] -> [_ _ _ w4284]
                  seq-local: [_ _ w4197 _] -> [_ _ _ w4274]
                  seq-local: [w4061 _ _ _] -> [_ w4110 _ _]
                  seq-local: [w4060 _ _ _] -> [_ w4109 _ _]
                  seq-local: [w4058 _ _ _] -> [_ w4107 _ _]
                  seq-local: [w4059 _ _ _] -> [_ w4108 _ _]
                  seq-local: [w4057 _ _ _] -> [_ w4106 _ _]
                  seq-local: [w4056 _ _ _] -> [_ w4101 _ _]
                  seq-local: [w4055 _ _ _] -> [_ w4102 _ _]
                  seq-local: [w4054 _ _ _] -> [_ w4103 _ _]
                  seq-local: [w4053 _ _ _] -> [_ w4104 _ _]
                  seq-local: [w4052 _ _ _] -> [_ w4105 _ _]
                  tunnel: w4051 -> [_ _ _ w4285]
                  tunnel: w4050 -> [_ _ _ w4268]
                  tunnel: w4049 -> [_ _ _ w4282]
                  tunnel: w4048 -> [_ _ _ w4281]
                  tunnel: w4047 -> [w4092 _ _ w4276]
                  tunnel: w4046 -> [_ _ w4227 _]
                  tunnel: w4045 -> [_ _ w4224 _]
                  tunnel: w4044 -> [_ _ w4223 _]
                  tunnel: w4043 -> [_ _ w4222 _]
                  tunnel: w4042 -> [_ _ w4221 _]
                  tunnel: w4041 -> [_ _ w4220 _]
                  tunnel: w4040 -> [_ _ w4219 _]
                  tunnel: w4039 -> [_ _ w4218 _]
                  tunnel: w4038 -> [_ _ w4217 _]
                  tunnel: w4037 -> [_ _ w4216 _]
                  frame #0 {
                    n2425 = case shown="False" w4092 {
                      frame False {
                        n2426 = local write "mail control"("") -> ()
                      }
                      frame True {
                      }
                    }
                    n2427 = local read "SET LAB01-1"() -> (w4091:T5)
                    n2428 = local read "SET LAB01-2"() -> (w4090:T5)
                    n2429 = local read "SET LAB02-1"() -> (w4089:T5)
                    n2430 = local read "SET LAB02-2"() -> (w4088:T5)
                    n2431 = local read "SET LAB03-1"() -> (w4087:T5)
                    n2432 = local read "SET LAB04-1"() -> (w4085:T5)
                    n2433 = local read "SET LAB05-1"() -> (w4083:T5)
                    n2434 = local read "SET LAB03-2"() -> (w4086:T5)
                    n2435 = local read "SET LAB04-2"() -> (w4084:T5)
                    n2436 = local read "SET LAB05-2"() -> (w4082:T5)
                    n2437 = Unbundle(w4087) -> ("DESCRIPTION"=w4067:string)  [unwired: 4 out]
                    n2438 = Unbundle(w4086) -> ("DESCRIPTION"=w4066:string)  [unwired: 4 out]
                    n2439 = Unbundle(w4085) -> ("DESCRIPTION"=w4065:string)  [unwired: 4 out]
                    n2440 = Unbundle(w4082) -> ("DESCRIPTION"=w4062:string)  [unwired: 4 out]
                    n2441 = Unbundle(w4088) -> ("DESCRIPTION"=w4068:string)  [unwired: 4 out]
                    n2442 = Unbundle(w4084) -> ("DESCRIPTION"=w4064:string)  [unwired: 4 out]
                    n2443 = Unbundle(w4091) -> ("DESCRIPTION"=w4080:string)  [unwired: 4 out]
                    n2444 = Unbundle(w4089) -> ("DESCRIPTION"=w4069:string)  [unwired: 4 out]
                    n2445 = Unbundle(w4083) -> ("DESCRIPTION"=w4063:string)  [unwired: 4 out]
                    n2446 = Unbundle(w4090) -> ("DESCRIPTION"=w4070:string)  [unwired: 4 out]
                    n2447 = Concatenate Strings("[LAB05-1/", w4062) -> (w4052:string)
                    n2448 = Concatenate Strings("[LAB05-2/", w4063) -> (w4053:string)
                    n2449 = Concatenate Strings("[LAB04-2/", w4064) -> (w4054:string)
                    n2450 = Concatenate Strings("[LAB03-2/", w4066) -> (w4056:string)
                    n2451 = Concatenate Strings("[LAB04-1/", w4065) -> (w4055:string)
                    n2452 = Concatenate Strings("[LAB03-1/", w4067) -> (w4057:string)
                    n2453 = Concatenate Strings("[LAB01-2/", w4070) -> (w4060:string)
                    n2454 = Concatenate Strings("[LAB02-2/", w4068) -> (w4058:string)
                    n2455 = Concatenate Strings("[LAB01-1/", w4080) -> (w4061:string)
                    n2456 = Concatenate Strings("[LAB02-1/", w4069) -> (w4059:string)
                  }
                  frame #1 {
                    w4114 = "/"
                    w4115 = 2.0
                    n2457 = local read "DISP LAB01-2"() -> (w4195:T4)
                    n2458 = local read "DISP LAB01-1"() -> (w4196:T4)
                    n2459 = local read "DISP LAB02-1"() -> (w4194:T4)
                    n2460 = local read "DISP LAB03-2"() -> (w4191:T4)
                    n2461 = local read "DISP LAB02-2"() -> (w4193:T4)
                    n2462 = local read "DISP LAB03-1"() -> (w4192:T4)
                    n2463 = local read "DISP LAB04-2"() -> (w4189:T4)
                    n2464 = local read "DISP LAB04-1"() -> (w4190:T4)
                    n2465 = local read "DISP LAB05-1"() -> (w4188:T4)
                    n2466 = local read "DISP LAB05-2"() -> (w4187:T4)
                    n2467 = Unbundle(w4195) -> ("CYCLE"=w4179:dbl, "MINS"=w4178:dbl, "STATUS"=w4175:string)
                    n2468 = Unbundle(w4196) -> ("CYCLE"=w4184:dbl, "MINS"=w4183:dbl, "STATUS"=w4180:string)
                    n2469 = Unbundle(w4194) -> ("CYCLE"=w4172:dbl, "MINS"=w4171:dbl, "STATUS"=w4170:string)
                    n2470 = Unbundle(w4191) -> ("CYCLE"=w4159:dbl, "MINS"=w4158:dbl, "STATUS"=w4155:string)
                    n2471 = Unbundle(w4192) -> ("CYCLE"=w4164:dbl, "MINS"=w4163:dbl, "STATUS"=w4160:string)
                    n2472 = Unbundle(w4193) -> ("CYCLE"=w4169:dbl, "MINS"=w4168:dbl, "STATUS"=w4165:string)
                    n2473 = Unbundle(w4190) -> ("CYCLE"=w4154:dbl, "MINS"=w4153:dbl, "STATUS"=w4150:string)
                    n2474 = Unbundle(w4189) -> ("CYCLE"=w4149:dbl, "MINS"=w4148:dbl, "STATUS"=w4145:string)
                    n2475 = Unbundle(w4188) -> ("CYCLE"=w4144:dbl, "MINS"=w4143:dbl, "STATUS"=w4140:string)
                    n2476 = Unbundle(w4187) -> ("CYCLE"=w4186:dbl, "MINS"=w4185:dbl, "STATUS"=w4137:string)
                    n2477 = Number To Decimal String(number=w4172) -> (decimal integer string=w4174:string)  [unwired: 1 in]
                    n2478 = Number To Decimal String(number=w4169) -> (decimal integer string=w4167:string)  [unwired: 1 in]
                    n2479 = Number To Decimal String(number=w4164) -> (decimal integer string=w4162:string)  [unwired: 1 in]
                    n2480 = Number To Decimal String(number=w4179) -> (decimal integer string=w4177:string)  [unwired: 1 in]
                    n2481 = Number To Decimal String(number=w4159) -> (decimal integer string=w4157:string)  [unwired: 1 in]
                    n2482 = Number To Decimal String(number=w4184) -> (decimal integer string=w4182:string)  [unwired: 1 in]
                    n2483 = Number To Decimal String(number=w4186) -> (decimal integer string=w4139:string)  [unwired: 1 in]
                    n2484 = Number To Decimal String(number=w4154) -> (decimal integer string=w4152:string)  [unwired: 1 in]
                    n2485 = Number To Decimal String(number=w4149) -> (decimal integer string=w4147:string)  [unwired: 1 in]
                    n2486 = Number To Decimal String(number=w4144) -> (decimal integer string=w4142:string)  [unwired: 1 in]
                    n2487 = Number To Fractional String(number=w4171, precision (6)=w4115) -> (F-format string=w4173:string)  [unwired: 2 in]
                    n2488 = Number To Fractional String(number=w4158, precision (6)=w4115) -> (F-format string=w4156:string)  [unwired: 2 in]
                    n2489 = Number To Fractional String(number=w4168, precision (6)=w4115) -> (F-format string=w4166:string)  [unwired: 2 in]
                    n2490 = Number To Fractional String(number=w4163, precision (6)=w4115) -> (F-format string=w4161:string)  [unwired: 2 in]
                    n2491 = Number To Fractional String(number=w4148, precision (6)=w4115) -> (F-format string=w4146:string)  [unwired: 2 in]
                    n2492 = Number To Fractional String(number=w4153, precision (6)=w4115) -> (F-format string=w4151:string)  [unwired: 2 in]
                    n2493 = Number To Fractional String(number=w4178, precision (6)=w4115) -> (F-format string=w4176:string)  [unwired: 2 in]
                    n2494 = Number To Fractional String(number=w4143, precision (6)=w4115) -> (F-format string=w4141:string)  [unwired: 2 in]
                    n2495 = Number To Fractional String(number=w4183, precision (6)=w4115) -> (F-format string=w4181:string)  [unwired: 2 in]
                    n2496 = Number To Fractional String(number=w4185, precision (6)=w4115) -> (F-format string=w4138:string)  [unwired: 2 in]
                    n2497 = Concatenate Strings(w4114, w4157, w4114, w4156, w4114, w4155) -> (w4131:string)
                    n2498 = Concatenate Strings(w4114, w4152, w4114, w4151, w4114, w4150) -> (w4130:string)
                    n2499 = Concatenate Strings(w4114, w4147, w4114, w4146, w4114, w4145) -> (w4129:string)
                    n2500 = Concatenate Strings(w4114, w4142, w4114, w4141, w4114, w4140) -> (w4128:string)
                    n2501 = Concatenate Strings(w4114, w4139, w4114, w4138, w4114, w4137) -> (w4127:string)
                    n2502 = Concatenate Strings(w4114, w4182, w4114, w4181, w4114, w4180) -> (w4136:string)
                    n2503 = Concatenate Strings(w4114, w4162, w4114, w4161, w4114, w4160) -> (w4132:string)
                    n2504 = Concatenate Strings(w4114, w4177, w4114, w4176, w4114, w4175) -> (w4135:string)
                    n2505 = Concatenate Strings(w4114, w4174, w4114, w4173, w4114, w4170) -> (w4134:string)
                    n2506 = Concatenate Strings(w4114, w4167, w4114, w4166, w4114, w4165) -> (w4133:string)
                    n2507 = Concatenate Strings("]", "\r") -> (w4111:string)
                    n2508 = Concatenate Strings(w4106, w4132, w4111) -> (w4122:string)
                    n2509 = Concatenate Strings(w4108, w4134, w4111) -> (w4124:string)
                    n2510 = Concatenate Strings(w4107, w4133, w4111) -> (w4123:string)
                    n2511 = Concatenate Strings(w4103, w4129, w4111) -> (w4119:string)
                    n2512 = Concatenate Strings(w4104, w4128, w4111) -> (w4120:string)
                    n2513 = Concatenate Strings(w4102, w4130, w4111) -> (w4118:string)
                    n2514 = Concatenate Strings(w4101, w4131, w4111) -> (w4117:string)
                    n2515 = Concatenate Strings(w4105, w4127, w4111) -> (w4121:string)
                    n2516 = Concatenate Strings(w4109, w4135, w4111) -> (w4125:string)
                    n2517 = Concatenate Strings(w4110, w4136, w4111) -> (w4126:string)
                    n2518 = Concatenate Strings(w4126, w4125, w4124, w4123, w4122, w4117, w4118, w4119, w4120, w4121) -> (w4094:string)
                    n2519 = Concatenate Strings("[PANEL/", "DESC/", "CYCLES/", "MINS/", "STATUS]", "\r", w4094) -> (w4116:string)
                    "MAIL REPORT" <- w4116
                  }
                  frame #2 {
                    w4225 = "END"
                    n2520 = local read "mail control"() -> (w4226:string)
                    n2521 = case shown="False" w4221 {
                      tunnel: w4226 -> [w4250 _]
                      tunnel: w4225 -> [w4249 _]
                      tunnel: [w4248 FALSE] -> w4211
                      frame False {
                        n2522 = Equal?(x=w4250, y=w4249) -> (x = y?=w4248:bool)
                      }
                      frame True {
                      }
                    }
                    n2523 = case shown="False" w4227 {
                      tunnel: w4226 -> [w4266 _]
                      tunnel: w4225 -> [w4265 _]
                      tunnel: [w4264 FALSE] -> w4215
                      frame False {
                        n2524 = Equal?(x=w4266, y=w4265) -> (x = y?=w4264:bool)
                      }
                      frame True {
                      }
                    }
                    n2525 = case shown="False" w4224 {
                      tunnel: w4226 -> [w4262 _]
                      tunnel: w4225 -> [w4261 _]
                      tunnel: [w4260 FALSE] -> w4214
                      frame False {
                        n2526 = Equal?(x=w4262, y=w4261) -> (x = y?=w4260:bool)
                      }
                      frame True {
                      }
                    }
                    n2527 = case shown="False" w4222 {
                      tunnel: w4226 -> [w4254 _]
                      tunnel: w4225 -> [w4253 _]
                      tunnel: [w4252 FALSE] -> w4212
                      frame False {
                        n2528 = Equal?(x=w4254, y=w4253) -> (x = y?=w4252:bool)
                      }
                      frame True {
                      }
                    }
                    n2529 = case shown="False" w4223 {
                      tunnel: w4226 -> [w4258 _]
                      tunnel: w4225 -> [w4257 _]
                      tunnel: [w4256 FALSE] -> w4213
                      frame False {
                        n2530 = Equal?(x=w4258, y=w4257) -> (x = y?=w4256:bool)
                      }
                      frame True {
                      }
                    }
                    n2531 = Or(x=w4213, y=w4212) -> (x .or. y?=w4204:bool)
                    n2532 = Or(x=w4215, y=w4214) -> (x .or. y?=w4205:bool)
                    n2533 = Or(x=w4205, y=w4204) -> (x .or. y?=w4200:bool)
                    n2534 = case shown="False" w4217 {
                      tunnel: w4226 -> [w4234 _]
                      tunnel: w4225 -> [w4233 _]
                      tunnel: [w4232 FALSE] -> w4206
                      frame False {
                        n2535 = Equal?(x=w4234, y=w4233) -> (x = y?=w4232:bool)
                      }
                      frame True {
                      }
                    }
                    n2536 = case shown="False" w4216 {
                      tunnel: w4226 -> [w4230 _]
                      tunnel: w4225 -> [w4229 _]
                      tunnel: [w4228 FALSE] -> w4210
                      frame False {
                        n2537 = Equal?(x=w4230, y=w4229) -> (x = y?=w4228:bool)
                      }
                      frame True {
                      }
                    }
                    n2538 = case shown="False" w4218 {
                      tunnel: w4226 -> [w4238 _]
                      tunnel: w4225 -> [w4237 _]
                      tunnel: [w4236 FALSE] -> w4207
                      frame False {
                        n2539 = Equal?(x=w4238, y=w4237) -> (x = y?=w4236:bool)
                      }
                      frame True {
                      }
                    }
                    n2540 = case shown="False" w4220 {
                      tunnel: w4226 -> [w4246 _]
                      tunnel: w4225 -> [w4245 _]
                      tunnel: [w4244 FALSE] -> w4209
                      frame False {
                        n2541 = Equal?(x=w4246, y=w4245) -> (x = y?=w4244:bool)
                      }
                      frame True {
                      }
                    }
                    n2542 = case shown="False" w4219 {
                      tunnel: w4226 -> [w4242 _]
                      tunnel: w4225 -> [w4241 _]
                      tunnel: [w4240 FALSE] -> w4208
                      frame False {
                        n2543 = Equal?(x=w4242, y=w4241) -> (x = y?=w4240:bool)
                      }
                      frame True {
                      }
                    }
                    n2544 = Or(x=w4209, y=w4208) -> (x .or. y?=w4203:bool)
                    n2545 = Or(x=w4207, y=w4206) -> (x .or. y?=w4202:bool)
                    n2546 = Or(x=w4210, y=w4211) -> (x .or. y?=w4198:bool)
                    n2547 = Or(x=w4203, y=w4202) -> (x .or. y?=w4201:bool)
                    n2548 = Or(x=w4200, y=w4201) -> (x .or. y?=w4199:bool)
                    n2549 = Or(x=w4199, y=w4198) -> (x .or. y?=w4197:bool)
                  }
                  frame #3 {
                    n2550 = local read "on loops"() -> (w4280:dbl)
                    n2551 = local read "jig cycle"() -> (w4277:dbl)
                    n2552 = local read "Send Mail Now"() -> (w4271:bool)
                    n2553 = Add(x=w4280, y=3.0) -> (x+y=w4278:dbl)
                    n2554 = Equal?(x=w4277, y=w4278) -> (x = y?=w4272:bool)
                    n2555 = And(x=w4272, y=w4271) -> (x .and. y?=w4270:bool)
                    n2556 = And(x=w4276, y=w4272) -> (x .and. y?=w4275:bool)
                    n2557 = And(x=w4275, y=w4274) -> (x .and. y?=w4273:bool)
                    n2558 = Or(x=w4273, y=w4270) -> (x .or. y?=w4269:bool)
                    n2559 = case shown="True" w4269 {
                      tunnel: w4285 -> [_ w4291]
                      tunnel: w4284 -> [_ w4290]
                      tunnel: "Lab Panel Test Status" -> [_ w4289]
                      tunnel: w4282 -> [_ w4288]
                      tunnel: w4281 -> [_ w4287]
                      tunnel: w4268 -> [_ w4286]
                      frame False {
                      }
                      frame True {
                        n2560 = stacked-sequence {
                          tunnel: w4291 -> [w4299 _]
                          tunnel: w4290 -> [w4298 _]
                          tunnel: w4289 -> [w4297 _]
                          tunnel: w4288 -> [w4296 _]
                          tunnel: w4287 -> [w4295 _]
                          tunnel: w4286 -> [w4294 _]
                          frame #0 {
                            n2561 = call "sub vi - send mail with attach v5.vi"("TO:"=w4299, "subject"=w4297, "from"=w4295, "out going server"=w4296, "message"=w4298) -> ("error out"=w4293:errorcluster)  [unwired: 10 in]
                            n2562 = Bundle(cluster=w4294, "mail error"=w4293) -> (w4292:T6)  [unwired: 6 in]
                            n2563 = local write "MAIL SETTINGS"(w4292) -> ()
                          }
                          frame #1 {
                            n2564 = local write "mail control"("") -> ()
                            n2565 = local write "Send Mail Now"(FALSE) -> ()
                          }
                        }
                      }
                    }
                  }
                }
              }
            }
          }
        }
        n2566 = node-c288() -> ()  [unwired: 1 in, 1 out]
        "loops" <- w165
        "stop2" <- "stop"
      }
      n2567 = node-c288(w142) -> ()  [unwired: 1 out]
    }
  }
